vi "UHR-Fleezers Control (host) -VD3_charlie.vi"(0 "Tab Control":T5(tab)) -> ()   [LabVIEW 2012]
uses:
  <vilib>/Utility/miscctls.llb/LVPoint32TypeDef.ctl
  <vilib>/Utility/miscctls.llb/LVMinMaxIncTypeDef.ctl
  <vilib>/userdefined/High Color/nirio_resource_hc.ctl
  <vilib>/Platform/TimedLoop/XDataNode/timing_clust.ctl
  <vilib>/Platform/TimedLoop/XDataNode/nitl_modes.ctl
  <vilib>/Platform/TimedLoop/XDataNode/wakeup.ctl
  <vilib>/FPGAPlugInAG/PCIe-7852R/niLvFpga_Open_PCIe-7852R.vi
  <vilib>/FPGAPlugInAG/PCIe-7852R/niLvFpga_Reset_PCIe-7852R.vi
  <vilib>/Utility/error.llb/Error Cluster From Error Code.vi
  <vilib>/rvi/errors/niLvFpgaAdjustHostInterfaceError.vi
  <vilib>/FPGAPlugInAG/PCIe-7852R/niLvFpga_Run_PCIe-7852R.vi
  <vilib>/Analysis/baseanly.llb/Mean (DBL).vi
  <vilib>/express/express analysis/Spectral/Block/exnSpectralBlock spectral measurements PSD poly.vi
  <vilib>/express/express analysis/Spectral/Block/exnSpectralBlock spectral measurements PSD WFM.vi
  <vilib>/Waveform/WDTOps.llb/WDT Append Waveforms DBL.vi
  <vilib>/FPGAPlugInAG/PCIe-7852R/niLvFpga_Abort_PCIe-7852R.vi
  <vilib>/FPGAPlugInAG/PCIe-7852R/niLvFpga_Close_PCIe-7852R.vi
  openfpgaref.8.6.ctl
  <vilib>/Platform/TimedLoop/XDataNode/XDataNode.xnode
  <vilib>/rvi/interface/nirviOpenFPGA/nirviOpenFPGA.xnode
  FPGA Bitfiles/UHR-FleezersInst_FPGATarget_UHR-FleezersCont_0F5B06C4.lvbitx
  UHR-Fleezers Control (fpga) - 10.3.vi
  <vilib>/rvi/interface/nirviMethod/nirviMethod.xnode
  <vilib>/rvi/interface/nirviReadWriteControl/nirviReadWriteControl.xnode
  <vilib>/express/express analysis/Spectral/XNode/ExpressSpectralMeasurementsBlockNode.xnode
  <vilib>/rvi/interface/nirviCloseFPGA/nirviCloseFPGA.xnode
  <vilib>/Analysis/NI_AALBase.lvlib
  <vilib>/Platform/TimedLoop/XDataNode/XDNodeRunTimeDep.lvlib
  <vilib>/vision/NI_Vision_Development_Module.lvlib
  NiFpgaLv.dll
  <vilib>/FPGAPlugInAG/PCIe-7852R/niLvFpga_ConfigureFifo_PCIe-7852R.vi
  <vilib>/rvi/errors/niLvFpgaMergeErrorWithErrorCode.vi
  <vilib>/FPGAPlugInAG/PCIe-7852R/niLvFpga_ReadFifo_PCIe-7852R.vi
panel:
  in  "Set SP to Reading":bool
  out "Trap X (AI1)":T1={"Trap 1"=-1.0, "Trap 2"=0.899993896484375}
  in  "Trap Pos FB SP":fxp<+/-,16,1>=-0.092803955078125 caption="Setpoint"
  in  "Trap Pos. FB ON":bool
  out "Trap Positions":waveform(dbl)[](graph)=[{"t0"=timestamp(12.90000000000001 s since 1904-01-01), "dt"=0.15, "Y"=[-1.7479351299698465e-12, -1.7479351299698465e-12], "attributes"=variant("NI_ChannelName"=variant(string "Trap 1 Pos."))}, {"t0"=timestamp(12.90000000000001 s since 1904-01-01), "dt"=0.15, "Y"=[6.991740519879386e-12, 6.991740519879386e-12], "attributes"=variant("NI_ChannelName"=variant(string "Trap 2 Pos."))}]
  out "Action (%)":dbl(knob) scale=-100.0..100.0
  in  "Trap Pos. FB Out Scale 2^n":u8=23 caption="Action Scale"
  in  "ESP Port 8":refnum<visa-resource-name>="COM22"
  in  "ESP Port 7":refnum<visa-resource-name>="COM22"
  in  "ESP Port 6":refnum<visa-resource-name>="COM22"
  in  "ESP Port 5":refnum<visa-resource-name>="COM22"
  in  "ESP Port 4":refnum<visa-resource-name>="COM22"
  in  "ESP Port 3":refnum<visa-resource-name>="COM22"
  in  "ESP Port 2":refnum<visa-resource-name>="COM22"
  out "Location path":path=path "D:/UnifiedHighRes_VIs/Locations.txt"
  out "Location Matrix":string[][](array[string])=[["N.D.\r\n", "N.D.\r\n", "N.D.\r\n"], ["0.19233\r\n", "0.00156\r\n", "0.20615\r\n"], ["N.D.\r\n", "N.D.\r\n", "N.D.\r\n"], ["N.D.\r\n", "N.D.\r\n", "N.D.\r\n"]]
  in  "radius":i32=10 min=1 max=20
  in  "clear markers":bool
  in  "trap\nmarkers?":bool
  in  "Pump 3 contents":string="Bottom: ADig beads" caption="contents"
  in  "Pump 1 contents":string="Top: DNA beads" caption="contents"
  in  "Scripts":T2(tab)
  in  "Take Stepping Data":bool
  in  "Got DNA bead":bool
  in  "Got ADig bead":bool
  in  "Cap 1 Flow ON":bool=TRUE
  in  "Move Cap. 1 (DNA Top)":bool
  in  "Dump Beads":bool
  in  "Cap 1 T ON":bool=TRUE
  in  "Cap 1 Samp Flow ON":bool=TRUE
  in  "Offset 2 Set":dbl=2.0
  in  "Offset 1 Set":dbl=1.0
  in  "Cal @ (MHz)":dbl=20.0
  in  "W/ Offset 1":bool=TRUE
  in  "Offset 1 Start (MHz)":dbl=13.0
  in  "W/ Offset 2":bool
  in  "Offset 2 Start (MHz)":dbl=16.0
  in  "Pause at Closest Delta (s)":dbl
  in  "Move to Delta 2 (MHz)":dbl=41.0
  in  "Attempt Limit":dbl=30.0 caption="Limit"
  out "Attempts":dbl=1.0
  in  "Wait Before Save (s)":u32=1
  in  "Fish for Tether":bool
  in  "Closest Delta (MHz)":dbl=13.0 step=0.25
  in  "Stop F (pN)":dbl=10.0
  in  "Then...":string(combo)="2"
  in  "Move to Delta 1 (MHz)":dbl=15.0
  in  "Tether Alarm?":bool=TRUE
  out "Tether":bool
  in  "TA Cancel Save?":bool=TRUE
  in  "TA Green Off?":bool=TRUE
  in  "Raster Set Upon Tether":u32=1
  in  "Save at end (5, 6)":bool
  in  "N Steps":dbl=20.0
  in  "Step Size (nm)":dbl=0.34
  in  "Save ave factor":dbl=1.0
  in  "Dip Trap Delta 1 (MHz)":dbl=15.0
  in  "Move Trap Before?":bool
  in  "Save Data After?":bool
  in  "Green ON After?":bool
  in  "Dip Trap Delta 2 (MHz)":dbl=15.0
  in  "Move Trap After?":bool
  in  "Duration (s)":dbl=1.0
  in  "Dip for Protein":bool
  in  "APD to Watch":bool
  out "Duration (s)":dbl
  in  "Action":string(combo)="Yank"
  in  "Fl. Triggered...":bool
  in  "Fl. Delta Thresh. (kHz)":dbl=0.6
  out "Waiting":bool
  out "Fl. High":bool
  in  "N pts to average":u16=6
  in  "Yank Delay (s)":dbl=3.5
  in  "Yank to Delta Array (MHz)":dbl[](array[numeric])=[16.3, 15.85, 14.85]
  in  "N Array El":u8=3 min=1 step=1
  in  "Random Choice":bool=TRUE
  in  "Force Yank":bool
  in  "Force Reset":bool
  in  "Y change (mm)":dbl
  in  "Profile":bool
  out "Sigma/Mean 2":dbl=nan caption="Sigma/Mean" format="%#_2g"
  out "Rate sigma (Hz) 2":dbl caption="Sigma (Hz)" format="%0.2f"
  out "APD 2 Rate (Hz)":dbl format="%#_3p"
  out "Primary Video Display":T3(plugin-control)
  out "Waveform Graph":dbl[](graph) caption="APD Line Scan"
  out "Messages":string="7:59 AM\tUHR-Fleezers ready.\r"
  in  "APD Ave N":dbl=10.0
  out "Int. Time (s)":dbl=3.0
  in  "Stop All":bool=TRUE
  out "Sigma/Mean":dbl=nan format="%#_2g"
  out "Rate sigma (Hz)":dbl caption="Sigma (Hz)" format="%0.2f"
  in  "Tab Control 6":T4(tab)=enum."Imaging"
  in  "APD 2 Offset":dbl
  in  "APD 1 Offset":dbl
  out "RMS (Ang)":dbl=nan format="%_2g"
  in  "Bead Sep. Int. Time (s)":dbl=5.0 caption="Int. Time (s)"
  in  "Below (kHz)":dbl=0.5
  in  "Above (kHz)":dbl=2.0
  in  "Adjust Scale\nto Mean":bool
  in  "Rescale on Mean":bool
  in  "Offset (nm)":dbl
  out "Mean":dbl=nan caption="Mean (pN)" format="%#_3g"
  out "Force":waveform(dbl)[](graph)=[{"t0"=timestamp(12.90000000000001 s since 1904-01-01), "dt"=0.15, "Y"=[nan, nan], "attributes"=variant("NI_ChannelName"=variant(string "T1 X"))}, {"t0"=timestamp(12.90000000000001 s since 1904-01-01), "dt"=0.15, "Y"=[nan, nan], "attributes"=variant("NI_ChannelName"=variant(string "T2 X"))}]
  out "APD Chart":waveform(dbl)[](graph)=[{"t0"=timestamp(12.90000000000001 s since 1904-01-01), "dt"=0.02, "Y"=[0.0, 0.0, 0.0, 0.0, 0.0, 0.0, 0.0, 0.0, 0.0, 0.0, 0.0, 0.0, 0.0, 0.0, 0.0], "attributes"=variant("NI_ChannelName"=variant(string "APD 1"))}, {"t0"=timestamp(12.90000000000001 s since 1904-01-01), "dt"=0.02, "Y"=[0.0, 0.0, 0.0, 0.0, 0.0, 0.0, 0.0, 0.0, 0.0, 0.0, 0.0, 0.0, 0.0, 0.0, 0.0], "attributes"=variant("NI_ChannelName"=variant(string "APD 2"))}]
  in  "Calibration":u16(ring) items=["None", "Position", "Force"]
  out "T1 X":dbl=nan caption="T1 X (pN)" format="%0.2f"
  out "T2 X":dbl=nan caption="T2 X (pN)" format="%0.2f"
  out "Bead Separation":waveform(dbl)(graph)={"t0"=timestamp(12.90000000000001 s since 1904-01-01), "dt"=0.15, "Y"=[nan, nan], "attributes"=variant("NI_ChannelName"=variant(string "T1 X"))}
  in  "Amplitude (nm)":dbl=3.0
  out "Bead Mean (nm)":dbl=nan caption="Mean (nm)" format="%0.2f"
  out "Difference":dbl=nan caption="Difference (pN)" format="%.2g"
  in  "Take Detection Laser\nImage":bool
  out "APD 2":T3(plugin-control) caption="APD 2 (Cy5)"
  in  "Flip Green Filter":bool
  in  "Set X Only":bool
  in  "Set Y Only":bool
  out "APD 1":T3(plugin-control) caption="APD 1 (Cy3)"
  out "Detection Laser Y":T3(plugin-control)
  out "Pointer Y (V)":dbl format="%_3g"
  out "Pointer X (V)":dbl format="%_3g"
  in  "Set Confocal Spot (X-Y)":bool
  out "Detection Laser X":T3(plugin-control)
  out "Saved APD":dbl[][](graph) caption="Most Recent Time Trace"
  out "Trap Delta Graph":dbl[](graph) caption="Most Recent Time Trace"
  out "Save APD Deriv":dbl[][](graph) caption="Most Recent Time Trace"
  out "Delta Fl. 1":dbl
  out "Delta Fl. 2":dbl
  out "All Signals":waveform(dbl)[](graph)=[{"t0"=timestamp(12.90000000000001 s since 1904-01-01), "dt"=0.02, "Y"=[0.0, 0.0, 0.0, 0.0, 0.0, 0.0, 0.0, 0.0, 0.0, 0.0, 0.0, 0.0, 0.0, 0.0, 0.0], "attributes"=variant("NI_ChannelName"=variant(string "APD 1"))}, {"t0"=timestamp(12.90000000000001 s since 1904-01-01), "dt"=0.02, "Y"=[0.0, 0.0, 0.0, 0.0, 0.0, 0.0, 0.0, 0.0, 0.0, 0.0, 0.0, 0.0, 0.0, 0.0, 0.0], "attributes"=variant("NI_ChannelName"=variant(string "APD 2"))}, {"t0"=timestamp(12.90000000000001 s since 1904-01-01), "dt"=0.15, "Y"=[nan, nan], "attributes"=variant("NI_ChannelName"=variant(string "T1 Y"))}, {"t0"=timestamp(12.90000000000001 s since 1904-01-01), "dt"=0.15, "Y"=[nan, nan], "attributes"=variant("NI_ChannelName"=variant(string "T1 X"))}, {"t0"=timestamp(12.90000000000001 s since 1904-01-01), "dt"=0.15, "Y"=[-0.0004235663930173644, -0.0004722739341410556], "attributes"=variant("NI_ChannelName"=variant(string "T1 Sum"))}, {"t0"=timestamp(12.90000000000001 s since 1904-01-01), "dt"=0.15, "Y"=[nan, nan], "attributes"=variant("NI_ChannelName"=variant(string "T2 Y"))}, {"t0"=timestamp(12.90000000000001 s since 1904-01-01), "dt"=0.15, "Y"=[nan, nan], "attributes"=variant("NI_ChannelName"=variant(string "T2 X"))}, {"t0"=timestamp(12.90000000000001 s since 1904-01-01), "dt"=0.15, "Y"=[-0.0005883053071687949, -0.0006281319620349712], "attributes"=variant("NI_ChannelName"=variant(string "T2 Sum"))}, {"t0"=timestamp(12.90000000000001 s since 1904-01-01), "dt"=0.15, "Y"=[nan, nan], "attributes"=variant("NI_ChannelName"=variant(string "T1 FB X"))}, {"t0"=timestamp(12.90000000000001 s since 1904-01-01), "dt"=0.15, "Y"=[-0.0004680013428144157, -0.0005167699209570592], "attributes"=variant("NI_ChannelName"=variant(string "T2 FB Sum"))}, {"t0"=timestamp(12.90000000000001 s since 1904-01-01), "dt"=0.15, "Y"=[nan, nan], "attributes"=variant("NI_ChannelName"=variant(string "T2 FB X"))}, {"t0"=timestamp(12.90000000000001 s since 1904-01-01), "dt"=0.15, "Y"=[-0.0006226691488387671, -0.0006504715109714008], "attributes"=variant("NI_ChannelName"=variant(string "T2 FB Sum"))}, {"t0"=timestamp(12.90000000000001 s since 1904-01-01), "dt"=0.15, "Y"=[-0.0007901852473525123, -0.0008601641895809732], "attributes"=variant("NI_ChannelName"=variant(string "PSD Y"))}, {"t0"=timestamp(12.90000000000001 s since 1904-01-01), "dt"=0.15, "Y"=[0.00031556138798181086, 0.0002525101474044007], "attributes"=variant("NI_ChannelName"=variant(string "PSD X"))}, {"t0"=timestamp(12.90000000000001 s since 1904-01-01), "dt"=0.15, "Y"=[-0.00019678334910122974, -0.0002453993346964931], "attributes"=variant("NI_ChannelName"=variant(string "PSD Sum"))}]
  in  "Signals to Plot":i32(listbox)
  out "Trap Disp. Freq. (Hz)":dbl=6.666666666666667 caption="Freq. (Hz)" format="%#_6p"
  out "Display Period (s)":dbl=0.15 caption="Period (s)" format="%#_6p"
  in  "Trap Disp. Downsample":dbl=10000.0 caption="Downsample" max=20000.0
  in  "APD Disp. Scale":dbl=0.1 caption="Scale (Divide,\nfor above plot only)"
  in  "APD Disp. Downsample":dbl=2.0 caption="Integrate" min=1.0 max=30.0 step=1.0
  out "APD Display Freq. (Hz)":dbl=50.0 caption="Freq. (Hz)"
  out "APD Display Period (s)":dbl=0.02 caption="Period (s)"
  out "FFT 1":cluster{"f0":dbl, "df":dbl, "magnitude":dbl[]}[](graph)=[{"f0"=0.0, "df"=16.666666666666668, "magnitude"=[-331.1367572010275, -79.05506245821404, -86.61411242440559, -88.4728176091699, -90.3181253945935, -94.12566333707997, -92.52740723119955, -94.92192587982518, -99.60936585245742, -96.87568627870715, -94.02570383337763, -83.8058550151726, -97.57441397235512, -101.59968530846606, -101.523049255742, -103.35038532190343, -101.58594091014982, -102.96098031851216, -91.39759462745924, -103.75019963279499, -104.45030075054324, -103.04245334279298, -104.0720279134107, -106.06482372394834, -103.69131867828104, -104.40395035115309, -105.96420043276396, -107.6735556337804, -106.673030006608, -107.34889066208132, -108.05626565233933, -106.25659018850432, -105.29934513380842, -105.43096056709592, -108.3728498841465, -106.0555440144992, -105.78001282181421, -107.48741857324953, -108.67624970548897, -105.39976667156175, -105.91413119232612, -109.4222808198164, -107.0898971593174, -107.91164191890915, -108.26032038855709, -107.58332347164534, -108.23559688234297, -108.01271040303237, -107.66511723652701, -106.51901583170391, -109.27249501469946, -108.55647681594805, -107.93499259231463, -107.05068166453935, -109.13641475410455, -109.29679733781423, -108.19360835527803, -109.57747591546632, -109.58364591011674, -110.47061433372711, -109.8144340420426, -108.79067462293897, -107.54887553357234, -107.99559866705923, -108.85023923652685, -109.68733225238618, -108.51101278437793, -108.51620475114115, -108.22212402200637, -104.63726950302143, -110.2989919678048, -107.61796444414897, -108.68882962798736, -104.79193983043893, -103.59504263746938, -93.64633660288543, -101.9191640501395, -105.73717393151816, -108.92572458793902, -107.43962662800902, -107.79595323081325, -107.0923101993207, -108.17603277205289, -107.87074270713183, -109.20899066381877, -108.61832060412445, -109.10072003106593, -105.76480632823524, -108.60877649218978, -109.67541158970121, -110.2286232768028, -109.84952155309578, -109.33772024076384, -109.95251642394683, -110.14777282585466, -109.13825677905699, -110.05989365698167, -109.39359990189426, -110.56255614635295, -109.66477183197163, -108.9397158528824, -110.26529907650465, -109.20049464984628, -108.20183857013548, -109.09752250184418, -108.00440442238454, -108.35465963524055, -111.16774134451799, -110.34812550238405, -108.94506763426756, -108.72845542102493, -109.41512344014713, -112.44661664432377, -110.35437330889101, -111.32939440655925, -109.42989530434981, -110.98084669076195, -111.92160561143541, -108.57755551751093, -111.40042616180912, -110.15284955891853, -112.21455132279115, -111.40787773511747, -108.82949641635288, -110.13442122547907, -111.42229298204664, -112.06314940885191, -110.6015308813694, -109.51144097251623, -111.15989713761475, -110.25535755335385, -109.65868178057926, -110.51649885452997, -109.77194745285269, -108.4234206864394, -109.50892632093968, -109.46471287444389, -107.92241289271415, -109.72283805386196, -108.63426821579918, -110.37316681536255, -111.09713996884652, -110.32903619589223, -105.32012665515045, -107.36858557554393, -108.00382215905725, -110.06430686942338, -108.81666625979916, -110.01277074453823, -110.94194741225512, -109.65934609082873, -107.80979136006962, -112.81333866824724, -111.61474300955487, -109.83998277184975, -109.45953946904639, -109.79640584952526, -108.19172301667324, -109.28894656674316, -107.61471301278785, -108.83814006090513, -109.08866847726084, -108.20250571862371, -107.96222236861584, -107.03811197900873, -108.93533000393974, -107.74482548035408, -110.79811544577694, -111.1387476496877, -107.42970105883512, -109.18442281176472, -108.73546184641192, -108.71800246690864, -108.51945944378063, -108.06825856571285, -107.27210712368412, -108.12304695877637, -107.84933283677306, -109.73682373154998, -109.32284761503395, -109.31328817453769, -106.68762108642842, -109.79203616876461, -109.9020278896408, -110.27080024357275, -108.54152101558762, -111.00464391726017, -112.42244020766577, -110.82707315747889, -111.00344011890857, -109.90461839395674, -109.42877207451863, -109.73549298167016, -111.67494793393293, -108.85799077901427, -108.5348443278263, -109.803781083881, -108.30644755543659, -108.5079527456017, -111.2055351312823, -108.53089994340155, -108.01739789012176, -108.70360662855235, -107.95873456794631, -109.58297170693093, -108.9372401694271, -110.15921663527153, -109.22399119911955, -110.89883651739237, -108.92840112258382, -110.0545300523626, -109.05961065387005, -109.45831398589371, -108.61239387653227, -110.13001256174265, -108.80060224137931, -109.46327400696283, -108.0177965824709, -109.29727944627197, -110.3237255895986, -109.03258262543821, -110.97880178489321, -109.70034895077919, -111.16405638194153, -109.17324451464711, -109.65698250854277, -108.96750235822178, -112.00534231585624, -108.69274607723942, -108.98110446396657, -108.40723795464795, -111.44459094807324, -111.74799245277113, -111.1601960491512, -108.92048232753773, -110.30506377784799, -111.33145973979093, -110.91850998672503, -110.33684985776448, -108.90206518366908, -109.28458878227542, -108.98773986023751, -110.85813863075646, -109.00041591105906, -110.84543686681204, -109.84382395806176, -109.69722434763266, -108.50915601095721, -107.80829925826895, -110.59736107582401, -109.75377770317087, -109.3992084496136, -110.51151565846742, -112.49753959826434, -109.7299632589479, -109.54070743868353, -109.90314341132164, -111.05974202976806, -109.03766862152392, -109.46667095459878, -109.52800799036197, -111.3163121356807, -110.07817134522178, -108.69251657453547, -109.40472158898045, -109.71400709815576, -110.60534468715097, -109.46937396724682, -107.70342491418788, -109.86331122597839, -108.64971387994616, -110.90117371097081, -108.34928840565928, -110.04172889660904, -111.52979926554961, -110.34759300823305, -109.62712781837159, -109.24131154553284, -110.23196152450447, -108.68509612326807, -108.0246905483419, -106.61876139289784, -101.5519630114271, -80.57695480953835, -102.03744443354402, -107.1449217193017, -110.0695213407169, -106.61597783999268, -110.79221011808191, -109.58974545931426, -109.1149802216988, -109.20993813088597, -109.63768480465863, -110.10428394219181, -109.08445084271477, -108.83472375362581, -109.69508502050168, -108.05588796178941, -110.62586360101581, -109.95315261676905, -107.52208264977473, -108.80708007514875, -110.43484881098874, -110.45942171588936, -107.83804717866751, -109.98973910294193, -109.3496496054193, -108.425252911127, -110.94579264380809, -108.54181722177951, -108.67696070083541, -108.4150202151644, -109.24973583101504, -112.0454922608961, -111.29046597340738, -110.75018248960077, -109.38326363603683, -109.2033340336957, -109.45076170874889, -109.52878049853727, -109.32340869724774, -110.98123395128233, -110.75736340635505, -109.7218385823809, -107.97422606064993, -109.77313701758703, -110.95948744392717, -110.08996774172691, -108.51011830110778, -109.78063140243836, -110.65996628628228, -109.83684298615616, -110.33329049188029, -110.13755118968292, -110.3717925645783, -108.55302219178951, -106.86811628734195, -108.6302156589162, -108.75341391045045, -108.32589578384841, -108.70061474734084, -112.30742263527534, -109.16842570592085, -109.29767035534508, -108.87829025017463, -108.2255616391397, -108.4316108616088, -108.82995906929271, -110.40135575415563, -109.51623498946435, -109.79409808792403, -107.03832759632121, -108.36534528684132, -109.72010868372905, -107.90933028179892, -106.95643597294047, -111.29929166165778, -110.23001135794706, -108.98838015381585, -109.79115357104436, -108.18627479511115, -108.14988122174307, -109.12074063466532, -109.41904850488358, -111.40409873721113, -108.83156790193294, -108.77032248953847, -108.88363158686694, -108.47515048290681, -105.94172147874599, -109.38146940214403, -109.21277078848794, -108.11309390545507, -110.70840012427504, -109.5504457849329, -109.52330684534209, -110.06776026911132, -108.21949434182314, -111.21266686269992, -108.78581501170974, -108.43115799297222, -109.63260325780062, -109.84070220619535, -109.72041980780126, -110.29615941882527, -110.60316734262464, -108.79165446414692, -110.95840439895592, -109.64926233107009, -109.16526769544322, -108.65292362430982, -109.56113898129935, -109.85693046339026, -108.92316027325207, -109.79492493553914, -109.38157962945887, -110.24545136266825, -109.30031463492487, -109.0795429936869, -111.4091719525013, -108.63499083917162, -108.43863465339358, -109.23207864880891, -111.21947487191643, -109.24525201480154, -109.56842406077318, -109.46711940800672, -111.91389548262572, -108.15655736690546, -108.71882059966947, -111.26328503478568, -110.95027143873176, -108.4853106242357, -110.36902802777546, -109.9314203579182, -108.77686164101732, -108.71871020068312, -111.04829661168574, -109.95072655339462, -109.88221342875462, -109.53241732756136, -108.2625005404823, -108.00677030040697, -110.19659317581693, -108.93858924796267, -109.46817875483995, -110.78063992017232, -111.11066570318451, -110.78774336696706, -109.19199744617812, -108.54914256407436, -109.28414960420909, -110.64143585101183, -110.5855350821307, -109.47578632252726, -108.89705360836223, -109.89214013612292, -107.93271261027171, -109.32631601340563, -108.60274611341092, -109.40110159872573, -110.889237682208, -110.01391165813328, -109.99747108785071, -108.65542819213674, -110.37211847668736, -110.44656500845738, -110.8128133834973, -108.8909299260433, -110.19551227077532, -111.37647266643523, -110.83802189730321, -109.98519377913681, -110.52378970770522, -108.16970420057817, -110.70974729773344, -110.76836765494402, -110.26884275594577, -109.22041044268806, -109.87809744746195, -107.76823252107832, -109.12119474042969, -110.28066108731146, -108.55000033509207, -110.18152097767907, -110.73030521152278, -111.49470908029893, -110.2320929919509, -110.03370979233021, -109.79181668155233, -108.6673501209991, -109.86695766650877, -107.88926518046961, -110.95525003776572, -109.18130359755742, -110.42618009658618, -107.90341931158893, -111.44736855661769, -110.72634267386593, -109.29945988519303, -107.67889101961411, -108.81148059987765, -109.13375212757057, -109.8122873383549, -109.80176697684155, -109.96342275204768, -109.90406635707086, -108.75674342748256, -110.12362902701081, -109.82151095527837, -108.62543344241836, -110.09171852771195, -110.21434637862887, -109.97254504855631, -109.27043209093468, -111.35149588204125, -110.12399876776051, -111.65983675538546, -109.28788875768564, -110.86554069990251, -111.26990906470603, -108.60956517491746, -111.49613890850938, -111.79685722966795, -109.26269485364045, -110.38555615546439, -109.40641023162068, -110.966136593156, -108.78892524584494, -110.29340727375603, -111.44032043281035, -109.95212021173755, -109.79233511584334, -112.41184021118175, -109.73687851881148, -108.65493879781806, -110.76132988919045, -108.43230346094671, -110.32968175895853, -110.29890782023821, -108.77609076424456, -110.3298662333555, -109.47734504217333, -108.2677295732245, -109.21234363352882, -107.83278941978479, -108.85136784424789, -108.43241251530755, -109.76609391460555, -108.53204373005357, -110.9660641972934, -110.3152512161094, -110.72570499399905, -109.23877906286317, -111.72407743101837, -109.20311421918561, -108.06021800233717, -109.29288625761943, -108.78395253409145, -111.85250172876302, -108.78827588901797, -109.79775055719482, -109.12089297455859, -109.49896359356035, -110.34432647103819, -107.94700097960238, -109.30489238477631, -108.89170290869342, -108.82574563272509, -110.11024077194833, -107.37946433552314, -109.60167933458756, -107.80625057819019, -110.11489057210264, -107.35436859378505, -105.69819484613895, -109.11280625683739, -109.27770293057978, -107.7053735252589, -109.75022444894368, -109.3310543596577, -107.87683693707739, -108.19931495338068, -109.26462246191564, -106.71885779297867, -100.00018022217961, -92.54434511397295, -107.20472143807373, -107.39203415155283, -110.04461177268398, -108.48860496315312, -109.0057168110333, -108.37627790492552, -108.4108380728248, -109.65509454313073, -109.64243000632982, -97.04219069306761, -109.0928856629964, -107.9760697315632, -107.52611064047497, -108.87702814778996, -109.08437599027614, -110.70097118837974, -109.00969860961283, -110.38275386163214, -110.0699155421545, -106.91498895181175, -106.22178738309017, -109.36827866896039, -107.59953130968307, -109.19516217272808, -108.31502495393616, -109.384158926223, -107.11670654202719, -108.09436312738853, -110.14559230873704, -109.84997663447679, -107.83465335309926, -108.60947100624459, -108.9932479423645, -109.17174810371898, -108.79457339828916, -109.40909327982367, -109.6328723628302, -109.51081854476179, -107.63054408568418, -109.63728404010122, -108.51163794839918, -107.55002282725216, -108.97796212764939, -107.24648164623483, -112.21470452291085, -108.74294024554423, -109.62070777514892, -108.05768666239368, -109.8224946685739, -109.34575507446003, -108.53536952609525, -109.60789300457671, -107.56681538208278, -109.22777325016398, -108.79047910308894, -110.10332477250668, -108.00206387955672, -108.45604004720035, -109.00645795765472, -109.81039564269616, -108.92785144634745, -108.3978471520567, -107.94411095685999, -110.53486519304262, -108.8773780319227, -109.03345093296107, -107.30746693745031, -108.54277704832029, -108.77629108166091, -108.91111762599647, -107.74965195880401, -109.97375370738439, -109.76326492689246, -107.91717581777407, -109.0730556927617, -107.66804873204664, -110.40438871064791, -108.05794247751498, -108.80206615156494, -107.51329354700796, -108.83687012994949, -107.57713176895379, -107.94774159581414, -109.41894615439651, -107.10869425078764, -110.51480854078629, -108.92221367099775, -109.91358786461535, -110.1744263092835, -109.30795472883494, -107.91359710691006, -109.77888185049835, -109.52060975706438, -108.66686651982212, -108.71041801553639, -110.13619546359467, -108.87957097273856, -109.72150387215271, -109.00776068810654, -109.70251113927438, -110.75769213896399, -108.53234896741436, -109.69439526582246, -110.15412541604617, -108.25183374628219, -107.97402569656481, -110.34920156998648, -108.45106995186384, -108.82031145748209, -111.38690005057539, -107.01968459818563, -110.3044500039584, -110.8755481852125, -111.08915057663255, -107.94824988655199, -110.21669144934839, -109.90539774633154, -109.58985438756767, -110.12258796623348, -109.41689951612143, -109.31128210476795, -109.00258476567323, -109.11093063041056, -108.83347064311234, -108.32685287566952, -109.44770946560935, -108.40145063144861, -109.68448193892085, -108.76525439243828, -107.62837139034596, -107.39300298848994, -109.36993934990318, -109.2465218489418, -106.66307369796812, -110.15891092764934, -109.57151745419041, -108.92425698310808, -109.8036704717834, -108.79751146756549, -109.25926431818017, -108.46260574057584, -109.1967554647261, -110.63319560262356, -109.02343067385144, -111.22073171487528, -109.4731095097105, -109.69335000085164, -109.48782989577005, -107.95204227683271, -108.19468255763758, -111.36195112053247, -109.55696116543685, -110.3130767640534, -108.9621824253354, -109.99735074896789, -109.20198058456344, -108.12100614259485, -111.27227490807289, -110.09248554008288, -109.14395535060149, -110.80882692379708, -109.22632926901655, -108.64497210802793, -111.00030482190711, -111.1317849358033, -107.43140429257826, -107.9783302193555, -109.2639893652291, -108.97008485446163, -108.66556668859064, -108.12995785876932, -109.73001061107855, -108.09691302413727, -110.68391499215569, -112.78583642012705, -108.7093037763389, -110.67868795924797, -109.0190959349128, -108.36247198231372, -109.82829353258869, -108.24916379311045, -109.84154533905823, -108.55470160833775, -109.75438989348815, -108.82865632118325, -107.63622268162582, -111.00943492886312, -110.81824358463759, -109.46028423652966, -107.52479398900992, -108.99087806823736, -109.94494831750349, -110.26788355564504, -109.8954055022304, -106.9478122391182, -108.91705388158901, -107.76095584490312, -109.28456723055147, -109.7982307261767, -108.98552661346622, -109.98937979783426, -110.57907422426224, -108.68113463944836, -108.06257240208589, -110.0707224529617, -109.19515280354733, -109.35868842818849, -110.37311467065695, -109.0404734478992, -108.16686395270187, -108.61859220485148, -109.19986437876149, -108.19707189725302, -110.06564239663074, -108.87850403465154, -110.63824157544798, -107.36918104067212, -108.7008736325543, -110.9359398265406, -111.08529123080929, -108.44209934821818, -109.79529621208783, -108.38917887958179, -108.169117639508, -109.24332926356216, -110.50584058811704, -109.63592524002665, -109.32261039377495, -109.16720880524552, -109.3084314664462, -109.5812223978583, -107.70213196487856, -108.0557884982431, -110.67058020007828, -111.68459781023608, -109.66270627185824, -110.52536245663693, -109.70208409132103, -108.78645420809342, -109.23122088059863, -109.24601474121832, -111.25604763816514, -109.50225851581177, -107.32434217163818, -109.28548556764925, -107.59972621660836, -110.46928774723048, -109.25950101547609, -110.32016453935465, -107.78482761561703, -107.89462895091089, -107.51366154391481, -108.08036891159172, -109.53371809947035, -101.2452927166745, -109.32763325689056, -107.52166868423687, -109.89648659445174, -109.11350200980485, -109.81336712738089, -110.02799517445062, -108.02767143538516, -107.97850220501483, -109.50772934896838, -109.31069875721964, -108.49991657749598, -105.60880911233095, -109.79128597340213, -106.91084537903113, -107.84880087118997, -109.63628170511824, -109.03203967193224, -110.64186113413658, -110.98027990365594, -112.33841002907062, -111.01793075565425, -108.58025797022215, -110.4259296883756, -110.38643255981424, -108.93051671115133, -110.97544177116494, -108.63883100482677, -108.37581711765226, -108.90240163126536, -107.94688047875466, -109.9482937437732, -110.09097112364414, -110.09805032265376, -111.44307114024532, -109.15483789122554, -110.9713708217832, -107.8548737634672, -111.41418477109195, -109.45699779859628, -97.03595099331734, -109.16746744169623, -109.66209204485918, -112.57048704774604, -109.73989735035725, -108.16252575067017, -110.7546980664636, -108.91536673403449, -109.20509151422344, -111.0260632167785, -109.62924582406518, -110.45466277291722, -110.2973970018937, -109.67550222925419, -108.84481022020094, -107.23686414357573, -111.79004633370906, -109.85453094194085, -109.45617270081004, -110.73920606732504, -108.90879956851099, -109.67774425528265, -109.4745715721361, -110.18080454693559, -109.26079184315502, -109.41692499885505, -109.02240975088358, -107.80833423058168, -109.32657361431549, -107.87138278655101, -110.910364670719, -109.70067156846706, -108.55301754282077, -109.4243252157005, -109.77567725161107, -107.83737232063925, -110.36509412773016, -109.6371048811367, -109.49430894422814, -108.55509251499753, -108.03996302911446, -110.4385715838736, -110.08864436068788, -109.48922484379962, -109.90865554258562, -109.7491963238264, -110.04796094537969, -107.413043439116, -108.54229076126079, -108.2522516728666, -109.75464941327974, -110.26795832300996, -109.28073673851144, -108.62990200974927, -109.89408067552287, -109.09160284731726, -109.90740624925795, -109.92534708896517, -109.79578862362752, -109.97278346890566, -107.80679350393824, -112.81728446281548, -108.09689504419987, -109.89549991422173, -108.43930976031248, -109.95153099843282, -108.18277483720716, -111.89607792605433, -109.52567003805, -109.17125106979698, -109.64300739407085, -108.21045178846524, -109.64036472149706, -109.02324448538845, -109.039163008889, -110.41006510134076, -109.50289952116489, -110.4732620447796, -110.08777181504614, -110.15589511434341, -109.55705089158471, -109.2547682932589, -110.86823885471617, -109.96330502176939, -109.85995369810554, -110.63211290903473, -112.08007783432191, -110.24725218052279, -107.62861148917592, -110.08691795849435, -108.89793794632287, -111.07702220466341, -109.46946126482341, -109.19747345337464, -110.70018609416007, -109.66366205691908, -110.78032312133551, -108.05724200456513, -108.195661625627, -110.90724508408255, -110.08307674771669, -110.76863516643007, -110.46620425061583, -109.16986788877276, -109.61921294239114, -108.51159432329543, -109.96308336765689, -107.38178944242856, -111.95930944846394, -109.3329826827624, -109.59119636368249, -108.83148571828912, -110.46194288788257, -105.87694286145472, -107.985886302892, -109.2975019660806, -111.05138725716857, -109.60005889204612, -110.92871351729086, -110.73480546964537, -108.41587420326718, -109.84275465824477, -108.8249071047676, -107.65358887817105, -108.3254150042995, -111.47362100321767, -112.7287536850025, -108.8217125660507, -109.50232320231771, -110.29587061625348, -109.30644535112089, -107.69178032077258, -110.84522325672016, -109.3735891463141, -109.12506388923123, -109.65582307934665, -111.11427272192576, -112.19827973435466, -109.11306367925813, -108.19203577968261, -107.89831568266465, -108.85805249169313, -109.51100049661844, -111.71546684086955, -109.53880495724334, -107.07739286222231, -110.66836728754211, -111.5415170557177, -110.16051267940297, -110.6107546662698, -111.36389129556191, -107.77888179117923, -110.34160392509817, -109.61287125994414, -110.23791773883013, -111.00669159903549, -110.97165069538953, -109.43965413392434, -110.6813161690388, -110.31441293654314, -111.96129906273796, -108.15998218707462, -110.08095912053633, -109.41084567452768, -109.28774416263552, -110.80159950384204, -110.41956747809755, -108.85005186267244, -107.9069227847757, -108.84249369063123, -109.92569208845894, -109.34109797584448, -109.41334788055491, -108.76462023086997, -108.22069272136177, -107.0786679601274, -108.30206755098202, -108.57613406368954, -110.83330887636482, -111.93966942736989, -109.76373713473264, -108.25782074884941, -108.16490627215555, -109.93351470267982, -110.75525684428368, -108.22814762283093, -109.73442331991602, -107.53145627482685, -108.27195221226805, -110.33032779278457, -109.48951857415828, -108.12599093700939, -107.97627415508097, -108.81426859968796, -111.21764717894752, -109.80856212352333, -110.92658779118501, -109.71551885834796, -110.38682741010847, -108.87671328341361, -109.68368600774755, -108.35359806351899, -111.7519400010676, -109.89407081573103, -108.24301180922755, -110.00646944788126, -108.6685299083706, -107.52856885980722, -111.7622363038509, -111.0025144494897, -108.64719599357296, -110.62968467177518, -108.821509935539, -107.94915453463719, -111.53070432277694, -109.87282048586256, -110.71167589371663, -109.79225006081626, -109.96203471712074, -110.29921092232489, -110.10644439440416, -111.28815007382043, -111.19165661703703, -108.46024117100558, -110.22528296512183, -110.32184972386672, -110.05120383416072, -109.78792549362107, -109.00355659956696, -108.85989369286315, -113.00899556732638, -110.91756826567867, -111.25016866167897, -111.84225040552181, -110.54451635944174, -110.72722829912917, -109.60759702177283, -110.49362602516815, -108.74419542915284, -110.3379671069179, -109.66259088220754, -110.45956400953156, -109.13956157147233, -109.27130155486806, -110.83015602667983, -109.17970724944131, -109.09662765889193, -108.0447366108107, -108.9536269357457, -110.35663108940085, -108.73418835472056, -113.42965806805827, -111.81270536656905, -110.06155590173537, -108.76582224646269, -106.7488061675813, -108.5700320158723, -111.11038264410035, -110.41435767488723, -109.12763443489911, -109.30517580756394, -111.61251165371237, -109.8116632664339, -109.36845864976851, -109.00390009629231, -110.54359197165573, -109.52629258465976, -110.75932197632896, -109.50903215359567, -107.42652056246085, -107.81146496533543, -103.22224383145215, -108.53803076819163, -109.78623360072066, -109.66306634612869, -110.80245829141279, -111.87835085452016, -102.27372781471168, -111.27763038431458, -108.45838423437681, -108.79077917058028, -109.31951755762685, -110.05415097017186, -109.5535934823387, -111.62732254641111, -110.73478247119641, -109.9468722686683, -110.39698367573979, -109.30612942398305, -109.7578384694043, -109.34817295524313, -105.56944757301993, -110.1940418750125, -109.27076023513962, -111.03491935225027, -112.2980497521063, -110.65725497955563, -109.0567530102422, -110.31700596563523, -109.64508026365678, -109.6190471404421, -110.52566833759428, -109.68595899227789, -109.7431160985074, -110.4798230300751, -109.45506977604765, -110.69504157940786, -110.63067849573177, -108.06456949500138, -107.99354148885966, -108.11349194720599, -109.15944121207349, -110.61766925164031, -110.14145801314527, -110.67420842201165, -111.91532881806512, -112.15901550030345, -109.94774413630104, -109.2819568305201, -110.94623189179737, -110.17685430287735, -110.39082916961016, -109.53953238698966, -110.76940623620611, -109.89327922318515, -109.10275695043765, -110.21445972656734, -110.58968777252528, -110.57016757660259, -109.59208496373341, -109.07946946465374, -109.10762003745964, -110.36892993974607, -109.81864495218393, -112.12972189864566, -109.26185849434863, -111.56305819991357, -111.36019621828058, -110.3397604159226, -109.58675612753163, -110.58041217474447, -106.34739062044932, -108.6722699609389, -110.03906060709869, -109.16794717548382, -109.65012481802809, -109.35377624077988, -110.51889143862303, -110.03397458059777, -110.7981307056636, -110.56653507062292, -107.61367005067231, -109.99279736988825, -111.79875182878175, -108.60382315996031, -109.71381533228038, -108.60388131505613, -107.0933685540362, -107.86037690830757, -108.40980028847238, -108.83869602763895, -110.76921375395764, -109.96766364716046, -110.8256171465781, -110.13805084291067, -108.5349140035878, -110.57158437465219, -110.8920694413417, -108.71646695477324, -108.33274238445665, -108.96152108305608, -111.03750932994224, -109.48915027983756, -110.29725207211165, -110.79527247268442, -109.47969936716117, -109.79306701834035, -110.16840035577498, -110.29840230783668, -109.15306387075587, -110.72651274964761, -109.08881658764956, -110.8349724030761, -110.64653625576447, -111.40392562616867, -109.94581588927414, -108.85136340231294, -109.77228546607624, -111.48297395390018, -109.7334001251941, -109.30537415590783, -109.63937411233408, -109.69785848648013, -109.3523781030017, -112.04667421182404, -111.56311816195343, -108.18548447362308, -110.63388993686104, -111.39768634137992, -109.87157345395542, -108.6734208287271, -109.46213300216168, -111.75774769437145, -110.10245994173216, -109.52385139033495, -110.96513097775451, -111.8709319163154, -111.54948269614047, -110.29760900080463, -108.52168175904663, -111.09033925738258, -111.14752744054172, -108.83074523709202, -109.05704141259113, -111.74377805749482, -109.57200906899736, -108.84121318623825, -110.86657990204343, -109.54363603755047, -110.89448416316372, -109.58965570570145, -110.21012263847972, -110.4063470702923, -109.5021950342969, -110.33648801598177, -110.90551031296536, -109.69205870504638, -109.8648503154861, -110.28183391384131, -109.65970942950766, -108.43615680946908, -111.11790511866548, -110.89043476451553, -113.64898442872548, -113.08004494963895, -110.81525412051718, -113.91009875719509, -110.95802128672312, -110.40944585634135, -110.33464695414992, -109.98984645778987, -110.18795067005652, -110.62364351231234, -110.44029833291248, -109.01598585569788, -110.95430216511514, -109.77987141110621, -108.54452361812068, -111.41780266439777, -110.47172771858405, -109.06084635984516, -109.30794593246578, -108.8764083815745, -108.18222749506985, -110.31330487887435, -109.04176821738014, -108.8558386035048, -109.47888284507395, -110.01459604573937, -110.48596659065309, -112.6781342298378, -109.85522803775775, -109.0569534499285, -109.08991286548698, -110.89485727880403, -109.18715778948663, -111.50381433568144, -111.3545424730884, -110.07710926239977, -111.99977850157067, -109.47444853853723, -109.81605328527645, -110.74995213151195, -112.56834665925544, -108.52052472391404, -110.89121213995557, -112.02004142355113, -108.66413739656008, -111.10053848695652, -110.41241079991636, -111.80152991764473, -110.21746151515111, -110.63265128607344, -109.483042128511, -112.78639954059729, -109.47114195846122, -109.23309637902875, -108.97133643967169, -110.08909147812822, -111.01105271457081, -111.18602432128249, -110.04633990216801, -109.53453538673071, -108.81939452082017, -111.13486114285661, -111.65877073200598, -111.63763706753498, -112.14107810664572, -113.6231865196724, -109.31743865878806, -109.18551713085722, -108.74951309653638, -109.28206426212142, -112.36687029711229, -110.10933061193728, -111.29501093502684, -108.19021080564794, -109.34497312126749, -110.37228033937312, -108.63277512903049, -110.61033993911002, -111.2975761598062, -111.49780004751436, -109.91019436685814, -109.32789992989028, -111.4482538110117, -110.1538439123475, -110.66347034043578, -110.05055133068794, -108.53002033538341, -111.7522199783972, -113.49108651193104, -108.03793940563418, -110.07108694011555, -110.83958739865201, -109.62805629409038, -112.69637731014087, -109.57996950503268, -110.104850643722, -108.83376203949506, -108.69400304840181, -110.59434352922563, -110.69121011800921, -110.18694553784364, -111.90598571547098, -110.30230802494223, -109.66810649416752, -112.6017099000434, -111.00296745333219, -110.64462650261785, -111.4775358707403, -111.98753241268494, -112.26574909791167, -112.04796822399412, -110.65853064447325, -109.6623218025264, -109.40559579075378, -110.42174451813142, -109.18991987957241, -111.02050178263048, -112.77950487440032, -110.42443751566815, -111.35440372400903, -108.5263524245987, -105.07498063939795, -107.15444425741984, -110.4508720018025, -110.25163264819463, -111.1383261104107, -109.91171620173931, -110.52200560606038, -110.5299174299573, -109.34628087255733, -110.26101817411786, -109.65071853372183, -109.66953335961068, -110.83590602054682, -110.980546313788, -109.4110066989163, -111.47223607390256, -110.00281523859483, -109.4088722967626, -109.00401922839337, -109.59655302543185, -109.7359970854586, -111.46016206343049, -110.23478747568004, -109.29441275295858, -109.82941912510167, -110.43088525283673, -108.21649744751299, -108.70220592702613, -105.2334473604296, -110.60620657984927, -107.97533820921146, -110.7664079806058, -110.56406610911355, -111.76465470250328, -108.84172809688911, -111.03661078143631, -109.85351980370237, -110.70091167176791, -109.52380717508088, -108.4356492672842, -112.25498760397127, -110.69648730540193, -110.36748838594507, -109.99090797924349, -111.2678642544111, -110.42541694325627, -111.4575545259775, -109.3211175669008, -112.7465573314208, -109.56208667784249, -111.59733497772172, -109.42295730962105, -108.55804089331346, -108.71397903286748, -110.09188290952392, -108.90810063278326, -110.31333217069538, -109.69794714542728, -109.06210020835357, -112.42465112160288, -111.74630553904855, -109.99304310093493, -108.93867687355595, -113.1669287525049, -109.09193568851137, -109.27500368450697, -108.99643325722404, -110.53962759110647, -111.2052088429852, -110.05855563908841, -110.30763723153481, -110.03411001268613, -109.6161415052669, -110.6304714466923, -110.17116005754627, -109.0753171640551, -110.92564270851628, -109.60831770517053, -110.25913363817017, -107.76644895378317, -109.2619309023068, -107.64198246311884, -107.37056168314048, -107.31978563121643, -107.68171928702894, -104.57515288104209, -104.75187637758803, -105.27246893266054, -106.96524396060869, -105.93920355631757, -103.66449995825586, -104.08476660009461, -104.53081578265315, -103.0148493379086, -106.74751670818362, -104.92309629919443, -103.98320340724693, -104.81633219413234, -105.77996356028235, -107.12559309216644, -107.28196039053535, -108.84583578337953, -109.4494696919565, -109.15525441177898, -109.7634811359225, -110.79433338587495, -108.44440079452527, -108.79597700117748, -109.98590735173822, -110.72144284267539, -109.30550753718086, -109.70072152916897, -109.65801130162137, -109.65949265997646, -109.82238573025273, -110.30669821947491, -109.83394128869384, -108.90433312205332, -110.664046708231, -110.39926453734134, -110.37725911098757, -112.12508639032839, -110.26795666332589, -108.98741993218054, -107.76168841100478, -109.82334992872889, -110.83516363498563, -112.60649745671253, -111.1960726449926, -111.03919163866381, -112.05129034965563, -108.83187987662883, -109.57240688505179, -109.32857861150738, -109.54934849013647, -108.29359879300195, -111.5179112931669, -109.52702486426027, -109.95429980789645, -110.7011078611564, -109.43204524997455, -105.56031249677113, -107.70609254346495, -108.78303653454363, -108.11457060956113, -110.44215460317537, -110.78267897406572, -110.33119812901934, -109.34449539666907, -108.82636558484161, -107.1834151347969, -108.83808254322192, -108.2542825327446, -108.80298057862501, -107.59922121598055, -108.9131916496929, -109.51519107961856, -107.7704986323755, -108.79678029009878, -111.13791068210752, -110.402746275919, -111.31702623823912, -108.49812727557243, -110.63723264798182, -109.32890666586829, -110.29721723278237, -111.66560929315017, -111.04227698307153, -111.36927505376269, -112.5203298417673, -109.93967930487354, -110.14533835678606, -110.3868348991775, -110.85413569165249, -108.44519725537315, -107.93391978795047, -109.82778679299085, -109.79311153223738, -109.25261055399044, -111.47738679135526, -111.11775495397512, -108.65898844492045, -110.26505495390529, -111.02017977446526, -110.34817965403467, -107.55161094495372, -110.21667403085983, -112.43970497917284, -110.70535338255132, -110.79438078890512, -109.81809822502822, -108.99167960596515, -106.5556893069368, -97.51736665041192, -105.29926513345109, -108.72453297392224, -108.23203912463346, -109.50324111400698, -110.9939986929772, -108.05367524487318, -108.37339392211176, -109.8553291283933, -110.46179639493138, -112.48795697163695, -111.88145079973545, -110.8678969738583, -110.62677605624849, -111.83824818603244, -109.76798658735359, -109.6654742351465, -112.58543522753767, -110.3406716250781, -109.55013159400883, -108.00481229232405, -109.90793236599207, -111.28597960985334, -110.54144527494444, -110.14704702870655, -111.2652554338908, -110.97520848958668, -108.63647576273343, -110.52472680617548, -113.16137826273847, -109.62457037485827, -109.53869420402964, -110.71399284283449, -108.55435337782664, -108.09492728294455, -112.2373886856363, -110.3693019226993, -111.65116752865308, -111.3223986412311, -109.67734725401074, -111.36420709226297, -109.14293108556625, -110.5982939020188, -110.29596476096043, -112.69847120697035, -108.39052787054206, -109.06205229490357, -110.00045399262885, -110.71775009467346, -110.69530760167493, -112.54144940754935, -109.55755373438097, -107.88943697845929, -109.98578587243783, -110.14202980613851, -110.80051915904802, -109.11327182471621, -109.50637030500913, -109.77023677605327, -109.98552825925917, -110.40235854896, -109.37603004890141, -111.36989177909379, -110.8399811877331, -109.30394670937987, -112.2769814990538, -109.10893172594731, -109.17733972841754, -108.35968166480572, -112.64492569586005, -110.13779257328873, -110.64439690778532, -108.45446935516622, -108.97325006911116, -110.54637968933774, -110.66412364132371, -111.38627695224784, -109.8942998516069, -110.36392017322382, -109.92355133054227, -109.61886697310419, -109.71969465343778, -109.85627196259388, -112.1407808286419, -111.1013489416651, -110.70428953307596, -109.3454280179969, -110.22984684615578, -109.53826801613613, -107.83673208330934, -108.72742563398342, -109.5745872123195, -108.83031823548816, -110.89059911076627, -109.87842545384129, -109.21980161063786, -109.07140273870678, -109.04628915564135, -108.79255665097845, -105.20875397856382, -110.0838008881032, -109.68293832806683, -111.24644641302518, -110.01257579497496, -110.99281477454484, -108.99296184719546, -110.96495665514604, -110.70404386182749, -108.25078498739035, -100.77667501455139, -107.61479263900088, -110.06600976399395, -110.02035637581871, -111.45524052052504, -109.975541184397, -111.07333860975358, -108.4808974233161, -109.59513524582242, -110.74711589861774, -109.50005300854993, -105.23071652566294, -111.81094849223531, -109.0168079712372, -111.89029991620679, -109.90672274216391, -109.30959446424889, -108.23718655264584, -110.10868108588909, -109.21139771899594, -110.33333323577992, -110.25792318324204, -110.67825932924109, -112.33148517950511, -108.9724848367048, -110.78371843797613, -111.40913868573313, -110.2930522718577, -111.9538408094371, -108.63639312641844, -112.4462941079034, -110.40266356498321, -108.66617580940074, -109.44306834729083, -111.08962916641603, -110.52132608161017, -110.53757698855654, -111.5587344449704, -109.77722315102946, -110.40060629757771, -109.45395807961631, -108.77558572395142, -109.0151938598724, -109.80739619986889, -108.9332873172888, -112.49933978358132, -111.28667321897437, -110.40629082858706, -109.9829216820938, -108.85102919990373, -110.84179127037925, -110.27309817549309, -109.88857884367955, -112.24517967927224, -110.23377125710859, -111.26951227953063, -110.09782138347559, -109.77508406986834, -110.55359722398646, -110.09534729906368, -109.96333904888587, -110.29372855476366, -111.36651812163072, -109.97141184588116, -110.16701683369045, -112.8562627359291, -110.66651146857079, -108.78873821095968, -108.59208174618087, -110.31784275318834, -109.43177042415276, -112.80272887161644, -111.79874205007107, -111.08216899537892, -110.73699224045636, -111.04738767291953, -110.43395896705012, -111.62106163510778, -111.32599933330843, -110.29360981749807, -109.66562228449096, -109.21316193790335, -110.06363162177448, -110.54480468587292, -109.31791670875509, -112.65386492377107, -109.91857609999171, -110.57233605624137, -110.7597333064856, -111.49767138733276, -109.36548654843229, -112.34145274183716, -110.52831153822652, -111.55802243871352, -111.81399803046556, -110.17680125962372, -111.23811621944807, -110.48042049674514, -112.43786993562033, -109.56507357271987, -110.67030752598993, -110.86377249100713, -109.06001892813467, -111.37023727930494, -109.52881096984436, -112.95107295160436, -110.49467818026214, -109.29804210589607, -109.89270706931751, -109.46354468058833, -112.10350702955014, -111.06083529077077, -110.49996587015904, -111.1617248913634, -108.84725633199014, -111.42852695852422, -110.01433866707184, -109.11616968390972, -110.76961079765468, -111.80403513904453, -109.84442686379181, -109.65447921666167, -111.3378640555306, -110.8882647652338, -112.58014202075226, -109.67128881545659, -111.73429980763389, -110.82258070774773, -110.71895931098041, -112.5117489008152, -109.16182299471309, -109.71651258790612, -109.7770618808562, -111.94294809571427, -111.1629115541574, -109.57489224865171, -109.8402445779754, -111.17931450307283, -110.09045865447595, -109.23658206733491, -112.54929616847242, -110.5150381158864, -111.32296447909377, -111.64472156295191, -111.65832771066007, -111.03359562742956, -110.85303206770837, -110.80655337650862, -109.3712696310075, -110.57313454785879, -111.18525355670417, -111.67423695430561, -112.00829831274282, -111.08915434609605, -110.3298290221436, -108.68552957386795, -112.11377370993225, -110.80288297661977, -110.33640536217185, -109.5907971201988, -107.9195263775506, -108.50223113159429, -111.91191347156142, -110.29585599512956, -109.50902788911351, -110.76819145749467, -108.86899533416589, -112.09963049260891, -110.13374376572433, -110.15881393584463, -110.87392107947531, -109.18658540731009, -109.72734703956934, -110.18732487568724, -108.76554115185057, -109.94122289815374, -110.39583285609643, -111.09540935727229, -110.6618176357367, -111.6281345666718, -109.69686483639367, -110.31633402076315, -110.61246951748903, -111.73300235294965, -111.34221378834899, -109.46708370903485, -110.70412671997354, -110.7007891485379, -110.31685483435038, -111.03016917417074, -110.94517365625376, -109.46580797053619, -111.20935248224806, -109.20661126636224, -109.50147037097533, -110.14241781654353, -109.8510950344643, -111.3794198224028, -111.28966889207122, -110.43347441663424, -109.86759980279523, -111.92101892013198, -109.31594011390644, -112.92253433794441, -110.74000829597605, -110.3690783911604, -111.9386136764295, -111.04196305034188, -110.41800427558245, -110.94287511448232, -111.66035388807579, -107.53723747644062, -110.68014818358719, -111.86628806511304, -110.12097497430523, -109.69880468221378, -111.4312783987915, -109.18240866486639, -111.45649839248873, -110.1242345454651, -113.75911576151633, -112.71747598882953, -110.9614554157337, -110.92294419716129, -110.87229098694876, -111.09943759113875, -109.48107247947176, -108.62783006742795, -110.8108025857779, -111.63342408317932, -112.0221522906341, -109.96411229549527, -111.29821085030613, -110.04566676239914, -108.41674583097112, -107.50256474992416, -108.68086611003493, -110.3738906060137, -108.86763212826641, -109.81681043446049, -111.04539822346567, -111.73290882980949, -109.75238769150758, -110.55268275367449, -110.48423701377924, -112.1116140908134, -109.53952175199518, -108.538611608547, -111.3788321484912, -110.36378736224961, -110.37712171023523, -109.82150687920334, -109.17046632238393, -105.1169578108227, -110.84067642540583, -112.91626789016587, -111.32030958133453, -108.93375913686056, -112.44450956563915, -111.1596840012794, -110.17380444915341, -109.634859036508, -110.68819277718731, -110.0648098825346, -108.87385575091399, -111.99676414571755, -111.32585405719519, -110.59892045991457, -110.32589048340424, -111.1172696292077, -109.79946399891651, -110.10030723919304, -110.71841081343656, -112.23013150012054, -108.94400401141407, -109.71044551701596, -111.77560214164039, -109.68779520039777, -110.96119601299907, -113.66477058855787, -110.17794649102234, -110.30159876509862, -110.11953836266514]}, ...(2 in all)]
  out "FFT 2":cluster{"f0":dbl, "df":dbl, "magnitude":dbl[]}[](graph)=[{"f0"=0.0, "df"=16.666666666666668, "magnitude"=[-324.19011195451765, -78.1272953812706, -85.85545438627958, -89.30587144190069, -92.90590394398903, -93.63083388385274, -91.8644929119412, -95.26924857401164, -97.0710469181336, -98.01148078956652, -99.33043660296804, -95.58776817681839, -99.9570097527269, -101.45494093095093, -101.51838334751548, -101.00386616525799, -103.01963069818913, -103.20223925731209, -103.53783076500916, -103.48065647812659, -103.97797518531912, -104.58942778240602, -104.46991277190502, -104.59813972158683, -104.56685024229951, -104.69893799348945, -105.05669000016238, -106.17061117835001, -106.43303821862656, -107.39468286383597, -106.2899368267905, -105.7863846168199, -105.17170638885071, -104.53818172761852, -106.70340956723133, -106.55444321137247, -106.67654843051936, -107.79888413750199, -107.86424326005849, -106.09722609215336, -107.71648639013972, -107.79500725395155, -106.17330953637067, -105.43663624517525, -108.04970689199158, -109.92106271611999, -106.2505251183406, -110.60221373795562, -107.11377887451098, -108.4126937286195, -108.37794745021417, -113.22457316369011, -106.38281814065472, -107.55385617652075, -108.93026538982782, -106.19334142366085, -108.90462602264525, -107.63084712174981, -109.12192537022624, -107.90627042480016, -109.44472079190832, -108.91731458372392, -105.74102972706788, -105.74407510394178, -107.5989477192235, -106.2838630137392, -107.46190542725505, -107.38881299750702, -109.08024783239452, -104.97871836903269, -106.65424712290651, -107.04966019632134, -106.16202578092883, -102.98374199247179, -99.1568704142098, -87.07383781389657, -96.41471411313154, -102.65176579899618, -107.65674867775193, -102.85397890306213, -107.58658613411464, -104.79044898833125, -106.65282019869865, -108.65027966345534, -109.46169054950127, -108.69969979291741, -110.4048706652988, -108.81020193837274, -109.42808902484134, -108.85398463561398, -108.3849716744813, -109.1844457168716, -109.32787859535676, -111.01992124870878, -106.64843449415699, -108.9926343573667, -111.59837822080355, -110.57121677672183, -111.17280164669164, -110.68901970586144, -111.69013245592781, -109.90200577018311, -109.3554172126163, -110.7515368822992, -109.2863324212524, -109.66209701262974, -108.50795548698007, -110.58126481096504, -112.36093896766921, -109.78612141282203, -108.85120530917233, -109.91424431080952, -109.84698632196245, -110.93960894966105, -109.77214706089354, -110.30762971422381, -108.77791302937449, -110.79522659679036, -108.47242514643455, -111.20629758187835, -109.05996769621125, -111.13574821570619, -107.79388178889101, -111.5768481279296, -110.52058839597171, -111.58729762739313, -108.99000864386126, -111.6585121505227, -110.50715371958135, -108.87151956974363, -110.30486244367107, -108.32392040018144, -108.1769507919999, -110.43198471512189, -109.81454097966842, -110.26717009815644, -110.82924135076777, -110.34103661156989, -110.0692667126265, -109.34555682020833, -109.1694484721415, -109.9940980324044, -110.81940616215803, -108.21162003366862, -107.97087538330561, -107.55312461506225, -110.60339321606872, -110.09004629292225, -109.05860430198882, -113.1412749514818, -109.81628200948371, -108.62343219429849, -109.48172424209761, -110.85978755785311, -109.47778611557064, -108.81728552967951, -107.47864241666747, -107.61735128422292, -109.62511618983821, -110.32417726356636, -108.24287897478176, -108.60460879530194, -110.2181558494026, -107.95550802888957, -110.80234484950323, -111.09955733353904, -109.43923052503506, -108.98949130235951, -110.05778199870154, -110.36224432927585, -108.13523430027999, -110.681114579241, -110.49106131529867, -108.73493328004297, -110.07663907252234, -109.9968931372618, -112.10715231091008, -108.80994125105168, -111.63774865669372, -111.54355694032755, -111.64024217585788, -109.34986300492378, -108.88053713185408, -111.14370830146245, -111.17327416167232, -110.36311492990576, -109.99414559884396, -112.96912007380595, -111.43191437097785, -111.71327312809349, -108.77202323682606, -110.25970374932486, -112.59574277180732, -109.77247894866957, -110.09219852365874, -111.7197662726775, -109.85454092697009, -110.06789440397942, -110.38055758638309, -111.04251386932805, -111.54279434240568, -109.74385329575985, -110.98924544863415, -111.17898077762852, -110.98364252730245, -110.75024385843372, -109.24766708578407, -109.67753987004863, -110.6537235844391, -111.84436313010086, -109.12654337292446, -109.65519521121124, -111.1845162935778, -110.5009101465602, -110.22980642268818, -110.88540043278346, -110.29249073109453, -108.80459864528464, -107.49372141121728, -108.50353962704821, -110.00730069533373, -112.012876492648, -109.01283702976382, -109.07442203290057, -108.2961442983685, -111.60962842680907, -108.84312815413224, -108.6276642979969, -108.75132871638827, -109.30004903844721, -107.20359872252604, -109.12175943862074, -110.43914247337625, -109.55954680842791, -110.37116786618797, -108.55907813251434, -110.19249995041955, -106.95269845697632, -111.07027929458712, -110.1073996792702, -110.61729280468039, -109.6419175310234, -109.47995019876329, -109.66602827275211, -110.01953864498805, -108.45989120418268, -109.79778555296474, -109.94663827736616, -109.52410616839379, -110.58014441463794, -110.09182359045897, -111.0487262011397, -110.49609187214915, -110.6114701312941, -111.17752423063314, -109.74965389041003, -108.58973724447526, -108.84292130035902, -108.90689510645983, -110.69840140049361, -111.30494362640982, -111.00224390075273, -110.50848328538423, -111.59232911931113, -109.30826761863756, -108.44510893127558, -109.63744704504391, -108.95037574307332, -111.36486409910674, -112.74508631930381, -111.03952454593811, -110.57133212903979, -110.59969855145111, -108.25570461975128, -110.44617635200193, -110.32190307214704, -110.95204704643322, -112.0595421753479, -110.45342552693265, -112.50183987758867, -110.08217804938009, -108.90353583389084, -107.02032313792242, -88.3334978919524, -107.92027625495886, -109.83148570028482, -110.30427997450572, -110.92855407802753, -109.67404674397338, -111.03606345823586, -110.58277018943096, -109.77692362669393, -109.39170901729935, -110.20711662408928, -109.41601946806779, -110.34213214925832, -111.2283900972803, -111.51682597931386, -110.47069117801351, -110.93808974285523, -111.11277478000933, -112.50698886748012, -112.12918507523611, -110.46316790252011, -109.9387334819968, -109.78723249688426, -107.13037722044297, -108.16132376075751, -109.07255491017162, -108.85068428558272, -110.28038153100799, -107.77611023481016, -110.69754506886444, -110.09495581837979, -109.21214884561816, -112.62718526248648, -109.22048725312992, -109.17793923163308, -110.87372121410577, -109.71902632604333, -112.61041177225496, -109.6374750969677, -110.74738952366951, -108.93404661877067, -109.84938675700889, -112.25316361679832, -110.30788094875312, -109.26929069321925, -111.20853536783942, -110.05212566057608, -111.72448131932816, -111.55474439772887, -111.81988954424324, -108.44452452934028, -109.21897824914645, -109.55634869894358, -111.36318572800242, -110.05777399011298, -109.64458567712875, -108.73315084760529, -108.93332091319675, -108.4816455312154, -108.80120578498936, -108.1804470361839, -109.7177707524778, -109.31977709844544, -109.33603116022124, -111.46120546572519, -111.7480378245176, -109.17907150677627, -110.47970652472505, -109.73718750984082, -109.7935026884937, -110.40458408612054, -110.91781389491092, -108.39352075861481, -108.27512197925346, -109.59155075404814, -110.40183121737397, -109.25423373270381, -108.37769008625712, -107.91335995938509, -109.5576520703013, -107.27392145737491, -110.98592762117059, -108.41809950647861, -111.48163889400448, -109.70961684769624, -109.22952568656495, -109.76504719131209, -108.86928627177666, -107.97855299877004, -109.8412204399902, -109.6690048999326, -112.28329030175193, -111.54977099314607, -109.55689540119126, -107.93716711232997, -109.84247640855929, -111.5098351445789, -109.14317615215809, -110.28319116384824, -110.57901069942578, -107.2890252845352, -109.66754569546274, -110.15708115946433, -108.83782190109405, -111.60783857760667, -111.46884385151185, -109.21985333366634, -109.63605494317056, -110.87999187262697, -112.26992029775087, -111.05491095860552, -109.22795442529183, -108.99135781712076, -110.46475190704264, -109.35746113713218, -109.29125989270668, -107.40922407684049, -109.24391685563656, -110.41554602144217, -110.68952735085914, -110.62457364102458, -110.39856310555466, -108.84256124354566, -110.01614601335088, -109.8071306678428, -110.2804500736802, -108.76205061238203, -110.3962440297242, -108.98253716257014, -109.32990745926702, -111.17276766165281, -110.41113652364085, -110.36616199963426, -112.09767002991742, -108.43599666470733, -110.91876588140981, -109.05329272502944, -107.07198690769708, -108.72934463903034, -108.6666471996132, -108.97529973794413, -109.68895260146817, -109.2658844652487, -109.75690097249196, -109.38585024123027, -110.17593039468063, -107.87223111061134, -108.15261097418302, -110.09277437980633, -110.8665497655964, -108.43061614348413, -110.3052458526819, -109.22446919161898, -110.51909692711594, -110.06620699121913, -109.53439413051383, -110.31952463872884, -111.4732125902982, -110.41443606663168, -109.9579358088152, -109.930778061577, -108.5473214465574, -109.34719220288939, -109.16964653934396, -110.04824158176345, -109.42616539603762, -108.3556027482992, -110.62331917617789, -111.3652147859356, -110.12362012120938, -110.13175448595814, -111.20110099151856, -111.50643914621541, -108.11659117128028, -111.06037600347967, -109.03822892917451, -108.25678204604324, -110.82608024151122, -109.15887945314851, -109.88255674562845, -111.18322672526185, -110.95836040044516, -107.91535345885436, -110.66285812468733, -109.61906549925033, -109.58059721670746, -109.65198009505977, -109.65950565672951, -108.95264505276342, -109.23343669003113, -110.74308548011575, -106.39170014998685, -109.61471203101753, -108.24258770956924, -109.84609566640096, -107.83834185503922, -108.93052854090027, -107.55568820082641, -109.758551082242, -110.65892780872205, -111.99907420485852, -110.71043004141137, -110.62257237494617, -109.15610413532767, -106.87403836327807, -108.19175324576331, -110.27819583792918, -110.23918003777561, -108.29703377268754, -110.07182881114713, -109.60256111108491, -111.00394752430006, -110.30750337485472, -108.78309624082331, -109.24103013025798, -108.76979253891403, -109.91618737478264, -108.83915940855513, -110.92536150834754, -109.72250903746432, -108.96533939688658, -111.08949280651164, -109.20335070860871, -109.37826578362439, -109.77953166722301, -110.1867310744785, -110.07114559821346, -110.7003631567182, -107.86455899696074, -108.94113264174617, -109.35999427135138, -109.33627364788704, -108.96588828808375, -109.08716536982254, -108.73575375369026, -109.47770132070654, -109.83726171472907, -110.73516506891792, -110.56827134787686, -107.65667508354096, -109.30200115708924, -109.28406803847896, -110.55374624323233, -111.2017766725333, -108.50851279608973, -109.79494403619485, -109.08320018013063, -110.21850624918747, -108.4652936555984, -108.74837610538873, -108.81326140648238, -108.83830180036702, -108.785270477003, -110.01845876259073, -108.76030368637825, -108.57879884880157, -110.6610608456059, -108.74669367794318, -111.55956030460833, -110.22906685783455, -110.48411613865359, -109.48060880085136, -112.77556331479562, -108.2676071206087, -108.8571136162698, -108.56944905160177, -109.16406757131058, -111.42259299295839, -108.25216316582294, -110.48487127684025, -109.69532331373831, -108.13992755196784, -109.2987762526628, -109.82536192480795, -111.28650061088359, -109.12820736404241, -109.37960655471406, -108.96014976926716, -107.97535047619023, -112.31953123574708, -109.06198330523004, -107.52722515967098, -107.31555373665437, -99.89671790804692, -107.44442600896275, -110.6549218761941, -108.02265794322076, -109.63582761762919, -110.00574746987859, -109.51565124961209, -109.3550083591902, -110.4541529175301, -107.85799722437162, -105.1197113090786, -110.25038075579738, -110.39710812865657, -109.3618876098789, -107.6131301952152, -109.21529527621463, -108.7995754403799, -108.48347353145697, -106.45678488065816, -109.60427918561142, -110.81194387812535, -109.52215044127382, -109.88751598659705, -109.30205143590227, -110.74984456751768, -109.03952092986351, -110.69170786328897, -110.39236248162467, -108.65456161733339, -107.60439764386904, -109.97367926606955, -110.2754359970249, -108.81546418006434, -106.99691398176165, -108.42047325825182, -107.24499915944605, -109.28116135603187, -108.70650358781573, -108.05516916105047, -107.20893100196241, -112.07029265690055, -109.38099990478445, -111.53461820465232, -108.11312509555277, -108.76714028655223, -109.89565008459624, -107.71879172001115, -108.08434857420214, -108.79142773619792, -107.25153085963885, -110.05595039449301, -109.31604222314259, -109.94405791565286, -109.04715370361387, -108.89278831045846, -108.84682466376424, -110.0067927716526, -107.63768959294084, -108.98109382020348, -111.4720219575084, -110.76023788797733, -108.78599647633777, -106.59726674064618, -108.66715709719243, -107.99134359630926, -110.11396713841884, -107.21091759882775, -108.08576824949941, -108.80217666857972, -111.72949572713338, -107.33126296136014, -107.33731660097102, -108.04470462977443, -109.42963925921418, -111.03517778720736, -109.55293581015796, -107.99948151285162, -106.59480934999681, -107.63777243313498, -108.96490626068824, -108.8948210299064, -108.30870516747477, -109.13612869658097, -109.59971429402015, -110.2571461001396, -108.7655464686992, -109.81144209568883, -109.80796806645141, -109.20948481699544, -108.68653880881129, -109.26329796696166, -109.22428132233863, -110.12571678351438, -109.14615461144786, -107.08261621308327, -109.11338327144382, -107.75421565039201, -107.45291780756361, -109.00477000647248, -107.41031480478154, -109.98948062864928, -107.45953654921264, -106.37522884807879, -107.7786128523167, -108.03610987358499, -108.05926797128022, -108.59400205554164, -109.89620453365603, -109.03811240487515, -109.96909236705363, -109.28212981785472, -109.6772152101994, -108.26493868190678, -110.55558039199732, -106.6252818398841, -110.19075011176416, -109.56520012524705, -109.8023423576176, -111.2697570480663, -108.26752571816566, -112.00337375484828, -109.85709226796116, -109.36922081321148, -108.8424844298318, -111.2512302139209, -110.61775974680471, -110.22501328999012, -107.76874906708105, -110.71023653476604, -109.4025656165291, -107.66667684986125, -107.59759854092948, -107.94763263251238, -107.3888591871119, -108.62692803125044, -109.18012867988286, -107.78662871481455, -108.5072814073944, -109.50348958982907, -109.95177634938378, -107.78756251182895, -108.03865042797304, -110.1814993556385, -109.34937567548833, -109.52162025123161, -109.50819015441117, -108.20953105254624, -110.52154040214435, -109.3324404469266, -109.2696617050831, -109.54675609195674, -108.5940367000989, -109.40184828664549, -108.2518305610941, -108.55972691669434, -109.03647225394408, -108.48166656251695, -107.42023429066523, -109.42453054302521, -110.09532345960083, -108.78315822119662, -109.97508586102265, -108.22687406536997, -109.17110028890058, -110.15390449992647, -107.88577458651508, -108.28851074361447, -108.52030295163331, -110.03496861709483, -109.40014319167584, -107.73048113044877, -108.17571683963915, -110.34839852994926, -108.55894048192191, -108.74107339998285, -111.17734138993401, -110.22946440841412, -109.45511941802884, -108.0657300641843, -109.33797363184166, -106.95974095511333, -107.93068343723691, -109.78867669512647, -107.2087297624043, -109.542665021243, -110.05035859052961, -110.30235238883523, -109.20586170783808, -109.2796396673401, -109.14260673746566, -108.22019460542734, -109.99011886871159, -109.89103038547285, -110.36964772493243, -108.62340319923602, -109.06779821699769, -109.21830861066148, -107.7402395759509, -107.7178850938205, -113.45665085929117, -109.24039191621704, -109.30387033426037, -107.61849760982835, -109.41430582703529, -109.11482836392241, -111.89328423764577, -111.84653367963301, -109.00674896486915, -109.84488648739638, -109.41914760797953, -108.53442910169935, -109.66883322968232, -107.68762956301386, -109.82583101109167, -107.83405397804887, -108.78052031141966, -107.37842078941692, -105.40843158543845, -108.81430898189338, -109.57374640194516, -109.41111270322058, -108.82621700188898, -110.2552502368822, -110.23903890097205, -110.52171662278697, -108.21249857906324, -109.97268479379733, -108.20088823960992, -108.85682002802234, -110.11642849164285, -109.94087886999255, -111.63180946270296, -108.20899499456195, -106.73341567332112, -109.90003508676807, -110.14688274481229, -109.62259307329889, -107.57811196819495, -106.88584597822792, -109.16132624528932, -109.78677836397806, -108.59319344451784, -108.55877448618652, -109.46883711353044, -108.47309455543844, -108.09487065732198, -109.82219079158135, -109.63780237877428, -109.28348848877269, -107.62893405379826, -109.46986737961593, -108.03089712610223, -110.3931917410696, -106.06970126043262, -109.41866550703786, -105.31710372440419, -109.20218082282653, -108.28467118008108, -108.80026326744611, -107.40729224715713, -111.07322915141532, -107.1057186510818, -107.98286374205958, -108.51298722989311, -108.69632670891366, -107.96509231988331, -108.15882223414738, -106.85862416470376, -109.70705792539056, -108.64519930633055, -106.78708421443504, -109.43552377900174, -109.4474526498122, -109.10135248755788, -111.43316642580763, -109.33457343739448, -110.23547887071898, -108.95690647379442, -109.21159903769149, -108.12969562680841, -110.82751409340537, -108.55724349027832, -109.8796329603075, -108.50369978374582, -107.43145467247209, -108.60003323209516, -108.77155705999647, -109.33806063660796, -108.37500858898439, -109.65641721611547, -109.81905873737344, -108.03483220769625, -110.48028107566635, -108.60527372219985, -109.28768201151478, -99.8804125587218, -108.8913334544964, -108.23534920737794, -111.07646463287153, -108.59029790589766, -110.3405916586831, -107.66387718565608, -108.73793152614131, -110.61440166477816, -108.76211382544581, -110.23236978486065, -109.10669297094852, -109.15247609779597, -109.00539004923506, -110.14424353412238, -110.55445060661157, -109.48721312920799, -108.17040942305823, -108.77592227268228, -108.77130256578067, -107.82494496098512, -109.57266989523707, -108.75767497229612, -108.13688624150026, -107.8280716764963, -105.676279602552, -107.6370316684844, -109.73508547021689, -109.25365178573009, -108.86767843317584, -109.70969944273735, -108.91917504090888, -109.97734866522867, -112.17308993943783, -110.28356299479682, -110.7927103729386, -110.30837645846702, -107.56364161860179, -109.50188349731121, -109.36065627483853, -109.75389877587511, -109.81713476007774, -108.14524057525358, -109.43832376796216, -110.89342891210596, -108.15657882822792, -106.84106061627887, -107.83091759905821, -108.61794662682962, -109.57142366843581, -109.85402645528154, -110.12877022469837, -109.19414429724044, -110.56168468006764, -108.74720588273881, -107.90448559921305, -108.54421401507743, -105.06700039841249, -109.17937358052484, -108.94317576365822, -107.79410219455083, -109.24955437598658, -108.23334395173994, -108.98759227946937, -107.05986359444529, -107.20956512998849, -109.00295831471958, -109.43119556916457, -108.93348410522628, -108.99932477701081, -106.6448790859128, -109.06877251308666, -107.67053918439544, -109.15052780608639, -110.16878033319385, -106.55101141640301, -108.02811045752685, -111.52173447126572, -110.16854119242062, -110.93164036911654, -111.25979320890855, -108.82629030379024, -108.52004501839738, -107.09697056562636, -108.94233383169858, -107.37962568194772, -109.1239201710643, -108.93949898577122, -110.62573772949195, -110.09592372075662, -107.56136391005947, -110.45600430869621, -108.79481000016084, -109.41462449554598, -109.30248158488335, -108.70735295493108, -109.9174743694956, -109.94232543385962, -110.71725446170196, -110.0346196158573, -110.34814317845934, -110.6651078322521, -107.55409880424479, -108.71734776861287, -109.50902203986271, -110.40207542979611, -108.7847687630861, -111.10599488129682, -109.30824728923263, -108.20134064331717, -110.55959112431609, -107.77099734327174, -110.23862843385446, -108.48520797666865, -108.54205896654946, -107.79288769037599, -109.84022250170581, -108.02758364115576, -109.35132492327935, -108.87009749667932, -109.86905123364855, -109.19826752168308, -106.835240323691, -109.37910022114056, -110.80633973102931, -109.12703823829597, -111.07432699570984, -111.8064506085314, -110.09349947650527, -108.66467295777367, -108.75119108236053, -112.63983351316729, -110.90940743670113, -110.27973159222081, -109.57141664526549, -108.61645363771719, -109.31742355616147, -109.5839599160637, -110.01188998365383, -110.01923429741011, -108.94779759137936, -108.26169431000017, -109.24553201026085, -109.95709526422822, -110.68677343596859, -108.7678734483002, -110.47090469179284, -110.31604700116512, -110.10256600741997, -109.76634647265719, -110.8830805828562, -109.94609564072982, -109.20662382740542, -108.12492970530919, -110.5274435478767, -108.02351960398035, -110.6264936805739, -107.14559226383577, -109.13821777857531, -111.05324489472586, -110.15190797512811, -107.96366234783144, -110.03950681967147, -109.17476300510336, -110.41251816187909, -111.39219865477246, -111.32530426869943, -109.97369363558423, -108.98666403063845, -109.62049358645565, -109.58130494498671, -111.72738873188874, -110.39825891106616, -108.57430325757545, -111.28625510212446, -108.77421250595326, -109.75025415031793, -109.51948456745635, -108.82129398637998, -109.81362137198361, -107.86292494316123, -107.49318292857053, -109.66948564589373, -109.54288390056654, -107.99912445612077, -110.3497559614379, -108.00549349666127, -110.01361420523357, -108.4977916421456, -109.67078387286976, -109.85678367732866, -112.01237658746248, -108.4855625950998, -110.84880875737286, -110.9178674382154, -110.44187536727453, -108.75076921971127, -110.04946286646651, -109.99780941000827, -110.14242932305507, -109.56343773672316, -109.6278993388131, -108.77419573790174, -109.10543670530926, -109.7801848627463, -110.30733124104881, -113.13440550301436, -109.32709134514755, -109.74136656933283, -110.01525283266193, -109.43924662938396, -110.25325289253, -107.75460576671303, -110.60057027395933, -110.71458404922404, -110.15788509050662, -110.69167485018224, -110.96006652476157, -111.01156633983031, -111.6058448010008, -109.51364005052672, -109.76058205940885, -108.43421621088261, -109.47973949170208, -109.25533250208288, -109.47422603921065, -111.36411644613841, -107.27566171102698, -110.45098686173688, -109.93589296291184, -109.03803734663714, -110.53118128434016, -110.2408872254969, -110.0532234862915, -109.94185495614619, -110.2662004220774, -109.51094016962288, -108.5210104215432, -108.13691752270934, -110.18460088390265, -108.32609309150783, -109.89652230508281, -109.80923900768477, -109.01917388968883, -110.01248300968739, -109.43415605440147, -108.09823485138017, -107.40637725320931, -109.40632232658412, -111.97981999127656, -111.16609811629485, -111.64500793960192, -110.99793748693381, -109.55531276386903, -110.2535662621666, -108.17429802469516, -109.09425673355422, -110.23187110421917, -110.55358397926925, -109.93461124753053, -109.55604345832225, -109.44569510408274, -109.72185151080762, -109.52963702944834, -109.2303630328152, -109.74819502244243, -109.3932530349457, -109.17096788339686, -110.46153727064616, -113.1073731246639, -109.43753070459397, -108.13332547768168, -109.42294574929969, -108.45798401969856, -110.29453435046327, -112.66249403705643, -108.78314667434937, -105.9634478773668, -109.14327524669528, -108.50645190860273, -100.81571594994128, -104.4482859840643, -110.68926237051092, -109.12362553230196, -109.45234390564677, -107.91461416156068, -110.67788819353727, -110.05744935668449, -111.78333392154664, -106.83628914455993, -110.11115457346548, -109.13434608275826, -110.80006861194663, -110.35323502651462, -112.29149906501372, -109.01656376530778, -109.30871662948859, -109.79736315392456, -109.17848983603582, -108.09752397056482, -111.6039030763455, -109.27008844877828, -110.84475733314184, -109.72393917557073, -111.31060762894991, -110.78858793807466, -107.12841545099752, -109.54510865218204, -105.2805426080281, -106.28514149354733, -109.50656759582803, -110.14700878401054, -110.49737016725709, -109.19811547071924, -109.92527399676051, -110.7961615015146, -109.7447227818197, -109.49432012009893, -108.714081576733, -110.09766801550917, -109.08448507943001, -110.36154838733857, -109.86328656267403, -109.21144237434696, -112.4145136888034, -108.57567151011159, -109.66748589540896, -109.72985837578446, -109.29989238126763, -109.85868902806475, -111.01778182304162, -111.23625326328558, -110.01270868104203, -109.27067928081415, -109.71171312410247, -109.28697459293629, -110.67868067201007, -110.91353786857455, -111.21479955051575, -109.11315965407708, -109.40418681804496, -107.80511819596003, -107.37201025889816, -111.81969609169838, -109.89875624306032, -110.29328043898657, -109.74853280072202, -111.39527865400605, -109.47746221101964, -111.75141177452517, -109.31325306583483, -109.30117448911659, -109.3997781364162, -109.45356931295724, -109.60585285774386, -111.33951689512735, -107.74187210470228, -109.62706021606415, -108.72139655505221, -109.79552836110567, -110.64354037499807, -110.96138240913136, -110.02215059889615, -110.92978442698893, -110.0620778287114, -110.85019647293322, -111.77397403227091, -109.81257196800128, -109.15643451383403, -110.72777566469594, -108.7463769025616, -109.80959395914073, -111.24500986151126, -110.48863498350322, -110.30863780110901, -109.79331354195703, -110.34087081762074, -109.45183222569266, -109.6440990067103, -111.15034876658994, -112.14912485578341, -111.8886180186196, -110.57054820211916, -111.07556239924551, -110.5872832735073, -110.28912501038172, -108.91501133754849, -111.44575118962761, -109.90799859177967, -109.74421995550023, -108.70941446115883, -110.28822893097275, -109.70039554000401, -110.33701797570251, -110.79445894683306, -109.57694314608153, -108.816904416038, -109.66517126767175, -109.39501469321644, -110.85775022889956, -109.3689402795614, -112.09107318723095, -110.67985626248422, -110.32971146814747, -112.08166943494875, -109.93955548712543, -109.31722953035252, -110.2062913031861, -108.22565380081006, -110.680898028151, -111.95386604441454, -110.83354130587097, -108.5873626748948, -111.97536144124408, -109.23944159551515, -111.57859477689586, -110.80135186615524, -110.4800953731021, -110.14040729648133, -109.25873050390551, -108.87000960474569, -110.97091597211167, -110.15787270199012, -111.62434537618091, -108.5421625277294, -110.42258666403919, -110.96896115868603, -108.98253068925274, -109.54245055160168, -110.28051096122468, -109.48060498658319, -109.77618362117276, -111.64513838754992, -111.13945484239875, -110.18094280356001, -110.43757222770748, -110.81588360154201, -110.11656805555333, -108.47936291282355, -109.16476249859961, -109.3549985917136, -110.77753190334253, -111.46065694661178, -110.40387985996301, -109.95673803226478, -111.58660981285446, -108.59894875229345, -109.37333363882607, -110.26849699991793, -109.30500469266264, -109.23789020998296, -110.82000706486865, -109.25927538839868, -111.03285659417519, -111.08899832832414, -110.69361682858042, -109.45187168573815, -109.9614018482838, -109.70209527974106, -112.11903952100165, -109.59713611623246, -110.70292028698111, -110.12743849746808, -110.63315585514292, -108.60450276298175, -109.32832664986026, -109.99753023477764, -109.46644696130294, -109.1781290160558, -111.58830180575129, -111.67229040267557, -111.3750024136205, -108.33616679452298, -109.99797067800029, -110.50892429124391, -108.66074740829372, -111.17094662568759, -109.87538933985836, -109.152526628291, -110.44623159817101, -110.21603106403009, -110.64376935639365, -109.36897426842583, -108.67303022227141, -109.89327693080823, -111.50442955563923, -111.37532237834381, -109.38132821290205, -109.73509680539144, -110.53918379735906, -111.22869870340647, -109.39977573957616, -110.3674665334106, -110.5366125953241, -109.99025356764304, -109.97300035646616, -109.87631077033762, -109.64608829594286, -113.02486102973394, -108.26250283140733, -109.62234918138763, -111.18766216512655, -110.33666026406992, -110.5808115327039, -108.2971671321189, -110.10964334161903, -110.61254021379767, -109.89852549557533, -110.16562049054073, -109.41433790018287, -111.2453823439446, -110.45554802599901, -113.11454453784393, -110.7333866145056, -110.00858191882439, -108.54745315874294, -110.08430415376903, -111.9006972727596, -110.3031506154679, -110.26331790366497, -109.36797925566673, -109.04860552478912, -111.83514212681175, -111.38960737633833, -109.01429665187288, -110.96404839103826, -108.95488871107163, -109.09652004914592, -111.884304581971, -110.57566691021339, -111.95113404442795, -110.13677174050159, -108.10078686353354, -107.69442565416006, -112.42676605669463, -109.12681161784135, -109.23120766087519, -110.57649395555585, -110.22143082743162, -108.40065951773644, -109.46923168308618, -111.39095086729745, -110.46375658526013, -111.45145283328486, -112.22610823637353, -110.61090190564383, -112.22250292674809, -111.7379343196361, -110.18530386733481, -108.93867365671692, -111.89304844956082, -109.06146134986984, -110.98405731832798, -109.76366821333497, -108.08326795663608, -109.95041147835065, -112.94140614324155, -111.79814935135965, -108.07337559063119, -109.13733403265212, -111.74906646037496, -111.12228668433455, -110.02899450462209, -110.22237716929811, -109.0224776891049, -110.18135850497721, -113.32516073881047, -111.3576490243877, -110.60510094465171, -109.6935518470342, -110.36313473154901, -111.95933240129618, -109.49625308071019, -109.18827910216122, -110.54311407822692, -108.4811035913567, -112.81280225723607, -108.86530665787413, -110.85796435061886, -110.40059714639627, -108.19250716343407, -108.96956521802292, -108.61281798886506, -109.78061525370413, -111.58885511891798, -109.06279169160345, -111.43043988466789, -111.63169336321079, -109.54702536206447, -109.62860636296405, -109.47865811135546, -108.02265793654806, -109.97461304995515, -110.72549884050886, -111.57309413919933, -110.03317891949746, -110.39570411598524, -110.27606115470397, -110.63294457306095, -110.71821689302902, -110.38076268941819, -111.51223508887897, -110.40703572670697, -112.24933273737743, -109.74954300082398, -108.46020292937696, -111.05315219575881, -110.38635148390118, -109.58268303790976, -112.34211536832117, -108.45894118755307, -108.96463982695337, -110.56040438523046, -110.67803313671729, -111.07349872375121, -110.42184162876096, -111.82081126435692, -108.85923651136297, -112.57723799596502, -113.65690874668172, -112.62314325834605, -110.70357529341362, -110.959925221544, -111.26336183001875, -108.1350700630152, -107.94545932312926, -111.17610778209841, -110.20386728310686, -108.55646511121591, -109.8400922569145, -111.73466587035968, -110.47272877573613, -108.33011124048193, -107.93042857580332, -108.60928277989103, -109.25240966798974, -108.96403833602028, -106.94222615757475, -109.37086694261907, -106.72743097285155, -109.03160193412796, -107.3549903889451, -106.8543848510082, -107.83503929060929, -106.30745467433752, -108.36915807168845, -107.13065938379303, -107.84769200880969, -106.08004345082777, -108.15244601930225, -108.37254117816573, -106.57863034819223, -108.1283698227614, -108.19776505569902, -107.58283412238643, -108.17365133196301, -108.6794309781181, -107.91552140588759, -111.60122989270022, -107.04360635941174, -111.55535949001795, -109.39870426166594, -109.55937904851662, -111.81389508925734, -109.88957041098786, -110.84764586896561, -110.59130246272693, -111.15944135223884, -110.19496154041607, -111.51861903129362, -110.74798816525838, -111.37312965175558, -110.10842817220238, -110.73198099204856, -111.36708667993291, -110.30840247819665, -110.11744489669044, -110.55237850846444, -108.2073528237766, -112.70750856801911, -110.99917956040802, -109.84949484779976, -111.3403161887679, -110.08924435263565, -110.17749213365616, -112.10849123224503, -110.94270741299202, -109.29350963424746, -110.33477486966507, -112.19620157705627, -111.45484078395934, -111.86858843505124, -110.22491147345858, -108.96177661263177, -108.67862820579893, -107.55155410582937, -108.27984439169573, -108.72682528077233, -110.64231212183269, -109.32873093119183, -112.98564364754564, -110.78933114228725, -108.50921025910479, -107.91087245586935, -112.57350030929283, -111.75871577457525, -108.42095298945462, -112.31266064114303, -110.1295657579673, -109.67444664474456, -110.33749884929306, -109.16098218724147, -109.63554874360221, -109.15892392675141, -111.90580809179818, -108.81196712336858, -111.42223552606656, -109.90571484965518, -109.99739812086352, -111.64103850263211, -111.31463957090885, -110.61247447444549, -110.20960333715526, -110.1707327818923, -109.70412636554525, -110.97278093107532, -110.24386747740314, -109.81378546061525, -110.83784085086458, -109.77357954318757, -111.22663832948885, -111.14563050139252, -110.87152231402447, -110.34246044319893, -109.97174570657546, -110.23599592972218, -111.08206161770731, -110.0073315341242, -111.11748366902188, -112.04005964728601, -109.81290191679287, -109.68543639040858, -112.01143296194752, -110.13641850530031, -108.19348942447623, -109.7534468948808, -109.36697824644176, -97.56454580435337, -104.97829040517887, -108.1539132982256, -110.048991273122, -107.46172505860011, -110.49269280640675, -109.94209901400029, -109.38576869679022, -111.43699124347364, -110.89973083498887, -111.2994445418276, -109.25144782032437, -113.25676258473536, -110.82078737428088, -109.97779571182073, -113.36294799183014, -111.38584551238931, -112.17267897274873, -108.56430946159155, -112.06841286528645, -110.36822473102735, -109.54758527532016, -110.48190506674653, -110.03535695860182, -109.3951469796576, -112.41910682256774, -111.38124138857238, -109.37850389100952, -111.65544568836181, -111.55876881606889, -109.3029209617236, -109.20030046194076, -108.82610577621037, -110.53329453526098, -109.96090595542142, -109.67834229432077, -110.62303603007352, -109.8388817181171, -109.22430039793213, -108.92749786663613, -110.05794249283548, -109.58534943218437, -110.50493887507297, -109.96373022997366, -111.0645036323456, -111.28501675364454, -109.77386932343008, -108.8952247140968, -110.09242801628717, -112.90943444063141, -110.72299296247249, -109.39094335967056, -110.95165384057718, -109.59809519359453, -110.4978602309597, -109.67109981692639, -111.2489619905986, -110.0937750887109, -109.76771021128954, -108.32976315018955, -111.3058145792439, -111.09464974601362, -110.99797900696136, -109.174315000222, -109.630351559617, -110.26289147175856, -110.22688407202517, -109.96748050100612, -112.13247633583758, -110.59994952890855, -110.93023020153811, -109.22457750926695, -110.26162558926984, -110.09713110375579, -111.73858994918328, -109.78183160058515, -109.7603471824367, -110.96016892586911, -111.23309626937036, -109.83093663960678, -114.05354944347246, -111.58202863059464, -110.42281828744524, -110.9521484732059, -112.5120328206343, -111.614891937737, -109.84428787405484, -111.61119567831453, -110.43095563229411, -111.71833448430398, -110.01132196809407, -109.37558169247951, -109.14091380022785, -110.42663661754088, -110.3598013572826, -109.78207135281417, -109.94058843992468, -109.88210328447205, -108.6217811850147, -107.17834387173707, -110.6447226986756, -111.10704778101115, -111.24396771977769, -110.47849395539598, -110.75150631628034, -109.67662689396347, -109.23145032835053, -108.83780193265358, -109.43468321661163, -102.22521103859944, -106.90009867479111, -108.91580608784525, -109.58671397003187, -110.56692028436989, -108.75103142680105, -111.00795573084157, -110.75039085328763, -109.48222099288613, -111.8621134816908, -110.26507966786443, -108.885924716389, -109.30841399453053, -112.3188631425597, -111.05677697153163, -108.8268571902449, -109.63028152237679, -114.82339015806369, -107.03435216376964, -111.34847692589166, -109.61354114874855, -112.32687758049907, -109.59816404231358, -111.64248480241805, -111.84075757907273, -110.44017657636552, -110.15181635726277, -111.93813663582833, -109.11826378836209, -109.99779889778326, -109.927119030584, -109.4389650887841, -111.52448814187727, -111.38736268499642, -110.51920914917922, -108.64230614681055, -108.90307263595304, -110.57246891832371, -109.65575340646116, -109.80359672370373, -108.83368585528197, -111.09385004343437, -108.83430005497769, -112.37784208819113, -109.50005381621696, -109.67421750136593, -111.39664088797532, -109.70867599669316, -109.52498993629875, -111.12341349673187, -110.0484037026941, -109.55138667646308, -111.06614422098669, -109.4785941493091, -110.25724082617013, -110.93950616855716, -110.53487953881397, -111.45722057988401, -110.32393446412904, -110.34361936710438, -108.6610336097813, -109.53631603696368, -108.06930707969195, -107.68056561368934, -108.73860971027449, -108.87111384617579, -108.40433837098611, -110.55999576884835, -106.83832061167207, -108.28786975902513, -109.18482905697472, -107.81071696594883, -107.91047268802457, -108.79613111673706, -111.05361322310213, -109.97897453479862, -109.12920563729425, -111.20538391490288, -109.26286135293664, -111.31400407177502, -109.92167984752287, -110.70854322826071, -108.59406515713611, -109.69371333227458, -109.36664873267313, -110.35521729513704, -110.40667924006368, -112.0181844636846, -111.01529188207431, -110.59246505728431, -109.95068312717868, -110.75807466894047, -109.58596443762707, -111.12127793384956, -109.59041634463125, -111.56255571372793, -110.43405578864342, -108.39660324329928, -111.1420710307505, -113.64788483868595, -111.67645688353934, -111.36878760365944, -109.68523694561108, -110.11608766310304, -109.25670490330123, -110.73546181099229, -111.77855039399805, -107.9662794718261, -109.67483334602832, -109.891258579519, -110.24757768183042, -109.50202895993814, -110.07763831916637, -109.96891925839451, -110.97268925927641, -109.31698133827767, -112.27933593506792, -110.36206721075725, -109.47379463718867, -110.27836850941338, -110.63738280998388, -111.3611682777485, -110.72689155959884, -111.55480904927032, -111.16689658479412, -110.35555645743601, -111.56609319131051, -110.88279459952174, -114.73607246523177, -109.95813757295693, -107.64639932425493, -111.26486783320321, -112.03946356928121, -111.8915972448334, -110.35245920812773, -110.83155104803564, -110.67437747473863, -110.9959682920065, -110.7815352345103, -111.13722283763049, -112.54797265493127, -110.06894780898469, -111.65186554925783, -111.83545188116254, -110.65894756123697, -108.48458025065264, -112.43760714427981, -114.1368408201927, -110.40065777895025, -110.1066998945526, -108.60654239598591, -110.5716060205154, -110.74257357180736, -111.1136089342442, -111.53539811075092, -113.2559601458872, -109.2003227548348, -110.42285840441025, -111.4086884998834, -111.61503050693868, -110.8194303494779, -108.9701587059964, -112.58521089509063, -110.10873915265242, -112.43440038319561, -110.03468788439882, -111.57896603236308, -110.21939233582523, -109.03614470500777, -110.11738923539659, -109.55359574898291, -110.416473622654, -109.4626868574157, -111.17164025076731, -110.3579689035081, -109.04338716157822, -112.36157114517567, -109.32125615922843, -112.71105693789394, -110.11019129547768, -108.96439402555632, -111.107663418839, -111.48306369859839, -110.9317530461794, -107.98628540532181, -111.1636972328743, -110.47837837583148, -109.04649309175733, -110.27110334963734, -111.35803630614352, -110.77259078859605, -111.46352820533895, -111.16789261049541, -109.2376344776325, -111.6795794983659, -111.74292205167644, -109.40835022991612, -111.02163652600731, -108.79482078001607, -110.6718658416566, -111.08747067599332, -112.15383726791498, -109.47049126158717, -109.061574046483, -111.23993049318979, -111.02521156588335, -109.46012868444186, -110.13918914826291, -112.08180381836377, -110.61929875223015, -111.4424805369965, -111.43420275069585, -109.71347556238717, -110.24726273025648, -109.7860268673935, -109.94126895018422, -111.41948668868926, -108.90555991781676, -110.81242861886172, -109.65007052722677, -112.12672329335953, -110.01123170946096, -111.13980448279096, -113.92013682657084, -108.6000853867411, -110.66793592761913, -110.61237681642844, -110.00839105230496, -109.38083187034974, -109.46119372195675, -110.3708067287448, -108.55518656223285, -113.33935987443276, -111.92184778392033, -111.80820718236087, -107.36852757311246, -109.51077803361602, -110.066791721019, -108.756710558672, -107.91391289865918, -110.72851430959301, -111.39074956442978, -112.928843679455, -109.87348280521556, -112.21371750380071, -110.82495902297394, -109.94006136010094, -110.58757785050143, -110.2790091349881, -111.43884888223081, -108.09540986530712, -109.63783244641691, -110.19577975613292, -110.01690033746098, -112.75938920157155, -109.27158857362184, -111.19519821680541, -110.14381902425255, -110.45955291199236, -111.55660330002316, -110.75604254261134, -111.02122553784838, -111.6490091060193, -110.93362819419399, -110.49033159684308, -110.70789549836027, -110.41991882034145, -110.0264093421208, -109.18432746063652, -110.15292268755287, -112.40733942236504, -111.32869665965416, -110.95418667871114, -111.14291568823575, -111.75555369152653, -112.98146297069803, -109.73870744292117, -111.33806139459435, -110.18838799491355, -112.60408243005732, -110.26112648646833, -110.58257045107274, -109.75155437454112]}, ...(2 in all)]
  in  "FFT 1 Choice 1":u16(ring) items=["T1 Y", "T1 X", "T1 Sum", "T2 Y", "T2 X", "T2 Sum", "T1 FB X", "T1 FB Sum", "T2 FB X", "T2 FB Sum", "PSD Y", "PSD X", "PSD Y Sum", "none"]
  in  "FFT 2 Choice 1":u16(ring)=3 items=["T1 Y", "T1 X", "T1 Sum", "T2 Y", "T2 X", "T2 Sum", "T1 FB X", "T1 FB Sum", "T2 FB X", "T2 FB Sum", "PSD Y", "PSD X", "PSD Y Sum", "none"]
  in  "FFT 1 Choice 2":u16(ring)=1 items=["T1 Y", "T1 X", "T1 Sum", "T2 Y", "T2 X", "T2 Sum", "T1 FB X", "T1 FB Sum", "T2 FB X", "T2 FB Sum", "PSD Y", "PSD X", "PSD Y Sum", "none"]
  in  "FFT 2 Choice 2":u16(ring)=4 items=["T1 Y", "T1 X", "T1 Sum", "T2 Y", "T2 X", "T2 Sum", "T1 FB X", "T1 FB Sum", "T2 FB X", "T2 FB Sum", "PSD Y", "PSD X", "PSD Y Sum", "none"]
  in  "Compute FFT":bool
  in  "Reset FFT":bool
  in  "# Spectra to Ave.":dbl=25.0
  out "Ave. Time (s)":dbl=1.5
  out "1 Channel":waveform(dbl)(graph)={"t0"=timestamp(0 s since 1904-01-01), "dt"=1.4999999999999999e-05, "Y"=array[20000 elements], "attributes"=variant("NI_ChannelName"=variant(string "T1 Y"))}
  out "Slow mean":dbl=nan format="%0.2f"
  in  "Slow mean N ave.":dbl=1.0 min=1.0 step=1.0
  out "Mean Intensity":dbl=nan
  out "Sigma":dbl=nan
  out "Sigma/Mean":dbl=nan
  in  "Subtract mean":bool
  in  "High Res. Display":u16(ring) items=["T1 Y", "T1 X", "T1 Sum", "T2 Y", "T2 X", "T2 Sum", "T1 FB X", "T1 FB Sum", "T2 FB X", "T2 FB Sum", "PSD Y", "PSD X", "PSD Y Sum"]
  out "APD 1 Rate (Hz)":dbl format="%#_3p"
  out "Stage Moving":bool
  in  "Read Cal":bool
  in  "Confocal Linescan":bool
  in  "Speed (nm/s)":dbl=100.0
  in  "Furthest Withdraw (MHz)":dbl=15.0
  in  "Confocal Image":bool
  in  "Round T1 X":bool caption="Round"
  in  "T1 offset_x (mV)":dbl=nan format="%#_2g"
  in  "T1 kappa_x (pN/nm)":dbl=nan min=0.0 step=0.001 format="%#_2g"
  out "Time (s)":dbl=6.12
  out "Total Time (s)":dbl=60.0
  in  "Start Saving":bool
  in  "Cal sets to save":u32=50 min=1 step=1
  in  "Comment (data description)":string="testing confocal setup"
  out "Calibrating Trap...":bool
  in  "Trap 2 (ON/OFF)":bool=TRUE
  in  "Trap 1 (ON/OFF)":bool=TRUE
  in  "Save Calibration":bool
  in  "N sets to save":u32=200 caption="N Sets"
  in  "Save N Sets":bool
  out "Save file name":path=path "C:/Data/110526/110526_022.dat"
  in  "Save ave N":dbl=500.0 caption="Averaging Factor"
  out "Saving...":bool
  in  "Stop Saving":bool
  out "Progress":u16(slide) scale=0.0..100.0
  out "Manipulating Trap":bool
  out "Buffer Status":dbl(slide) scale=0.0..1.0
  out "Overflow (data lost)":bool
  in  "Reset":bool
  out "Data Rate (Hz)":dbl=66666.66666666667 caption="Trap Data Rate (Hz)" format="%#_3p"
  out "Data Period (s)":dbl=1.4999999999999999e-05 caption="Trap Data Period (s)" format="%#_6p"
  out "Save Data Rate (Hz)":dbl=133.33333333333334 caption="Rate (Hz)" format="%#_6p"
  out "Save Data Period (s)":dbl=0.0075 caption="Period (s)" format="%#_6p"
  in  "T1 alpha_x (nm/V)":dbl=nan step=10.0 format="%#_3g"
  in  "T2 alpha_x (nm/V)":dbl=nan step=10.0 format="%#_3g"
  in  "T2 kappa_x (pN/nm)":dbl=nan min=0.0 step=0.001 format="%#_2g"
  in  "T2 offset_x (mV)":dbl=nan format="%#_2g"
  in  "BD 1 Frequency 2 (MHz)":dbl=80.0 caption="T2 X (MHz)" min=50.0 max=100.0 step=1.0 format="%#_6p"
  in  "Green Laser ON/Interlacing":bool=TRUE
  in  "Round T2 X":bool caption="Round"
  in  "AO1":dbl(slide) caption="Confocal Y (V)" min=0.0 max=10.0 step=0.01 scale=0.0..10.0 scale format="%_1f"
  in  "AO2":dbl(slide) caption="Confocal X (V)" min=0.0 max=10.0 step=0.01 scale=0.0..10.0 scale format="%_1f"
  in  "Trap Raster Scan":bool
  out "Raster Scanning...":bool
  in  "Trap Delta (MHz)":dbl(slide)=20.0 step=0.1 scale=6.0..15.0
  in  "Trap Intensity\nSetpoints (V)":cluster{"Set 1":dbl, "Set 2":dbl}={"Set 1"=5.2, "Set 2"=6.6}
  in  "Index":dbl=1.0 caption="Save File Index" min=1.0 step=1.0
  in  "BD 1 Frequency 1 (MHz)":dbl=65.0 caption="T1 X (MHz)" min=50.0 max=100.0 step=1.0 format="%#_6p"
  in  "Goto Top (F6)":bool
  in  "Save":bool
  in  "Capture":bool
  out "?":cluster{"x":string, "y":string, "z":string}={"x"="0.19233\r\n", "y"="0.00156\r\n", "z"="0.20615\r\n"}
  in  "Capture Locations":i32(listbox)=1
  out "X Pos":string="0.20503\r\n"
  out "Y Pos":string="0.00713\r\n"
  out "Z Pos Pos":string="0.21899\r\n"
  out "X Motion":string
  out "Y Motion":string
  out "Z motion":string
  in  "Goto Bottom (F7)":bool
  in  "Goto Exp (F8)":bool
  in  "Inject Top:":bool caption="Inject Pump 3"
  in  "Inject Bottom:":bool caption="Inject Pump 1"
  in  "Inject Shunt:":bool
  in  "Inject Main:":bool
  in  "Cal/Data Acq. Spot":bool
  out "Current Position":dbl[](array[numeric])=[4.2944, 4.91027471, 2.9278058] format="%7_7g"
  in  "Position Label 5":string="upper flow spot" caption="5"
  in  "Position 1 Label":string="Top capillary (SA beads)" caption="1"
  in  "Position 2 Label":string="Bottom capillary (AD) beads)" caption="2"
  in  "Position 3 Label":string="lower flow spot (ATP)" caption="3"
  in  "Position 4 Label":string="Dump beads" caption="4"
  out "Pump 3 cont disp":string="Left: ADig beads"
  out "Pump 1 cont disp":string="Right: DNA beads "
  in  "Ch 1 Inject Rate (ul/h)":dbl=50.0
  in  "Pump write delay (ms)":dbl=300.0
  in  "All Pump Parameters":T6={"Pump 1"={"Diameter (mm)"=4.61, "Units"=4.0, "Volume"=100.0, "Rate"=50.0}, "Pump 2"={"Diameter (mm)"=4.61, "Units"=3.0, "Volume"=0.0, "Rate"=0.0}, "Pump 3"={"Diameter (mm)"=4.61, "Units"=4.0, "Volume"=100.0, "Rate"=250.0}}
  in  "Ch 2 Inject Volume (uL)":dbl=100.0
  in  "Pump pause delay (ms)":u32
  in  "Ch 3 Inject Volume (uL)":dbl=100.0
  in  "Ch 3 Inject Rate (ul/h)":dbl=250.0
  in  "Flush Center Ch Volume (uL)":dbl=15.0
  in  "Flush Center Ch Rate (ul/m)":dbl=100.0
  in  "Inject Valve B":bool caption="Inject Pump 2\n(Flush Center)"
  in  "Total Volume\nFlushed (uL)":dbl
  in  "Tab Control 2":T7(tab)=enum."Feedback on Trap Intensity"
  in  "Restart RF":bool
  out "Total Counts (ticks)":u32=600
  in  "Trap ON/OFF X or Y Amp?":bool=TRUE
  in  "Oscillate Set 2":bool
  in  "Trap 1 ON":bool=TRUE
  in  "Number Interlace Sets":u8=3 min=1 max=3
  in  "DIO count 3 (ticks)":u32=200
  in  "DIO count 2 (ticks)":u32=200
  in  "DIO count 1 (ticks)":u32=200
  in  "BD 2 Amplitude 3 (%)":dbl min=0.0 max=75.0 step=1.0
  in  "BD 2 Amplitude 2 (%)":dbl min=0.0 max=75.0 step=1.0
  in  "BD 2 Amplitude 1 (%)":dbl min=0.0 max=75.0 step=1.0
  in  "BD 1 Amplitude 3 (%)":dbl min=0.0 max=75.0 step=1.0
  in  "BD 1 Amplitude 2 (%)":dbl=30.0 min=0.0 max=75.0 step=1.0
  in  "BD 1 Amplitude 1 (%)":dbl=30.0 min=0.0 max=75.0 step=1.0
  in  "BD 2 Frequency 3 (MHz)":dbl=26.0 min=50.0 max=100.0 step=1.0 format="%#_6p"
  in  "BD 1 Frequency 3 (MHz)":dbl=70.0 min=50.0 max=100.0 step=1.0 format="%#_6p"
  in  "BD 2 Frequency 2 (MHz)":dbl=26.0 min=50.0 max=100.0 step=1.0 format="%#_6p"
  in  "BD 2 Frequency 1 (MHz)":dbl=26.0 min=50.0 max=100.0 step=1.0 format="%#_6p"
  in  "Not-Interlacing Set":enum32{"Set 1", "Set 2", "Set 3"}(radio)
  in  "Interlace":bool=TRUE
  in  "Trap 2 ON":bool=TRUE
  in  "Trap 3 ON":bool
  in  "Scan axis 2":bool=TRUE
  in  "Osc. freq. (Hz)":dbl=0.25
  in  "Osc. amp. (MHz)":dbl=2.0 format="%1_3g"
  out "Coords":T8
  in  "Manipulation Scaling":cluster{"Horizontal":dbl, "Vertical":dbl}={"Horizontal"=0.075, "Vertical"=0.01}
  in  "Freq or Amp switch first":bool=TRUE
  in  "Swap F1 and F2":bool
  in  "Freq switch delay":u16
  in  "Amp switch delay":u16=5
  in  "Period":i64=2
  in  "MCL Step Increment (V_int)":dbl=3.0
  out "Time to Finish All (min)":dbl=0.122877 format="%#_2p"
  in  "Scan Speed (nm/s)":dbl=100.0
  in  "Scan Range (nm)":dbl=369.00000000000034
  in  "Step Size (nm)":dbl=1.0
  in  "MCL/AOM Scale Tweak":dbl=1.0
  in  "MCL Step Position Ratio":dbl=0.5
  in  "Move MCL Also?":bool=TRUE
  out "Final sep (nm)":dbl=4587.0
  out "Initial sep (nm)":dbl=4218.0
  out "Save index":dbl=22.0
  out "Final delta (MHz)":dbl=44.0
  out "Initial delta (MHz)":dbl=41.0
  out "Final freq. (MHz)":dbl=50.0
  out "Initial freq. (MHz)":dbl=53.0
  in  "Saved AOD Raster Scan Parameter Sets":T9(array[cluster])=[{"Scan Range AOD (nm) 2"=500.0, "Step Size AOD (nm) 2"=1.0, "Scan Speed AOD (nm/s) 2"=100.0, "Number of scans (AOD) 2"=1, "Label"="offset curve"}, {"Scan Range AOD (nm) 2"=420.0, "Step Size AOD (nm) 2"=1.0, "Scan Speed AOD (nm/s) 2"=100.0, "Number of scans (AOD) 2"=1, "Label"="hp raster check"}, {"Scan Range AOD (nm) 2"=6.8, "Step Size AOD (nm) 2"=0.34, "Scan Speed AOD (nm/s) 2"=0.34, "Number of scans (AOD) 2"=1, "Label"="3.4 kbp - 1 bp steps"}]
  in  "Load parameters":bool
  out "Scan Range (MHz)":dbl=-3.0000000000000027
  in  "Restart DMA? (AOD)":bool=TRUE caption="Restart DMA?"
  out "Incr. int (AOD)":i64=-7759651845
  out "Time/Scan (s) (AOD)":dbl=3.68631 format="%#_2p"
  out "Data points/scans":dbl=491508.0
  out "Data points/scan (f/b)":dbl=491508.0
  in  "Save scans":bool=TRUE
  out "AOD Scan I":u64 caption="Scan I"
  in  "Continuous AOD Scanning":bool caption="Continuous Scanning"
  in  "Abort AOD Scan":bool caption="Abort Scan"
  in  "Scan BD":bool=TRUE
  out "Cycles/step (AOD)":u64=666 format="%.3p"
  in  "Number of F/B Scans (AOD)":u16=1 min=1
  out "Scan steps (AOD)":u64=369
  out "Scan Increment (MHz)":dbl=-0.008152173913043485
  out "AOD Scanning":bool caption="Scanning"
  in  "Start AOD Scan":bool caption="Start Scan"
  out "N sets should be saved":dbl=24.5754
  out "Progress 2":u16(slide) caption="Progress" scale=0.0..100.0
  in  "Abort save 2":bool caption="Abort save"
  in  "Trap 1 Bead Size (nm)":dbl=2100.0
  in  "Trap 2 Bead Size (nm)":dbl=2100.0
  out "MCL Count":dbl=230502201.82069838
  in  "All FB On/Off":bool
  in  "AI2 to Setpoint":cluster{"Set 1":bool, "Set 2":bool}
  out "AI2 (V)":cluster{"Set 1":dbl, "Set 2":dbl}={"Set 1"=-0.0012207403790398877, "Set 2"=0.004577776421399579}
  in  "Reset Feedback":cluster{"Set 1":bool, "Set 2":bool}
  in  "PID Gains":T10={"Set 1"={"proportional gain (Kc)"=0, "integral gain (Kc*Ts/Ti)"=5, "derivative gain (Kc*Td/Ts)"=0}, "Set 2"={"proportional gain (Kc)"=0, "integral gain (Kc*Ts/Ti)"=5, "derivative gain (Kc*Td/Ts)"=0}}
  in  "Feedback On/Off":cluster{"Set 1":bool, "Set 2":bool}={"Set 1"=TRUE, "Set 2"=TRUE}
  in  "Reset Trap Pos. FB":bool
  in  "Tab Control 8":enum32{"Main Setting", "Details"}(tab)
  in  "Trap Pos FB Int Count":u16=100
  in  "Trap Pos. FB Gains":T11={"proportional gain (Kc)"=10.0, "integral gain (Kc*Ts/Ti)"=10.0, "derivative gain (Kc*Td/Ts)"=0.0} {"proportional gain (Kc)" format="%.11g"; "integral gain (Kc*Ts/Ti)" format="%.11g"; "derivative gain (Kc*Td/Ts)" format="%.11g"}
  in  "Trap Pos. FB Offset Factor":i64
  in  "Trap Pos FB Negate Action":bool
  in  "Trap Pos. FB Mult Factor":i64=33554432
  in  "Trap Pos. AI1 X Pre-scale":u16
  in  "Trap Pos. FB Range":T12={"output high"=0.999969482421875, "output low"=-1.0}
  out "Trap Pos FB Int Signal":fxp<+/-,24,9> format="%.18g"
  out "Trap Pos FB Int-Norm Signal":fxp<+/-,16,1> format="%.16g"
  in  "Set SP Using...":bool
  in  "Trap Pos FB Monitor\nT1 or T2":bool
  out "Trap X AI1 (DMA)":T13={"Set 1"=0.999969482421875, "Set 2"=0.999969482421875}
  in  "N El. to Ave.":dbl=10000.0
  out "Trap Pos FB Action":i64
  out "Mean T1 Position (nm)":dbl=-1.7479351299698465e-12 caption="Mean T1 (nm)" format="%0.2f"
  out "Trap 1 Position RMS (A)":dbl caption="RMS (Ang)"
  in  "Tab Control 3":enum32{"Timing", "MCL Scan", "Analog Out"}(tab)
  out "APD 2 Gate Late Counter":u32
  out "APD 2 Gate Relative Phase":i16
  in  "Phase Adj. (APD 2 Gate)":i16=20
  in  "Initial Phase Adjustment (APD 2 Gate)":i16=55
  out "APD 1 Gate Late Counter":u32
  in  "- phase (APD 1 Gate)":bool
  in  "+ phase (APD 1 Gate)":bool
  out "APD 1 Gate Relative Phase":i16
  in  "Phase Adj. (APD 1 Gate)":i16=20
  in  "Initial Phase Adjustment (APD 1 Gate)":i16=60
  in  "Save APD Data\nwith Trap Data":bool=TRUE
  out "APD FIFO Elements Remaining":u32
  in  "- phase (APD Acq)":bool
  in  "+ phase (APD Acq)":bool
  out "APD Acq Late Counter":u32
  out "APD Acq Relative Phase":i16
  in  "Phase Adj. (APD Acq)":i16=20
  in  "Initial Phase Adjustment (APD Acq)":i16
  in  "Invert APD Gate":bool caption="Invert Gate"
  in  "APD Gate OFF Count":u32=450 caption="Gate OFF Count"
  in  "APD Gate ON Count":u32=150 caption="Gate ON Count"
  in  "APD Gate":enum32{"ON", "OFF", "Interlace"}(radio)=enum."Interlace"
  in  "APD Integration Time (s)":dbl=0.01 caption="Integration Time (s)"
  out "APD Acq Rate (Hz)":dbl=100.0 caption="Rate (Hz)"
  out "APD Samples/FIFO Acq.":dbl=30.0
  out "APD Elements/DMA read":u32=60
  out "APD Int. Count":u32=400000 format="%.0p"
  in  "+ phase (APD 2 Gate)":bool
  in  "- phase (APD 2 Gate)":bool
  in  "Tab Control 5":enum32{"PSD X", "PSD Y", "Other Data Channel"}(tab)
  out "Data map":dbl[][](graph)
  in  "Channel":i32=4
  in  "Abort MCL Scan":bool
  out "MCL Scan I":u64
  out "MCL Scanning":bool
  in  "Start MCL Scan":bool
  out "wait to reset values":bool
  in  "Tab Control 4":enum32{"Scan Settings", "MCL FPGA Loop Timing"}(tab)
  out "Total Time (s)":dbl=48.0
  in  "Scan lines (y)":u64=20
  in  "Fast Scan Dir":bool=TRUE
  in  "2D or 1D Scan":bool=TRUE
  out "Initial X":dbl
  out "Initial Y":dbl
  out "Time/f+b scan (s) (MCL)":dbl=2.4 caption="Time/scan (s)"
  in  "Number of scans (MCL)":u64=1 caption="Scans"
  in  "Scan steps (MCL)":u64=40 caption="Scan steps (x)"
  in  "N APD Samp/step":dbl=3.0
  in  "Scan Range (V)\n(of steps)":dbl=3.5
  in  "Restart DMA? (MCL)":bool=TRUE caption="Restart DMA?"
  in  "Continuous MCL Scanning":bool caption="Cont. Scanning"
  in  "Center Scan":bool=TRUE
  in  "Save Data (MCL)":bool=TRUE caption="Save Data"
  out "Actual Incr. int (MCL)":i16=294 caption="Incr. int"
  out "Desired incr (int)":dbl=294.0628205128205
  out "Desired Scan Incr (V)":dbl=0.08974358974358974
  out "N sets should be saved (MCL)":dbl=160.0 caption="N sets should be saved"
  out "Data points/scans (MCL)":dbl=4800.0 caption="Data points/scans"
  out "Data points/scan (f+b)":dbl=240.0 caption="points/scan (f+b)"
  out "Cycles/step (MCL)":u64=2000 caption="Cycles/step" format="%.0p"
  out "Actual MCL Inc (V)":dbl=0.08972441785943175
  in  "Phase adjust (MCL)":i16 caption="Phase adjust"
  out "Relative Phase (MCL)":i16 caption="Relative Phase"
  in  "Initial Phase Adj. (MCL)":i16 caption="Initial Phase Adj."
  in  "Update Count (MCL)":u32=600
  in  "+ phase (MCL)":bool
  in  "- phase (MCL)":bool
  out "MCL Late Counter":u32
  in  "APD 1 AO Mult.":i16=1 min=1
  in  "APD 2 AO Mult.":i16=1 min=1
  in  "Tab Control 7":enum32{"Green FB Signals", "Slow MCL Scan"}(tab)
  out "Green FB Plot":dbl(graph)=10.0
  out "MCL Scan 2":cluster{"Begin (V)":dbl, dbl, dbl[]}(graph)
  out "MCL Scan":cluster{"Begin (V)":dbl, dbl, dbl[]}(graph)
  in  "Green laser mode":enum32{"Laser ON", "Laser OFF", "Interlace"}(radio)
  in  "GI Frequency, ON count":u32=150 min=1 step=1
  in  "Invert GI":bool
  out "GI Late Counter":u32
  in  "Phase adj. (GI)":i16=5
  out "GI relative phase":i16
  in  "+ phase (GI)":bool
  in  "Initial Phase Adjustment (GI)":i16=19
  in  "GI Frequency, OFF count":u32=450 min=1 step=1
  in  "- phase (GI)":bool
  out "Green FB Signals (V)":cluster{"Y":dbl, "X":dbl, "Sum":dbl}={"Y"=1.0, "X"=1.0, "Sum"=10.0}
  out "Relative phase (Green FB)":i16
  in  "+ phase (Green FB)":bool
  in  "- phase (Green FB)":bool
  in  "Green FB Count":u32=600
  in  "Phase adj. (Green FB)":i16=10
  in  "Initial Phase Adjustment (Green FB)":i16=50
  in  "Green FB On/Off":bool
  in  "Current When FB OFF (%)":dbl=10.0 min=0.0 max=100.0 step=1.0
  in  "Green int current ON count adj":u32=150
  in  "Green FB Gains":T14={"proportional gain (Kc)"=10, "integral gain (Kc*Ts/Ti)"=5, "derivative gain (Kc*Td/Ts)"=0}
  in  "Green FB Setpoint (mV)":dbl=100.0
  in  "- phase (GI) 2":bool
  in  "Initial Phase Adjustment (GI) 2":i16=-100
  in  "+ phase (GI) 2":bool
  out "GI relative phase 2":i16
  in  "Phase adj. (GI) 2":i16=20
  out "GI Late Counter 2":u32
  in  "Trap Position FIFO Depth":u32=300000 format="%.0p"
  in  "# Samples/trap":u32=20000 format="%.0p"
  out "Trap AI Elements/DMA read":u32=320000 format="%.0p"
  out "Ave. Rate (Hz)":dbl=200000.0 format="%#_6p"
  out "Trap AI FIFO El. Rem.":u32 format="%.0p"
  in  "Phase adj. (AI1)":i16
  out "Relative phase (AI1)":i16
  in  "+ phase (AI1)":bool
  in  "- phase (AI1)":bool
  out "Late Counter (AI1)":u32
  in  "Initial Phase Adjustment (AI1)":i16=180
  out "AI rate (Hz)":dbl=200000.0 format="%#_6p"
  in  "AI Count (ticks)":u32=200
  out "# Samples/channel":u32=40000 format="%.0p"
  in  "Trap AI FIFO Depth":u32=340000 format="%.0p"
  in  "Detector Type":string(combo)="UCB Fleezers 052511"
  in  "N Acq Sets (Traps + Fl.)":i16=3
  in  "Sets to FIFO (Traps)":T15={"Set 1"=TRUE, "Set 2"=TRUE, "Set 3"=FALSE}
  in  "FPGA Ave.":dbl=1.0 min=1.0 step=1.0
  out "Ave. Period (s)":dbl=5e-06 format="%#_6p"
  out "DMA Update Period (s)":dbl=0.3
  out "FPGA Averaging":bool
  out "Trap Sets":u32=2
  out "Counts/DMA":dbl=12000000.0 format="%#_6p"
  out "Trap Pos FIFO El Remaining":u32=141
  out "Trap Pos Elements/DMA read":u32=120000 format="%.0p"
  out "Trap AI FIFO Timeout":u16
  out "Trap Pos FIFO Timeout":u16
  out "Waveform Chart":i32(graph)=320000
  out "error out 2":errorcluster
  in  "Lost Tether Alarm Threshold (pN)":dbl=0.5
  in  "AOM X Cal (nm/MHz)":dbl=168.33
  in  "MCL X Cal (nm/V)":dbl=1070.0
  out "X RF Amplitude Limits (%)":T16={"Minimum"=0.0, "Maximum"=50.0, "Increment"=1.0}
  out "X RF Frequency Limits (MHz)":T16={"Minimum"=50.0, "Maximum"=100.0, "Increment"=1.0}
  out "Y RF Frequency Limits (MHz)":T16={"Minimum"=50.0, "Maximum"=100.0, "Increment"=1.0}
  out "Y RF Amplitude Limits (%)":T16={"Minimum"=0.0, "Maximum"=50.0, "Increment"=1.0}
  in  "Manip. X?":bool=TRUE
  in  "Manip. Y?":bool
  in  "Force Manip Abort":bool
  out "Read cal error":errorcluster
  in  "DAQ Delay (ms)":u32=1000
  in  "Start Scan":bool
  in  "Scan axis":bool
  in  "Osc. amp. (V)":dbl=5.0
  in  "Osc. center (V)":dbl=5.0
  in  "Osc. freq. (Hz) 2":dbl=1.0
  in  "MCL Mode":u16(ring) items=["Manual Positioning", "Sinusoidal Wave", "Linear Scan"]
  in  "Begin (V)":dbl
  in  "End (V)":dbl=10.0
  in  "N Points":dbl=20.0
  in  "Delay to Interlace (s)":dbl
  in  "Delayed Interlace Start":bool
  in  "Read Lateness and Rel Phase":bool
  out "Vec Mean of T1 T2":dbl[](array[numeric])=[nan, nan]
  in  "Cal read wait (s)":u32=5
  out "Time tether formed":timestamp=timestamp(3371146929.513132 s since 1904-01-01)
  in  "Chemyx Syringe Pump Serial Port":refnum<visa-resource-name>="ASRL3::INSTR"
  in  "Limit Min (MHz)":dbl=10.0 caption="Min (MHz)"
  in  "Limit Max (MHz)":dbl=16.0 caption="Max (MHz)"
  in  "Limits Enable":bool=TRUE caption="Enable"
  out "AI labels":string[](array[string])=["T1 Y", "T1 X", "T1 Sum", "T2 Y", "T2 X", "T2 Sum", "T1 FB X", "T2 FB Sum", "T2 FB X", "T2 FB Sum", "PSD Y", "PSD X", "PSD Sum"]
  in  "Save Trap Pos. Data":bool=TRUE
  in  "ESP Port":refnum<visa-resource-name>="COM22"
  in  "Axis 3":string="0.00500\r\n"
  in  "Axis 2":string="0.00500\r\n"
  in  "Axis 1":string="0.00500\r\n"
  in  "Axis 3":string="0.20000\r\n"
  in  "Axis 2":string="0.20000\r\n"
  in  "Axis 1":string="0.20000\r\n"
  in  "Activate Joystick":bool
  in  "ESP ZL-Limit":string="-0.09900"
  in  "ESP ZR-Limit":string="0.09900"
  in  "error in":errorcluster
  out "error out":errorcluster
  # "Save Positions of Cambers"
  # "After"
  # "During"
  # "Trap On?"
  # "BD Flow ON?"
  # "Samp Flow ON?"
  # "1"
  # "2"
  # "Trap Display:"
  # "APD Display:"
  # "originally 10k"
  # "Data Saving"
  # "Trap Manipulation"
  # "DAQ"
  # "Central frequency 80 MHz"
  # "F9"
  # "F10"
  # "Bead Calibration"
  # "Current Location"
  # "Select the position to go to"
  # "F4"
  # "Press F12 to move stage\nwith the mouse. F12 to cancel."
  # "F5"
  # "F6"
  # "F7"
  # "F8"
  # "Harvard Pump\n(sample channel for flow exp)"
  # "Chemyx Pump 2"
  # "Units: \n1 = ml/m\n2 = ml/h\n3 = ul/m\n4 = ul/h"
  # "Rate param is ul/h\nVolume param is ul"
  # "X"
  # "Y"
  # "Oscillate Set 2 freq. (debugging)"
  # "BD 1"
  # "BD 2"
  # "AOD Raster Scan"
  # "Approx. trap separations"
  # "X"
  # "Y"
  # "DON'T TURN ON\nUNTIL YOU CLOSE\nTHE LOOP"
  # "FPGA\nreading"
  # "DMA\ntransfer"
  # "APD Gates"
  # "APD 2"
  # "APD 1"
  # "X"
  # "2D"
  # "Y"
  # "1D"
  # "Green FB Measurement"
  # "Green Laser Interlacing"
  # "Digital Gate"
  # "Current Analog Control"
  # "was 87"
  # "originally 600k"
  # "Total AI Rates (NOT rates/trap)"
  # "originally 20k"
  # "(Samples/trap x Trap Sets)"
  # "(Samples/channel x\n8 if averaging (8 channels)\n4 if no averaging)"
  # "Trap 1"
  # "Trap 2"
  # "Flour./Trap 3"
  # "External Video Window"
  # "MCL Position Debugging"
  # "Temporary Control Storage\n(these used to be somewhere else, still want to keep them)"
  # "Y"
  # "X"
  # "Trap Position Difference Limits"
  # "Joystick Control"
  # "Setting Limit for the z-axis"
  # "High Jog Velocity"
  # "Low Jog Velocity"
  # "Errors detected in determing Current Location"
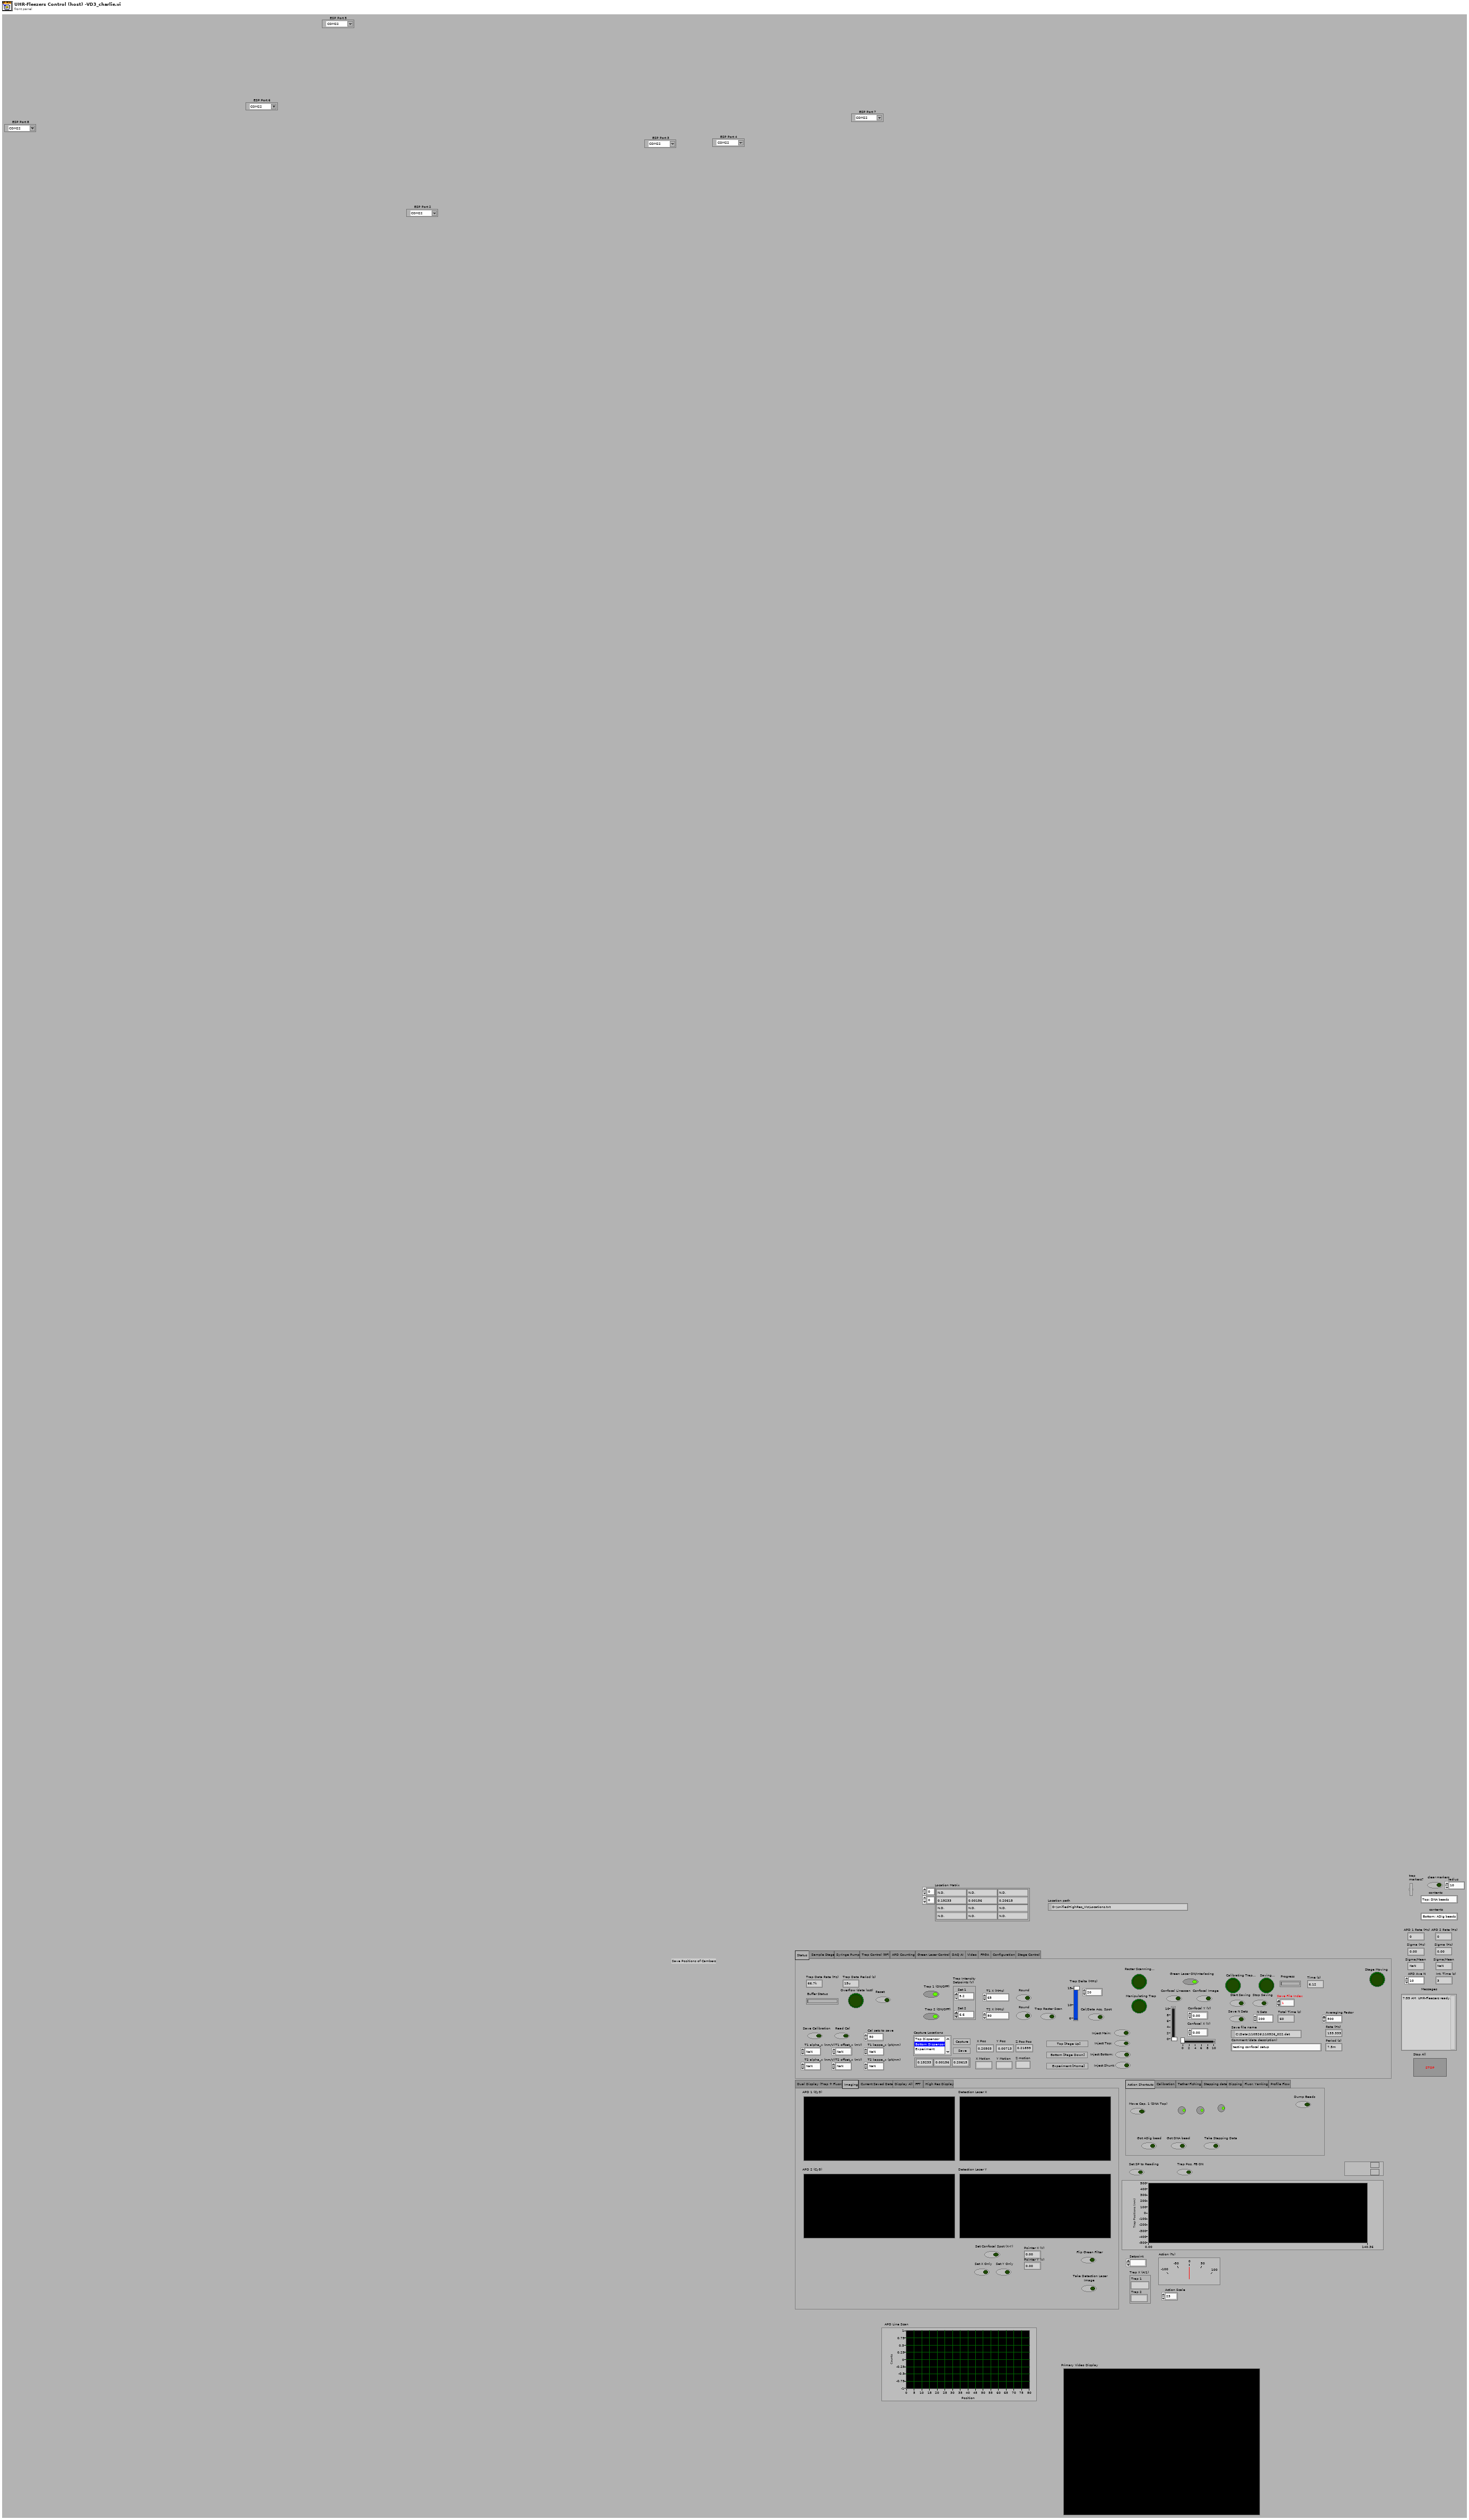
[diagram p1: front panel]
types:
  T1 = cluster{"Trap 1":fxp<+/-,16,1>, "Trap 2":fxp<+/-,16,1>}
  T2 = enum32{"Action Shortcuts", "Calibration", "Tether Fishing", "Stepping data", "Dipping", "Fluor. Yanking", "Profile Flow"}
  T3 = typedef "IMAQ Image.ctl" = refnum<image>
  T4 = enum32{"Dual Display (Trap + Fluor.)", "Imaging", "Current Saved Data", "Display All", "FFT", "High Res Display"}
  T5 = enum32{"Status", "Sample Stage", "Syringe Pump", "Trap Control (RF)", "APD Counting", "Green Laser Control", "DAQ AI", "Video", "FPGA", "Configuration", "Stage Control"}
  T6 = cluster{"Pump 1":cluster{"Diameter (mm)":dbl, "Units":dbl, "Volume":dbl, "Rate":dbl}, "Pump 2":cluster{"Diameter (mm)":dbl, "Units":dbl, "Volume":dbl, "Rate":dbl}, "Pump 3":cluster{"Diameter (mm)":dbl, "Units":dbl, "Volume":dbl, "Rate":dbl}}
  T7 = enum32{"IR Laser Interlacing (Direct RF Board Control Method)", "AOD Raster Scan", "Feedback on Trap Intensity", "Feedback on Trap Position"}
  T8 = typedef "LVPoint32TypeDef.ctl" = cluster{"Horizontal":i32, "Vertical":i32}
  T9 = cluster{"Scan Range AOD (nm) 2":dbl, "Step Size AOD (nm) 2":dbl, "Scan Speed AOD (nm/s) 2":dbl, "Number of scans (AOD) 2":u16, "Label":string}[]
  T10 = cluster{"Set 1":cluster{"proportional gain (Kc)":i16, "integral gain (Kc*Ts/Ti)":i16, "derivative gain (Kc*Td/Ts)":i16}, "Set 2":cluster{"proportional gain (Kc)":i16, "integral gain (Kc*Ts/Ti)":i16, "derivative gain (Kc*Td/Ts)":i16}}
  T11 = cluster{"proportional gain (Kc)":fxp<+/-,16,8>, "integral gain (Kc*Ts/Ti)":fxp<+/-,16,8>, "derivative gain (Kc*Td/Ts)":fxp<+/-,16,8>}
  T12 = cluster{"output high":fxp<+/-,16,1>, "output low":fxp<+/-,16,1>}
  T13 = cluster{"Set 1":fxp<+/-,16,1>, "Set 2":fxp<+/-,16,1>}
  T14 = cluster{"proportional gain (Kc)":i16, "integral gain (Kc*Ts/Ti)":i16, "derivative gain (Kc*Td/Ts)":i16}
  T15 = cluster{"Set 1":bool, "Set 2":bool, "Set 3":bool}
  T16 = typedef "LVMinMaxIncTypeDef.ctl" = cluster{"Minimum":dbl, "Maximum":dbl, "Increment":dbl}
  T17 = typedef "Image Type" = u32
  T18 = typedef "nirio_resource_hc.ctl" = tag
  T19 = typedef "openfpgaref.8.6.ctl" = refnum<k20>
  T20 = enum16{"CONNECT", "INITIALIZE VALVES", "DISCONNECT", "MOVE VALVE"}
  T21 = cluster{"New Image":T3, "New Image":T3, "New Image":T3, "New Image":T3}
  T22 = cluster{"Location Matrix[0]":string, "Location Matrix[1]":string, "Location Matrix[2]":string}
  T23 = enum16{"open", "replace", "create", "open or create", "replace or create", "replace or create with confirmation"}
  T24 = typedef "XDNodeRunTimeDep.lvlib/timing_clust.ctl" = cluster{"Expected End [f-1]":u64, "Actual End [f-1]":u64, "Finished Late? [f-1]":bool, "Expected End [i-1]":u64, "Actual End [i-1]":u64, "Finished Late? [i-1]":bool, "Expected Start [i]":u64, "Actual Start [i]":u64, "Expected Start [f]":u64, "Actual Start [f]":u64, "Source Name":string, "Structure Name":string, "Period":i64, "Deadline":i64, "Offset":i64, "Start":i64, "Priority":i32, "Timeout":i32, "Mode":T25, "Wakeup Reason":T26, "Error":errorcluster, "Source Type":string, "Secondary Source Type":string, "Global End Time":u64, "Global Start Time":u64, "Frame Duration":u64, "Iteration Duration":u64, "Assigned CPU":i32, "I/O Scan Engine Mode":u32}
  T25 = typedef "XDNodeRunTimeDep.lvlib/nitl_modes.ctl" = enum32{"No Change", "Process missed periods, maintain original phase", "Discard missed periods, maintain original phase", "Process missed periods, ignore original phase", "Discard missed periods, ignore original phase"}
  T26 = typedef "XDNodeRunTimeDep.lvlib/wakeup.ctl" = enum32{"Normal", "Aborted", "Asynchronous wakeup", "Timing source error", "Timed loop error", "Timeout"}
  T27 = cluster{"[0]":i32, "[1]":i32, "[2]":i32, "[3]":i32}
  T28 = cluster{"[0]":i32, "[1]":i32, "[2]":i32, "[3]":i32}[]
  T29 = enum16{"big-endian, network order", "native, host order", "little-endian"}
  T30 = cluster{"Scan Range AOD (nm) 2":dbl, "Step Size AOD (nm) 2":dbl, "Scan Speed AOD (nm/s) 2":dbl, "Number of scans (AOD) 2":u16, "Label":string}
  T31 = cluster{"[0]":dbl, "[1]":dbl, "[2]":dbl, "[3]":dbl, "[4]":dbl, "[5]":dbl}
  T32 = cluster{"Diameter (mm)":dbl, "Units":dbl, "Volume":dbl, "Rate":dbl}
  T33 = cluster{"Left":i32, "Top":i32, "Width":u32, "Height":u32}
  T34 = cluster{cluster{"Left":i32, "Top":i32, "Width":u32, "Height":u32}}[]
  T35 = enum32{"Normal Display", "Dual Display (APD)", "FFT", "High Res Display"}
  T36 = cluster{"Origin Pixel":cluster{"X":sgl, "Y":sgl}, "Angle Relative to Horizontal (deg)":sgl, "Axis Reference":u32}
  T37 = typedef "Simple Grid Descriptor" = cluster{"X Step":sgl, "Y Step":sgl, "Unit":T38}
  T38 = typedef "Image Unit" = enum32{"Undefined", "Angström", "Micrometer", "Millimeter", "Centimeter", "Meter", "Kilometer", "Microinch", "Inch", "Feet", "Nautical miles", "Standard miles", "Steps"}
  T39 = cluster{"averaging mode":u16, "weighting mode":u16, "number of averages":u32}
  T40 = cluster{"dB On (F)":bool, "unwrap phase (F)":bool, "convert to degree (F)":bool}
  T41 = cluster{string, string, string, string, string, string, string, string}
  T42 = cluster{string, string, string, string, string, string, string, string, string, string, string, string}
  T43 = cluster{string, string, string, string, string, string, string, string, string, string, string, string, string}
  T44 = cluster{string, string, string, string, string, string, string, string, string, string, string, string, string, string}
  T45 = cluster{"BD 1 Frequency 1 (MHz)":dbl, "BD 1 Frequency 2 (MHz)":dbl}
  T46 = cluster{"f0":dbl, "df":dbl, "magnitude":dbl[]}[][]
  T47 = cluster{"Green FB Ch 0":i16, "Green FB Ch 1":i16, "Green FB Ch 2":i16}
  T48 = cluster{"Green FB Ch 0":dbl, "Green FB Ch 1":dbl, "Green FB Ch 2":dbl}
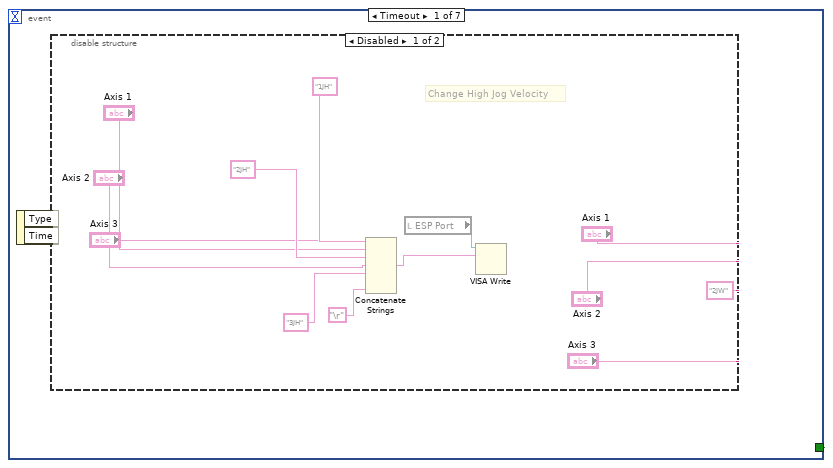
[diagram p2: hidden frame]
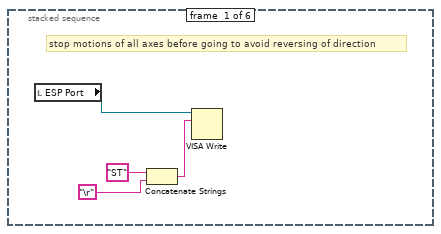
[diagram p5: hidden frame]
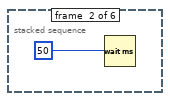
[diagram p6: hidden frame]
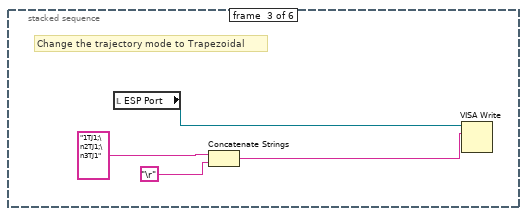
[diagram p7: hidden frame]
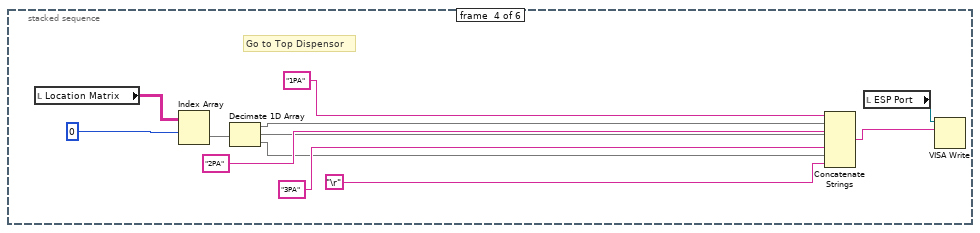
[diagram p8: hidden frame]
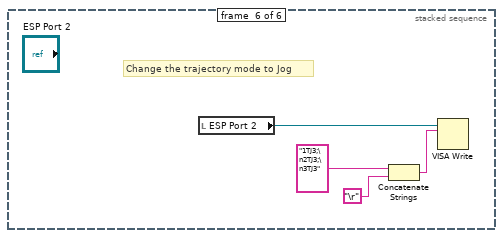
[diagram p9: hidden frame]
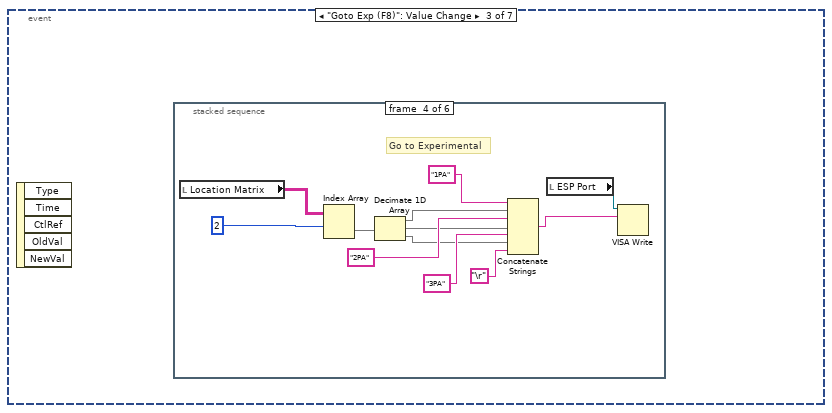
[diagram p10: hidden frame]
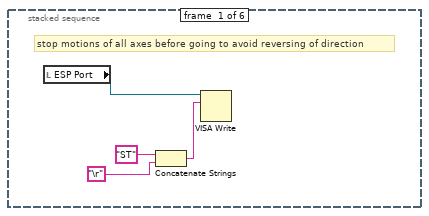
[diagram p11: hidden frame]
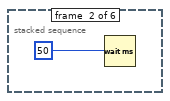
[diagram p12: hidden frame]
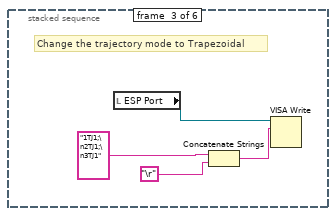
[diagram p13: hidden frame]
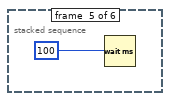
[diagram p14: hidden frame]
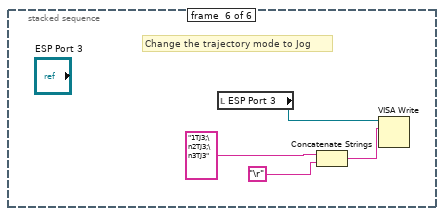
[diagram p15: hidden frame]
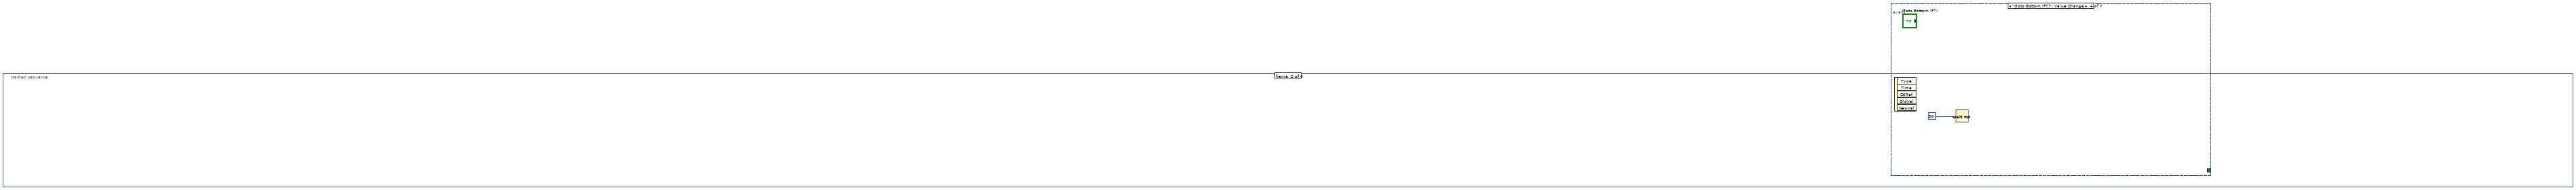
[diagram p16: hidden frame]
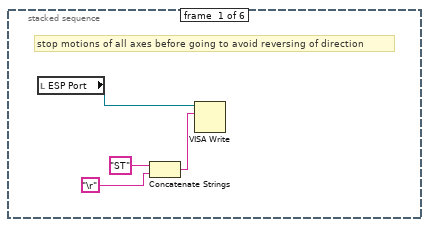
[diagram p17: hidden frame]
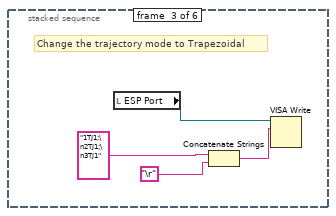
[diagram p18: hidden frame]
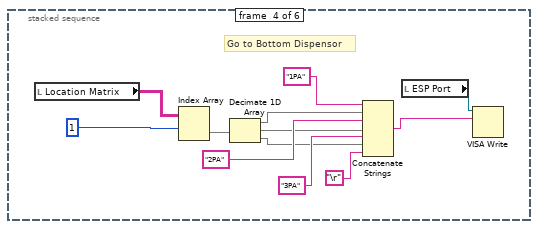
[diagram p19: hidden frame]
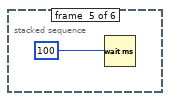
[diagram p20: hidden frame]
diagram:
  w64 = T17 2 items=["Grayscale (U8)", "Grayscale (I16)", "Grayscale (SGL)", "Complex (CSG)", "RGB (U32)", "HSL (U32)", "RGB (U64)", "Grayscale (U16)"] ("Image Type")
  w121 = cluster{"output high":i16, "output low":i16} {"output high"=3000, "output low"=0} ("FB output range 1")
  w196 = 10.0 ("y")
  w195 = 32767.0 ("y")
  w211 = 6.0  # clock mult.
  w212 = 49152000.0  # TCXO frequ.
  # "Initialize location matrix"
  n1 = Build Array("DIO count 1 (ticks)", "DIO count 2 (ticks)", "DIO count 3 (ticks)") -> (w110:u32[])
  n2 = Multiply(x="APD Integration Time (s)", y=40000000.0) -> (x*y=w128:dbl)
  n3 = Reciprocal(x="APD Integration Time (s)") -> (1/x=w125:dbl)
  n4 = local write "APD Acq Rate (Hz)"(w125) -> ()
  n5 = local read "AO1"() -> (w190:dbl)
  n6 = local read "AO2"() -> (w189:dbl)
  n7 = To Unsigned Long Integer(number=w128) -> (unsigned 32bit integer=w127:u32)
  "APD Int. Count" <- w127
  n8 = local read "Scan Increment (MHz)"() -> (w207:dbl)
  n9 = local read "Continuous MCL Scanning"() -> (w177:bool)
  n10 = local read "Fast Scan Dir"() -> (w176:bool)
  n11 = local read "Trap Intensity\nSetpoints (V)"() -> (w226:cluster{"Set 1":dbl, "Set 2":dbl})
  n12 = local read "Number of scans (MCL)"() -> (w178:u64)
  n13 = Multiply(x=w190, y=w195) -> (x*y=w192:dbl)
  n14 = Multiply(x=w189, y=w195) -> (x*y=w194:dbl)
  n15 = Divide(x=w192, y=w196) -> (x/y=w191:dbl)
  n16 = Divide(x=w194, y=w196) -> (x/y=w193:dbl)
  n17 = To Word Integer(number=w191) -> (16bit integer=w188:i16)
  n18 = To Word Integer(number=w193) -> (16bit integer=w187:i16)
  n19 = Not(x=w176) -> (.not. x?=w171:bool)
  n20 = local read "Cycles/step (MCL)"() -> (w179:u64)
  n21 = Multiply(x=w207, y=1000.0) -> (x*y=w214:dbl)
  n22 = local read "Scan steps (MCL)"() -> (w180:u64)
  n23 = local write "Trap Pos FIFO Timeout"(u16 0 ("Trap Pos FIFO Timeout")) -> ()
  n24 = local read "Desired Scan Incr (V)"() -> (w182:dbl)
  n25 = Scale By Power Of 2(n=48, x=w214) -> (x*2^n=w215:dbl)
  n26 = Multiply(x=w212, y=w211) -> (x*y=w210:dbl)
  n27 = Divide(x=w215, y=w210) -> (x/y=w209:dbl)
  n28 = local read "Number Interlace Sets"() -> (w103:u8)
  n29 = Split 1D Array(array=w110, index=w103) -> (first subarray=w112:u32[])  [unwired: 1 out]
  n30 = Add Array Elements(numeric array=w112) -> (sum=w111:u32)
  n31 = property on="AI Count (ticks)" class="DigNum (strict)"("Val(Sgnl)"="AI Count (ticks)") -> ()  [unwired: 2 in, 2 out]
  n32 = local read "# Samples/channel"() -> (w199:u32)
  n33 = local read "Number of F/B Scans (AOD)"() -> (w200:u16)
  n34 = To Quad Integer(1:w209) -> (0:w206:i64)
  n35 = local read "Not-Interlacing Set"() -> (w102:enum32{"Set 1", "Set 2", "Set 3"})
  n36 = To Unsigned Byte Integer(number=w102) -> (unsigned 8bit integer=w108:u8)
  n37 = Index Array(array=w110, index=w108) -> (element=w109:u32)
  n38 = local read "Feedback On/Off"() -> (w229:cluster{"Set 1":bool, "Set 2":bool})
  n39 = local read "PID Gains"() -> (w221:T10)
  n40 = Divide(x=40000000.0, y="AI Count (ticks)") -> (x/y=w168:dbl)
  n41 = Multiply(x=w182, y=32767.0) -> (x*y=w184:dbl)
  n42 = local read "Scan steps (AOD)"() -> (w205:u64)
  n43 = local read "All FB On/Off"() -> (w230:bool)
  n44 = local read "Cycles/step (AOD)"() -> (w204:u64)
  n45 = local write "AI rate (Hz)"(w168) -> ()
  n46 = Divide(x=w184, y=10.0) -> (x/y=w183:dbl)
  n47 = Multiply(x=w205, y=w204) -> (x*y=w203:u64)
  n48 = Multiply(x=3276.7, y=w226) -> (x*y=w225:cluster{"Set 1":dbl, "Set 2":dbl})
  n49 = To Word Integer(number=w183) -> (16bit integer=w181:i16)
  n50 = Multiply(x=w203, y=u64 2) -> (x*y=w201:u64)
  n51 = local read "Sets to FIFO (Traps)"() -> (w233:T15)
  n52 = Divide(x=w168, y="FPGA Ave.") -> (x/y=w169:dbl)
  n53 = To Word Integer(number=w225) -> (16bit integer=w224:cluster{"Set 1":i16, "Set 2":i16})
  n54 = xnode "Open FPGA VI Reference"("resource name"=T18 "750kHzDAQ") -> ("FPGA VI Reference Out"=w218:T19)  [unwired: 1 in, 1 out]
  n55 = Unbundle By Name(w221) -> ("Set 1"=w220:T14, "Set 2"=w219:T14)
  n56 = Multiply(x=w201, y=w200) -> (x*y=w198:u64)
  n57 = local write "Ave. Rate (Hz)"(w169) -> ()
  n58 = Divide(x=w198, y=w199) -> (x/y=w197:dbl)
  n59 = Unbundle By Name(w224) -> ("Set 1"=w223:i16, "Set 2"=w222:i16)
  n60 = local read "2D or 1D Scan"() -> (w122:bool)
  n61 = local write "Data points/scans"(w198) -> ()
  n62 = local read "Scan BD"() -> (w216:bool)
  n63 = And(x=w229, y=w230) -> (x .and. y?=w228:cluster{"Set 1":bool, "Set 2":bool})
  n64 = local write "Data points/scan (f/b)"(w201) -> ()
  n65 = Reciprocal(x=w169) -> (1/x=w170:dbl)
  n66 = local read "N Acq Sets (Traps + Fl.)"() -> (w161:i16)
  n67 = local write "N sets should be saved"(w197) -> ()
  n68 = Unbundle By Name(w228) -> ("Set 1"=w232:bool, "Set 2"=w231:bool)
  n69 = local read "Interlace"() -> (w104:bool)
  n70 = Select(t=w111, s=w104, f=w109) -> (s? t:f=w101:u32)
  n71 = local write "Update Count (MCL)"(w101) -> ()
  n72 = local write "Total Counts (ticks)"(w101) -> ()
  n73 = xnode "Invoke Method"("FPGA VI Reference In"=w218) -> ("FPGA VI Reference Out"=w120:T19, "error out"=w139:errorcluster)  [unwired: 1 in]
  n74 = local write "Ave. Period (s)"(w170) -> ()
  n75 = property on="2D or 1D Scan" class="Bool (strict)"("Val(Sgnl)"=w122) -> ()  [unwired: 2 in, 2 out]
  n76 = xnode "Read/Write Control"("FPGA VI Reference In"=w119, "error in"=w139, "ai count"="AI Count (ticks)", "Interlace ON/OFF"=w104, "Number Interlace Cycles"=w103, "AI1 Sets to FIFO"=w233, "FB On/Off Set 1"=w232, "FB On/Off Set 2"=w231, "Interlace Off Parameters"=w102, "FB Setpoint Set 1"=w223, "FB Setpoint Set 2"=w222, "FB Gains Set 1"=w220, "FB Gains Set 2"=w219, "FB output range 1"=w121, "FB output range 2"=w121, "Cycles per step"=w204, "Scan BD"=w216, "Number of scans"=w200, "Scan steps"=w205, "Scan freq.  increment"=w206, "AO1"=w188, "AO2"=w187, "Scan freq.  increment (MCL)"=w181, "Scan steps (MCL)"=w180, "Cycles per step (MCL)"=w179, "Number of scans (MCL)"=w178, "MCL count"=w101, "Cont. Scan (MCL)"=w177, "MCL Scan Axis"=w171, "1D or 2D Scan?"=w122, "N of AI1 Int Acq Sets"=w161, "Freq or Amp switch first"="Freq or Amp switch first", "Freq switch delay"="Freq switch delay", "Amp switch delay"="Amp switch delay", "Swap F1 and F2"="Swap F1 and F2", "APD Acq Rate Count"=w127, "APD to FIFO"=FALSE, "APD Gate Operating Mode"="APD Gate", "APD Gate ON Count"="APD Gate ON Count", "APD Gate OFF Count"="APD Gate OFF Count", "Invert APD Gate"="Invert APD Gate", "DIO count 1 (ticks)"="DIO count 1 (ticks)", "DIO count 2 (ticks)"="DIO count 2 (ticks)", "DIO count 3 (ticks)"="DIO count 3 (ticks)", "APD 1 AO scale factor"="APD 1 AO Mult.", "APD 2 AO scale factor"="APD 2 AO Mult.") -> ("FPGA VI Reference Out"=w96:T19, "error out"=w98:errorcluster)  [unwired: 1 in]
  n77 = local read "Green Laser ON/Interlacing"() -> (w99:bool)
  n78 = local read "Green laser mode"() -> (w100:enum32{"Laser ON", "Laser OFF", "Interlace"})
  n79 = local read "GI Frequency, OFF count"() -> (w92:u32)
  n80 = local read "GI Frequency, ON count"() -> (w91:u32)
  n81 = Multiply(x="Current When FB OFF (%)", y=655.35) -> (x*y=w82:dbl)
  n82 = local read "Green FB Count"() -> (w90:u32)
  n83 = Multiply(x="Green FB Setpoint (mV)", y=3.2767) -> (x*y=w79:dbl)
  n84 = To Unsigned Word Integer(number=w82) -> (unsigned 16bit integer=w80:u16)
  n85 = local read "Invert GI"() -> (w94:bool)
  n86 = To Word Integer(number=w79) -> (16bit integer=w77:i16)
  n87 = case shown="True" w99 {
    tunnel: w100 -> [_ w253]
    tunnel: [enum32{"Laser ON", "Laser OFF", "Interlace"}."Laser OFF" ("Green laser mode") w253] -> w93
    frame False {
    }
    frame True {
    }
  }
  n88 = local read "Trap Pos. AI1 X Pre-scale"() -> (w48:u16)
  n89 = local read "Trap Pos FB Monitor\nT1 or T2"() -> (w55:bool)
  n90 = local read "Trap Pos FB Int Count"() -> (w43:u16)
  n91 = local read "Trap Pos FB Negate Action"() -> (w54:bool)
  n92 = local read "Trap Pos. FB Offset Factor"() -> (w53:i64)
  n93 = local read "Trap Pos. FB Mult Factor"() -> (w52:i64)
  n94 = local read "Trap Pos. FB Gains"() -> (w50:T11)
  n95 = local read "Trap Pos. FB Range"() -> (w51:T12)
  n96 = xnode "Read/Write Control"("FPGA VI Reference In"=w96, "error in"=w98, "Green interlace ON count 2"=w91, "Green interlace OFF count 2"=w92, "Invert GI 2"=w94, "Operating Mode 2"=w93, "Green FB Gains"="Green FB Gains", "Green FB Setpoint"=w77, "Green FB On/Off"="Green FB On/Off", "Current Out"=w80, "Green int current ON count adj"="Green int current ON count adj", "Green FB Count"=w90, "Operating Mode"=w93, "Green interlace OFF count"=w92, "Green interlace ON count"=w91, "Invert GI"=w94, "Trap Pos FB Monitor T1 or T2"=w55, "Trap Pos FB Negate Action"=w54, "Trap Pos. FB Offset Factor"=w53, "Trap Pos. FB Mult Factor"=w52, "Trap Pos. FB Range"=w51, "Trap Pos. FB Gains"=w50, "Force feedback"=FALSE, "AI1 X Scale"=w48, "Trap Pos to FIFO"=TRUE, "Trap Pos FB Int Count"=w43) -> ("FPGA VI Reference Out"=w95:T19, "error out"=w97:errorcluster)
  n97 = xnode "Invoke Method"("FPGA VI Reference In"=w95, "error in"=w97, "Requested Depth"="Trap AI FIFO Depth") -> ("FPGA VI Reference Out"=w58:T19, "error out"=w57:errorcluster)  [unwired: 1 out]
  n98 = xnode "Invoke Method"("FPGA VI Reference In"=w58, "error in"=w57, "Requested Depth"="Trap Position FIFO Depth") -> ("FPGA VI Reference Out"=w45:T19, "error out"=w44:errorcluster)  [unwired: 1 out]
  n99 = flat-sequence {
    tunnel: w120 -> [w258]
    tunnel: [w258] -> w119
    tunnel: [w257] -> w118
    tunnel: [w256] -> w117
    tunnel: [w254] -> w115
    tunnel: [w255] -> w116
    frame #0 {
      w255 = T16 {"Minimum"=50.0, "Maximum"=100.0, "Increment"=1.0} ("Min Max Inc")
      w254 = T16 {"Minimum"=0.0, "Maximum"=75.0, "Increment"=1.0} ("Data Entry Limits")
      w257 = T16 {"Minimum"=50.0, "Maximum"=100.0, "Increment"=1.0} ("Min Max Inc")
      w256 = T16 {"Minimum"=0.0, "Maximum"=75.0, "Increment"=1.0} ("Data Entry Limits")
      n100 = property on="BD 2 Frequency 1 (MHz)" class="DigNum (strict)"("Data Range"=w255) -> ()  [unwired: 2 in, 2 out]
      n101 = property on="BD 2 Frequency 3 (MHz)" class="DigNum (strict)"("Data Range"=w255) -> ()  [unwired: 2 in, 2 out]
      n102 = property on="BD 2 Frequency 2 (MHz)" class="DigNum (strict)"("Data Range"=w255) -> ()  [unwired: 2 in, 2 out]
      n103 = property on="BD 1 Frequency 1 (MHz)" class="DigNum (strict)"("Data Range"=w257) -> ()  [unwired: 2 in, 2 out]
      n104 = property on="BD 1 Frequency 2 (MHz)" class="DigNum (strict)"("Data Range"=w257) -> ()  [unwired: 2 in, 2 out]
      n105 = property on="BD 1 Frequency 3 (MHz)" class="DigNum (strict)"("Data Range"=w257) -> ()  [unwired: 2 in, 2 out]
      n106 = property on="BD 2 Amplitude 1 (%)" class="DigNum (strict)"("Data Range"=w254) -> ()  [unwired: 2 in, 2 out]
      n107 = property on="BD 2 Amplitude 2 (%)" class="DigNum (strict)"("Data Range"=w254) -> ()  [unwired: 2 in, 2 out]
      n108 = property on="BD 2 Amplitude 3 (%)" class="DigNum (strict)"("Data Range"=w254) -> ()  [unwired: 2 in, 2 out]
      n109 = property on="BD 1 Amplitude 3 (%)" class="DigNum (strict)"("Data Range"=w256) -> ()  [unwired: 2 in, 2 out]
      n110 = property on="BD 1 Amplitude 2 (%)" class="DigNum (strict)"("Data Range"=w256) -> ()  [unwired: 2 in, 2 out]
      n111 = property on="BD 1 Amplitude 1 (%)" class="DigNum (strict)"("Data Range"=w256) -> ()  [unwired: 2 in, 2 out]
      "X RF Frequency Limits (MHz)" <- w257
      "X RF Amplitude Limits (%)" <- w256
      "Y RF Amplitude Limits (%)" <- w254
      "Y RF Frequency Limits (MHz)" <- w255
    }
  }
  n112 = xnode "Invoke Method"("FPGA VI Reference In"=w45, "error in"=w44) -> ("FPGA VI Reference Out"=w22:T19, "error out"=w21:errorcluster)  [unwired: 1 in]
  n113 = flat-sequence "Initial FPGA Loop Relative Phase Adjustment" {
    tunnel: "Initial Phase Adjustment (APD 2 Gate)" -> [w260]
    tunnel: "Initial Phase Adjustment (GI) 2" -> [w261]
    tunnel: "Initial Phase Adj. (MCL)" -> [w262]
    tunnel: w21 -> [w263]
    tunnel: w22 -> [w264]
    tunnel: "Initial Phase Adjustment (GI)" -> [w265]
    tunnel: "Initial Phase Adjustment (AI1)" -> [w266]
    tunnel: [w266] -> w31
    tunnel: [w265] -> w30
    tunnel: [w264] -> w29
    tunnel: [w263] -> w28
    tunnel: [w262] -> w27
    tunnel: [w261] -> w26
    tunnel: [w260] -> w25
    tunnel: [w278] -> w145
    tunnel: [w272] -> w143
    tunnel: "Initial Phase Adjustment (APD Acq)" -> [w271]
    tunnel: "Initial Phase Adjustment (APD 1 Gate)" -> [w270]
    tunnel: "Initial Phase Adjustment (Green FB)" -> [w269]
    tunnel: w31 -> [w277]
    tunnel: w30 -> [w276]
    tunnel: w29 -> [w275]
    tunnel: w28 -> [w274]
    tunnel: w27 -> [w273]
    tunnel: w26 -> [w268]
    tunnel: w25 -> [w267]
    tunnel: w145 -> [w280]
    tunnel: [w281] -> w144
    tunnel: w143 -> [w281]
    tunnel: [w280] -> w142
    tunnel: w144 -> [w284]
    tunnel: w142 -> [w283]
    tunnel: [w286] -> w141
    tunnel: [w285] -> w140
    tunnel: [w288] -> w20
    tunnel: [w289] -> w23
    tunnel: w141 -> [w289]
    tunnel: w140 -> [w288]
    frame #0 {
      n114 = Wait (ms)(milliseconds to wait=u32 1000) -> ()  [unwired: 1 out]
    }
    frame #1 {
      n115 = xnode "Read/Write Control"("FPGA VI Reference In"=w275, "error in"=w274, "Phase count adjustment"=w277, "Phase count adjustment (GI)"=w276, "Phase count adjustment (MCL)"=w273, "Phase Count Adjustment (APD Acq)"=w271, "Phase count adjustment (APD 1 Gate)"=w270, "Phase count adjustment (APD 2 Gate)"=w267, "Phase count adjustment (Green FB)"=w269, "Phase count adjustment (GI) 2"=w268) -> ("FPGA VI Reference Out"=w272:T19, "error out"=w278:errorcluster)
    }
    frame #2 {
      n116 = Wait (ms)(milliseconds to wait=u32 1000) -> ()  [unwired: 1 out]
    }
    frame #3 {
      w282 = TRUE
      n117 = xnode "Read/Write Control"("FPGA VI Reference In"=w284, "error in"=w283, "+ phase"=w282, "+ phase (GI)"=w282, "+ phase (MCL)"=w282, "+ phase (APD Acq)"=w282, "+ phase (APD 1 Gate)"=w282, "+ phase (APD 2 Gate)"=w282, "+ phase (Green FB)"=w282, "+ phase (GI) 2"=w282) -> ("FPGA VI Reference Out"=w285:T19, "error out"=w286:errorcluster)
    }
    frame #4 {
      n118 = Wait (ms)(milliseconds to wait=u32 1000) -> ()  [unwired: 1 out]
    }
  }
  n119 = local read "Phase adj. (Green FB)"() -> (w113:i16)
  n120 = local read "Phase adj. (GI) 2"() -> (w83:i16)
  n121 = local read "Phase adjust (MCL)"() -> (w172:i16)
  n122 = local read "Phase adj. (AI1)"() -> (w174:i16)
  n123 = local read "Phase adj. (GI)"() -> (w173:i16)
  n124 = xnode "Read/Write Control"("FPGA VI Reference In"=w20, "error in"=w23, "Phase count adjustment"=w174, "Phase count adjustment (GI)"=w173, "Phase count adjustment (MCL)"=w172, "Phase Count Adjustment (APD Acq)"="Phase Adj. (APD Acq)", "Phase count adjustment (APD 1 Gate)"="Phase Adj. (APD 1 Gate)", "Phase count adjustment (APD 2 Gate)"="Phase Adj. (APD 2 Gate)", "Phase count adjustment (Green FB)"=w113, "Phase count adjustment (GI) 2"=w83) -> ("FPGA VI Reference Out"=w19:T19, "error out"=w18:errorcluster)
  n125 = call "Initialize RF boards - interlace 3.vi"("error in"=w18, "FPGA VI Reference In"=w19) -> ("FPGA VI Reference Out"=w150:T19)  [unwired: 1 out]
  n126 = call "set RF board frequency - interlace.vi"("Board 2 Frequency Limits"=w116, "Board 1 Frequency Limits"=w118, "FPGA VI Reference In"=w150, "Board 2 Frequency 3 (MHz)"="BD 2 Frequency 3 (MHz)", "Board 1 Frequency 3 (MHz)"="BD 1 Frequency 3 (MHz)", "Board 2 Frequency 2 (MHz)"="BD 2 Frequency 2 (MHz)", "Board 2 Frequency 1 (MHz)"="BD 2 Frequency 1 (MHz)", "Board 1 Frequency 2 (MHz)"="BD 1 Frequency 2 (MHz)", "Board 1 Frequency 1  (MHz)"="BD 1 Frequency 1 (MHz)") -> ("error out"=w244:errorcluster, "FPGA VI Reference Out"=w245:T19)  [unwired: 1 in]
  n127 = call "set RF board amplitude - interlace.vi"("Board 2 Amplitude Limits"=w115, "Board 1 Amplitude Limits"=w117, "error in"=w244, "FPGA VI Reference In"=w245, "Board 2 Amplitude 3 (%)"="BD 2 Amplitude 3 (%)", "Board 1 Amplitude 3 (%)"="BD 1 Amplitude 3 (%)", "Board 2 Amplitude 2 (%)"="BD 2 Amplitude 2 (%)", "Board 2 Amplitude 1 (%)"="BD 2 Amplitude 1 (%)", "Board 1 Amplitude 2 (%)"="BD 1 Amplitude 2 (%)", "Board 1 Amplitude 1 (%)"="BD 1 Amplitude 1 (%)") -> ("error out"=w16:errorcluster, "FPGA VI Reference Out"=w17:T19)
  n128 = flat-sequence {
    tunnel: w17 -> [w298]
    tunnel: w16 -> [w297]
    tunnel: [w296] -> w237
    tunnel: [w295] -> w236
    tunnel: [w302] -> w235
    tunnel: w237 -> [w302]
    tunnel: [w301] -> w234
    tunnel: w236 -> [w301]
    tunnel: w235 -> [w311]
    tunnel: w234 -> [w310]
    tunnel: [w309] -> w12
    tunnel: [w304] -> w11
    tunnel: [w314] -> w40
    tunnel: [w318] -> w24
    tunnel: w12 -> [w318]
    tunnel: w11 -> [w313]
    frame #0 {
      n129 = local read "Trap 1 (ON/OFF)"() -> (w290:bool)
      n130 = xnode "Read/Write Control"("FPGA VI Reference In"=w298, "error in"=w297, "Direct RF Box  Communication"=FALSE) -> ("FPGA VI Reference Out"=w296:T19, "error out"=w295:errorcluster)
      n131 = local write "Saving..."(FALSE ("Saving Data")) -> ()
      n132 = local write "Stop All"(FALSE ("Stop All")) -> ()
      n133 = local write "Index"(1.0 ("Index")) -> ()
      n134 = property on="Trap 1 ON" class="Bool (strict)"("Value"=w290) -> ()  [unwired: 2 in, 2 out]
      "Manipulating Trap" <- FALSE ("Manipulating Trap")
    }
    frame #1 {
      n135 = local read "Trap 2 (ON/OFF)"() -> (w300:bool)
      n136 = Wait (ms)(milliseconds to wait=u32 50) -> ()  [unwired: 1 out]
      n137 = property on="Trap 2 ON" class="Bool (strict)"("Val(Sgnl)"=w300) -> ()  [unwired: 2 in, 2 out]
    }
    frame #2 {
      n138 = local read "Scan Range (nm)"() -> (w305:dbl)
      n139 = xnode "Read/Write Control"("FPGA VI Reference In"=w311, "error in"=w310, "FPGA Controls  RF Box"=TRUE ("Direct RF Box  Communication")) -> ("FPGA VI Reference Out"=w309:T19, "error out"=w304:errorcluster)
      n140 = call "Update messages.vi"("Message to add"="UHR-Fleezers ready.", "Old message string"="") -> ("New message string"=w308:string)
      n141 = local write "Messages"(w308) -> ()
      n142 = property on="Scan Range (nm)" class="DigNum (strict)"("Val(Sgnl)"=w305) -> ()  [unwired: 2 in, 2 out]
    }
    frame #3 {
      n143 = call "hamilton_controller.vi"("error in"=w313, "action"=T20."CONNECT") -> ("error out"=w315:errorcluster)  [unwired: 9 in]
      n144 = call "hamilton_controller.vi"("error in"=w315, "action"=T20."INITIALIZE VALVES") -> ("error out"=w314:errorcluster)  [unwired: 9 in]
    }
  }
  n145 = Subtract(x="BD 1 Frequency 1 (MHz)", y="BD 1 Frequency 2 (MHz)") -> (x-y=w160:dbl)
  n146 = Subtract(x="BD 2 Frequency 1 (MHz)", y="BD 2 Frequency 2 (MHz)") -> (x-y=w159:dbl)
  n147 = Square(x=w159) -> (x^2=w157:dbl)
  n148 = Square(x=w160) -> (x^2=w158:dbl)
  n149 = Add(x=w158, y=w157) -> (x+y=w156:dbl)
  n150 = Square Root(x=w156) -> (sqrt(x)=w155:dbl)
  n151 = local write "Trap Delta (MHz)"(w155) -> ()
  n152 = call "IMAQ Create"("Image Name"="APD 1 Image", "Image Type"=w64) -> ("New Image"=w63:T3)  [unwired: 3 in, 1 out]
  n153 = call "IMAQ Create"("Image Name"="APD 2 Image", "Image Type"=w64) -> ("New Image"=w62:T3)  [unwired: 3 in, 1 out]
  n154 = call "IMAQ Create"("Image Name"="Det. X Image", "Image Type"=w64) -> ("New Image"=w61:T3)  [unwired: 3 in, 1 out]
  n155 = call "IMAQ Create"("Image Name"="Det. Y Image", "Image Type"=w64) -> ("New Image"=w60:T3)  [unwired: 3 in, 1 out]
  n156 = Bundle("New Image"=w63, "New Image"=w62, "New Image"=w61, "New Image"=w60) -> (w59:T21)  [unwired: 1 in]
  n157 = Current VI's Path() -> (path=w1:path)
  n158 = Strip Path(path=w1) -> (stripped path=w2:path)  [unwired: 1 out]
  n159 = Build Path(base path=w2, name or relative path="Locations.txt") -> (appended path=→"Location path":path)
  n160 = Concatenate Strings("N.D.", "\r\n") -> (w5:string)
  n161 = Initialize Array(w5, 4, 3) -> (w8:string[][])
  n162 = local write "Location Matrix"(w8) -> ()
  n163 = while {
    stop <- w319 stop-if-true
    n164 = event shown="[1] \"Goto Top (F6)\": Value Change" {
      selector: _ -> [_ _ _ _ _ _ _]
      dyn-events: _ -> [_ _ _ _ _ _ _]
      timeout: 10 -> [_ _ _ _ _ _ _]
      tunnel: [FALSE _ _ _ _ _ _] -> w319
      event Timeout {
        # "Change the trajectory mode to Jog"
        # "Query and display stage positions"
        # "Setting ESP300 left and right limits for Z-axis, input in mm"
        # "Display Selected Location"
        n165 = local read "ESP Port"() -> (w340:refnum<visa-resource-name>)
        n166 = Concatenate Strings("3SL" ("Substring"), "ESP ZL-Limit", ";3SR", "ESP ZR-Limit", "\r") -> (w339:string)
        n167 = VISA Write(VISA resource name=w340, write buffer=w339) -> ()  [unwired: 1 in, 3 out]
        n168 = local read "Capture Locations"() -> (w344:i32)
        n169 = local read "Location Matrix"() -> (w345:string[][])
        n170 = Index Array(array=w345, index (row)=w344) -> (element=w343:string[])  [unwired: 1 in]
        n171 = Array To Cluster(array=w343) -> (cluster=w342:T22)
        n172 = local write item#485(w342) -> ()
        n173 = event-data() -> ()  [unwired: 1 in, 2 out]
        n174 = disable-structure shown="Disabled" {
          frame Disabled {
            # "Change Low Jog Velocity"
            # "Change High Jog Velocity"
            n175 = Concatenate Strings("1JH" ("Substring"), "Axis 1", "2JH" ("Substring"), "Axis 2", "3JH" ("Substring"), "Axis 3", "\r") -> (w363:string)
            n176 = local read "ESP Port"() -> (w362:refnum<visa-resource-name>)
            n177 = VISA Write(VISA resource name=w362, write buffer=w363) -> ()  [unwired: 1 in, 3 out]
            n178 = Concatenate Strings("1JW" ("Substring"), "Axis 1", "2JW" ("Substring"), "Axis 2", "3JW" ("Substring"), "Axis 3", "\r") -> (w354:string)
            n179 = local read "ESP Port"() -> (w353:refnum<visa-resource-name>)
            n180 = VISA Write(VISA resource name=w353, write buffer=w354) -> ()  [unwired: 1 in, 3 out]
          }
          frame Enabled {
          }
        }
        n181 = local read "ESP Port 8"() -> (w321:refnum<visa-resource-name>)
        n182 = Concatenate Strings("1TJ3;\n2TJ3;\n3TJ3" ("Substring"), "\r") -> (w324:string)
        n183 = VISA Write(VISA resource name=w321, write buffer=w324) -> ()  [unwired: 1 in, 3 out]
        n184 = Concatenate Strings("1TP;\n2TP;\n3TP;\n1MD?;\n2MD?;\n3MD?" ("Substring"), "\r") -> (w328:string)
        n185 = local read "ESP Port"() -> (w331:refnum<visa-resource-name>)
        n186 = VISA Write(VISA resource name=w331, write buffer=w328, error in (no error)="error in") -> (VISA resource name out=w329:refnum<visa-resource-name>, error out=w327:errorcluster)  [unwired: 1 out]
        n187 = case shown="True" TRUE ("Case Constant\n(See Context Help)") {
          tunnel: w329 -> [_ w383]
          tunnel: w327 -> [w364 w382]
          tunnel: [w364 w366] -> w333
          frame False {
          }
          frame True {
            w376 = u16 10 items=["1.0"=10, "1.5"=15, "2.0"=20] ("Serial Settings:Stop Bits")
            w377 = u16 0 items=["None", "Odd", "Even", "Mark", "Space"] ("Serial Settings:Parity")
            n188 = property class="Instr"(reference=w383, error in=w382, "Baud"=u32 921600 ("Serial Settings:Baud Rate"), "Data Bits"=u16 8 ("Serial Settings:Data Bits"), "Parity"=w377, "Stop Bits"=w376) -> (reference out=w381:refnum<visa-resource-name>, error out=w380:errorcluster, "Bytes at Port"=w365:u32)
            n189 = Wait (ms)(milliseconds to wait=u32 10) -> ()  [unwired: 1 out]
            n190 = VISA Read(VISA resource name=w381, byte count=w365, error in (no error)=w380) -> (VISA resource name out=w389:refnum<visa-resource-name>, read buffer=→"X Pos":string, error out=w390:errorcluster)  [unwired: 1 out]
            n191 = VISA Read(VISA resource name=w389, byte count=w365, error in (no error)=w390) -> (VISA resource name out=w387:refnum<visa-resource-name>, read buffer=→"Y Pos":string, error out=w388:errorcluster)  [unwired: 1 out]
            n192 = VISA Read(VISA resource name=w387, byte count=w365, error in (no error)=w388) -> (VISA resource name out=w375:refnum<visa-resource-name>, read buffer=→"Z Pos Pos":string, error out=w374:errorcluster)  [unwired: 1 out]
            n193 = VISA Read(VISA resource name=w375, byte count=w365, error in (no error)=w374) -> (VISA resource name out=w371:refnum<visa-resource-name>, read buffer=→"X Motion":string, error out=w372:errorcluster)  [unwired: 1 out]
            n194 = VISA Read(VISA resource name=w371, byte count=w365, error in (no error)=w372) -> (VISA resource name out=w370:refnum<visa-resource-name>, read buffer=→"Y Motion":string, error out=w368:errorcluster)  [unwired: 1 out]
            n195 = VISA Read(VISA resource name=w370, byte count=w365, error in (no error)=w368) -> (read buffer=→"Z motion":string, error out=w366:errorcluster)  [unwired: 2 out]
          }
        }
        "error out" <- w333
      }
      event "Goto Top (F6)": Value Change {
        n196 = stacked-sequence {
          frame #0 {
            # "stop motions of all axes before going to avoid reversing of direction"
            n197 = local read "ESP Port"() -> (w395:refnum<visa-resource-name>)
            n198 = Concatenate Strings("ST" ("Substring"), "\r") -> (w392:string)
            n199 = VISA Write(VISA resource name=w395, write buffer=w392) -> ()  [unwired: 1 in, 3 out]
          }
          frame #1 {
            n200 = Wait (ms)(milliseconds to wait=u32 50) -> ()  [unwired: 1 out]
          }
          frame #2 {
            # "Change the trajectory mode to Trapezoidal"
            n201 = local read "ESP Port"() -> (w400:refnum<visa-resource-name>)
            n202 = Concatenate Strings("1TJ1;\n2TJ1;\n3TJ1" ("Substring"), "\r") -> (w397:string)
            n203 = VISA Write(VISA resource name=w400, write buffer=w397) -> ()  [unwired: 1 in, 3 out]
          }
          frame #3 {
            # "Go to Top Dispensor"
            n204 = local read "Location Matrix"() -> (w412:string[][])
            n205 = Index Array(array=w412, index (row)=0) -> (element=w408:string[])  [unwired: 1 in]
            n206 = Decimate 1D Array(w408) -> (w406:string[], w404:string[], w402:string[])
            n207 = Concatenate Strings("1PA" ("Substring"), w406, "2PA" ("Substring"), w404, "3PA" ("Substring"), w402, "\r") -> (w410:string)
            n208 = local read "ESP Port"() -> (w409:refnum<visa-resource-name>)
            n209 = VISA Write(VISA resource name=w409, write buffer=w410) -> ()  [unwired: 1 in, 3 out]
          }
          frame #4 {
            n210 = Wait (ms)(milliseconds to wait=u32 100) -> ()  [unwired: 1 out]
          }
          frame #5 {
            # "Change the trajectory mode to Jog"
            n211 = local read "ESP Port 2"() -> (w417:refnum<visa-resource-name>)
            n212 = Concatenate Strings("1TJ3;\n2TJ3;\n3TJ3" ("Substring"), "\r") -> (w414:string)
            n213 = VISA Write(VISA resource name=w417, write buffer=w414) -> ()  [unwired: 1 in, 3 out]
          }
        }
        n214 = event-data() -> ()  [unwired: 1 in, 5 out]
      }
      event "Goto Exp (F8)": Value Change {
        n215 = event-data() -> ()  [unwired: 1 in, 5 out]
        n216 = stacked-sequence {
          frame #0 {
            # "stop motions of all axes before going to avoid reversing of direction"
            n217 = local read "ESP Port"() -> (w421:refnum<visa-resource-name>)
            n218 = Concatenate Strings("ST" ("Substring"), "\r") -> (w418:string)
            n219 = VISA Write(VISA resource name=w421, write buffer=w418) -> ()  [unwired: 1 in, 3 out]
          }
          frame #1 {
            n220 = Wait (ms)(milliseconds to wait=u32 50) -> ()  [unwired: 1 out]
          }
          frame #2 {
            # "Change the trajectory mode to Trapezoidal"
            n221 = local read "ESP Port"() -> (w426:refnum<visa-resource-name>)
            n222 = Concatenate Strings("1TJ1;\n2TJ1;\n3TJ1" ("Substring"), "\r") -> (w423:string)
            n223 = VISA Write(VISA resource name=w426, write buffer=w423) -> ()  [unwired: 1 in, 3 out]
          }
          frame #3 {
            # "Go to Experimental"
            n224 = local read "Location Matrix"() -> (w438:string[][])
            n225 = Index Array(array=w438, index (row)=2) -> (element=w434:string[])  [unwired: 1 in]
            n226 = Decimate 1D Array(w434) -> (w432:string[], w430:string[], w428:string[])
            n227 = Concatenate Strings("1PA" ("Substring"), w432, "2PA" ("Substring"), w430, "3PA" ("Substring"), w428, "\r") -> (w436:string)
            n228 = local read "ESP Port"() -> (w435:refnum<visa-resource-name>)
            n229 = VISA Write(VISA resource name=w435, write buffer=w436) -> ()  [unwired: 1 in, 3 out]
          }
          frame #4 {
            n230 = Wait (ms)(milliseconds to wait=u32 100) -> ()  [unwired: 1 out]
          }
          frame #5 {
            # "Change the trajectory mode to Jog"
            n231 = local read "ESP Port 3"() -> (w440:refnum<visa-resource-name>)
            n232 = Concatenate Strings("1TJ3;\n2TJ3;\n3TJ3" ("Substring"), "\r") -> (w443:string)
            n233 = VISA Write(VISA resource name=w440, write buffer=w443) -> ()  [unwired: 1 in, 3 out]
          }
        }
      }
      event "Goto Bottom (F7)": Value Change {
        n234 = stacked-sequence {
          frame #0 {
            # "stop motions of all axes before going to avoid reversing of direction"
            n235 = local read "ESP Port"() -> (w447:refnum<visa-resource-name>)
            n236 = Concatenate Strings("ST" ("Substring"), "\r") -> (w444:string)
            n237 = VISA Write(VISA resource name=w447, write buffer=w444) -> ()  [unwired: 1 in, 3 out]
          }
          frame #1 {
            n238 = Wait (ms)(milliseconds to wait=u32 50) -> ()  [unwired: 1 out]
          }
          frame #2 {
            # "Change the trajectory mode to Trapezoidal"
            n239 = local read "ESP Port"() -> (w452:refnum<visa-resource-name>)
            n240 = Concatenate Strings("1TJ1;\n2TJ1;\n3TJ1" ("Substring"), "\r") -> (w449:string)
            n241 = VISA Write(VISA resource name=w452, write buffer=w449) -> ()  [unwired: 1 in, 3 out]
          }
          frame #3 {
            # "Go to Bottom Dispensor"
            n242 = local read "Location Matrix"() -> (w464:string[][])
            n243 = Index Array(array=w464, index (row)=1) -> (element=w460:string[])  [unwired: 1 in]
            n244 = Decimate 1D Array(w460) -> (w458:string[], w456:string[], w454:string[])
            n245 = Concatenate Strings("1PA" ("Substring"), w458, "2PA" ("Substring"), w456, "3PA" ("Substring"), w454, "\r") -> (w462:string)
            n246 = local read "ESP Port"() -> (w461:refnum<visa-resource-name>)
            n247 = VISA Write(VISA resource name=w461, write buffer=w462) -> ()  [unwired: 1 in, 3 out]
          }
          frame #4 {
            n248 = Wait (ms)(milliseconds to wait=u32 100) -> ()  [unwired: 1 out]
          }
          frame #5 {
            # "Change the trajectory mode to Jog"
            n249 = local read "ESP Port 4"() -> (w466:refnum<visa-resource-name>)
            n250 = Concatenate Strings("1TJ3;\n2TJ3;\n3TJ3" ("Substring"), "\r") -> (w469:string)
            n251 = VISA Write(VISA resource name=w466, write buffer=w469) -> ()  [unwired: 1 in, 3 out]
          }
        }
        n252 = event-data() -> ()  [unwired: 1 in, 5 out]
      }
      event "Capture": Value Change {
        n253 = event-data() -> ()  [unwired: 1 in, 5 out]
        n254 = local read "Capture Locations"() -> (w470:i32)
        n255 = local read "Z Pos Pos"() -> (w471:string)
        n256 = local read "X Pos"() -> (w473:string)
        n257 = local read "Y Pos"() -> (w472:string)
        n258 = case shown="1" w470 {
          selector: w470 -> [w477 w484 w491 w498]
          tunnel: w473 -> [w480 w487 w494 w501]
          tunnel: w472 -> [w479 w486 w493 w500]
          tunnel: w471 -> [w478 w485 w492 w499]
          frame 0, Default {
            # "Capture Top Dispensor Location"
            n259 = local read "Location Matrix"() -> (w476:string[][])
            n260 = Build Array(w480, w479, w478) -> (w475:string[])
            n261 = Replace Array Subset(array=w476, new element=w475, index (row)=w477) -> (w474:string[][])  [unwired: 1 in]
            n262 = local write "Location Matrix"(w474) -> ()
          }
          frame 1 {
            # "Capture Bottom Dispensor Location"
            n263 = local read "Location Matrix"() -> (w483:string[][])
            n264 = Build Array(w487, w486, w485) -> (w482:string[])
            n265 = Replace Array Subset(array=w483, new element=w482, index (row)=w484) -> (w481:string[][])  [unwired: 1 in]
            n266 = local write "Location Matrix"(w481) -> ()
          }
          frame 2 {
            # "Capture Experimental Region Location"
            n267 = local read "Location Matrix"() -> (w490:string[][])
            n268 = Build Array(w494, w493, w492) -> (w489:string[])
            n269 = Replace Array Subset(array=w490, new element=w489, index (row)=w491) -> (w488:string[][])  [unwired: 1 in]
            n270 = local write "Location Matrix"(w488) -> ()
          }
          frame 3 {
            # "Capture Other Location"
            n271 = local read "Location Matrix"() -> (w497:string[][])
            n272 = Build Array(w501, w500, w499) -> (w496:string[])
            n273 = Replace Array Subset(array=w497, new element=w496, index (row)=w498) -> (w495:string[][])  [unwired: 1 in]
            n274 = local write "Location Matrix"(w495) -> ()
          }
        }
      }
      event "Save": Value Change {
        # "reshape Location Matrix to 1-D array to write"
        n275 = event-data() -> ()  [unwired: 1 in, 5 out]
        n276 = local read "Location Matrix"() -> (w505:string[][])
        n277 = local read "Location path"() -> (w502:path)
        n278 = Reshape Array(w505, 12) -> (w503:string[])
        n279 = Write to Text File(file (use dialog)=w502, text=w503) -> ()  [unwired: 2 in, 3 out]
      }
      event "Activate Joystick": Value Change {
        # "Change the trajectory mode to Jog"
        n280 = disable-structure shown="Disabled" {
          frame Disabled {
            n281 = case shown="True" "Activate Joystick" {
              frame False {
              }
              frame True {
                # "Change the trajectory mode to Jog"
                n282 = local read "ESP Port"() -> (w514:refnum<visa-resource-name>)
                n283 = Concatenate Strings("1TJ3;\n2TJ3;\n3TJ3" ("Substring"), "\r") -> (w511:string)
                n284 = VISA Write(VISA resource name=w514, write buffer=w511) -> ()  [unwired: 1 in, 3 out]
              }
            }
          }
          frame Enabled {
          }
        }
        n285 = local read "ESP Port 5"() -> (w509:refnum<visa-resource-name>)
        n286 = event-data() -> ()  [unwired: 1 in, 5 out]
        n287 = Concatenate Strings("1TJ3;\n2TJ3;\n3TJ3" ("Substring"), "\r") -> (w506:string)
        n288 = VISA Write(VISA resource name=w509, write buffer=w506) -> ()  [unwired: 1 in, 3 out]
      }
    }
  }
  n289 = disable-structure shown="Disabled" {
    disable-tunnel: w24 -> [w543 _]
    frame Disabled {
      w538 = T17 0 items=["Grayscale (U8)", "Grayscale (I16)", "Grayscale (SGL)", "Complex (CSG)", "RGB (U32)", "HSL (U32)", "RGB (U64)", "Grayscale (U16)"] ("Image Type")
      n290 = call <vilib>:"IMAQ Init.vi"("Interface Name"="img0") -> ("error out"=w540:errorcluster, "IMAQ Session Out"=w542:refnum<k11>)  [unwired: 9 in]
      n291 = call <vilib>:"IMAQ Grab Setup.vi"("error in (no error)"=w540, "IMAQ Session In"=w542) -> ("error out"=w536:errorcluster, "IMAQ Session Out"=w537:refnum<k11>)  [unwired: 8 in]
      n292 = call "IMAQ Create"("Image Name"="untitled", "Image Type"=w538) -> ("New Image"=w535:T3)  [unwired: 3 in, 1 out]
      n293 = call <vilib>:"Application Directory.vi"() -> ("Application Directory"=w522:path)
      n294 = Build Path(base path=w522, name or relative path="_trap_screen_positions") -> (appended path=w530:path)
      n295 = Open/Create/Replace File(file path (use dialog)=w530, operation (0:open)=T23."open or create", access (0:read/write)=enum16{"read/write", "read-only", "write-only"}."read/write") -> (refnum out=w532:refnum<file>)  [unwired: 3 in, 2 out]
      n296 = local read "Trap Sets"() -> (w524:u32)
      n297 = for "Load trap positions on video screen from file." {
        N: w524 -> [_]
        tunnel: [w550] -> w525
        tunnel: w532 -> [w549]
        tunnel: [w546] -> w521 mode=indexing
        w548 = 4
        n298 = for {
          N: w548 -> [_]
          tunnel: [w554] -> w550
          tunnel: w549 -> [w553]
          tunnel: w548 -> [w552]
          tunnel: [w551] -> w547 mode=indexing
          n299 = Read from Binary File(5:w552, 11:w553) -> (2:w551:i32, 3:w554:refnum<file>)  [unwired: 4 in, 2 out]
        }
        n300 = Array To Cluster(array=w547) -> (cluster=w546:T27)
      }
      n301 = node-c288() -> (w545:T24)  [unwired: 4 in]
      n302 = timed-loop "acquire video and stage position" {
        timing: w545 -> [_]
        timing-out: [_] -> w544
        tunnel: w537 -> [w573]
        tunnel: w536 -> [w572]
        tunnel: w535 -> [w571]
        tunnel: [w570] -> w517
        tunnel: [w567] -> w518
        tunnel: [w568] -> w516
        tunnel: w543 -> [_]
        shift-right: [w564] -> w534
        shift-left: w521 -> [w565]
        tunnel: w524 -> [w562]
        stop <- w569 stop-if-true
        n303 = node-c288() -> ()  [unwired: 1 in, 1 out]
        n304 = event shown="[0] Timeout" {
          selector: _ -> [_ _ _ _]
          dyn-events: _ -> [_ _ _ _]
          timeout: 10 -> [_ _ _ _]
          tunnel: w573 -> [w584 w599 w608 w627]
          tunnel: w572 -> [w583 w601 w606 w629]
          tunnel: w571 -> [w582 w600 w607 w628]
          tunnel: [w581 w599 w608 w627] -> w570
          tunnel: [w574 w603 FALSE FALSE] -> w569
          tunnel: [w578 w601 w606 w629] -> w568
          tunnel: [w577 w600 w607 w628] -> w567
          tunnel: "radius" -> [_ _ w613 _]
          tunnel: w565 -> [w575 w602 w611 _]
          tunnel: [w575 w602 w612 cluster{i32, i32, i32, i32}[] []] -> w564
          tunnel: w562 -> [_ _ w604 _]
          event Timeout {
            n305 = event-data() -> ()  [unwired: 1 in, 2 out]
            n306 = call <vilib>:"IMAQ Grab Acquire.vi"("error in (no error)"=w583, "Image In"=w582, "IMAQ Session In"=w584) -> ("error out"=w579:errorcluster, "Image Out"=w580:T3, "IMAQ Session Out"=w581:refnum<k11>)  [unwired: 5 in, 1 out]
            n307 = case shown="True" "trap\nmarkers?" {
              tunnel: w575 -> [_ w592]
              tunnel: w580 -> [w586 w591]
              tunnel: w579 -> [w585 w590]
              tunnel: [w585 w589] -> w578
              tunnel: [w586 w587] -> w577
              frame False {
              }
              frame True {
                n308 = for {
                  tunnel: w592 -> [w598] mode=indexing
                  shift-right: [w596] -> w587
                  shift-left: w591 -> [w597]
                  tunnel: w590 -> [w595]
                  tunnel: [w594] -> w589
                  tunnel: u32 16711680 ("Color") -> [w593]
                  n309 = call "IMAQ Overlay Oval"("Color"=w593, "error in (no error)"=w595, "Bounding Rectangle"=w598, "Image"=w597) -> ("error out"=w594:errorcluster, "Image Out"=w596:T3)  [unwired: 6 in]
                }
              }
            }
            "Primary Video Display" <- w577
            n310 = Unbundle By Name(w579) -> ("status"=w574:bool)
          }
          event "Stop All": Value Change {
            n311 = event-data() -> ()  [unwired: 1 in, 5 out]
            n312 = local read "Stop All"() -> (w603:bool)
          }
          event "Primary Video Display": Mouse Down {
            n313 = event-data() -> ()  [unwired: 1 in, 7 out]
            n314 = Array Size(array=w611) -> (size(s)=w610:i32)
            n315 = Less?(x=w610, y=w604) -> (x < y?=w609:bool)
            n316 = case shown="True" w609 {
              tunnel: w613 -> [_ w623]
              tunnel: w611 -> [w614 w617]
              tunnel: [w614 w616] -> w612
              frame False {
              }
              frame True {
                n317 = property on="Primary Video Display" class="ImageControl"() -> ("Last Mouse Position"=w615:cluster{"X":i32, "Y":i32})  [unwired: 2 in, 2 out]
                n318 = Unbundle By Name(w615) -> ("X"=w625:i32, "Y"=w624:i32)
                n319 = Add(x=w624, y=w623) -> (x+y=w621:i32)
                n320 = Subtract(x=w624, y=w623) -> (x-y=w619:i32)
                n321 = Add(x=w625, y=w623) -> (x+y=w620:i32)
                n322 = Subtract(x=w625, y=w623) -> (x-y=w622:i32)
                n323 = Bundle(w622, w621, w620, w619) -> (w618:cluster{i32, i32, i32, i32})  [unwired: 1 in]
                n324 = Build Array (concatenate)(w617, w618) -> (w616:T28)
              }
            }
          }
          event "clear markers": Value Change {
            n325 = event-data() -> ()  [unwired: 1 in, 5 out]
          }
        }
        n326 = node-c288() -> ()  [unwired: 1 in, 1 out]
      }
      n327 = node-c288(w544) -> ()  [unwired: 1 out]
      n328 = Set File Position(offset (in bytes) (0)=i64 0, refnum=w525, from (0:start)=enum16{"start", "end", "current"}."start") -> (refnum out=w526:refnum<file>)  [unwired: 1 in, 1 out]
      n329 = for "Write trap positions to file so they can be remembered\nwhen program is removed from memory" {
        tunnel: w534 -> [w558] mode=indexing
        tunnel: [w556] -> w533
        tunnel: w526 -> [w555]
        n330 = Cluster To Array(cluster=w558) -> (array=w557:i32[])
        n331 = for {
          tunnel: w557 -> [w561] mode=indexing
          tunnel: [w560] -> w556
          tunnel: w555 -> [w559]
          n332 = Write to Binary File(file (use dialog)=w559, data=w561) -> (refnum out=w560:refnum<file>)  [unwired: 4 in, 2 out]
        }
      }
      n333 = Close File(refnum=w533) -> ()  [unwired: 1 in, 2 out]
      n334 = call "IMAQ Dispose"("Image"=w518, "error in (no error)"=w516) -> ("error out"=w515:errorcluster)  [unwired: 4 in]
      n335 = call <vilib>:"IMAQ Stop.vi"("error in (no error)"=w515, "IMAQ Session In"=w517) -> ("error out"=w519:errorcluster, "IMAQ Session Out"=w520:refnum<k11>)  [unwired: 8 in]
      n336 = call <vilib>:"IMAQ Close.vi"("error in (no error)"=w519, "IMAQ Session In"=w520) -> ()  [unwired: 9 in, 1 out]
    }
    frame Enabled {
    }
  }
  n337 = disable-structure shown="Enabled" {
    disable-tunnel: [w636 _] -> w35
    disable-tunnel: w24 -> [w635 _]
    frame Enabled {
      n338 = node-c288() -> (w638:T24)  [unwired: 4 out]
      n339 = timed-loop "Rough control of MCL mirror stage (debugging)" {
        tunnel: w635 -> [w641]
        tunnel: [w640] -> w636
        timing: w638 -> [_]
        timing-out: [_] -> w637
        stop <- w640 stop-if-true
        n340 = node-c288() -> ()  [unwired: 2 out]
        n341 = case shown="1" "MCL Mode" {
          tunnel: w641 -> [_ w644 w691]
          frame 0, Default {
            # "manual positioning"
          }
          frame 1 {
            # "sinusoidal wave"
            n342 = node-c288() -> (w646:T24)  [unwired: 4 out]
            n343 = timed-loop "Oscillate MCL mirror" {
              timing: w646 -> [_]
              timing-out: [_] -> w645
              tunnel: w644 -> [w685]
              i -> [w684]
              stop <- w647 stop-if-true
              n344 = node-c288() -> (w683:i64)  [unwired: 1 out]
              n345 = Multiply(x="AO1", y=32767.0) -> (x*y=w679:dbl)
              n346 = Multiply(x="AO2", y=32767.0) -> (x*y=w674:dbl)
              n347 = Divide(x=w679, y=10.0) -> (x/y=w680:dbl)
              n348 = Divide(x=w674, y=10.0) -> (x/y=w675:dbl)
              n349 = To Word Integer(number=w680) -> (16bit integer=w672:i16)
              n350 = To Word Integer(number=w675) -> (16bit integer=w671:i16)
              n351 = Divide(x=w683, y=i64 1000) -> (x/y=w654:dbl)
              n352 = Multiply(x=w654, y=w684) -> (x*y=w665:dbl)
              n353 = Multiply(x="Osc. freq. (Hz) 2", y=6.283185307179586) -> (x*y=w666:dbl)
              n354 = Multiply(x=w666, y=w665) -> (x*y=w664:dbl)
              n355 = Sine(x=w664) -> (sin(x)=w663:dbl)
              n356 = Multiply(x=w663, y="Osc. amp. (V)") -> (x*y=w661:dbl)
              n357 = Add(x=w661, y="Osc. center (V)") -> (x+y=w659:dbl)
              n358 = Divide(x=w659, y=10.0) -> (x/y=w657:dbl)
              n359 = Multiply(x=w657, y=32767.0) -> (x*y=w652:dbl)
              n360 = Select(t=w652, s="Scan axis", f=w672) -> (s? t:f=w670:dbl)
              n361 = Select(t=w671, s="Scan axis", f=w652) -> (s? t:f=w669:dbl)
              n362 = local read "MCL Mode"() -> (w651:u16)
              n363 = Not Equal?(x=w651, y=u16 1) -> (x != y?=w648:bool)
              n364 = local read "Stop All"() -> (w649:bool)
              n365 = xnode "Read/Write Control"("FPGA VI Reference In"=w685, "AO1"=w670, "AO2"=w669) -> ()  [unwired: 1 in, 2 out]
              n366 = Compound Arithmetic op=OR(w649, w648) -> (w647:bool)
              n367 = node-c288() -> ()  [unwired: 2 out]
            }
            n368 = node-c288(w645) -> ()  [unwired: 1 out]
          }
          frame 2 {
            # "linear scan"
            n369 = case shown="True" "Start Scan" {
              tunnel: w691 -> [_ w703]
              frame False {
              }
              frame True {
                n370 = Subtract(x="End (V)", y="Begin (V)") -> (x-y=w699:dbl)
                n371 = Decrement(x="N Points") -> (x-1=w698:dbl)
                n372 = Divide(x=w699, y=w698) -> (x/y=w696:dbl)
                n373 = for {
                  N: "N Points" -> [_]
                  tunnel: "Begin (V)" -> [w716]
                  tunnel: w703 -> [w708]
                  tunnel: [w707] -> w702 mode=indexing
                  tunnel: w696 -> [w706]
                  tunnel: [w704] -> w695 mode=indexing
                  i -> [w715]
                  n374 = Multiply(x=w706, y=w715) -> (x*y=w714:dbl)
                  n375 = Add(x=w716, y=w714) -> (x+y=w711:dbl)
                  n376 = local read "Scan axis"() -> (w705:bool)
                  n377 = local read "AO1"() -> (w713:dbl)
                  n378 = local read "AO2"() -> (w712:dbl)
                  n379 = Select(t=w711, s=w705, f=w713) -> (s? t:f=w710:dbl)
                  n380 = Select(t=w712, s=w705, f=w711) -> (s? t:f=w709:dbl)
                  n381 = flat-sequence {
                    tunnel: w710 -> [w720]
                    tunnel: w709 -> [w719]
                    tunnel: w708 -> [w717]
                    tunnel: [w730] -> w707
                    tunnel: [w729] -> w704
                    frame #0 {
                      w723 = 10.0 ("y")
                      w718 = 32767.0 ("y")
                      n382 = Multiply(x=w720, y=w718) -> (x*y=w726:dbl)
                      n383 = Multiply(x=w719, y=w718) -> (x*y=w724:dbl)
                      n384 = Divide(x=w726, y=w723) -> (x/y=w727:dbl)
                      n385 = Divide(x=w724, y=w723) -> (x/y=w725:dbl)
                      n386 = To Word Integer(number=w727) -> (16bit integer=w721:i16)
                      n387 = To Word Integer(number=w725) -> (16bit integer=w722:i16)
                      n388 = xnode "Read/Write Control"("FPGA VI Reference In"=w717, "AO1"=w721, "AO2"=w722) -> ()  [unwired: 1 in, 2 out]
                    }
                    frame #1 {
                      n389 = Wait (ms)(milliseconds to wait="DAQ Delay (ms)") -> ()  [unwired: 1 out]
                    }
                    frame #2 {
                      n390 = local read "Slow mean"() -> (w730:dbl)
                      n391 = local read "Sigma"() -> (w729:dbl)
                    }
                  }
                }
                n392 = Bundle("Begin (V)"="Begin (V)", w696, w702) -> (→"MCL Scan":cluster{"Begin (V)":dbl, dbl, dbl[]})  [unwired: 1 out]
                n393 = Bundle("Begin (V)"="Begin (V)", w696, w695) -> (→"MCL Scan 2":cluster{"Begin (V)":dbl, dbl, dbl[]})  [unwired: 1 out]
              }
            }
          }
        }
        n394 = local read "Stop All"() -> (w640:bool)
        n395 = node-c288() -> ()  [unwired: 2 out]
      }
      n396 = node-c288(w637) -> ()  [unwired: 1 out]
    }
    frame Disabled {
    }
  }
  n397 = node-c288(2 ("Processor")) -> (w15:T24)  [unwired: 3 in]
  n398 = node-c288() -> (w69:T24)  [unwired: 4 in]
  n399 = timed-loop "Control parameters (event loop)" {
    tunnel: w24 -> [w736]
    shift-right: [w735] -> _
    shift-left: errorcluster {"status"=FALSE, "code"=0, "source"=""} ("error out") -> [w734]
    tunnel: [w733] -> w37
    timing: w15 -> [_]
    timing-out: [_] -> w14
    stop <- w733 stop-if-true
    n400 = node-c288() -> ()  [unwired: 1 in, 1 out]
    n401 = event shown="[6] \"BD 1 Frequency 1 (MHz)\", \"BD 1 Frequency 2 (MHz)\", \"BD 1 Frequency 3 (MHz)\", \"BD 2 Frequency 1 (MHz)\", \"BD 2 Frequency 2 (MHz)\", \"BD 2 Frequency 3 (MHz)\", \"Trap Delta (MHz)\": Value Change" {
      selector: _ -> [_ _ _ _ _ _ _ _ _ _ _ _ _ _ _ _ _ _ _ _ _ _ _ _ _ _ _ _ _ _ _ _ _ _ _ _ _ _ _ _ _ _ _ _ _ _ _ _ _ _ _ _ _ _ _ _]
      dyn-events: _ -> [_ _ _ _ _ _ _ _ _ _ _ _ _ _ _ _ _ _ _ _ _ _ _ _ _ _ _ _ _ _ _ _ _ _ _ _ _ _ _ _ _ _ _ _ _ _ _ _ _ _ _ _ _ _ _ _]
      timeout: _ -> [_ _ _ _ _ _ _ _ _ _ _ _ _ _ _ _ _ _ _ _ _ _ _ _ _ _ _ _ _ _ _ _ _ _ _ _ _ _ _ _ _ _ _ _ _ _ _ _ _ _ _ _ _ _ _ _]
      tunnel: w736 -> [w774 _ _ _ w811 _ w833 _ w900 _ _ _ w943 _ _ w986 w992 w997 w1003 w1039 w1057 w1064 w1082 w1093 w1104 w1115 w1126 w1137 w1155 w1161 w1255 _ w1264 w1302 _ w1337 w1341 w1352 w1356 w1360 _ w1368 _ _ _ _ _ w1504 _ w1521 w1524 w1533 w1536 w1540 _ w1557]
      tunnel: [w773 _ _ _ w801 _ w832 _ w863 _ w908 _ w922 _ _ w985 w988 w994 w1000 w1038 w1055 w1063 w1076 w1087 w1098 w1109 w1120 w1131 w1153 w1160 w1253 _ w1262 w1300 _ w1335 w1339 w1342 w1354 w1358 _ w1366 _ _ _ _ _ w1502 _ _ _ _ _ _ _ _] -> w735
      tunnel: w734 -> [w772 _ _ _ w810 _ w831 _ w895 _ w908 _ w942 _ _ w984 w987 w993 w999 w1037 w1056 w1062 w1081 w1092 w1103 w1114 w1125 w1136 w1154 w1159 w1254 _ w1263 w1301 _ w1336 w1340 w1351 w1355 w1359 _ w1367 _ _ _ _ _ w1503 _ w1520 w1523 w1532 w1535 w1539 _ w1556]
      tunnel: [_ _ _ _ _ _ _ _ _ _ w907 _ _ _ _ _ _ _ _ _ _ _ _ _ _ _ _ _ _ _ _ _ _ _ _ _ _ _ _ _ _ _ _ _ _ _ _ _ _ _ _ _ _ _ _ _] -> w733
      tunnel: [_ _ _ _ _ _ _ "Round T1 X" _ _ _ _ _ _ _ _ _ _ _ _ _ _ _ _ _ _ _ _ _ _ _ _ _ _ _ _ _ _ _ _ _ _ _ _ _ _ _ _ _ _ _ _ _ _ _ _] -> _
      tunnel: [_ _ _ "Adjust Scale\nto Mean" _ _ _ _ _ _ _ _ _ _ _ _ _ _ _ _ _ _ _ _ _ _ _ _ _ _ _ _ _ _ _ _ _ _ _ _ _ _ _ _ _ _ _ _ _ _ _ _ _ "Set SP to Reading" _ _] -> _
      tunnel: [_ _ _ _ _ _ _ _ _ "Round T2 X" _ "Delayed Interlace Start" _ _ _ _ _ _ _ _ _ _ _ _ _ _ _ _ _ _ _ _ _ _ _ _ _ _ _ _ _ _ _ _ _ _ _ _ _ _ _ _ _ _ _ _] -> _
      event "AI Count (ticks)", "Sets to FIFO (Traps)", "Save ave N", "FPGA Ave.", "# Samples/channel", "N sets to save": Value Change {
        # "So that if 'Save ave N' is updated, the AOD scanning code updates too."
        n402 = event-data() -> ()  [unwired: 6 out]
        n403 = local read "AI Count (ticks)"() -> (w754:u32)
        n404 = Boolean To (0,1)(Boolean="Sets to FIFO (Traps)") -> (0, 1=w764:cluster{"Set 1":i16, "Set 2":i16, "Set 3":i16})
        n405 = xnode "Read/Write Control"("FPGA VI Reference In"=w774, "error in"=w772, "ai count"=w754, "AI1 Sets to FIFO"="Sets to FIFO (Traps)", "N of AI1 Int Acq Sets"="N Acq Sets (Traps + Fl.)") -> ("error out"=w773:errorcluster)  [unwired: 1 out]
        n406 = Cluster To Array(cluster=w764) -> (array=w763:i16[])
        n407 = To Unsigned Long Integer(number=w763) -> (unsigned 32bit integer=w743:u32[])
        n408 = local read "Scan steps (AOD)"() -> (w765:u64)
        n409 = Multiply(x=w754, y="N Acq Sets (Traps + Fl.)") -> (x*y=w752:u32)
        n410 = Divide(x=40000000.0, y=w754) -> (x/y=w746:dbl)
        "AI rate (Hz)" <- w746
        "Ave. Rate (Hz)" <- w746
        n411 = Add Array Elements(numeric array=w743) -> (sum=w755:u32)
        "Trap Sets" <- w755
        n412 = Reciprocal(x=w746) -> (1/x=→"Ave. Period (s)":dbl)
        n413 = property on="Scan steps (AOD)" class="DigNum (strict)"("Val(Sgnl)"=w765) -> ()  [unwired: 2 in, 2 out]
        n414 = Divide(x=w746, y="N Acq Sets (Traps + Fl.)") -> (x/y=w769:dbl)
        "Data Rate (Hz)" <- w769
        n415 = Reciprocal(x=w769) -> (1/x=→"Data Period (s)":dbl)
        n416 = local read "Save ave N"() -> (w768:dbl)
        n417 = Divide(x=w769, y=w768) -> (x/y=w767:dbl)
        "Save Data Rate (Hz)" <- w767
        n418 = Reciprocal(x=w767) -> (1/x=→"Save Data Period (s)":dbl)
        n419 = Multiply(x=w752, y="# Samples/trap") -> (x*y=w750:u32)
        "Counts/DMA" <- w750
        n420 = property on="Trap Disp. Downsample" class="DigNum (strict)"("Maximum"="# Samples/trap") -> ()  [unwired: 2 in, 2 out]
        n421 = Multiply(x=w755, y="# Samples/trap") -> (x*y=w744:u32)
        "# Samples/channel" <- w744
        n422 = Multiply(x=w744, y=u32 8) -> (x*y=→"Trap AI Elements/DMA read":u32)
        n423 = local read "APD Int. Count"() -> (w751:u32)
        n424 = Multiply(x=w744, y=u32 3) -> (x*y=→"Trap Pos Elements/DMA read":u32)
        n425 = Divide(x=w750, y=w751) -> (x/y=w741:dbl)
        "APD Samples/FIFO Acq." <- w741
        n426 = Divide(x=w750, y=40000000.0) -> (x/y=w748:dbl)
        "DMA Update Period (s)" <- w748
        n427 = Multiply(x=2.0, y=w741) -> (x*y=→"APD Elements/DMA read":dbl)
        n428 = property on="APD Disp. Downsample" class="DigNum (strict)"("Maximum"=w741) -> ()  [unwired: 2 in, 2 out]
        n429 = local read "N sets to save"() -> (w761:u32)
        n430 = Multiply(x=w748, y=w761) -> (x*y=→"Total Time (s)":dbl)
        "FPGA Averaging" <- FALSE ("FPGA Averaging")
      }
      event "Rescale on Mean": Value Change {
        n431 = event-data() -> ()  [unwired: 7 out]
        n432 = And(x=FALSE, y="Rescale on Mean") -> (x .and. y?=w776:bool)
        n433 = local write "Rescale on Mean"(w776) -> ()
        n434 = local read "Bead Mean (nm)"() -> (w781:dbl)
        n435 = Add(x="Amplitude (nm)", y=w781) -> (x+y=w779:dbl)
        n436 = Subtract(x=w781, y="Amplitude (nm)") -> (x-y=w778:dbl)
        n437 = property on="Bead Separation" class="WFChart (strict)"("YScale.Minimum"=w778) -> ()  [unwired: 2 in, 2 out]
        n438 = property on="Bead Separation" class="WFChart (strict)"("YScale.Maximum"=w779) -> ()  [unwired: 2 in, 2 out]
      }
      event "Detector Type": Value Change {
        n439 = event-data() -> ()  [unwired: 7 out]
        n440 = local read "AI labels"() -> (w782:string[])
        n441 = property on="High Res. Display" class="Ring (strict)"("Strings []"=w782) -> ()  [unwired: 2 in, 2 out]
        n442 = Build Array (concatenate)(w782, "none") -> (w783:string[])
        n443 = property on="FFT 1 Choice 1" class="Ring (strict)"("Strings []"=w783) -> ()  [unwired: 2 in, 2 out]
        n444 = property on="FFT 1 Choice 2" class="Ring (strict)"("Strings []"=w783) -> ()  [unwired: 2 in, 2 out]
        n445 = property on="FFT 2 Choice 1" class="Ring (strict)"("Strings []"=w783) -> ()  [unwired: 2 in, 2 out]
        n446 = property on="FFT 2 Choice 2" class="Ring (strict)"("Strings []"=w783) -> ()  [unwired: 2 in, 2 out]
        n447 = Bundle("APD 1", "APD 2") -> (w786:cluster{string, string})  [unwired: 1 out]
        n448 = Cluster To Array(cluster=w786) -> (array=w784:string[])
        n449 = Build Array (concatenate)(w784, w783) -> (w788:string[])
        n450 = Array Size(array=w788) -> (size(s)=w789:i32)
        n451 = property on="Signals to Plot" class="LstBox (strict)"("Item Names"=w788) -> ()  [unwired: 2 in, 2 out]
        n452 = property on="Signals to Plot" class="LstBox (strict)"("Number of Rows"=w789) -> ()  [unwired: 2 in, 2 out]
        n453 = property on="All Signals" class="WFChart (strict)"("LegNumRows"=w789) -> ()  [unwired: 2 in, 2 out]
      }
      event "Adjust Scale\nto Mean": Value Change {
        n454 = event-data() -> ()  [unwired: 7 out]
        n455 = local read "APD 1 Rate (Hz)"() -> (w798:dbl)
        n456 = Multiply(x=1000.0, y="Above (kHz)") -> (x*y=w796:dbl)
        n457 = Multiply(x=1000.0, y="Below (kHz)") -> (x*y=w794:dbl)
        n458 = Add(x=w796, y=w798) -> (x+y=w791:dbl)
        n459 = Subtract(x=w798, y=w794) -> (x-y=w792:dbl)
        n460 = property on="APD Chart" class="WFChart (strict)"("YScale.Minimum"=w792) -> ()  [unwired: 2 in, 2 out]
        n461 = property on="APD Chart" class="WFChart (strict)"("YScale.Maximum"=w791) -> ()  [unwired: 2 in, 2 out]
      }
      event "Phase adj. (AI1)", "+ phase (AI1)", "- phase (AI1)": Value Change {
        n462 = event-data() -> ()  [unwired: 7 out]
        n463 = Negate(x="Phase adj. (AI1)") -> (-x=w808:i16)
        n464 = Select(t=w808, s="- phase (AI1)", f="Phase adj. (AI1)") -> (s? t:f=w807:i16)
        n465 = xnode "Read/Write Control"("FPGA VI Reference In"=w811, "error in"=w810, "Phase count adjustment"=w807) -> ("FPGA VI Reference Out"=w806:T19, "error out"=w805:errorcluster)
        n466 = Or(x="- phase (AI1)", y="+ phase (AI1)") -> (x .or. y?=w802:bool)
        n467 = xnode "Read/Write Control"("FPGA VI Reference In"=w806, "error in"=w805, "+ phase"=w802) -> ("error out"=w801:errorcluster)  [unwired: 1 out]
      }
      event "Signals to Plot": Double Click {
        w814 = u32 9868950 ("Color Box")
        n468 = event-data() -> ("Row"=w816:i32)  [unwired: 9 out]
        n469 = property on="All Signals" class="WFChart (strict)"("Active Plot"=w816) -> (error out=w827:errorcluster)  [unwired: 2 in, 1 out]
        n470 = property on="All Signals" class="WFChart (strict)" props=["Plot", "Visible?", "Plot", "Plot Color"](error in=w827) -> (error out=w826:errorcluster, "Plot.Visible?"=w825:bool)  [unwired: 1 in, 2 out]
        n471 = Select(t=FALSE ("Plot.Visible"), s=w825, f=TRUE ("Plot.Visible")) -> (s? t:f=w820:bool)
        n472 = property on="All Signals" class="WFChart (strict)"(error in=w826, "Plot.Visible?"=w820) -> (error out=w822:errorcluster)  [unwired: 1 in, 1 out]
        n473 = property on="All Signals" class="WFChart (strict)"(error in=w822) -> (error out=w817:errorcluster, "Plot.Plot Color"=w821:u32)  [unwired: 1 in, 1 out]
        n474 = property on="Signals to Plot" class="LstBox (strict)"(error in=w817, "Active Row"=w816) -> (error out=w815:errorcluster)  [unwired: 1 in, 1 out]
        n475 = Select(t=w821, s=w820, f=u32 0) -> (s? t:f=w818:u32)
        n476 = property on="Signals to Plot" class="LstBox (strict)"(error in=w815, "CellFontColor"=w818, "SelColor"=w814, "CellBG"=w814, "CellFontSize"=u32 20 ("Active Row:Cell Font:Size"), "CellFontBold"=TRUE ("Active Row:Cell Font:Bold")) -> ()  [unwired: 1 in, 2 out]
      }
      event "BD 1 Frequency 1 (MHz)", "BD 1 Frequency 2 (MHz)", "BD 1 Frequency 3 (MHz)", "BD 2 Frequency 1 (MHz)", "BD 2 Frequency 2 (MHz)", "BD 2 Frequency 3 (MHz)", "Trap Delta (MHz)": Value Change {
        # "anytime one of the frequencies is changed, write it to the RF board UNLESS Set 2 is being oscillated. The oscillation\nscript writes the frequencies to the RF board."
        n477 = event-data() -> ("CtlRef"=w830:refnum<vi>)  [unwired: 6 out]
        n478 = control-ref of="Trap Delta (MHz)"() -> (w829:refnum<vi>)
        n479 = Equal?(x=w829, y=w830) -> (x = y?=w828:bool)
        n480 = case shown="False" "Oscillate Set 2" {
          tunnel: w833 -> [w856 _]
          tunnel: [w855 w859] -> w832
          tunnel: w831 -> [w854 w859]
          tunnel: w828 -> [w841 _]
          frame False {
            w835 = 80
            n481 = local read "BD 1 Frequency 2 (MHz)"() -> (w843:dbl)
            n482 = Divide(x="Trap Delta (MHz)", y=2) -> (x/y=w837:dbl)
            n483 = Subtract(x=w835, y=w837) -> (x-y=w836:dbl)
            n484 = local write "BD 1 Frequency 1 (MHz)"(w836) -> ()
            n485 = Add(x=w835, y=w837) -> (x+y=w842:dbl)
            n486 = Select(t=w842, s=w841, f=w843) -> (s? t:f=w840:dbl)
            n487 = local read "Y RF Frequency Limits (MHz)"() -> (w844:T16)
            n488 = local read "X RF Frequency Limits (MHz)"() -> (w845:T16)
            n489 = local read "BD 1 Frequency 3 (MHz)"() -> (w857:dbl)
            n490 = local write "BD 1 Frequency 2 (MHz)"(w840) -> ()
            n491 = local read "BD 2 Frequency 1 (MHz)"() -> (w848:dbl)
            n492 = local read "BD 2 Frequency 2 (MHz)"() -> (w847:dbl)
            n493 = local read "BD 2 Frequency 3 (MHz)"() -> (w858:dbl)
            n494 = call "set RF board frequency - interlace.vi"("Board 2 Frequency Limits"=w844, "Board 1 Frequency Limits"=w845, "error in"=w854, "FPGA VI Reference In"=w856, "Board 2 Frequency 3 (MHz)"=w858, "Board 1 Frequency 3 (MHz)"=w857, "Board 2 Frequency 2 (MHz)"=w847, "Board 2 Frequency 1 (MHz)"=w848, "Board 1 Frequency 2 (MHz)"=w840, "Board 1 Frequency 1  (MHz)"=w836) -> ("error out"=w855:errorcluster)  [unwired: 1 out]
            n495 = Subtract(x=w848, y=w847) -> (x-y=w852:dbl)
            n496 = Subtract(x=w840, y=w836) -> (x-y=w853:dbl)
            n497 = Square(x=w852) -> (x^2=w850:dbl)
            n498 = Square(x=w853) -> (x^2=w851:dbl)
            n499 = Add(x=w851, y=w850) -> (x+y=w849:dbl)
            n500 = Square Root(x=w849) -> (sqrt(x)=w846:dbl)
            n501 = local write "Trap Delta (MHz)"(w846) -> ()
            n502 = property on="Initial delta (MHz)" class="DigNum (strict)"("Val(Sgnl)"=w846) -> ()  [unwired: 2 in, 2 out]
          }
          frame True {
          }
        }
      }
      event "Round T1 X": Value Change {
        n503 = event-data() -> ()  [unwired: 7 out]
        n504 = local read "BD 1 Frequency 1 (MHz)"() -> (w862:dbl)
        n505 = Round To Nearest(number=w862) -> (nearest integer value=w861:dbl)
        n506 = property on="BD 1 Frequency 1 (MHz)" class="DigNum (strict)"("Val(Sgnl)"=w861) -> ()  [unwired: 2 in, 2 out]
      }
      event "Restart RF": Value Change {
        n507 = event-data() -> ()  [unwired: 7 out]
        n508 = xnode "Read/Write Control"("FPGA VI Reference In"=w900, "error in"=w895, "FPGA Controls  RF Box"=FALSE) -> ("FPGA VI Reference Out"=w899:T19, "error out"=w894:errorcluster)
        n509 = local read "Y RF Amplitude Limits (%)"() -> (w875:T16)
        n510 = local read "X RF Amplitude Limits (%)"() -> (w876:T16)
        n511 = local read "X RF Frequency Limits (MHz)"() -> (w878:T16)
        n512 = local read "Y RF Frequency Limits (MHz)"() -> (w877:T16)
        n513 = xnode "Read/Write Control"("FPGA VI Reference In"=w899, "error in"=w894, "Direct RF Box  Communication"=TRUE) -> ("FPGA VI Reference Out"=w898:T19, "error out"=w893:errorcluster)
        n514 = local read "BD 2 Frequency 3 (MHz)"() -> (w885:dbl)
        n515 = local read "BD 2 Frequency 2 (MHz)"() -> (w886:dbl)
        n516 = local read "BD 1 Frequency 3 (MHz)"() -> (w889:dbl)
        n517 = local read "BD 1 Frequency 1 (MHz)"() -> (w890:dbl)
        n518 = local read "BD 2 Frequency 1 (MHz)"() -> (w887:dbl)
        n519 = local read "BD 1 Frequency 2 (MHz)"() -> (w888:dbl)
        n520 = call "Initialize RF boards - interlace 3.vi"("error in"=w893, "FPGA VI Reference In"=w898) -> ("error out"=w892:errorcluster, "FPGA VI Reference Out"=w897:T19)
        n521 = local read "BD 2 Amplitude 2 (%)"() -> (w880:dbl)
        n522 = local read "BD 2 Amplitude 1 (%)"() -> (w881:dbl)
        n523 = local read "BD 2 Amplitude 3 (%)"() -> (w879:dbl)
        n524 = local read "BD 1 Amplitude 3 (%)"() -> (w884:dbl)
        n525 = local read "BD 1 Amplitude 1 (%)"() -> (w883:dbl)
        n526 = local read "BD 1 Amplitude 2 (%)"() -> (w882:dbl)
        n527 = call "set RF board frequency - interlace.vi"("Board 2 Frequency Limits"=w877, "Board 1 Frequency Limits"=w878, "error in"=w892, "FPGA VI Reference In"=w897, "Board 2 Frequency 3 (MHz)"=w885, "Board 1 Frequency 3 (MHz)"=w889, "Board 2 Frequency 2 (MHz)"=w886, "Board 2 Frequency 1 (MHz)"=w887, "Board 1 Frequency 2 (MHz)"=w888, "Board 1 Frequency 1  (MHz)"=w890) -> ("error out"=w891:errorcluster, "FPGA VI Reference Out"=w896:T19)
        n528 = call "set RF board amplitude - interlace.vi"("Board 2 Amplitude Limits"=w875, "Board 1 Amplitude Limits"=w876, "error in"=w891, "FPGA VI Reference In"=w896, "Board 2 Amplitude 3 (%)"=w879, "Board 1 Amplitude 3 (%)"=w884, "Board 2 Amplitude 2 (%)"=w880, "Board 2 Amplitude 1 (%)"=w881, "Board 1 Amplitude 2 (%)"=w882, "Board 1 Amplitude 1 (%)"=w883) -> ("error out"=w868:errorcluster, "FPGA VI Reference Out"=w872:T19)
        n529 = xnode "Read/Write Control"("FPGA VI Reference In"=w872, "error in"=w868, "Direct RF Box  Communication"=FALSE) -> ("FPGA VI Reference Out"=w871:T19, "error out"=w870:errorcluster)
        n530 = flat-sequence {
          tunnel: w870 -> [w901]
          tunnel: [w901] -> w869
          frame #0 {
            n531 = Wait (ms)(milliseconds to wait=u32 50) -> ()  [unwired: 1 out]
          }
        }
        n532 = xnode "Read/Write Control"("FPGA VI Reference In"=w871, "error in"=w869, "FPGA Controls  RF Box"=TRUE) -> ("error out"=w864:errorcluster)  [unwired: 1 out]
        n533 = property on="Restart RF" class="Bool (strict)"(error in=w864, "Value"=FALSE ("Restart RF")) -> (error out=w863:errorcluster)  [unwired: 1 in, 1 out]
      }
      event "Round T2 X": Value Change {
        n534 = event-data() -> ()  [unwired: 7 out]
        n535 = local read "BD 1 Frequency 2 (MHz)"() -> (w904:dbl)
        n536 = Round To Nearest(number=w904) -> (nearest integer value=w903:dbl)
        n537 = property on="BD 1 Frequency 2 (MHz)" class="DigNum (strict)"("Val(Sgnl)"=w903) -> ()  [unwired: 2 in, 2 out]
      }
      event "Stop All": Value Change {
        n538 = event-data() -> ()  [unwired: 7 out]
        n539 = call "hamilton_controller.vi"("action"=T20."DISCONNECT") -> ()  [unwired: 10 in, 1 out]
        n540 = local read "Stop All"() -> (w907:bool)
      }
      event "Delayed Interlace Start": Value Change {
        n541 = event-data() -> ()  [unwired: 7 out]
        n542 = flat-sequence {
          frame #0 {
            n543 = Multiply(x="Delay to Interlace (s)", y=1000.0) -> (x*y=w910:dbl)
            n544 = Wait (ms)(milliseconds to wait=w910) -> ()  [unwired: 1 out]
          }
          frame #1 {
            n545 = property on="Green laser mode" class="RadioBtnsControl (strict)"("Val(Sgnl)"=enum32{"Laser ON", "Laser OFF", "Interlace"}."Interlace" ("Value (Signaling)")) -> ()  [unwired: 2 in, 2 out]
          }
        }
      }
      event "BD 1 Amplitude 1 (%)", "BD 1 Amplitude 2 (%)", "BD 1 Amplitude 3 (%)", "BD 2 Amplitude 1 (%)", "BD 2 Amplitude 2 (%)", "BD 2 Amplitude 3 (%)", "Trap 1 ON", "Trap 2 ON", "Trap 3 ON", "Feedback On/Off", "All FB On/Off": Value Change {
        w934 = i16 1 ("f")
        n546 = event-data() -> ()  [unwired: 7 out]
        n547 = local write "Trap 1 (ON/OFF)"("Trap 1 ON") -> ()
        n548 = local write "Trap 2 (ON/OFF)"("Trap 2 ON") -> ()
        n549 = Boolean To (0,1)(Boolean="Trap 3 ON") -> (0, 1=w935:i16)
        n550 = Boolean To (0,1)(Boolean="Trap 1 ON") -> (0, 1=w936:i16)
        n551 = Boolean To (0,1)(Boolean="Trap 2 ON") -> (0, 1=w937:i16)
        n552 = Select(t=w937, s="Trap ON/OFF X or Y Amp?", f=w934) -> (s? t:f=w932:i16)
        n553 = Select(t=w936, s="Trap ON/OFF X or Y Amp?", f=w934) -> (s? t:f=w933:i16)
        n554 = Select(t=w935, s="Trap ON/OFF X or Y Amp?", f=w934) -> (s? t:f=w931:i16)
        n555 = Select(t=w934, s="Trap ON/OFF X or Y Amp?", f=w937) -> (s? t:f=w929:i16)
        n556 = Select(t=w934, s="Trap ON/OFF X or Y Amp?", f=w936) -> (s? t:f=w930:i16)
        n557 = Select(t=w934, s="Trap ON/OFF X or Y Amp?", f=w935) -> (s? t:f=w928:i16)
        n558 = And(x="All FB On/Off", y="Feedback On/Off") -> (x .and. y?=w926:cluster{"Set 1":bool, "Set 2":bool})
        n559 = local read "BD 1 Amplitude 1 (%)"() -> (w946:dbl)
        n560 = local read "BD 1 Amplitude 2 (%)"() -> (w945:dbl)
        n561 = local read "BD 1 Amplitude 3 (%)"() -> (w944:dbl)
        n562 = Unbundle By Name(w926) -> ("Set 1"=w921:bool, "Set 2"=w918:bool)
        n563 = local read "Y RF Amplitude Limits (%)"() -> (w914:T16)
        n564 = local read "X RF Amplitude Limits (%)"() -> (w915:T16)
        n565 = local read "BD 2 Amplitude 1 (%)"() -> (w947:dbl)
        n566 = local read "BD 2 Amplitude 2 (%)"() -> (w948:dbl)
        n567 = local read "BD 2 Amplitude 3 (%)"() -> (w949:dbl)
        n568 = And(x="Trap 2 ON", y=w918) -> (x .and. y?=w916:bool)
        n569 = And(x="Trap 1 ON", y=w921) -> (x .and. y?=w919:bool)
        n570 = Multiply(x=w933, y=w946) -> (x*y=w941:dbl)
        n571 = Multiply(x=w945, y=w932) -> (x*y=w939:dbl)
        n572 = Multiply(x=w944, y=w931) -> (x*y=w940:dbl)
        n573 = Multiply(x=w947, y=w930) -> (x*y=w950:dbl)
        n574 = Multiply(x=w948, y=w929) -> (x*y=w951:dbl)
        n575 = Multiply(x=w949, y=w928) -> (x*y=w952:dbl)
        n576 = call "set RF board amplitude - interlace.vi"("Board 2 Amplitude Limits"=w914, "Board 1 Amplitude Limits"=w915, "error in"=w942, "FPGA VI Reference In"=w943, "Board 2 Amplitude 3 (%)"=w952, "Board 1 Amplitude 3 (%)"=w940, "Board 2 Amplitude 2 (%)"=w951, "Board 2 Amplitude 1 (%)"=w950, "Board 1 Amplitude 2 (%)"=w939, "Board 1 Amplitude 1 (%)"=w941) -> ("error out"=w923:errorcluster, "FPGA VI Reference Out"=w924:T19)
        n577 = xnode "Read/Write Control"("FPGA VI Reference In"=w924, "error in"=w923, "FB On/Off Set 1"=w919, "FB On/Off Set 2"=w916) -> ("error out"=w922:errorcluster)  [unwired: 1 out]
      }
      event "Load parameters": Value Change {
        n578 = event-data() -> ()  [unwired: 7 out]
        n579 = property on="Saved AOD Raster Scan Parameter Sets" class="Arr (strict)"() -> ("Index Values"=w963:u32[])  [unwired: 2 in, 2 out]
        n580 = Index Array(array=w963, index=0) -> (element=w960:u32)
        n581 = local write "Load parameters"(FALSE ("Load parameters")) -> ()
        n582 = Index Array(array="Saved AOD Raster Scan Parameter Sets", index=w960) -> (element=w959:T30)
        n583 = Unbundle By Name(w959) -> ("Scan Range AOD (nm) 2"=w958:dbl, "Step Size AOD (nm) 2"=w957:dbl, "Scan Speed AOD (nm/s) 2"=w956:dbl, "Number of scans (AOD) 2"=w955:u16)
        n584 = flat-sequence {
          tunnel: w958 -> [w966]
          tunnel: w957 -> [w965]
          tunnel: w956 -> [w964]
          tunnel: w955 -> [w967]
          frame #0 {
            n585 = local write "Scan Speed (nm/s)"(w964) -> ()
            n586 = local write "Scan Range (nm)"(w966) -> ()
            n587 = local write "Step Size (nm)"(w965) -> ()
          }
          frame #1 {
            n588 = property on="Number of F/B Scans (AOD)" class="DigNum (strict)"("Val(Sgnl)"=w967) -> ()  [unwired: 2 in, 2 out]
          }
        }
      }
      event "Trap 1 (ON/OFF)", "Trap 2 (ON/OFF)": Value Change {
        n589 = event-data() -> ()  [unwired: 7 out]
        n590 = property on="Trap 2 ON" class="Bool (strict)"("Val(Sgnl)"="Trap 2 (ON/OFF)") -> ()  [unwired: 2 in, 2 out]
        n591 = property on="Trap 1 ON" class="Bool (strict)"("Val(Sgnl)"="Trap 1 (ON/OFF)") -> ()  [unwired: 2 in, 2 out]
      }
      event "DIO count 1 (ticks)", "DIO count 2 (ticks)", "DIO count 3 (ticks)", "Interlace", "Number Interlace Sets", "Not-Interlacing Set": Value Change {
        n592 = event-data() -> ()  [unwired: 7 out]
        n593 = local read "DIO count 3 (ticks)"() -> (w980:u32)
        n594 = local read "DIO count 1 (ticks)"() -> (w982:u32)
        n595 = local read "DIO count 2 (ticks)"() -> (w981:u32)
        n596 = To Unsigned Byte Integer(number="Not-Interlacing Set") -> (unsigned 8bit integer=w971:u8)
        n597 = Add(x=w971, y=u8 1) -> (x+y=w975:u8)
        n598 = xnode "Read/Write Control"("FPGA VI Reference In"=w986, "error in"=w984, "DIO count 1 (ticks)"=w982, "DIO count 2 (ticks)"=w981, "DIO count 3 (ticks)"=w980, "Interlace ON/OFF"="Interlace", "Number Interlace Cycles"="Number Interlace Sets", "Interlace Off Parameters"=w975) -> ("error out"=w985:errorcluster)  [unwired: 1 out]
        n599 = Build Array(w982, w981, w980) -> (w973:u32[])
        n600 = Split 1D Array(array=w973, index="Number Interlace Sets") -> (first subarray=w983:u32[])  [unwired: 1 out]
        n601 = Index Array(array=w973, index=w971) -> (element=w972:u32)
        n602 = Add Array Elements(numeric array=w983) -> (sum=w977:u32)
        n603 = Select(t=w977, s="Interlace", f=w972) -> (s? t:f=→"Total Counts (ticks)":u32)
      }
      event "Reset Feedback": Value Change {
        n604 = event-data() -> ()  [unwired: 7 out]
        n605 = Unbundle By Name("Reset Feedback") -> ("Set 1"=w990:bool, "Set 2"=w989:bool)
        n606 = xnode "Read/Write Control"("FPGA VI Reference In"=w992, "error in"=w987, "FB Reset Set 1"=w990, "FB Reset Set 2"=w989) -> ("error out"=w988:errorcluster)  [unwired: 1 out]
      }
      event "PID Gains": Value Change {
        n607 = event-data() -> ()  [unwired: 7 out]
        n608 = Unbundle By Name("PID Gains") -> ("Set 1"=w996:T14, "Set 2"=w995:T14)
        n609 = xnode "Read/Write Control"("FPGA VI Reference In"=w997, "error in"=w993, "FB Gains Set 1"=w996, "FB Gains Set 2"=w995) -> ("error out"=w994:errorcluster)  [unwired: 1 out]
      }
      event "AI2 to Setpoint", "Trap Intensity\nSetpoints (V)": Value Change {
        n610 = event-data() -> ()  [unwired: 7 out]
        n611 = xnode "Read/Write Control"("FPGA VI Reference In"=w1003, "error in"=w999) -> ("FPGA VI Reference Out"=w1002:T19, "error out"=w1001:errorcluster, "AI2 Y Sum Set 1"=w1010:i16, "AI2 Y Sum Set 2"=w1009:i16)
        n612 = Cluster To Array(cluster="AI2 to Setpoint") -> (array=w1013:bool[])
        n613 = local read "AI2 (V)"() -> (w1011:cluster{"Set 1":dbl, "Set 2":dbl})
        n614 = Or Array Elements(Boolean array=w1013) -> (logical OR=w1014:bool)
        n615 = Bundle By Name(cluster=w1011, "Set 1"=w1010, "Set 2"=w1009) -> (w1008:cluster{"Set 1":dbl, "Set 2":dbl})
        n616 = Divide(x=w1008, y=3276.7) -> (x/y=w1007:cluster{"Set 1":dbl, "Set 2":dbl})
        "AI2 (V)" <- w1007
        n617 = case shown="True" w1014 {
          tunnel: [w1017 w1034] -> w1006
          tunnel: "AI2 to Setpoint" -> [_ w1030]
          tunnel: "Trap Intensity\nSetpoints (V)" -> [w1018 w1033]
          tunnel: w1007 -> [_ w1027]
          frame False {
            n618 = Multiply(x=3276.7, y=w1018) -> (x*y=w1019:cluster{"Set 1":dbl, "Set 2":dbl})
            n619 = To Word Integer(number=w1019) -> (16bit integer=w1017:cluster{"Set 1":i16, "Set 2":i16})
          }
          frame True {
            n620 = Unbundle By Name(w1027) -> ("Set 1"=w1026:dbl, "Set 2"=w1025:dbl)
            n621 = Unbundle By Name(w1033) -> ("Set 1"=w1032:dbl, "Set 2"=w1031:dbl)
            n622 = Unbundle By Name(w1030) -> ("Set 1"=w1029:bool, "Set 2"=w1028:bool)
            n623 = Select(t=w1026, s=w1029, f=w1032) -> (s? t:f=w1024:dbl)
            n624 = Select(t=w1025, s=w1028, f=w1031) -> (s? t:f=w1023:dbl)
            n625 = Bundle By Name(cluster=w1033, "Set 1"=w1024, "Set 2"=w1023) -> (w1021:cluster{"Set 1":dbl, "Set 2":dbl})
            n626 = local write "Trap Intensity\nSetpoints (V)"(w1021) -> ()
            n627 = Multiply(x=3276.7, y=w1021) -> (x*y=w1022:cluster{"Set 1":dbl, "Set 2":dbl})
            n628 = To Word Integer(number=w1022) -> (16bit integer=w1034:cluster{"Set 1":i16, "Set 2":i16})
          }
        }
        n629 = Unbundle By Name(w1006) -> ("Set 1"=w1005:i16, "Set 2"=w1004:i16)
        n630 = xnode "Read/Write Control"("FPGA VI Reference In"=w1002, "error in"=w1001, "FB Setpoint Set 1"=w1005, "FB Setpoint Set 2"=w1004) -> ("error out"=w1000:errorcluster)  [unwired: 1 out]
      }
      event "Invert GI": Value Change {
        n631 = event-data() -> ()  [unwired: 7 out]
        n632 = xnode "Read/Write Control"("FPGA VI Reference In"=w1039, "error in"=w1037, "Invert GI"="Invert GI", "Invert GI 2"="Invert GI") -> ("error out"=w1038:errorcluster)  [unwired: 1 out]
      }
      event "Green FB Setpoint (mV)", "Green FB Gains", "Green FB On/Off", "Current When FB OFF (%)", "Green int current ON count adj": Value Change {
        n633 = event-data() -> ()  [unwired: 7 out]
        n634 = local read "Green FB Setpoint (mV)"() -> (w1046:dbl)
        n635 = local read "Current When FB OFF (%)"() -> (w1049:dbl)
        n636 = Multiply(x=w1046, y=3.2767) -> (x*y=w1045:dbl)
        n637 = Multiply(x=w1049, y=655.35) -> (x*y=w1050:dbl)
        n638 = To Unsigned Word Integer(number=w1050) -> (unsigned 16bit integer=w1048:u16)
        n639 = local read "Green int current ON count adj"() -> (w1053:u32)
        n640 = local read "Green FB Gains"() -> (w1052:T14)
        n641 = local read "Green Laser ON/Interlacing"() -> (w1043:bool)
        n642 = local read "Green laser mode"() -> (w1042:enum32{"Laser ON", "Laser OFF", "Interlace"})
        n643 = local read "Green FB On/Off"() -> (w1054:bool)
        n644 = Equal?(x=w1042, y=enum32{"Laser ON", "Laser OFF", "Interlace"}."Interlace") -> (x = y?=w1040:bool)
        n645 = Compound Arithmetic op=AND(w1040, w1054, w1043) -> (w1044:bool)
        n646 = xnode "Read/Write Control"("FPGA VI Reference In"=w1057, "error in"=w1056, "Green FB Setpoint"=w1045, "Green FB On/Off"=w1044, "Current Out"=w1048, "Green int current ON count adj"=w1053, "Green FB Gains"=w1052) -> ("error out"=w1055:errorcluster)  [unwired: 1 out]
      }
      event "Green laser mode", "Green Laser ON/Interlacing": Value Change {
        n647 = event-data() -> ()  [unwired: 7 out]
        n648 = case shown="True" "Green Laser ON/Interlacing" {
          tunnel: "Green laser mode" -> [_ w1071]
          tunnel: [enum32{"Laser ON", "Laser OFF", "Interlace"}."Laser OFF" ("Green laser mode") w1071] -> w1059
          tunnel: [FALSE w1067] -> w1058
          frame False {
          }
          frame True {
            n649 = local read "Green FB On/Off"() -> (w1068:bool)
            n650 = Equal?(x=w1071, y=enum32{"Laser ON", "Laser OFF", "Interlace"}."Interlace") -> (x = y?=w1069:bool)
            n651 = And(x=w1069, y=w1068) -> (x .and. y?=w1067:bool)
          }
        }
        n652 = xnode "Read/Write Control"("FPGA VI Reference In"=w1064, "error in"=w1062, "Operating Mode"=w1059, "Operating Mode 2"=w1059, "Green FB On/Off"=w1058) -> ("error out"=w1063:errorcluster)  [unwired: 1 out]
      }
      event "- phase (APD 1 Gate)", "+ phase (APD 1 Gate)": Value Change {
        n653 = event-data() -> ()  [unwired: 7 out]
        n654 = local read "Phase Adj. (APD 1 Gate)"() -> (w1072:i16)
        n655 = Negate(x=w1072) -> (-x=w1080:i16)
        n656 = Select(t=w1080, s="- phase (APD 1 Gate)", f=w1072) -> (s? t:f=w1079:i16)
        n657 = Or(x="- phase (APD 1 Gate)", y="+ phase (APD 1 Gate)") -> (x .or. y?=w1075:bool)
        n658 = xnode "Read/Write Control"("FPGA VI Reference In"=w1082, "error in"=w1081, "Phase count adjustment (APD 1 Gate)"=w1079) -> ("FPGA VI Reference Out"=w1077:T19, "error out"=w1078:errorcluster)
        n659 = xnode "Read/Write Control"("FPGA VI Reference In"=w1077, "error in"=w1078, "+ phase (APD 1 Gate)"=w1075) -> ("error out"=w1076:errorcluster)  [unwired: 1 out]
      }
      event "+ phase (APD 2 Gate)", "- phase (APD 2 Gate)": Value Change {
        n660 = event-data() -> ()  [unwired: 7 out]
        n661 = local read "Phase Adj. (APD 2 Gate)"() -> (w1083:i16)
        n662 = Negate(x=w1083) -> (-x=w1091:i16)
        n663 = Select(t=w1091, s="- phase (APD 2 Gate)", f=w1083) -> (s? t:f=w1090:i16)
        n664 = Or(x="- phase (APD 2 Gate)", y="+ phase (APD 2 Gate)") -> (x .or. y?=w1086:bool)
        n665 = xnode "Read/Write Control"("FPGA VI Reference In"=w1093, "error in"=w1092, "Phase count adjustment (APD 2 Gate)"=w1090) -> ("FPGA VI Reference Out"=w1088:T19, "error out"=w1089:errorcluster)
        n666 = xnode "Read/Write Control"("FPGA VI Reference In"=w1088, "error in"=w1089, "+ phase (APD 2 Gate)"=w1086) -> ("error out"=w1087:errorcluster)  [unwired: 1 out]
      }
      event "Phase Adj. (APD Acq)", "+ phase (APD Acq)", "- phase (APD Acq)": Value Change {
        n667 = event-data() -> ()  [unwired: 7 out]
        n668 = local read "Phase Adj. (APD Acq)"() -> (w1096:i16)
        n669 = Negate(x=w1096) -> (-x=w1102:i16)
        n670 = Select(t=w1102, s="+ phase (APD Acq)", f=w1096) -> (s? t:f=w1101:i16)
        n671 = Or(x="+ phase (APD Acq)", y="- phase (APD Acq)") -> (x .or. y?=w1097:bool)
        n672 = xnode "Read/Write Control"("FPGA VI Reference In"=w1104, "error in"=w1103, "Phase Count Adjustment (APD Acq)"=w1101) -> ("FPGA VI Reference Out"=w1099:T19, "error out"=w1100:errorcluster)
        n673 = xnode "Read/Write Control"("FPGA VI Reference In"=w1099, "error in"=w1100, "+ phase (APD Acq)"=w1097) -> ("error out"=w1098:errorcluster)  [unwired: 1 out]
      }
      event "Phase adj. (GI)", "+ phase (GI)", "- phase (GI)": Value Change {
        n674 = event-data() -> ()  [unwired: 7 out]
        n675 = Negate(x="Phase adj. (GI)") -> (-x=w1113:i16)
        n676 = Select(t=w1113, s="+ phase (GI)", f="Phase adj. (GI)") -> (s? t:f=w1112:i16)
        n677 = Or(x="+ phase (GI)", y="- phase (GI)") -> (x .or. y?=w1108:bool)
        n678 = xnode "Read/Write Control"("FPGA VI Reference In"=w1115, "error in"=w1114, "Phase count adjustment (GI)"=w1112) -> ("FPGA VI Reference Out"=w1110:T19, "error out"=w1111:errorcluster)
        n679 = xnode "Read/Write Control"("FPGA VI Reference In"=w1110, "error in"=w1111, "+ phase (GI)"=w1108) -> ("error out"=w1109:errorcluster)  [unwired: 1 out]
      }
      event "Phase adj. (GI) 2", "+ phase (GI) 2", "- phase (GI) 2": Value Change {
        n680 = event-data() -> ()  [unwired: 7 out]
        n681 = Negate(x="Phase adj. (GI) 2") -> (-x=w1124:i16)
        n682 = Select(t=w1124, s="+ phase (GI) 2", f="Phase adj. (GI) 2") -> (s? t:f=w1123:i16)
        n683 = Or(x="+ phase (GI) 2", y="- phase (GI) 2") -> (x .or. y?=w1119:bool)
        n684 = xnode "Read/Write Control"("FPGA VI Reference In"=w1126, "error in"=w1125, "Phase count adjustment (GI) 2"=w1123) -> ("FPGA VI Reference Out"=w1121:T19, "error out"=w1122:errorcluster)
        n685 = xnode "Read/Write Control"("FPGA VI Reference In"=w1121, "error in"=w1122, "+ phase (GI) 2"=w1119) -> ("error out"=w1120:errorcluster)  [unwired: 1 out]
      }
      event "Phase adj. (Green FB)", "- phase (Green FB)", "+ phase (Green FB)": Value Change {
        n686 = event-data() -> ()  [unwired: 7 out]
        n687 = Negate(x="Phase adj. (Green FB)") -> (-x=w1135:i16)
        n688 = Select(t=w1135, s="+ phase (Green FB)", f="Phase adj. (Green FB)") -> (s? t:f=w1134:i16)
        n689 = Or(x="+ phase (Green FB)", y="- phase (Green FB)") -> (x .or. y?=w1130:bool)
        n690 = xnode "Read/Write Control"("FPGA VI Reference In"=w1137, "error in"=w1136, "Phase count adjustment (Green FB)"=w1134) -> ("FPGA VI Reference Out"=w1132:T19, "error out"=w1133:errorcluster)
        n691 = xnode "Read/Write Control"("FPGA VI Reference In"=w1132, "error in"=w1133, "+ phase (Green FB)"=w1130) -> ("error out"=w1131:errorcluster)  [unwired: 1 out]
      }
      event "Invert APD Gate", "APD Gate ON Count", "APD Gate OFF Count", "APD Gate", "APD Integration Time (s)", "APD 1 AO Mult.", "APD 2 AO Mult.": Value Change {
        n692 = event-data() -> ()  [unwired: 7 out]
        n693 = local read "APD Integration Time (s)"() -> (w1138:dbl)
        n694 = local read "APD Gate ON Count"() -> (w1151:u32)
        n695 = local read "APD Gate OFF Count"() -> (w1150:u32)
        n696 = local read "Invert APD Gate"() -> (w1152:bool)
        n697 = local read "APD Gate"() -> (w1149:enum32{"ON", "OFF", "Interlace"})
        n698 = Multiply(x=w1138, y=40000000.0) -> (x*y=w1147:dbl)
        n699 = Reciprocal(x=w1138) -> (1/x=→"APD Acq Rate (Hz)":dbl)
        n700 = To Unsigned Long Integer(number=w1147) -> (unsigned 32bit integer=w1146:u32)
        n701 = local read "DMA Update Period (s)"() -> (w1139:dbl)
        n702 = Divide(x=w1139, y=w1138) -> (x/y=w1142:dbl)
        n703 = local read "APD 1 AO Mult."() -> (w1144:i16)
        n704 = local read "APD 2 AO Mult."() -> (w1143:i16)
        n705 = Multiply(x=2.0, y=w1142) -> (x*y=w1141:dbl)
        n706 = local write "APD Samples/FIFO Acq."(w1142) -> ()
        n707 = local write "APD Elements/DMA read"(w1141) -> ()
        n708 = xnode "Read/Write Control"("FPGA VI Reference In"=w1155, "error in"=w1154, "Invert APD Gate"=w1152, "APD Gate ON Count"=w1151, "APD Gate OFF Count"=w1150, "APD Acq Rate Count"=w1146, "APD Gate Operating Mode"=w1149, "APD 1 AO scale factor"=w1144, "APD 2 AO scale factor"=w1143) -> ("error out"=w1153:errorcluster)  [unwired: 1 out]
      }
      event "GI Frequency, ON count", "Green FB Count", "GI Frequency, OFF count": Value Change {
        n709 = event-data() -> ()  [unwired: 7 out]
        n710 = xnode "Read/Write Control"("FPGA VI Reference In"=w1161, "error in"=w1159, "Green interlace ON count"="GI Frequency, ON count", "Green interlace OFF count"="GI Frequency, OFF count", "Green interlace ON count 2"="GI Frequency, ON count", "Green interlace OFF count 2"="GI Frequency, OFF count", "Green FB Count"="Green FB Count") -> ("error out"=w1160:errorcluster)  [unwired: 1 out]
      }
      event "Number of F/B Scans (AOD)", "Scan Speed (nm/s)", "Scan BD", "Initial delta (MHz)", "Step Size (nm)", "Scan Range (nm)": Value Change {
        w1223 = 123.0  # AOM cal (nm/MHz)
        n711 = event-data() -> ()  [unwired: 7 out]
        n712 = local read "BD 1 Frequency 1 (MHz)"() -> (w1206:dbl)
        n713 = local read "AOM X Cal (nm/MHz)"() -> (w1198:dbl)
        n714 = local read "X RF Frequency Limits (MHz)"() -> (w1210:T16)
        n715 = local read "Y RF Frequency Limits (MHz)"() -> (w1207:T16)
        n716 = local read "BD 2 Frequency 1 (MHz)"() -> (w1212:dbl)
        n717 = Negate(x="Scan Range (nm)") -> (-x=w1176:dbl)
        n718 = Divide(x=w1176, y=w1198) -> (x/y=w1180:dbl)
        n719 = Select(t=w1210, s="Scan BD", f=w1207) -> (s? t:f=w1209:T16)
        n720 = Select(t=w1206, s="Scan BD", f=w1212) -> (s? t:f=w1211:dbl)
        n721 = Unbundle By Name(w1209) -> ("Maximum"=w1218:dbl, "Minimum"=w1217:dbl)
        n722 = Add(x=w1180, y=w1211) -> (x+y=w1215:dbl)
        n723 = Divide(x=w1176, y="Step Size (nm)") -> (x/y=w1195:dbl)
        n724 = Divide(x="Step Size (nm)", y=w1198) -> (x/y=w1204:dbl)
        n725 = Absolute Value(x=w1195) -> (abs(x)=w1179:dbl)
        n726 = Sign(1:w1176) -> (0:w1177:dbl)
        n727 = In Range and Coerce(upper limit=w1218, x=w1215, lower limit=w1217) -> (coerced(x)=w1214:dbl, In Range?=w1216:bool)
        n728 = To Unsigned Quad Integer(1:w1179) -> (0:w1194:u64)
        "Scan steps (AOD)" <- w1194
        n729 = call "IR AOM freq to word.vi"("Frequency In (MHz)"=w1204) -> ("Frequency Word Out (double)"=w1201:dbl)
        n730 = Multiply(x=w1177, y=w1201) -> (x*y=w1178:dbl)
        n731 = Subtract(x=w1215, y=w1214) -> (x-y=w1213:dbl)
        n732 = To Quad Integer(1:w1178) -> (0:w1200:i64)
        "Incr. int (AOD)" <- w1200
        n733 = Subtract(x=w1180, y=w1213) -> (x-y=w1199:dbl)
        "Scan Range (MHz)" <- w1199
        n734 = Select(t=w1180, s=w1216, f=w1199) -> (s? t:f=w1219:dbl)
        n735 = Multiply(x=w1199, y=w1198) -> (x*y=w1197:dbl)
        n736 = Decrement(x=w1194) -> (x-1=w1247:u64)
        n737 = Negate(x=w1197) -> (-x=w1193:dbl)
        n738 = local write "Scan Range (nm)"(w1193) -> ()
        n739 = Divide(x=w1219, y=w1247) -> (x/y=w1203:dbl)
        "Scan Increment (MHz)" <- w1203
        n740 = call "IR AOM freq to word.vi"("Frequency In (MHz)"=w1203) -> ("Frequency Word Out (double)"=w1202:dbl)
        n741 = Divide(x="Step Size (nm)", y="Scan Speed (nm/s)") -> (x/y=w1190:dbl)
        n742 = To Quad Integer(1:w1202) -> ()  [unwired: 1 out]
        n743 = local read "Number Interlace Sets"() -> (w1174:u8)
        n744 = local read "AI Count (ticks)"() -> (w1175:u32)
        n745 = local read "Total Counts (ticks)"() -> (w1173:u32)
        n746 = local read "# Samples/trap"() -> (w1205:u32)
        n747 = Multiply(x=w1175, y=w1174) -> (x*y=w1172:u32)
        n748 = Divide(x=w1173, y=w1172) -> (x/y=w1171:dbl)
        n749 = Select(t=w1206, s="Scan BD", f=w1212) -> (s? t:f=w1244:dbl)
        "Initial freq. (MHz)" <- w1244
        n750 = Add(x=w1219, y=w1244) -> (x+y=→"Final freq. (MHz)":dbl)
        n751 = Divide(x=w1173, y=40000000.0) -> (x/y=w1189:dbl)
        n752 = Divide(x=w1190, y=w1189) -> (x/y=w1188:dbl)
        n753 = To Unsigned Quad Integer(1:w1188) -> (0:w1163:u64)
        n754 = Quotient & Remainder(x=w1163, y=u64 2) -> (x-y*floor(x/y)=w1167:u64)  [unwired: 1 out]
        n755 = Equal?(x=w1167, y=u64 0) -> (x = y?=w1165:bool)
        n756 = Decrement(x=w1163) -> (x-1=w1164:u64)
        n757 = Select(t=w1163, s=w1165, f=w1164) -> (s? t:f=w1162:u64)
        "Cycles/step (AOD)" <- w1162
        n758 = xnode "Read/Write Control"("FPGA VI Reference In"=w1255, "error in"=w1254, "Scan steps"=w1194, "Number of scans"="Number of F/B Scans (AOD)", "Cycles per step"=w1162, "Scan freq.  increment"=w1200, "Scan BD"="Scan BD") -> ("error out"=w1253:errorcluster)  [unwired: 1 out]
        n759 = Multiply(x=w1194, y=w1162) -> (x*y=w1248:u64)
        n760 = Multiply(x=w1248, y=u64 2) -> (x*y=w1170:u64)
        n761 = Multiply(x=w1171, y=w1170) -> (x*y=w1169:dbl)
        "Data points/scan (f/b)" <- w1169
        n762 = Multiply(x=w1169, y="Number of F/B Scans (AOD)") -> (x*y=w1251:dbl)
        "Data points/scans" <- w1251
        n763 = Divide(x=w1251, y=w1205) -> (x/y=→"N sets should be saved":dbl)
        n764 = Multiply(x=w1248, y=w1189) -> (x*y=w1187:dbl)
        "Time/Scan (s) (AOD)" <- w1187
        n765 = Select(t=w1219, s="Scan BD", f=0.0) -> (s? t:f=w1245:dbl)
        n766 = Select(t=0.0, s="Scan BD", f=w1219) -> (s? t:f=w1241:dbl)
        n767 = local read "BD 2 Frequency 2 (MHz)"() -> (w1237:dbl)
        n768 = local read "BD 1 Frequency 2 (MHz)"() -> (w1240:dbl)
        n769 = Add(x=w1241, y=w1212) -> (x+y=w1238:dbl)
        n770 = Add(x=w1206, y=w1245) -> (x+y=w1239:dbl)
        n771 = Multiply(x=w1187, y=2.0) -> (x*y=w1186:dbl)
        n772 = Multiply(x=w1186, y="Number of F/B Scans (AOD)") -> (x*y=w1183:dbl)
        n773 = Divide(x=w1183, y=60.0) -> (x/y=→"Time to Finish All (min)":dbl)
        n774 = Add(x="Trap 2 Bead Size (nm)", y="Trap 1 Bead Size (nm)") -> (x+y=w1227:dbl)
        n775 = local read "Initial delta (MHz)"() -> (w1224:dbl)
        n776 = Divide(x=w1227, y=2.0) -> (x/y=w1221:dbl)
        n777 = Subtract(x=w1238, y=w1237) -> (x-y=w1235:dbl)
        n778 = Subtract(x=w1239, y=w1240) -> (x-y=w1236:dbl)
        n779 = Square(x=w1235) -> (x^2=w1234:dbl)
        n780 = Square(x=w1236) -> (x^2=w1233:dbl)
        n781 = Add(x=w1233, y=w1234) -> (x+y=w1232:dbl)
        n782 = Square Root(x=w1232) -> (sqrt(x)=w1231:dbl)
        "Final delta (MHz)" <- w1231
        n783 = Multiply(x=w1223, y=w1231) -> (x*y=w1230:dbl)
        n784 = Multiply(x=w1224, y=w1223) -> (x*y=w1222:dbl)
        n785 = Subtract(x=w1222, y=w1221) -> (x-y=→"Initial sep (nm)":dbl)
        n786 = Subtract(x=w1230, y=w1221) -> (x-y=→"Final sep (nm)":dbl)
      }
      event "Raster Scanning...": Value Change {
        n787 = event-data() -> ("NewVal"=w1256:bool)  [unwired: 6 out]
        n788 = case shown="True" w1256 {
          frame False {
          }
          frame True {
            n789 = property on="BD 1 Frequency 1 (MHz)" class="DigNum (strict)"("Val(Sgnl)"=65.0 ("Value (Signaling)")) -> ()  [unwired: 2 in, 2 out]
          }
        }
      }
      event "Freq or Amp switch first", "Swap F1 and F2", "Freq switch delay", "Amp switch delay": Value Change {
        n790 = event-data() -> ()  [unwired: 7 out]
        n791 = local read "Freq or Amp switch first"() -> (w1258:bool)
        n792 = local read "Amp switch delay"() -> (w1259:u16)
        n793 = local read "Freq switch delay"() -> (w1261:u16)
        n794 = local read "Swap F1 and F2"() -> (w1260:bool)
        n795 = xnode "Read/Write Control"("FPGA VI Reference In"=w1264, "error in"=w1263, "Freq switch delay"=w1261, "Swap F1 and F2"=w1260, "Amp switch delay"=w1259, "Freq or Amp switch first"=w1258) -> ("error out"=w1262:errorcluster)  [unwired: 1 out]
      }
      event "Scan steps (MCL)", "Number of scans (MCL)", "Scan Range (V)\n(of steps)", "2D or 1D Scan", "N APD Samp/step", "Fast Scan Dir", "Continuous MCL Scanning", "Scan lines (y)": Value Change {
        w1266 = 32767.0 ("y")
        n796 = event-data() -> ()  [unwired: 7 out]
        n797 = Select(t="Scan lines (y)", s="2D or 1D Scan", f="Number of scans (MCL)") -> (s? t:f=w1271:u64)
        n798 = Decrement(x="Scan steps (MCL)") -> (x-1=w1287:u64)
        n799 = Divide(x="Scan Range (V)\n(of steps)", y=w1287) -> (x/y=w1286:dbl)
        "Desired Scan Incr (V)" <- w1286
        n800 = local read "APD Integration Time (s)"() -> (w1279:dbl)
        n801 = Multiply(x=w1286, y=w1266) -> (x*y=w1295:dbl)
        n802 = Divide(x=w1295, y=10.0) -> (x/y=w1285:dbl)
        "Desired incr (int)" <- w1285
        n803 = local read "Update Count (MCL)"() -> (w1291:u32)
        n804 = Round Toward -Infinity(1:w1285) -> (0:w1294:dbl)
        n805 = To Word Integer(number=w1294) -> (16bit integer=w1269:i16)
        "Actual Incr. int (MCL)" <- w1269
        n806 = Multiply(x=w1279, y=40000000.0) -> (x*y=w1292:dbl)
        n807 = Divide(x=w1292, y=w1291) -> (x/y=w1290:dbl)
        n808 = Multiply(x=i16 10, y=w1269) -> (x*y=w1267:i16)
        n809 = Multiply(x="N APD Samp/step", y=w1290) -> (x*y=w1289:dbl)
        "Cycles/step (MCL)" <- w1289
        n810 = Divide(x=w1267, y=w1266) -> (x/y=→"Actual MCL Inc (V)":dbl)
        n811 = Multiply(x="N APD Samp/step", y="Scan steps (MCL)") -> (x*y=w1281:dbl)
        n812 = local read "APD Samples/FIFO Acq."() -> (w1278:dbl)
        n813 = Multiply(x=w1281, y=u64 2) -> (x*y=w1280:dbl)
        "Data points/scan (f+b)" <- w1280
        n814 = Multiply(x=w1280, y=w1271) -> (x*y=w1298:dbl)
        "Data points/scans (MCL)" <- w1298
        n815 = Multiply(x=w1279, y=w1280) -> (x*y=w1272:dbl)
        "Time/f+b scan (s) (MCL)" <- w1272
        n816 = Divide(x=w1298, y=w1278) -> (x/y=→"N sets should be saved (MCL)":dbl)
        n817 = Multiply(x=w1272, y=w1271) -> (x*y=→"Total Time (s)":dbl)
        n818 = Not(x="Fast Scan Dir") -> (.not. x?=w1276:bool)
        n819 = xnode "Read/Write Control"("FPGA VI Reference In"=w1302, "error in"=w1301, "Scan steps (MCL)"="Scan steps (MCL)", "Number of scans (MCL)"=w1271, "Cycles per step (MCL)"=w1289, "Scan freq.  increment (MCL)"=w1269, "1D or 2D Scan?"="2D or 1D Scan", "MCL Scan Axis"=w1276, "Cont. Scan (MCL)"="Continuous MCL Scanning") -> ("error out"=w1300:errorcluster)  [unwired: 1 out]
      }
      event "Read Cal": Value Change {
        w1304 = 1000.0 ("y")
        n820 = event-data() -> ()  [unwired: 7 out]
        n821 = local read "Save file name"() -> (w1329:path)
        n822 = local write "Read Cal"(FALSE ("Read Cal")) -> ()
        n823 = Strip Path(path=w1329) -> (stripped path=w1328:path)  [unwired: 1 out]
        n824 = Path To String(path=w1328) -> (string=w1327:string)
        n825 = Concatenate Strings(w1327, "\\current.cal" ("string")) -> (w1325:string)
        n826 = String To Path(string=w1325) -> (path=w1324:path)
        n827 = Open/Create/Replace File(file path (use dialog)=w1324, operation (0:open)=T23."open", access (0:read/write)=enum16{"read/write", "read-only", "write-only"}."read-only") -> (refnum out=w1332:refnum<file>, error out=w1318:errorcluster)  [unwired: 1 in, 3 out]
        n828 = Deny Access(4:w1318, 7:w1332) -> (0:w1317:errorcluster, 3:w1323:refnum<file>)  [unwired: 1 out]
        n829 = Read from Binary File(5:0.0, 8:w1317, 9:T29."big-endian, network order" ("byte order (0:big-endian, network order)"), 10:-1 ("count (1)"), 11:w1323) -> (0:w1316:errorcluster, 2:w1314:dbl[], 3:w1319:refnum<file>)  [unwired: 2 out]
        n830 = Array To Cluster(array=w1314) -> (cluster=w1313:T31)
        n831 = Unbundle(w1313) -> ("[0]"=w1312:dbl, "[1]"=w1311:dbl, "[2]"=w1310:dbl, "[3]"=w1309:dbl, "[4]"=w1308:dbl, "[5]"=w1307:dbl)
        n832 = Close File(refnum=w1319, error in=w1316) -> (error out=→"Read cal error":errorcluster)  [unwired: 1 out]
        n833 = Multiply(x=w1307, y=w1304) -> (x*y=w1305:dbl)
        n834 = local write "T2 kappa_x (pN/nm)"(w1309) -> ()
        n835 = local write "T1 kappa_x (pN/nm)"(w1310) -> ()
        n836 = local write "T1 alpha_x (nm/V)"(w1312) -> ()
        n837 = local write "T2 alpha_x (nm/V)"(w1311) -> ()
        n838 = Multiply(x=w1308, y=w1304) -> (x*y=w1306:dbl)
        n839 = local write "T1 offset_x (mV)"(w1306) -> ()
        n840 = local write "T2 offset_x (mV)"(w1305) -> ()
      }
      event "Abort MCL Scan": Value Change {
        n841 = event-data() -> ()  [unwired: 7 out]
        n842 = local write "MCL Scanning"(FALSE ("MCL Scanning")) -> ()
        n843 = xnode "Read/Write Control"("FPGA VI Reference In"=w1337, "error in"=w1336, "Abort scan (MCL)"="Abort MCL Scan") -> ("error out"=w1335:errorcluster)  [unwired: 1 out]
      }
      event "Update Count (MCL)": Value Change {
        n844 = event-data() -> ()  [unwired: 7 out]
        n845 = xnode "Read/Write Control"("FPGA VI Reference In"=w1341, "error in"=w1340, "MCL count"="Update Count (MCL)") -> ("error out"=w1339:errorcluster)  [unwired: 1 out]
      }
      event "Phase adjust (MCL)", "+ phase (MCL)", "- phase (MCL)": Value Change {
        n846 = event-data() -> ()  [unwired: 7 out]
        n847 = Negate(x="Phase adjust (MCL)") -> (-x=w1350:i16)
        n848 = Select(t=w1350, s="- phase (MCL)", f="Phase adjust (MCL)") -> (s? t:f=w1348:i16)
        n849 = Or(x="- phase (MCL)", y="+ phase (MCL)") -> (x .or. y?=w1343:bool)
        n850 = xnode "Read/Write Control"("FPGA VI Reference In"=w1352, "error in"=w1351, "Phase count adjustment (MCL)"=w1348) -> ("FPGA VI Reference Out"=w1344:T19, "error out"=w1345:errorcluster)
        n851 = xnode "Read/Write Control"("FPGA VI Reference In"=w1344, "error in"=w1345, "+ phase (MCL)"=w1343) -> ("error out"=w1342:errorcluster)  [unwired: 1 out]
      }
      event "Abort AOD Scan": Value Change {
        n852 = event-data() -> ()  [unwired: 7 out]
        n853 = xnode "Read/Write Control"("FPGA VI Reference In"=w1356, "error in"=w1355, "Abort scan"="Abort AOD Scan") -> ("error out"=w1354:errorcluster)  [unwired: 1 out]
      }
      event "Continuous AOD Scanning": Value Change {
        n854 = event-data() -> ()  [unwired: 7 out]
        n855 = xnode "Read/Write Control"("FPGA VI Reference In"=w1360, "error in"=w1359, "Cont. Scan"="Continuous AOD Scanning") -> ("error out"=w1358:errorcluster)  [unwired: 1 out]
      }
      event "Index": Value Change {
        n856 = event-data() -> ()  [unwired: 7 out]
        n857 = call "Create new save file.vi"("Insert"="", "Ext"=".dat" ("string"), "Index In"="Index") -> ("Path Out"=→"Save file name":path, "Index Out"=w1361:dbl)
        "Save index" <- w1361
        n858 = local write "Index"(w1361) -> ()
      }
      event "AO1", "AO2": Value Change {
        w1376 = 10.0 ("y")
        w1375 = 32767.0 ("y")
        n859 = event-data() -> ()  [unwired: 7 out]
        n860 = local read "AO2"() -> (w1374:dbl)
        n861 = local read "AO1"() -> (w1371:dbl)
        n862 = Multiply(x=w1371, y=w1375) -> (x*y=w1370:dbl)
        n863 = Multiply(x=w1374, y=w1375) -> (x*y=w1373:dbl)
        n864 = Divide(x=w1370, y=w1376) -> (x/y=w1369:dbl)
        n865 = Divide(x=w1373, y=w1376) -> (x/y=w1372:dbl)
        n866 = To Word Integer(number=w1369) -> (16bit integer=w1377:i16)
        n867 = To Word Integer(number=w1372) -> (16bit integer=w1378:i16)
        n868 = xnode "Read/Write Control"("FPGA VI Reference In"=w1368, "error in"=w1367, "AO1"=w1377, "AO2"=w1378) -> ("error out"=w1366:errorcluster)  [unwired: 1 out]
      }
      event "Inject Bottom:": Value Change {
        n869 = event-data() -> ()  [unwired: 7 out]
        n870 = disable-structure shown="Enabled" {
          disable-tunnel: "Inject Bottom:" -> [w1380 w1420]
          frame Disabled {
            n871 = local read "Chemyx Syringe Pump Serial Port"() -> (w1381:refnum<visa-resource-name>)
            n872 = local read "Pump write delay (ms)"() -> (w1382:dbl)
            n873 = case shown="True" w1380 {
              tunnel: w1382 -> [w1388 w1402]
              tunnel: w1381 -> [w1385 w1401]
              frame False {
                n874 = flat-sequence {
                  tunnel: w1385 -> [w1389]
                  tunnel: [w1389] -> w1386
                  tunnel: w1388 -> [_]
                  tunnel: [w1392] -> w1387
                  tunnel: w1386 -> [w1392]
                  tunnel: w1387 -> [w1393]
                  tunnel: [w1393] -> w1383
                  tunnel: [w1395] -> w1384
                  tunnel: w1383 -> [w1395]
                  tunnel: w1384 -> [w1397]
                  frame #0 {
                    n875 = call "Write to pump.vi"("string"="enter pump1", "VISA resource name"=w1389) -> ()  [unwired: 1 out]
                  }
                  frame #1 {
                    n876 = Wait (ms)(milliseconds to wait="Pump pause delay (ms)") -> ()  [unwired: 1 out]
                  }
                  frame #2 {
                    n877 = call "Write to pump.vi"("string"="stop", "VISA resource name"=w1393) -> ()  [unwired: 1 out]
                  }
                  frame #3 {
                    n878 = Wait (ms)(milliseconds to wait=u32 500) -> ()  [unwired: 1 out]
                  }
                  frame #4 {
                    n879 = call "Write to pump.vi"("string"="stop", "VISA resource name"=w1397) -> ()  [unwired: 1 out]
                  }
                }
              }
              frame True {
                n880 = flat-sequence {
                  tunnel: w1401 -> [w1411]
                  tunnel: w1402 -> [w1406]
                  tunnel: w1402 -> [w1413]
                  tunnel: w1401 -> [w1414]
                  tunnel: [w1414] -> w1399
                  tunnel: [w1416] -> w1400
                  tunnel: w1399 -> [w1416]
                  tunnel: w1400 -> [w1418]
                  frame #0 {
                    n881 = local read "All Pump Parameters"() -> (w1405:T6)
                    n882 = Unbundle By Name(w1405) -> ("Pump 1"=w1412:T32)
                    n883 = call "Set pump parameters.vi"("Pump write delay (ms)"=w1406, "Volume (uL)"="Ch 2 Inject Volume (uL)", "Rate (uL/h)"="Ch 1 Inject Rate (ul/h)", "Units"=4.0, "Pump #"=1.0, "Pump Parameters In"=w1412, "VISA resource name"=w1411) -> ("Pump Parameters Out"=w1404:T32)  [unwired: 3 in]
                    n884 = Bundle By Name(cluster=w1405, "Pump 1"=w1404) -> (w1403:T6)
                    n885 = local write "All Pump Parameters"(w1403) -> ()
                  }
                  frame #1 {
                    n886 = Wait (ms)(milliseconds to wait=w1413) -> ()  [unwired: 1 out]
                  }
                  frame #2 {
                    n887 = call "Write to pump.vi"("string"="start", "VISA resource name"=w1414) -> ()  [unwired: 1 out]
                  }
                  frame #3 {
                    n888 = Wait (ms)(milliseconds to wait=u32 500) -> ()  [unwired: 1 out]
                  }
                  frame #4 {
                    n889 = call "Write to pump.vi"("string"="start", "VISA resource name"=w1418) -> ()  [unwired: 1 out]
                  }
                }
              }
            }
          }
          frame Enabled {
            n890 = call "hamilton_controller.vi"("Open?"=w1420, "valve"=enum16{"A", "B", "C", "D", "ALL"}."B", "action"=T20."MOVE VALVE") -> ()  [unwired: 8 in, 1 out]
          }
        }
      }
      event "Inject Top:": Value Change {
        n891 = event-data() -> ()  [unwired: 7 out]
        n892 = disable-structure shown="Disabled" {
          disable-tunnel: "Inject Top:" -> [_ w1464]
          frame Disabled {
            n893 = local read "Pump write delay (ms)"() -> (w1425:dbl)
            n894 = case shown="False" w1426 {
              tunnel: w1425 -> [w1432 w1446]
              tunnel: "Chemyx Syringe Pump Serial Port" -> [w1429 w1445]
              frame False {
                n895 = flat-sequence {
                  tunnel: w1429 -> [w1433]
                  tunnel: [w1433] -> w1430
                  tunnel: w1432 -> [_]
                  tunnel: [w1436] -> w1431
                  tunnel: w1430 -> [w1436]
                  tunnel: w1431 -> [w1437]
                  tunnel: [w1437] -> w1427
                  tunnel: [w1439] -> w1428
                  tunnel: w1427 -> [w1439]
                  tunnel: w1428 -> [w1441]
                  frame #0 {
                    n896 = call "Write to pump.vi"("string"="enter pump3", "VISA resource name"=w1433) -> ()  [unwired: 1 out]
                  }
                  frame #1 {
                    n897 = local read "Pump pause delay (ms)"() -> (w1435:u32)
                    n898 = Wait (ms)(milliseconds to wait=w1435) -> ()  [unwired: 1 out]
                  }
                  frame #2 {
                    n899 = call "Write to pump.vi"("string"="stop", "VISA resource name"=w1437) -> ()  [unwired: 1 out]
                  }
                  frame #3 {
                    n900 = Wait (ms)(milliseconds to wait=u32 0) -> ()  [unwired: 1 out]
                  }
                  frame #4 {
                    n901 = call "Write to pump.vi"("string"="stop", "VISA resource name"=w1441) -> ()  [unwired: 1 out]
                  }
                }
              }
              frame True {
                n902 = flat-sequence {
                  tunnel: w1445 -> [w1455]
                  tunnel: w1446 -> [w1450]
                  tunnel: w1446 -> [w1457]
                  tunnel: w1445 -> [w1458]
                  tunnel: [w1458] -> w1443
                  tunnel: [w1461] -> w1444
                  tunnel: w1443 -> [w1461]
                  tunnel: w1444 -> [w1462]
                  frame #0 {
                    n903 = local read "All Pump Parameters"() -> (w1449:T6)
                    n904 = Unbundle By Name(w1449) -> ("Pump 3"=w1456:T32)
                    n905 = call "Set pump parameters.vi"("Pump write delay (ms)"=w1450, "Volume (uL)"="Ch 3 Inject Volume (uL)", "Rate (uL/h)"="Ch 3 Inject Rate (ul/h)", "Units"=4.0, "Pump #"=3.0, "Pump Parameters In"=w1456, "VISA resource name"=w1455) -> ("Pump Parameters Out"=w1448:T32)  [unwired: 3 in]
                    n906 = Bundle By Name(cluster=w1449, "Pump 3"=w1448) -> (w1447:T6)
                    n907 = local write "All Pump Parameters"(w1447) -> ()
                  }
                  frame #1 {
                    n908 = Wait (ms)(milliseconds to wait=w1457) -> ()  [unwired: 1 out]
                  }
                  frame #2 {
                    n909 = call "Write to pump.vi"("string"="start", "VISA resource name"=w1458) -> ()  [unwired: 1 out]
                  }
                  frame #3 {
                    n910 = Wait (ms)(milliseconds to wait=u32 500) -> ()  [unwired: 1 out]
                  }
                  frame #4 {
                    n911 = call "Write to pump.vi"("string"="start", "VISA resource name"=w1462) -> ()  [unwired: 1 out]
                  }
                }
              }
            }
          }
          frame Enabled {
            n912 = call "hamilton_controller.vi"("Open?"=w1464, "valve"=enum16{"A", "B", "C", "D", "ALL"}."A", "action"=T20."MOVE VALVE") -> ()  [unwired: 8 in, 1 out]
          }
        }
      }
      event "Inject Valve B": Value Change {
        n913 = event-data() -> ()  [unwired: 7 out]
        n914 = disable-structure shown="Enabled" {
          disable-tunnel: "Inject Valve B" -> [w1468 w1488]
          frame Disabled {
            n915 = local read "Pump write delay (ms)"() -> (w1470:dbl)
            n916 = flat-sequence {
              tunnel: w1469 -> [w1483]
              tunnel: w1470 -> [w1479]
              tunnel: w1468 -> [_]
              tunnel: w1470 -> [w1485]
              tunnel: w1469 -> [w1486]
              frame #0 {
                n917 = local read "All Pump Parameters"() -> (w1478:T6)
                n918 = Multiply(x=60.0, y="Flush Center Ch Rate (ul/m)") -> (x*y=w1475:dbl)
                n919 = Unbundle By Name(w1478) -> ("Pump 2"=w1484:T32)
                n920 = call "Set pump parameters.vi"("Pump write delay (ms)"=w1479, "Volume (uL)"="Flush Center Ch Volume (uL)", "Rate (uL/h)"=w1475, "Units"=3.0, "Pump #"=2.0, "Pump Parameters In"=w1484, "VISA resource name"=w1483) -> ("Pump Parameters Out"=w1477:T32)  [unwired: 3 in]
                n921 = Bundle By Name(cluster=w1478, "Pump 2"=w1477) -> (w1476:T6)
                n922 = local write "All Pump Parameters"(w1476) -> ()
                n923 = Add(x="Flush Center Ch Volume (uL)", y="Total Volume\nFlushed (uL)") -> (x+y=w1472:dbl)
                n924 = local write "Total Volume\nFlushed (uL)"(w1472) -> ()
              }
              frame #1 {
                n925 = Wait (ms)(milliseconds to wait=w1485) -> ()  [unwired: 1 out]
              }
              frame #2 {
                n926 = call "Write to pump.vi"("string"="start", "VISA resource name"=w1486) -> ()  [unwired: 1 out]
              }
            }
            n927 = local read "Chemyx Syringe Pump Serial Port"() -> (w1469:refnum<visa-resource-name>)
          }
          frame Enabled {
            n928 = call "hamilton_controller.vi"("Open?"=w1488, "valve"=enum16{"A", "B", "C", "D", "ALL"}."B", "action"=T20."MOVE VALVE") -> ()  [unwired: 8 in, 1 out]
          }
        }
      }
      event "Inject Main:": Value Change {
        n929 = event-data() -> ()  [unwired: 7 out]
        n930 = call "hamilton_controller.vi"("Open?"="Inject Main:", "valve"=enum16{"A", "B", "C", "D", "ALL"}."C", "action"=T20."MOVE VALVE") -> ()  [unwired: 8 in, 1 out]
      }
      event "Inject Shunt:": Value Change {
        n931 = event-data() -> ()  [unwired: 7 out]
        n932 = call "hamilton_controller.vi"("Open?"="Inject Shunt:", "valve"=enum16{"A", "B", "C", "D", "ALL"}."D", "action"=T20."MOVE VALVE") -> ()  [unwired: 8 in, 1 out]
      }
      event "Flip Green Filter": Value Change {
        n933 = event-data() -> ()  [unwired: 7 out]
        n934 = local write "Flip Green Filter"("Flip Green Filter") -> ()
        n935 = flat-sequence {
          tunnel: w1504 -> [w1509]
          tunnel: w1503 -> [w1508]
          tunnel: [w1506] -> w1501
          tunnel: [w1505] -> w1500
          tunnel: [w1511] -> w1499
          tunnel: w1501 -> [w1511]
          tunnel: [w1510] -> w1498
          tunnel: w1500 -> [w1510]
          tunnel: w1499 -> [w1515]
          tunnel: w1498 -> [w1514]
          tunnel: [w1513] -> w1502
          frame #0 {
            n936 = xnode "Read/Write Control"("FPGA VI Reference In"=w1509, "error in"=w1508, "Green Filter Flipper"=TRUE) -> ("FPGA VI Reference Out"=w1506:T19, "error out"=w1505:errorcluster)
          }
          frame #1 {
            n937 = Wait (ms)(milliseconds to wait=u32 100) -> ()  [unwired: 1 out]
          }
          frame #2 {
            n938 = xnode "Read/Write Control"("FPGA VI Reference In"=w1515, "error in"=w1514, "Green Filter Flipper"=FALSE) -> ("error out"=w1513:errorcluster)  [unwired: 1 out]
          }
        }
      }
      event "Pump 1 contents", "Pump 3 contents": Value Change {
        n939 = event-data() -> ()  [unwired: 7 out]
        n940 = local read "Pump 1 contents"() -> (→"Pump 1 cont disp":string)
        n941 = local read "Pump 3 contents"() -> (→"Pump 3 cont disp":string)
      }
      event "Reset Trap Pos. FB": Value Change {
        n942 = event-data() -> ()  [unwired: 7 out]
        n943 = xnode "Read/Write Control"("FPGA VI Reference In"=w1521, "error in"=w1520, "Trap Pos. FB Reset"="Reset Trap Pos. FB") -> ()  [unwired: 2 out]
      }
      event "Trap Pos. FB ON": Value Change {
        n944 = event-data() -> ()  [unwired: 7 out]
        n945 = xnode "Read/Write Control"("FPGA VI Reference In"=w1524, "error in"=w1523, "Force feedback"="Trap Pos. FB ON") -> ()  [unwired: 2 out]
      }
      event "Trap Pos. FB Range", "Trap Pos. FB Gains", "Trap Pos. FB Mult Factor", "Trap Pos. FB Offset Factor", "Trap Pos FB Negate Action", "Trap Pos FB Monitor\nT1 or T2": Value Change {
        n946 = event-data() -> ()  [unwired: 7 out]
        n947 = xnode "Read/Write Control"("FPGA VI Reference In"=w1533, "error in"=w1532, "Trap Pos. FB Range"="Trap Pos. FB Range", "Trap Pos. FB Gains"="Trap Pos. FB Gains", "Trap Pos. FB Mult Factor"="Trap Pos. FB Mult Factor", "Trap Pos. FB Offset Factor"="Trap Pos. FB Offset Factor", "Trap Pos FB Negate Action"="Trap Pos FB Negate Action", "Trap Pos FB Monitor T1 or T2"="Trap Pos FB Monitor\nT1 or T2", "AI1 X Scale"="Trap Pos. AI1 X Pre-scale") -> ()  [unwired: 2 out]
      }
      event "Trap Pos FB SP": Value Change {
        n948 = event-data() -> ()  [unwired: 7 out]
        n949 = xnode "Read/Write Control"("FPGA VI Reference In"=w1536, "error in"=w1535, "Trap Pos. FB SP"="Trap Pos FB SP") -> ()  [unwired: 2 out]
      }
      event "Set SP to Reading": Value Change {
        n950 = event-data() -> ()  [unwired: 7 out]
        n951 = local read "Trap Pos FB Monitor\nT1 or T2"() -> (w1544:bool)
        n952 = local read "Trap X AI1 (DMA)"() -> (w1547:T13)
        n953 = local read "Trap X (AI1)"() -> (w1550:T1)
        n954 = Unbundle By Name(w1550) -> ("Trap 1"=w1549:fxp<+/-,16,1>, "Trap 2"=w1548:fxp<+/-,16,1>)
        n955 = Unbundle By Name(w1547) -> ("Set 1"=w1546:fxp<+/-,16,1>, "Set 2"=w1545:fxp<+/-,16,1>)
        n956 = Select(t=w1549, s=w1544, f=w1548) -> (s? t:f=w1543:fxp<+/-,16,1>)
        n957 = Select(t=w1546, s=w1544, f=w1545) -> (s? t:f=w1542:fxp<+/-,16,1>)
        n958 = Not(x="Set SP Using...") -> (.not. x?=w1537:bool)
        n959 = Select(t=w1543, s=w1537, f=w1542) -> (s? t:f=w1538:fxp<+/-,16,1>)
        n960 = xnode "Read/Write Control"("FPGA VI Reference In"=w1540, "error in"=w1539, "Trap Pos. FB SP"=w1538) -> ()  [unwired: 2 out]
        n961 = local write "Trap Pos FB SP"(w1538) -> ()
      }
      event "Trap Pos. FB Out Scale 2^n": Value Change {
        n962 = event-data() -> ()  [unwired: 7 out]
        n963 = Scale By Power Of 2(n="Trap Pos. FB Out Scale 2^n", x=ext 1.0) -> (x*2^n=w1552:ext)
        n964 = property on="Trap Pos. FB Mult Factor" class="DigNum (strict)"("Val(Sgnl)"=w1552) -> ()  [unwired: 2 in, 2 out]
      }
      event "Trap Pos FB Int Count": Value Change {
        n965 = event-data() -> ()  [unwired: 7 out]
        n966 = xnode "Read/Write Control"("FPGA VI Reference In"=w1557, "error in"=w1556, "Trap Pos FB Int Count"="Trap Pos FB Int Count") -> ()  [unwired: 2 out]
      }
    }
    "error out 2" <- w735
    n967 = node-c288() -> ()  [unwired: 1 in, 1 out]
  }
  n968 = timed-loop "Run Scripts, including: stage motion" {
    timing: w69 -> [_]
    timing-out: [_] -> w68
    tunnel: w24 -> [_]
    stop <- w1559 stop-if-true
    n969 = node-c288() -> ()  [unwired: 1 in, 1 out]
    n970 = event shown="[1] Timeout" {
      selector: _ -> [_ _ _ _ _ _ _ _ _ _ _ _]
      dyn-events: _ -> [_ _ _ _ _ _ _ _ _ _ _ _]
      timeout: 50 -> [_ _ _ _ _ _ _ _ _ _ _ _]
      tunnel: ["Move Cap. 1 (DNA Top)" _ "Cal/Data Acq. Spot" "Dump Beads" "Dip for Protein" _ "Got ADig bead" "Got DNA bead" "Take Stepping Data" _ "Take Detection Laser\nImage" _] -> _
      tunnel: [_ _ _ _ _ _ _ _ _ _ _ w1767] -> w1559
      event "Move Cap. 1 (DNA Top)": Value Change {
        n971 = event-data() -> ()  [unwired: 1 in, 5 out]
        n972 = local write "Move Cap. 1 (DNA Top)"(FALSE ("Move Cap. 1 (DNA Right)")) -> ()
        n973 = flat-sequence {
          tunnel: "Cap 1 Samp Flow ON" -> [w1565]
          frame #0 {
            n974 = local write "Stage Moving"(FALSE ("Stage Moving")) -> ()
            n975 = case "stop flow" shown="True" w1565 {
              frame False {
              }
              frame True {
                n976 = call "hamilton_controller.vi"("Open?"=FALSE, "valve"=enum16{"A", "B", "C", "D", "ALL"}."C", "action"=T20."MOVE VALVE") -> ()  [unwired: 8 in, 1 out]
              }
            }
            n977 = case shown="True" TRUE {
              tunnel: "Cap 1 T ON" -> [w1574 w1575]
              frame False {
                n978 = property on="Trap 1 (ON/OFF)" class="Bool (strict)"("Val(Sgnl)"=w1574) -> ()  [unwired: 2 in, 2 out]
              }
              frame True {
                n979 = property on="Trap 2 (ON/OFF)" class="Bool (strict)"("Val(Sgnl)"=w1575) -> ()  [unwired: 2 in, 2 out]
              }
            }
            n980 = call <vilib>:"Beep.vi"() -> ()  [unwired: 3 in, 9 out]
            n981 = case shown="True" "Cap 1 Flow ON" {
              frame False {
              }
              frame True {
                n982 = property on="Inject Top:" class="Bool (strict)"("Val(Sgnl)"=TRUE ("Value (Signaling)")) -> ()  [unwired: 2 in, 2 out]
              }
            }
          }
        }
      }
      event Timeout {
        n983 = event-data() -> ()  [unwired: 1 in, 2 out]
      }
      event "Cal/Data Acq. Spot": Value Change {
        # "wait for calibration file\nto be written"
        # "signal save cal true\nthis tells the data \nacquisition loop to\nstart sending the data\nto a calibration file"
        # "separate traps to\nthe desired trap delta"
        # "move stage to data acquisition spot"
        # "CHANGE FISH FOR TETHER BACK\nTO TRUE VALUE HERE."
        n984 = event-data() -> ()  [unwired: 1 in, 5 out]
        n985 = local write "Cal/Data Acq. Spot"(FALSE ("Cal/Data Acq. Spot")) -> ()
        n986 = flat-sequence {
          tunnel: ["Cal @ (MHz)"] -> w1576
          tunnel: w1576 -> [w1586]
          tunnel: w1576 -> [w1607]
          frame #0 {
            n987 = property on="Trap Delta (MHz)" class="Slide (strict)"("Val(Sgnl)"="Cal @ (MHz)") -> ()  [unwired: 2 in, 2 out]
            n988 = call <vilib>:"Beep.vi"() -> ()  [unwired: 3 in, 9 out]
          }
          frame #1 {
            n989 = Wait (ms)(milliseconds to wait=u32 100) -> ()  [unwired: 1 out]
          }
          frame #2 {
            n990 = property on="Save Calibration" class="Bool (strict)"("Val(Sgnl)"=TRUE ("Value (Signaling)")) -> ()  [unwired: 2 in, 2 out]
          }
          frame #3 {
            n991 = Wait (ms)(milliseconds to wait=u32 4000) -> ()  [unwired: 1 out]
          }
          frame #4 {
            n992 = while {
              stop <- w1583 stop-if-true
              n993 = local read "Saving..."() -> (w1584:bool)
              n994 = Wait (ms)(milliseconds to wait=u32 100) -> ()  [unwired: 1 out]
              n995 = Not(x=w1584) -> (.not. x?=w1583:bool)
            }
          }
          frame #5 {
            n996 = case shown="True" "W/ Offset 1" {
              tunnel: w1586 -> [_ w1588]
              frame False {
              }
              frame True {
                n997 = stacked-sequence {
                  tunnel: w1588 -> [_ _ _ _ _ _ _ w1605]
                  frame #0 {
                    n998 = Replace Array Subset(array=u32[] [0] ("Index Values"), new element="Offset 1 Set", index=0) -> (w1589:u32[])
                    n999 = property on="Saved AOD Raster Scan Parameter Sets" class="Arr (strict)"("Index Values"=w1589) -> ()  [unwired: 2 in, 2 out]
                    n1000 = property on="Trap Delta (MHz)" class="Slide (strict)"("Val(Sgnl)"="Offset 1 Start (MHz)") -> ()  [unwired: 2 in, 2 out]
                  }
                  frame #1 {
                    n1001 = Wait (ms)(milliseconds to wait=u32 200) -> ()  [unwired: 1 out]
                  }
                  frame #2 {
                    n1002 = property on="Load parameters" class="Bool (strict)"("Val(Sgnl)"=TRUE ("Value (Signaling)")) -> ()  [unwired: 2 in, 2 out]
                  }
                  frame #3 {
                    n1003 = Wait (ms)(milliseconds to wait=u32 200) -> ()  [unwired: 1 out]
                  }
                  frame #4 {
                    n1004 = property on="Trap Raster Scan" class="Bool (strict)"("Val(Sgnl)"=TRUE ("Value (Signaling)")) -> ()  [unwired: 2 in, 2 out]
                  }
                  frame #5 {
                    n1005 = Wait (ms)(milliseconds to wait=u32 2000) -> ()  [unwired: 1 out]
                  }
                  frame #6 {
                    n1006 = while {
                      stop <- w1602 stop-if-true
                      n1007 = local read "Raster Scanning..."() -> (w1604:bool)
                      n1008 = local read "Saving..."() -> (w1600:bool)
                      n1009 = Wait (ms)(milliseconds to wait=u32 100) -> ()  [unwired: 1 out]
                      n1010 = Not(x=w1600) -> (.not. x?=w1599:bool)
                      n1011 = Not(x=w1604) -> (.not. x?=w1601:bool)
                      n1012 = And(x=w1601, y=w1599) -> (x .and. y?=w1602:bool)
                    }
                  }
                  frame #7 {
                    n1013 = property on="Trap Delta (MHz)" class="Slide (strict)"("Val(Sgnl)"=w1605) -> ()  [unwired: 2 in, 2 out]
                  }
                }
              }
            }
          }
          frame #6 {
            n1014 = local read "Save ave N"() -> (w1606:dbl)
            n1015 = case shown="True" "W/ Offset 2" {
              tunnel: w1607 -> [_ w1613]
              tunnel: w1606 -> [_ w1612]
              frame False {
                n1016 = Multiply(x="Cal read wait (s)", y=u32 1000 ("milliseconds to wait")) -> (x*y=w1610:u32)
                n1017 = Wait (ms)(milliseconds to wait=w1610) -> ()  [unwired: 1 out]
              }
              frame True {
                n1018 = stacked-sequence {
                  tunnel: w1613 -> [_ _ _ _ _ _ _ _ _ w1634 _ _]
                  tunnel: w1612 -> [_ _ _ _ _ _ _ _ _ w1632 _ _]
                  frame #0 {
                    n1019 = property on="Save ave N" class="DigNum (strict)"("Val(Sgnl)"=1.0 ("Value (Signaling)")) -> ()  [unwired: 2 in, 2 out]
                  }
                  frame #1 {
                    n1020 = Wait (ms)(milliseconds to wait=u32 500) -> ()  [unwired: 1 out]
                  }
                  frame #2 {
                    n1021 = property on="Trap Delta (MHz)" class="Slide (strict)"("Val(Sgnl)"="Offset 2 Start (MHz)") -> ()  [unwired: 2 in, 2 out]
                    n1022 = Replace Array Subset(array=u32[] [0] ("Index Values"), new element="Offset 2 Set", index=0) -> (w1618:u32[])
                    n1023 = property on="Saved AOD Raster Scan Parameter Sets" class="Arr (strict)"("Index Values"=w1618) -> ()  [unwired: 2 in, 2 out]
                  }
                  frame #3 {
                    n1024 = Wait (ms)(milliseconds to wait=u32 500) -> ()  [unwired: 1 out]
                  }
                  frame #4 {
                    n1025 = property on="Load parameters" class="Bool (strict)"("Val(Sgnl)"=TRUE ("Value (Signaling)")) -> ()  [unwired: 2 in, 2 out]
                  }
                  frame #5 {
                    n1026 = Wait (ms)(milliseconds to wait=u32 500) -> ()  [unwired: 1 out]
                  }
                  frame #6 {
                    n1027 = property on="Trap Raster Scan" class="Bool (strict)"("Val(Sgnl)"=TRUE ("Value (Signaling)")) -> ()  [unwired: 2 in, 2 out]
                  }
                  frame #7 {
                    n1028 = Wait (ms)(milliseconds to wait=u32 2000) -> ()  [unwired: 1 out]
                  }
                  frame #8 {
                    n1029 = while {
                      stop <- w1627 stop-if-true
                      n1030 = local read "Raster Scanning..."() -> (w1630:bool)
                      n1031 = local read "Saving..."() -> (w1628:bool)
                      n1032 = Wait (ms)(milliseconds to wait=u32 100) -> ()  [unwired: 1 out]
                      n1033 = Not(x=w1628) -> (.not. x?=w1626:bool)
                      n1034 = Not(x=w1630) -> (.not. x?=w1629:bool)
                      n1035 = And(x=w1629, y=w1626) -> (x .and. y?=w1627:bool)
                    }
                  }
                  frame #9 {
                    n1036 = property on="Trap Delta (MHz)" class="Slide (strict)"("Val(Sgnl)"=w1634) -> ()  [unwired: 2 in, 2 out]
                    n1037 = property on="Saved AOD Raster Scan Parameter Sets" class="Arr (strict)"("Index Values"=u32[] [0]) -> ()  [unwired: 2 in, 2 out]
                    n1038 = property on="Save ave N" class="DigNum (strict)"("Val(Sgnl)"=w1632) -> ()  [unwired: 2 in, 2 out]
                  }
                  frame #10 {
                    n1039 = Wait (ms)(milliseconds to wait=u32 500) -> ()  [unwired: 1 out]
                  }
                  frame #11 {
                    n1040 = property on="Load parameters" class="Bool (strict)"("Val(Sgnl)"=TRUE ("Value (Signaling)")) -> ()  [unwired: 2 in, 2 out]
                  }
                }
              }
            }
          }
          frame #7 {
            n1041 = property on="Read Cal" class="Bool (strict)"("Val(Sgnl)"=TRUE ("Value (Signaling)")) -> ()  [unwired: 2 in, 2 out]
          }
          frame #8 {
            n1042 = Wait (ms)(milliseconds to wait=u32 500) -> ()  [unwired: 1 out]
          }
          frame #9 {
            n1043 = property on="Fish for Tether" class="Bool (strict)"("Val(Sgnl)"=FALSE ("Value (Signaling)")) -> ()  [unwired: 2 in, 2 out]
          }
        }
      }
      event "Dump Beads": Value Change {
        # "SCRIPT TO REMOVE BOTH BEADS FROM THE TRAPS. TURNS ON LIGHT WHICH INDICATES THAT STAGE IS MOVING. THEN STOPS SAVING DATA. \nSETS Sample Channel Flow TO TRUE. STOPS INTERLACING GREEN FLUORESCENCE. TURNS OFF Tether INDICATOR BECAUSE WE ARE THROWING IT\nAWAY. SHUTS OFF TRAP POSITION FEEDBACK."
        n1044 = event-data() -> ()  [unwired: 1 in, 5 out]
        n1045 = flat-sequence {
          frame #0 {
            w1641 = FALSE ("Fl. Triggered...")
            w1642 = TRUE ("Stage Moving")
            n1046 = local read "Saving..."() -> (w1643:bool)
            n1047 = local write "Fl. Triggered..."(w1641) -> ()
            n1048 = local write "Stage Moving"(w1642) -> ()
            n1049 = local write "Tether"(w1641) -> ()
            n1050 = property on="Green Laser ON/Interlacing" class="Bool (strict)"("Val(Sgnl)"=w1641) -> ()  [unwired: 2 in, 2 out]
            n1051 = property on="Trap Pos. FB ON" class="Bool (strict)"("Val(Sgnl)"=w1641) -> ()  [unwired: 2 in, 2 out]
            n1052 = property on="Inject Main:" class="Bool (strict)"("Val(Sgnl)"=w1642) -> ()  [unwired: 2 in, 2 out]
            n1053 = local write "Stop Saving"(w1643) -> ()
          }
          frame #1 {
            w1644 = FALSE ("Value (Signaling)")
            # "TURNS TRAPS OFF SO THAT\nBEADS REMAIN AT DUMP \nBEADS POSITION"
            n1054 = property on="Trap 1 (ON/OFF)" class="Bool (strict)"("Val(Sgnl)"=w1644) -> ()  [unwired: 2 in, 2 out]
            n1055 = property on="Trap 2 (ON/OFF)" class="Bool (strict)"("Val(Sgnl)"=w1644) -> ()  [unwired: 2 in, 2 out]
            n1056 = call <vilib>:"Beep.vi"() -> ()  [unwired: 3 in, 9 out]
          }
          frame #2 {
            n1057 = property on="Goto Bottom (F7)" class="Bool (strict)"("Val(Sgnl)"=TRUE ("Value (Signaling)")) -> ()  [unwired: 2 in, 2 out]
          }
          frame #3 {
            n1058 = Wait (ms)(milliseconds to wait=u32 8000) -> ()  [unwired: 1 out]
          }
          frame #4 {
            n1059 = property on="Trap Delta (MHz)" class="Slide (strict)"("Val(Sgnl)"=20.0 ("Value (Signaling)")) -> ()  [unwired: 2 in, 2 out]
          }
          frame #5 {
            n1060 = property on="Trap 2 (ON/OFF)" class="Bool (strict)"("Val(Sgnl)"=TRUE ("Value (Signaling)")) -> ()  [unwired: 2 in, 2 out]
          }
          frame #6 {
            n1061 = property on="Inject Main:" class="Bool (strict)"("Val(Sgnl)"=FALSE ("Value (Signaling)")) -> ()  [unwired: 2 in, 2 out]
          }
        }
      }
      event "Dip for Protein": Value Change {
        n1062 = event-data() -> ()  [unwired: 1 in, 5 out]
        n1063 = flat-sequence {
          frame #0 {
            n1064 = case shown="True" "Move Trap Before?" {
              frame False {
              }
              frame True {
                n1065 = property on="Trap Delta (MHz)" class="Slide (strict)"("Val(Sgnl)"="Dip Trap Delta 1 (MHz)") -> ()  [unwired: 2 in, 2 out]
              }
            }
          }
          frame #1 {
            n1066 = Multiply(x="Duration (s)", y=1000.0) -> (x*y=w1653:dbl)
            n1067 = Wait (ms)(milliseconds to wait=w1653) -> ()  [unwired: 1 out]
          }
          frame #2 {
            n1068 = case shown="True" "Move Trap After?" {
              frame False {
              }
              frame True {
                n1069 = property on="Trap Delta (MHz)" class="Slide (strict)"("Val(Sgnl)"="Dip Trap Delta 2 (MHz)") -> ()  [unwired: 2 in, 2 out]
              }
            }
          }
          frame #3 {
            n1070 = case shown="True" "Green ON After?" {
              frame False {
              }
              frame True {
                n1071 = property on="Green Laser ON/Interlacing" class="Bool (strict)"("Val(Sgnl)"=TRUE ("Value (Signaling)")) -> ()  [unwired: 2 in, 2 out]
              }
            }
          }
          frame #4 {
            n1072 = Wait (ms)(milliseconds to wait=u32 500) -> ()  [unwired: 1 out]
          }
          frame #5 {
            n1073 = case shown="True" "Save Data After?" {
              frame False {
              }
              frame True {
                n1074 = property on="Start Saving" class="Bool (strict)"("Val(Sgnl)"=TRUE ("Value (Signaling)")) -> ()  [unwired: 2 in, 2 out]
              }
            }
          }
        }
      }
      event "Profile": Value Change {
        n1075 = event-data() -> ()  [unwired: 1 in, 5 out]
        n1076 = flat-sequence {
          frame #0 {
            w1663 = 0.0 ("element")
            n1077 = Build Array(w1663, "Y change (mm)", w1663) -> ()  [unwired: 1 out]
          }
          frame #1 {
            # "stop saving"
            n1078 = local write "Stop Saving"(TRUE ("Stop Saving")) -> ()
            n1079 = local write "Stage Moving"(FALSE ("Stage Moving")) -> ()
          }
        }
      }
      event "Got ADig bead": Value Change {
        n1080 = event-data() -> ()  [unwired: 1 in, 5 out]
        n1081 = property on="Move Cap. 1 (DNA Top)" class="Bool (strict)"("Val(Sgnl)"=TRUE ("Value (Signaling)")) -> ()  [unwired: 2 in, 2 out]
        n1082 = property on="Inject Bottom:" class="Bool (strict)"("Val(Sgnl)"=FALSE ("Value (Signaling)")) -> ()  [unwired: 2 in, 2 out]
      }
      event "Got DNA bead": Value Change {
        n1083 = event-data() -> ()  [unwired: 1 in, 5 out]
        n1084 = property on="Cal/Data Acq. Spot" class="Bool (strict)"("Val(Sgnl)"=TRUE ("Value (Signaling)")) -> ()  [unwired: 2 in, 2 out]
        n1085 = property on="Inject Top:" class="Bool (strict)"("Val(Sgnl)"=FALSE ("Value (Signaling)")) -> ()  [unwired: 2 in, 2 out]
      }
      event "Take Stepping Data": Value Change {
        n1086 = event-data() -> ()  [unwired: 1 in, 5 out]
        n1087 = local read "Save ave N"() -> (w1681:dbl)
        n1088 = flat-sequence {
          tunnel: w1681 -> [w1683]
          tunnel: [w1683] -> w1676
          tunnel: [w1685] -> w1677
          tunnel: w1676 -> [w1685]
          tunnel: [w1687] -> w1678
          tunnel: w1677 -> [w1687]
          tunnel: [w1690] -> w1679
          tunnel: w1678 -> [w1690]
          tunnel: [w1692] -> w1680
          tunnel: w1679 -> [w1692]
          tunnel: [w1694] -> w1674
          tunnel: w1680 -> [w1694]
          tunnel: w1674 -> [w1697]
          tunnel: [w1697] -> w1673
          tunnel: w1673 -> [w1698]
          tunnel: [w1698] -> w1675
          tunnel: w1675 -> [w1704]
          frame #0 {
            n1089 = property on="Save ave N" class="DigNum (strict)"("Val(Sgnl)"="Save ave factor") -> ()  [unwired: 2 in, 2 out]
          }
          frame #1 {
            n1090 = Wait (ms)(milliseconds to wait=u32 100) -> ()  [unwired: 1 out]
          }
          frame #2 {
            n1091 = local read "Offset 2 Start (MHz)"() -> (w1689:dbl)
            n1092 = property on="Saved AOD Raster Scan Parameter Sets" class="Arr (strict)"("Index Values"=u32[] [2]) -> ()  [unwired: 2 in, 2 out]
            n1093 = property on="Trap Delta (MHz)" class="Slide (strict)"("Val(Sgnl)"=w1689) -> ()  [unwired: 2 in, 2 out]
          }
          frame #3 {
            n1094 = property on="Load parameters" class="Bool (strict)"("Val(Sgnl)"=TRUE ("Value (Signaling)")) -> ()  [unwired: 2 in, 2 out]
          }
          frame #4 {
            n1095 = Wait (ms)(milliseconds to wait=u32 100) -> ()  [unwired: 1 out]
          }
          frame #5 {
            n1096 = property on="Trap Raster Scan" class="Bool (strict)"("Val(Sgnl)"=TRUE ("Value (Signaling)")) -> ()  [unwired: 2 in, 2 out]
          }
          frame #6 {
            n1097 = Wait (ms)(milliseconds to wait=u32 1000) -> ()  [unwired: 1 out]
          }
          frame #7 {
            n1098 = while {
              stop <- w1701 stop-if-true
              n1099 = local read "Raster Scanning..."() -> (w1703:bool)
              n1100 = local read "Saving..."() -> (w1702:bool)
              n1101 = Not(x=w1702) -> (.not. x?=w1699:bool)
              n1102 = Not(x=w1703) -> (.not. x?=w1700:bool)
              n1103 = And(x=w1700, y=w1699) -> (x .and. y?=w1701:bool)
            }
          }
          frame #8 {
            n1104 = property on="Save ave N" class="DigNum (strict)"("Val(Sgnl)"=w1704) -> ()  [unwired: 2 in, 2 out]
          }
        }
      }
      event "Step Size (nm)": Value Change {
        n1105 = event-data() -> ()  [unwired: 1 in, 5 out]
        n1106 = flat-sequence {
          frame #0 {
            n1107 = property on="Saved AOD Raster Scan Parameter Sets" class="Arr (strict)"("Index Values"=u32[] [1]) -> ()  [unwired: 2 in, 2 out]
          }
          frame #1 {
            n1108 = Multiply(x="N Steps", y="Step Size (nm)") -> (x*y=w1706:dbl)
            n1109 = property on="Scan Speed AOD (nm/s) 2" class="DigNum (strict)"("Value"="Step Size (nm)") -> ()  [unwired: 2 in, 2 out]
            n1110 = property on="Step Size AOD (nm) 2" class="DigNum (strict)"("Value"="Step Size (nm)") -> ()  [unwired: 2 in, 2 out]
            n1111 = property on="Scan Range AOD (nm) 2" class="DigNum (strict)"("Value"=w1706) -> ()  [unwired: 2 in, 2 out]
          }
        }
      }
      event "Take Detection Laser\nImage": Value Change {
        n1112 = event-data() -> ()  [unwired: 1 in, 5 out]
        n1113 = flat-sequence {
          tunnel: [w1734] -> w1724
          tunnel: [w1733] -> w1717
          tunnel: [w1732] -> w1709
          tunnel: [w1737] -> w1725
          tunnel: w1724 -> [w1737]
          tunnel: [w1736] -> w1718
          tunnel: w1717 -> [w1736]
          tunnel: [w1735] -> w1710
          tunnel: w1709 -> [w1735]
          tunnel: [w1741] -> w1726
          tunnel: w1725 -> [w1741]
          tunnel: [w1740] -> w1719
          tunnel: w1718 -> [w1740]
          tunnel: [w1739] -> w1711
          tunnel: w1710 -> [w1739]
          tunnel: [w1747] -> w1727
          tunnel: w1726 -> [w1747]
          tunnel: [w1746] -> w1720
          tunnel: w1719 -> [w1746]
          tunnel: [w1745] -> w1712
          tunnel: w1711 -> [w1745]
          tunnel: [w1751] -> w1728
          tunnel: w1727 -> [w1751]
          tunnel: [w1750] -> w1721
          tunnel: w1720 -> [w1750]
          tunnel: [w1749] -> w1713
          tunnel: w1712 -> [w1749]
          tunnel: [w1755] -> w1729
          tunnel: w1728 -> [w1755]
          tunnel: [w1754] -> w1722
          tunnel: w1721 -> [w1754]
          tunnel: [w1753] -> w1714
          tunnel: w1713 -> [w1753]
          tunnel: [w1759] -> w1730
          tunnel: w1729 -> [w1759]
          tunnel: [w1758] -> w1723
          tunnel: w1722 -> [w1758]
          tunnel: [w1757] -> w1715
          tunnel: w1714 -> [w1757]
          tunnel: w1730 -> [w1765]
          tunnel: w1723 -> [w1764]
          tunnel: [w1762] -> w1716
          tunnel: w1715 -> [w1762]
          tunnel: w1716 -> [w1766]
          frame #0 {
            n1114 = local read "Green Laser ON/Interlacing"() -> (w1734:bool)
            n1115 = local read "Green laser mode"() -> (w1733:enum32{"Laser ON", "Laser OFF", "Interlace"})
            n1116 = local read "Green FB On/Off"() -> (w1732:bool)
          }
          frame #1 {
            n1117 = property on="Green FB On/Off" class="Bool (strict)"("Val(Sgnl)"=FALSE ("Value (Signaling)")) -> ()  [unwired: 2 in, 2 out]
          }
          frame #2 {
            n1118 = property on="Green Laser ON/Interlacing" class="Bool (strict)"("Val(Sgnl)"=TRUE ("Value (Signaling)")) -> ()  [unwired: 2 in, 2 out]
            n1119 = property on="Flip Green Filter" class="Bool (strict)"("Val(Sgnl)"=TRUE ("Value (Signaling)")) -> ()  [unwired: 2 in, 2 out]
            n1120 = property on="Green laser mode" class="RadioBtnsControl (strict)"("Val(Sgnl)"=enum32{"Laser ON", "Laser OFF", "Interlace"}."Laser ON" ("Value (Signaling)")) -> ()  [unwired: 2 in, 2 out]
          }
          frame #3 {
            n1121 = Wait (ms)(milliseconds to wait=u32 500) -> ()  [unwired: 1 out]
          }
          frame #4 {
            n1122 = property on="Confocal Image" class="Bool (strict)"("Val(Sgnl)"=TRUE ("Value (Signaling)")) -> ()  [unwired: 2 in, 2 out]
          }
          frame #5 {
            n1123 = Wait (ms)(milliseconds to wait=u32 2000) -> ()  [unwired: 1 out]
          }
          frame #6 {
            n1124 = while {
              stop <- w1760 stop-if-true
              n1125 = local read "Saving..."() -> (w1761:bool)
              n1126 = Not(x=w1761) -> (.not. x?=w1760:bool)
            }
          }
          frame #7 {
            n1127 = property on="Flip Green Filter" class="Bool (strict)"("Val(Sgnl)"=TRUE ("Value (Signaling)")) -> ()  [unwired: 2 in, 2 out]
            n1128 = property on="Green Laser ON/Interlacing" class="Bool (strict)"("Val(Sgnl)"=w1765) -> ()  [unwired: 2 in, 2 out]
            n1129 = property on="Green laser mode" class="RadioBtnsControl (strict)"("Val(Sgnl)"=w1764) -> ()  [unwired: 2 in, 2 out]
          }
          frame #8 {
            n1130 = property on="Green FB On/Off" class="Bool (strict)"("Val(Sgnl)"=w1766) -> ()  [unwired: 2 in, 2 out]
          }
        }
      }
      event "Stop All": Value Change {
        n1131 = event-data() -> ()  [unwired: 1 in, 5 out]
        n1132 = local read "Stop All"() -> (w1767:bool)
      }
    }
    n1133 = node-c288() -> ()  [unwired: 1 in, 1 out]
  }
  n1134 = node-c288() -> (w76:T24)  [unwired: 4 out]
  n1135 = timed-loop "Mouse control: trap position (AOM deflection), set confocal spot from image" {
    tunnel: [w1769] -> w34
    tunnel: w24 -> [w1768]
    timing: w76 -> [_]
    timing-out: [_] -> w75
    stop <- w1769 stop-if-true
    n1136 = node-c288() -> ()  [unwired: 2 out]
    n1137 = event shown="[0] \"Pane\": Mouse Down" {
      selector: _ -> [_ _]
      dyn-events: _ -> [_ _]
      timeout: _ -> [_ _]
      tunnel: w1768 -> [w1772 _]
      event Mouse Down {
        n1138 = event-data() -> ("Time"=w1774:u32, "Coords"=w1773:T8, "Button"=w1775:u16)  [unwired: 6 out]
        n1139 = case shown="1" w1775 {
          tunnel: w1774 -> [_ _ w1878]
          tunnel: w1773 -> [_ w1812 w1876]
          tunnel: w1772 -> [_ _ w1874]
          frame 0, Default {
          }
          frame 1 {
            n1140 = property on="APD 2" class="ImageControl"() -> ("Displayed Image Position"=w1782:cluster{"Left":i32, "Top":i32})  [unwired: 2 in, 2 out]
            n1141 = property on="APD 1" class="ImageControl"() -> ("Displayed Image Position"=w1811:cluster{"Left":i32, "Top":i32})  [unwired: 2 in, 2 out]
            n1142 = property on="Detection Laser X" class="ImageControl"() -> ("Displayed Image Position"=w1808:cluster{"Left":i32, "Top":i32})  [unwired: 2 in, 2 out]
            n1143 = property on="Detection Laser Y" class="ImageControl"() -> ("Displayed Image Position"=w1807:cluster{"Left":i32, "Top":i32})  [unwired: 2 in, 2 out]
            n1144 = property on="APD 2" class="ImageControl"() -> ("Displayed Image Size"=w1781:cluster{"Width":u32, "Height":u32})  [unwired: 2 in, 2 out]
            n1145 = property on="APD 1" class="ImageControl"() -> ("Displayed Image Size"=w1809:cluster{"Width":u32, "Height":u32})  [unwired: 2 in, 2 out]
            n1146 = property on="Detection Laser X" class="ImageControl"() -> ("Displayed Image Size"=w1810:cluster{"Width":u32, "Height":u32})  [unwired: 2 in, 2 out]
            n1147 = property on="Detection Laser Y" class="ImageControl"() -> ("Displayed Image Size"=w1806:cluster{"Width":u32, "Height":u32})  [unwired: 2 in, 2 out]
            n1148 = Unbundle By Name(w1781) -> ("Width"=w1778:u32, "Height"=w1777:u32)
            n1149 = Unbundle By Name(w1782) -> ("Left"=w1780:i32, "Top"=w1779:i32)
            n1150 = Unbundle By Name(w1809) -> ("Width"=w1803:u32, "Height"=w1802:u32)
            n1151 = Unbundle By Name(w1810) -> ("Width"=w1799:u32, "Height"=w1798:u32)
            n1152 = Unbundle By Name(w1806) -> ("Width"=w1795:u32, "Height"=w1794:u32)
            n1153 = Unbundle By Name(w1811) -> ("Left"=w1805:i32, "Top"=w1804:i32)
            n1154 = Unbundle By Name(w1808) -> ("Left"=w1801:i32, "Top"=w1800:i32)
            n1155 = Unbundle By Name(w1807) -> ("Left"=w1797:i32, "Top"=w1796:i32)
            n1156 = Bundle("Left"=w1780, "Top"=w1779, "Width"=w1778, "Height"=w1777) -> (w1776:T33)  [unwired: 1 in]
            n1157 = Bundle("Left"=w1805, "Top"=w1804, "Width"=w1803, "Height"=w1802) -> (w1793:T33)  [unwired: 1 in]
            n1158 = Bundle("Left"=w1801, "Top"=w1800, "Width"=w1799, "Height"=w1798) -> (w1792:T33)  [unwired: 1 in]
            n1159 = Bundle("Left"=w1797, "Top"=w1796, "Width"=w1795, "Height"=w1794) -> (w1791:T33)  [unwired: 1 in]
            n1160 = Build Cluster Array(w1776, w1793, w1792, w1791) -> (w1790:T34)
            n1161 = for {
              tunnel: w1812 -> [w1823]
              tunnel: w1790 -> [w1824] mode=indexing
              shift-right: [w1821] -> w1788
              shift-left: TRUE -> [w1822]
              shift-right: [w1820] -> w1786
              shift-left: _ -> [w1816]
              shift-right: [w1819] -> w1785
              shift-left: _ -> [w1815]
              shift-right: [w1818] -> w1784
              shift-left: _ -> [w1814]
              shift-right: [w1817] -> w1783
              shift-left: _ -> [w1813]
              n1162 = case shown="True" w1822 {
                selector: w1822 -> [w1829 _]
                tunnel: w1824 -> [_ w1838]
                tunnel: w1823 -> [_ w1836]
                tunnel: [w1829 w1834] -> w1821
                tunnel: [w1828 w1833] -> w1820
                tunnel: [w1827 w1832] -> w1819
                tunnel: [w1826 w1831] -> w1818
                tunnel: [w1825 w1830] -> w1817
                tunnel: w1816 -> [w1828 _]
                tunnel: w1815 -> [w1827 _]
                tunnel: w1814 -> [w1826 _]
                tunnel: w1813 -> [w1825 _]
                frame False {
                }
                frame True {
                  n1163 = Unbundle(w1838) -> (w1837:T33)
                  n1164 = call "isclickinwindow.vi"("Image Param"=w1837, "Point32"=w1836) -> ("4 Y"=w1830:i32, "3 Height"=w1831:i32, "2 X"=w1832:i32, "1 Width"=w1833:i32, "In image?"=w1835:bool)  [unwired: 1 in]
                  n1165 = Not(x=w1835) -> (.not. x?=w1834:bool)
                }
              }
            }
            n1166 = Not(x=w1788) -> (.not. x?=w1787:bool)
            n1167 = case shown="True" w1787 {
              tunnel: w1785 -> [_ w1851]
              tunnel: w1783 -> [_ w1850]
              tunnel: w1786 -> [_ w1849]
              tunnel: w1784 -> [_ w1848]
              frame False {
              }
              frame True {
                w1844 = FALSE ("Get Point")
                n1168 = local read "Scan lines (y)"() -> (w1853:u64)
                n1169 = local read "Actual MCL Inc (V)"() -> (w1845:dbl)
                n1170 = local read "Scan steps (MCL)"() -> (w1852:u64)
                n1171 = Divide "Y Pix/step"(x=w1848, y=w1853) -> (x/y=w1860:dbl)
                n1172 = Divide "Y V/pix"(x=w1845, y=w1860) -> (x/y=w1859:dbl)
                n1173 = Divide "Y half step offset"(x=w1845, y=2.0) -> (x/y=w1861:dbl)
                n1174 = Divide "X pix/step"(x=w1849, y=w1852) -> (x/y=w1858:dbl)
                n1175 = Negate(x=w1861) -> (-x=w1862:dbl)
                n1176 = local read "Initial Y"() -> (w1868:dbl)
                n1177 = Multiply(x=w1850, y=w1859) -> (x*y=w1869:dbl)
                n1178 = Divide "X half step offset"(x=w1845, y=2.0) -> (x/y=w1855:dbl)
                n1179 = Divide "X V/pix"(x=w1845, y=w1858) -> (x/y=w1857:dbl)
                n1180 = Multiply(x=w1845, y=w1852) -> (x*y=w1864:dbl)
                n1181 = Compound Arithmetic op=ADD(w1862, w1869, w1868) -> (w1846:dbl)
                "Pointer Y (V)" <- w1846
                n1182 = Multiply(x=w1857, y=w1851) -> (x*y=w1866:dbl)
                n1183 = Negate(x=w1855) -> (-x=w1854:dbl)
                n1184 = local read "Initial X"() -> (w1867:dbl)
                n1185 = Negate(x=w1866) -> (-x=w1865:dbl)
                n1186 = Compound Arithmetic op=ADD(w1854, w1864, w1867, w1865) -> (w1847:dbl)
                "Pointer X (V)" <- w1847
                n1187 = Or(x="Set X Only", y="Set Confocal Spot (X-Y)") -> (x .or. y?=w1840:bool)
                n1188 = Or(x="Set Confocal Spot (X-Y)", y="Set Y Only") -> (x .or. y?=w1839:bool)
                n1189 = case shown="True" w1840 {
                  tunnel: w1847 -> [_ w1870]
                  frame False {
                  }
                  frame True {
                    n1190 = property on="AO2" class="Slide (strict)"("Val(Sgnl)"=w1870) -> ()  [unwired: 2 in, 2 out]
                  }
                }
                n1191 = case shown="True" w1839 {
                  tunnel: w1846 -> [_ w1871]
                  frame False {
                  }
                  frame True {
                    n1192 = property on="AO1" class="Slide (strict)"("Val(Sgnl)"=w1871) -> ()  [unwired: 2 in, 2 out]
                  }
                }
                n1193 = local write "Set Confocal Spot (X-Y)"(w1844) -> ()
                n1194 = local write "Set X Only"(w1844) -> ()
                n1195 = local write "Set Y Only"(w1844) -> ()
              }
            }
          }
          frame 3 {
            n1196 = local read "BD 2 Frequency 1 (MHz)"() -> (w1872:dbl)
            n1197 = local read "BD 1 Frequency 1 (MHz)"() -> (w1873:dbl)
            n1198 = local write "Manipulating Trap"(TRUE ("Manipulating Trap")) -> ()
            n1199 = local write "Coords"(T8 {"Horizontal"=0, "Vertical"=0} ("Coords")) -> ()
            n1200 = while {
              tunnel: w1878 -> [w1883]
              tunnel: w1876 -> [w1882]
              tunnel: w1874 -> [w1881]
              tunnel: w1873 -> [w1880]
              tunnel: w1872 -> [w1879]
              stop <- w1884 stop-if-true
              n1201 = event shown="[0] \"Pane\": Mouse Move" {
                selector: _ -> [_ _]
                dyn-events: _ -> [_ _]
                timeout: _ -> [_ _]
                tunnel: ["Force Manip Abort" w1948] -> w1884
                tunnel: w1883 -> [w1891 _]
                tunnel: w1882 -> [w1889 _]
                tunnel: w1881 -> [w1888 _]
                tunnel: w1880 -> [w1887 _]
                tunnel: w1879 -> [w1886 _]
                event Mouse Move {
                  n1202 = event-data() -> ("Time"=w1892:u32, "Coords"=w1893:T8)  [unwired: 3 out]
                  n1203 = Less?(x=w1892, y=w1891) -> (x < y?=w1890:bool)
                  n1204 = case "Makes sure old motion events prior to mouse click aren't used" shown="False" w1890 {
                    tunnel: w1893 -> [w1935 _]
                    tunnel: w1889 -> [w1936 _]
                    tunnel: w1888 -> [w1913 _]
                    tunnel: w1887 -> [w1909 _]
                    tunnel: w1886 -> [w1908 _]
                    frame False {
                      n1205 = Subtract(x=w1935, y=w1936) -> (x-y=w1934:T8)
                      "Coords" <- w1934
                      n1206 = local read "Y RF Frequency Limits (MHz)"() -> (w1894:T16)
                      n1207 = To Double Precision Float(number=w1934) -> (double precision float=w1933:cluster{"Horizontal":dbl, "Vertical":dbl})
                      n1208 = Multiply(x=cluster{"Horizontal":dbl, "Vertical":dbl} {"Horizontal"=-1.0, "Vertical"=1.0}, y="Manipulation Scaling") -> (x*y=w1929:cluster{"Horizontal":dbl, "Vertical":dbl})
                      n1209 = local read "X RF Frequency Limits (MHz)"() -> (w1895:T16)
                      n1210 = Multiply(x=w1933, y=w1929) -> (x*y=w1931:cluster{"Horizontal":dbl, "Vertical":dbl})
                      n1211 = Unbundle By Name(w1931) -> ("Horizontal"=w1926:dbl, "Vertical"=w1930:dbl)
                      n1212 = Unbundle By Name(w1894) -> ("Maximum"=w1897:dbl, "Minimum"=w1896:dbl)
                      n1213 = Boolean To (0,1)(Boolean="Manip. X?") -> (0, 1=w1924:i16)
                      n1214 = Boolean To (0,1)(Boolean="Manip. Y?") -> (0, 1=w1921:i16)
                      n1215 = local read "BD 1 Frequency 2 (MHz)"() -> (w1911:dbl)
                      n1216 = Multiply(x=w1930, y=w1921) -> (x*y=w1923:dbl)
                      n1217 = Multiply(x=w1924, y=w1926) -> (x*y=w1927:dbl)
                      n1218 = local read "BD 2 Frequency 2 (MHz)"() -> (w1910:dbl)
                      n1219 = Unbundle By Name(w1895) -> ("Maximum"=w1899:dbl, "Minimum"=w1898:dbl)
                      n1220 = Add(x=w1908, y=w1923) -> (x+y=w1901:dbl)
                      n1221 = Add(x=w1909, y=w1927) -> (x+y=w1903:dbl)
                      n1222 = In Range and Coerce(upper limit=w1899, x=w1903, lower limit=w1898) -> (coerced(x)=w1902:dbl)  [unwired: 1 out]
                      n1223 = In Range and Coerce(upper limit=w1897, x=w1901, lower limit=w1896) -> (coerced(x)=w1900:dbl)  [unwired: 1 out]
                      n1224 = Subtract(x=w1902, y=w1911) -> (x-y=w1920:dbl)
                      n1225 = Subtract(x=w1900, y=w1910) -> (x-y=w1919:dbl)
                      n1226 = Square(x=w1920) -> (x^2=w1918:dbl)
                      n1227 = Square(x=w1919) -> (x^2=w1917:dbl)
                      n1228 = Add(x=w1918, y=w1917) -> (x+y=w1916:dbl)
                      n1229 = Square Root(x=w1916) -> (sqrt(x)=w1912:dbl)
                      n1230 = In Range and Coerce(upper limit="Limit Max (MHz)", x=w1912, lower limit="Limit Min (MHz)") -> (In Range?=w1905:bool)  [unwired: 1 out]
                      n1231 = Not(x="Limits Enable") -> (.not. x?=w1904:bool)
                      n1232 = Or(x=w1905, y=w1904) -> (x .or. y?=w1906:bool)
                      n1233 = case shown="True" w1906 {
                        tunnel: w1913 -> [_ w1946]
                        tunnel: w1912 -> [_ w1937]
                        tunnel: w1902 -> [_ w1944]
                        tunnel: w1911 -> [_ w1943]
                        tunnel: w1900 -> [_ w1942]
                        tunnel: w1910 -> [_ w1941]
                        tunnel: w1895 -> [_ w1939]
                        tunnel: w1894 -> [_ w1938]
                        frame False {
                        }
                        frame True {
                          n1234 = local read "BD 1 Frequency 3 (MHz)"() -> (w1945:dbl)
                          n1235 = local read "BD 2 Frequency 3 (MHz)"() -> (w1940:dbl)
                          n1236 = local write "Trap Delta (MHz)"(w1937) -> ()
                          n1237 = property on="Initial delta (MHz)" class="DigNum (strict)"("Val(Sgnl)"=w1937) -> ()  [unwired: 2 in, 2 out]
                          n1238 = call "set RF board frequency - interlace.vi"("Board 2 Frequency Limits"=w1938, "Board 1 Frequency Limits"=w1939, "FPGA VI Reference In"=w1946, "Board 2 Frequency 3 (MHz)"=w1940, "Board 1 Frequency 3 (MHz)"=w1945, "Board 2 Frequency 2 (MHz)"=w1941, "Board 2 Frequency 1 (MHz)"=w1942, "Board 1 Frequency 2 (MHz)"=w1943, "Board 1 Frequency 1  (MHz)"=w1944) -> ()  [unwired: 1 in, 2 out]
                          n1239 = local write "BD 2 Frequency 1 (MHz)"(w1942) -> ()
                          n1240 = local write "BD 1 Frequency 1 (MHz)"(w1944) -> ()
                        }
                      }
                    }
                    frame True {
                    }
                  }
                }
                event Mouse Up {
                  n1241 = event-data() -> ("Button"=w1947:u16)  [unwired: 8 out]
                  n1242 = case shown="3" w1947 {
                    tunnel: [FALSE TRUE] -> w1948
                    frame 0, Default {
                    }
                    frame 3 {
                      n1243 = local write "Manipulating Trap"(FALSE ("Manipulating Trap")) -> ()
                    }
                  }
                }
              }
            }
          }
        }
      }
      event Mouse Move {
        n1244 = event-data() -> ()  [unwired: 6 out]
      }
    }
    n1245 = local read "Stop All"() -> (w1769:bool)
    n1246 = node-c288() -> ()  [unwired: 2 out]
  }
  n1247 = node-c288(w14) -> ()  [unwired: 1 out]
  n1248 = node-c288(w68) -> ()  [unwired: 1 out]
  n1249 = node-c288(w75) -> ()  [unwired: 1 out]
  n1250 = node-c288(i64 1 ("Period"), 1 ("Processor")) -> (w164:T24)  [unwired: 2 out]
  n1251 = timed-loop "Acquire Data" {
    tunnel: w24 -> [w2206]
    tunnel: w40 -> [w2205]
    tunnel: [w2236] -> w33
    tunnel: [w2230] -> w32
    timing: w164 -> [_]
    timing-out: [_] -> w163
    tunnel: w59 -> [w2034]
    stop <- "Stop All" stop-if-true
    (unwired) u32 0 ("Number of Elements")
    w2021 = "NI_ChannelName" ("name")
    n1252 = node-c288() -> ()  [unwired: 2 out]
    n1253 = First Call?() -> (First Call?: T/F=w1987:bool)
    n1254 = Or(x="Reset", y=w1987) -> (x .or. y?=w1988:bool)
    n1255 = case "Reset data stream" shown="True" w1988 {
      tunnel: w2206 -> [w2252 w2260]
      tunnel: w2205 -> [w2251 w2259]
      tunnel: [w2252 w2254] -> w2201
      tunnel: [w2251 w2253] -> w2200
      frame False {
      }
      frame True {
        w2257 = TRUE ("AI to FIFO")
        n1256 = local write "Overflow (data lost)"(FALSE ("Overflow (data lost)")) -> ()
        n1257 = call "reset FPGA DMA.vi"("error in"=w2259, "FPGA VI Reference In"=w2260) -> ("error out"=w2255:errorcluster, "FPGA VI Reference Out"=w2256:T19)
        n1258 = xnode "Read/Write Control"("FPGA VI Reference In"=w2256, "error in"=w2255, "AI to FIFO"=w2257, "APD to FIFO"=w2257) -> ("FPGA VI Reference Out"=w2254:T19, "error out"=w2253:errorcluster)
      }
    }
    n1259 = Or(x="Start AOD Scan", y="Trap Raster Scan") -> (x .or. y?=w2151:bool)
    n1260 = case "Start AOM raster scan" shown="True" w2151 {
      tunnel: w2201 -> [w2989 w2999]
      tunnel: w2200 -> [w2988 w2998]
      tunnel: [w2989 w2992] -> w2199
      tunnel: [w2988 w2991] -> w2198
      frame False {
      }
      frame True {
        n1261 = case shown="True" "Restart DMA? (AOD)" {
          tunnel: [w3037 w3039] -> w2993
          tunnel: [w3036 w3038] -> w2994
          tunnel: w2999 -> [w3037 w3041]
          tunnel: w2998 -> [w3036 w3040]
          frame False {
          }
          frame True {
            n1262 = local write "Overflow (data lost)"(FALSE ("Overflow (data lost)")) -> ()
            n1263 = call "reset FPGA DMA.vi"("error in"=w3040, "FPGA VI Reference In"=w3041) -> ("error out"=w3038:errorcluster, "FPGA VI Reference Out"=w3039:T19)
          }
        }
        n1264 = local write "Trap Raster Scan"(FALSE ("Trap Raster Scan")) -> ()
        n1265 = case shown="False" "Move MCL Also?" {
          tunnel: w2994 -> [w3002 w3031]
          tunnel: w2993 -> [w3003 w3032]
          tunnel: [w3001 w3035] -> w2992
          tunnel: [w3000 w3034] -> w2991
          frame False {
            w3004 = TRUE ("AI to FIFO")
            n1266 = xnode "Read/Write Control"("FPGA VI Reference In"=w3003, "error in"=w3002, "AI to FIFO"=w3004, "APD to FIFO"=w3004, "Start scan"=w3004) -> ("FPGA VI Reference Out"=w3001:T19, "error out"=w3000:errorcluster)
          }
          frame True {
            w3028 = FALSE ("1D or 2D Scan?")
            w3033 = TRUE ("AI to FIFO")
            # "Count for MCL loop"
            # "N total cycles"
            # "N steps"
            # "V_int"
            n1267 = local read "Scan Range (nm)"() -> (w3010:dbl)
            n1268 = local read "Number of F/B Scans (AOD)"() -> (w3027:u16)
            n1269 = Sign(1:w3010) -> (0:w3009:dbl)
            n1270 = Compound Arithmetic op=MULTIPLY(w3010, "MCL Step Position Ratio", "MCL/AOM Scale Tweak") -> (w3014:dbl)
            n1271 = Negate(x=w3009) -> (-x=w3006:dbl)
            n1272 = Multiply(x=w3006, y="MCL Step Increment (V_int)") -> (x*y=w3008:dbl)
            n1273 = Divide(x=w3014, y="MCL X Cal (nm/V)") -> (x/y=w3020:dbl)
            n1274 = Multiply(x=32767.0 ("y"), y=w3020) -> (x*y=w3026:dbl)
            n1275 = local read "Total Counts (ticks)"() -> (w3011:u32)
            n1276 = local read "Cycles/step (AOD)"() -> (w3022:u64)
            n1277 = local read "Scan steps (AOD)"() -> (w3023:u64)
            n1278 = Divide(x=w3026, y=10.0) -> (x/y=w3019:dbl)
            n1279 = Divide(x=w3019, y="MCL Step Increment (V_int)") -> (x/y=w3017:dbl)
            n1280 = Absolute Value(x=w3017) -> (abs(x)=w3005:dbl)
            n1281 = Compound Arithmetic op=MULTIPLY(w3023, w3022, w3011) -> (w3018:u64)
            n1282 = local write "wait to reset values"(w3033) -> ()
            n1283 = local write "MCL Scanning"(w3033) -> ()
            n1284 = Divide(x=w3018, y=w3005) -> (x/y=w3015:dbl)
            "MCL Count" <- w3015
            n1285 = xnode "Read/Write Control"("FPGA VI Reference In"=w3032, "error in"=w3031, "Scan steps (MCL)"=w3005, "Number of scans (MCL)"=w3027, "Cycles per step (MCL)"=u64 1, "Scan freq.  increment (MCL)"=w3008, "1D or 2D Scan?"=w3028, "MCL Scan Axis"=w3028, "Cont. Scan (MCL)"=w3028, "MCL count"=w3015) -> ("FPGA VI Reference Out"=w3030:T19, "error out"=w3029:errorcluster)
            n1286 = xnode "Read/Write Control"("FPGA VI Reference In"=w3030, "error in"=w3029, "AI to FIFO"=w3033, "APD to FIFO"=w3033, "Start scan"=w3033, "Start scan (MCL)"=w3033) -> ("FPGA VI Reference Out"=w3035:T19, "error out"=w3034:errorcluster)
          }
        }
        "Raster Scanning..." <- TRUE ("Scanning...")
      }
    }
    n1287 = And(x="Save scans", y=w2151) -> (x .and. y?=w2197:bool)
    n1288 = Compound Arithmetic op=OR("Start MCL Scan", "Confocal Image", "Confocal Linescan") -> (w2149:bool)
    n1289 = And(x="Save Data (MCL)", y=w2149) -> (x .and. y?=w2196:bool)
    n1290 = case "Start MCL raster scan" shown="True" w2149 {
      tunnel: w2199 -> [w2543 w2558]
      tunnel: w2198 -> [w2542 w2557]
      tunnel: [w2543 w2553] -> w1956
      tunnel: [w2542 w2552] -> w1955
      tunnel: [FALSE w2551] -> w2182
      tunnel: "Start MCL Scan" -> [_ w2546]
      tunnel: "Confocal Image" -> [_ w2545]
      tunnel: "Confocal Linescan" -> [_ _]
      frame False {
      }
      frame True {
        w2551 = TRUE
        n1291 = case shown="True" "Restart DMA? (MCL)" {
          tunnel: [w2603 w2605] -> w2556
          tunnel: [w2602 w2604] -> w2555
          tunnel: w2558 -> [w2603 w2608]
          tunnel: w2557 -> [w2602 w2607]
          frame False {
          }
          frame True {
            n1292 = call "reset FPGA DMA.vi"("error in"=w2607, "FPGA VI Reference In"=w2608) -> ("error out"=w2604:errorcluster, "FPGA VI Reference Out"=w2605:T19)
            n1293 = local write "Overflow (data lost)"(FALSE ("Overflow (data lost)")) -> ()
          }
        }
        n1294 = case shown="False" w2546 {
          selector: w2546 -> [_ w2562]
          tunnel: w2545 -> [w2561 _]
          tunnel: [w2561 w2562] -> w2544
          frame False {
            n1295 = property on="2D or 1D Scan" class="Bool (strict)"("Val(Sgnl)"=w2561) -> ()  [unwired: 2 in, 2 out]
            n1296 = property on="Confocal Image" class="Bool (strict)"("Value"=FALSE ("Start Confocal Map")) -> ()  [unwired: 2 in, 2 out]
          }
          frame True {
          }
        }
        n1297 = local write "MCL Scanning"(w2551) -> ()
        n1298 = local read "AO1"() -> (w2548:dbl)
        n1299 = local read "AO2"() -> (w2547:dbl)
        n1300 = case shown="True" "Center Scan" {
          tunnel: w2556 -> [w2569 w2601]
          tunnel: w2555 -> [w2568 w2600]
          tunnel: [w2567 w2599] -> w2553
          tunnel: [w2566 w2598] -> w2552
          tunnel: [w2564 w2585] -> w2550
          tunnel: [w2563 w2584] -> w2549
          tunnel: w2548 -> [w2564 w2590]
          tunnel: w2547 -> [w2563 w2593]
          tunnel: w2544 -> [_ _]
          frame False {
            w2565 = TRUE ("AI to FIFO")
            n1301 = xnode "Read/Write Control"("FPGA VI Reference In"=w2569, "error in"=w2568, "AI to FIFO"=w2565, "APD to FIFO"=w2565, "Start scan (MCL)"=w2565) -> ("FPGA VI Reference Out"=w2567:T19, "error out"=w2566:errorcluster)
          }
          frame True {
            w2597 = TRUE ("AI to FIFO")
            n1302 = local read "Scan steps (MCL)"() -> (w2576:u64)
            n1303 = local read "Scan lines (y)"() -> (w2572:u64)
            n1304 = local read "Fast Scan Dir"() -> (w2583:bool)
            n1305 = local read "Actual MCL Inc (V)"() -> (w2573:dbl)
            n1306 = Decrement(x=w2572) -> (x-1=w2571:u64)
            n1307 = Decrement(x=w2576) -> (x-1=w2575:u64)
            n1308 = Multiply(x=w2573, y=w2571) -> (x*y=w2570:dbl)
            n1309 = Divide(x=w2570, y=2.0) -> (x/y=w2580:dbl)
            n1310 = Multiply(x=w2573, y=w2575) -> (x*y=w2574:dbl)
            n1311 = Divide(x=w2574, y=2.0) -> (x/y=w2579:dbl)
            n1312 = Select(t=w2579, s=w2583, f=w2580) -> (s? t:f=w2578:dbl)
            n1313 = Select(t=w2580, s=w2583, f=w2579) -> (s? t:f=w2582:dbl)
            n1314 = Subtract(x=w2590, y=w2582) -> (x-y=w2581:dbl)
            n1315 = Subtract(x=w2593, y=w2578) -> (x-y=w2577:dbl)
            n1316 = local read "2D or 1D Scan"() -> (w2595:bool)
            n1317 = Not(x=w2583) -> (.not. x?=w2589:bool)
            n1318 = Not(x=w2595) -> (.not. x?=w2591:bool)
            n1319 = And(x=w2583, y=w2591) -> (x .and. y?=w2592:bool)
            n1320 = And(x=w2591, y=w2589) -> (x .and. y?=w2594:bool)
            n1321 = Select(t=w2593, s=w2594, f=w2577) -> (s? t:f=w2584:dbl)
            n1322 = Select(t=w2590, s=w2592, f=w2581) -> (s? t:f=w2585:dbl)
            n1323 = call "Volt to I16.vi"("Voltage In"=w2585) -> ("I16 Voltage Out"=w2588:i16)
            n1324 = call "Volt to I16.vi"("Voltage In"=w2584) -> ("I16 Voltage Out"=w2587:i16)
            n1325 = xnode "Read/Write Control"("FPGA VI Reference In"=w2601, "error in"=w2600, "AI to FIFO"=w2597, "APD to FIFO"=w2597, "Start scan (MCL)"=w2597, "AO1"=w2588, "AO2"=w2587) -> ("FPGA VI Reference Out"=w2599:T19, "error out"=w2598:errorcluster)
          }
        }
        "Initial Y" <- w2550
        "Initial X" <- w2549
        "wait to reset values" <- w2551
      }
    }
    n1326 = local read "Trap Pos Elements/DMA read"() -> (w2030:u32)
    n1327 = local read "Trap AI Elements/DMA read"() -> (w1954:u32)
    n1328 = local read "APD Elements/DMA read"() -> (w2073:u32)
    n1329 = local read "Trap AI FIFO Depth"() -> (w2246:u32)
    n1330 = xnode "Invoke Method"("FPGA VI Reference In"=w1956, "error in"=w1955, "Number of Elements"=w2030, "Timeout (ms)"=-1) -> ("Data"=w1994:u16[], "Elements Remaining"=→"Trap Pos FIFO El Remaining":u32)  [unwired: 2 out]
    n1331 = xnode "Invoke Method"("FPGA VI Reference In"=w1956, "error in"=w1955, "Number of Elements"=w1954, "Timeout (ms)"=-1 ("Timeout")) -> ("FPGA VI Reference Out"=w1958:T19, "error out"=w1957:errorcluster, "Data"=w1953:i16[], "Elements Remaining"=w1959:u32)
    "Trap AI FIFO El. Rem." <- w1959
    n1332 = xnode "Get APD Data"("FPGA VI Reference In"=w1956, "error in"=w1955, "Number of Elements"=w2073, "Timeout (ms)"=-1) -> ("Data"=w2072:u32[], "Elements Remaining"=→"APD FIFO Elements Remaining":u32)  [unwired: 2 out]
    n1333 = Subtract(x=w2246, y=w1954) -> (x-y=w2245:u32)
    n1334 = Decimate 1D Array(w1994) -> (w1991:u16[], w1993:u16[], w1992:u16[])
    n1335 = Divide(x=w1959, y=w2245) -> (x/y=w2244:dbl)
    "Buffer Status" <- w2244
    n1336 = To Unsigned Long Integer(number=w1991) -> (unsigned 32bit integer=w1990:u32[])
    n1337 = Join Numbers(hi=w1993, lo=w1992) -> ((hi.lo)=w1989:u32[])
    n1338 = Equal?(x=w2244, y=1.0) -> (x = y?=w2242:bool)
    n1339 = Join Numbers(hi=w1990, lo=w1989) -> ((hi.lo)=w1983:u64[])
    n1340 = call "IR AOM word to freq - vec.vi"("Frequency Word In (double vec)"=w1983) -> ("Frequency Out"=w2029:dbl[])
    n1341 = case "Alert buffer overflow" shown="False" w2242 {
      frame False {
      }
      frame True {
        n1342 = call <vilib>:"Beep.vi"() -> ()  [unwired: 3 in, 9 out]
        "Overflow (data lost)" <- TRUE ("Overflow (data lost)")
      }
    }
    n1343 = Decimate 1D Array(w2029) -> (w2028:dbl[], w2027:dbl[])
    n1344 = Array Size(array=w1953) -> (size(s)=→"Waveform Chart":i32)
    n1345 = Build Array(w2028, w2027) -> (w2026:dbl[][])
    n1346 = local read "Trap Sets"() -> (w2110:u32)
    n1347 = case "Deinterlace trap data, average down PSD" shown="2" w2110 {
      tunnel: w1953 -> [w2638 w2703]
      tunnel: [w2635 w2700] -> w2103
      tunnel: [w2638 w2702] -> w1986
      tunnel: "Detector Type" -> [w2637 w2698]
      tunnel: [w2636 w2701] -> w2102
      tunnel: [w2634 w2699] -> w2217
      frame 1, Default {
        n1348 = Divide(x=w2638, y=3276.7) -> (x/y=w2639:dbl[])
        n1349 = Decimate 1D Array(w2639) -> (w2648:dbl[], w2647:dbl[], w2646:dbl[], w2645:dbl[], w2644:dbl[], w2643:dbl[], w2642:dbl[], w2641:dbl[])
        n1350 = case shown="\"IR-QPD + PSD + FB-QPD position\"" w2637 {
          tunnel: w2648 -> [w2672 w2697]
          tunnel: w2647 -> [w2671 w2696]
          tunnel: w2646 -> [w2656 w2674]
          tunnel: w2645 -> [w2657 w2684]
          tunnel: w2644 -> [w2670 w2695]
          tunnel: w2643 -> [w2669 w2694]
          tunnel: w2642 -> [w2653 w2675]
          tunnel: w2641 -> [w2652 w2673]
          tunnel: [w2651 w2681] -> w2636
          tunnel: [w2650 w2680] -> w2635
          tunnel: [w2649 w2679] -> w2634
          frame "IR-QPD + PSD + FB-QPD", Default {
            w2649 = 0  # Channel pattern
            n1351 = Divide(x=w2672, y=w2657) -> (x/y=w2659:dbl[])
            n1352 = Divide(x=w2671, y=w2657) -> (x/y=w2658:dbl[])
            n1353 = Divide(x=w2670, y=w2653) -> (x/y=w2655:dbl[])
            n1354 = Divide(x=w2669, y=w2652) -> (x/y=w2654:dbl[])
            n1355 = Build Array(w2659, w2658, w2657, w2656, w2655, w2654, w2653, w2652) -> (w2650:dbl[][])
            n1356 = Bundle("T1 Y", "T1 X", "T1 Sum", "FB Sum", "PSD Y", "PSD X", "PSD Y Sum", "PSD X Sum") -> (w2668:T41)  [unwired: 1 out]
            n1357 = Cluster To Array(cluster=w2668) -> (array=w2651:string[])
          }
          frame "IR-QPD + PSD + FB-QPD position" {
            w2679 = 3  # Channel pattern
            n1358 = Negate(x=w2675) -> (-x=w2676:dbl[])
            n1359 = Divide(x=w2697, y=w2684) -> (x/y=w2686:dbl[])
            n1360 = Divide(x=w2696, y=w2684) -> (x/y=w2685:dbl[])
            n1361 = Divide(x=w2695, y=w2675) -> (x/y=w2683:dbl[])
            n1362 = Divide(x=w2694, y=w2676) -> (x/y=w2682:dbl[])
            n1363 = Build Array(w2686, w2685, w2684, w2673, w2674, w2683, w2682, w2675) -> (w2680:dbl[][])
            n1364 = Bundle("T1 Y", "T1 X", "T1 Sum", "FB X", "FB Sum", "PSD Y", "PSD X", "PSD Y Sum") -> (w2693:T41)  [unwired: 1 out]
            n1365 = Cluster To Array(cluster=w2693) -> (array=w2681:string[])
          }
        }
      }
      frame 2 {
        n1366 = case shown="\"UCB Fleezers 052511\"" w2698 {
          tunnel: w2703 -> [w2765 w2832 w2860 w2967]
          tunnel: [w2704 w2824 w2855 w2898] -> w2702
          tunnel: [w2731 w2815 w2857 w2945] -> w2701
          tunnel: [w2730 w2779 w2834 w2912] -> w2700
          tunnel: [w2724 w2814 w2897 w2943] -> w2699
          frame "IR-QPD + PSD + FB-QPD", Default {
            w2724 = 1  # Channel pattern
            # "time average x2 the 4th signal and the 4 psd signals (detection laser)"
            # "deinterlace 3 signals from qpd"
            n1367 = Decimate 1D Array(w2765) -> (w2764:i16[], w2763:i16[], w2729:i16[], w2762:i16[], w2752:i16[], w2750:i16[], w2749:i16[], w2747:i16[])
            n1368 = call "downsample 1D array - double.vi"("Ave N"=2.0, "Array In"=w2752) -> ("Array Out"=w2751:dbl[])  [unwired: 1 out]
            n1369 = call "downsample 1D array - double.vi"("Ave N"=2.0, "Array In"=w2747) -> ("Array Out"=w2746:dbl[])  [unwired: 1 out]
            n1370 = call "downsample 1D array - double.vi"("Ave N"=2.0, "Array In"=w2749) -> ("Array Out"=w2748:dbl[])  [unwired: 1 out]
            n1371 = call "downsample 1D array - double.vi"("Ave N"=2.0, "Array In"=w2750) -> ("Array Out"=w2732:dbl[])  [unwired: 1 out]
            n1372 = Decimate 1D Array(w2764) -> (w2761:i16[], w2733:i16[])
            n1373 = Decimate 1D Array(w2763) -> (w2760:i16[], w2758:i16[])
            n1374 = Decimate 1D Array(w2762) -> (w2759:i16[], w2757:i16[])
            n1375 = Decimate 1D Array(w2729) -> (w2728:i16[], w2727:i16[])
            n1376 = Interleave 1D Arrays(w2761, w2760, w2759, w2733, w2758, w2757, w2728, w2727, w2751, w2732, w2748, w2746) -> (w2745:dbl[])
            n1377 = To Word Integer(number=w2745) -> (16bit integer=w2704:i16[])
            n1378 = Divide(x=w2745, y=3276.7) -> (x/y=w2744:dbl[])
            n1379 = Decimate 1D Array(w2744) -> (w2743:dbl[], w2742:dbl[], w2741:dbl[], w2740:dbl[], w2739:dbl[], w2738:dbl[], w2726:dbl[], w2725:dbl[], w2737:dbl[], w2736:dbl[], w2735:dbl[], w2734:dbl[])
            n1380 = Divide(x=w2743, y=w2741) -> (x/y=w2711:dbl[])
            n1381 = Divide(x=w2742, y=w2741) -> (x/y=w2710:dbl[])
            n1382 = Divide(x=w2740, y=w2738) -> (x/y=w2709:dbl[])
            n1383 = Divide(x=w2739, y=w2738) -> (x/y=w2708:dbl[])
            n1384 = Divide(x=w2737, y=w2735) -> (x/y=w2707:dbl[])
            n1385 = Divide(x=w2736, y=w2734) -> (x/y=w2706:dbl[])
            n1386 = Bundle("T1 Y", "T1 X", "T1 Sum", "T2 Y", "T2 X", "T2 Sum", "T1 FB Sum", "T2 FB Sum", "PSD Y", "PSD X", "PSD Y Sum", "PSD X Sum") -> (w2712:T42)  [unwired: 1 out]
            n1387 = Build Array(w2711, w2710, w2741, w2709, w2708, w2738, w2726, w2725, w2707, w2706, w2735, w2734) -> (w2730:dbl[][])
            n1388 = Cluster To Array(cluster=w2712) -> (array=w2731:string[])
          }
          frame "IR-QPD + PSD + FB-QPD X position" {
            w2814 = 2  # Channel pattern
            # "convert\nADC numbers\nto volts"
            # "time average x2 the 3 psd signals (detection laser)"
            # "deinterlace 3 signals from qpds"
            n1389 = Decimate 1D Array(w2832) -> (w2831:i16[], w2830:i16[], w2767:i16[], w2768:i16[], w2777:i16[], w2774:i16[], w2771:i16[], w2802:i16[])
            n1390 = Decimate 1D Array(w2831) -> (w2829:i16[], w2816:i16[])
            n1391 = call "downsample 1D array - I16.vi"("Ave N"=2.0, "Array In"=w2777) -> ("Array Out"=w2775:i16[])  [unwired: 1 in]
            n1392 = call "downsample 1D array - I16.vi"("Ave N"=2.0, "Array In"=w2774) -> ("Array Out"=w2772:i16[])  [unwired: 1 in]
            n1393 = Decimate 1D Array(w2830) -> (w2828:i16[], w2826:i16[])
            n1394 = Decimate 1D Array(w2768) -> (w2827:i16[], w2825:i16[])
            n1395 = Decimate 1D Array(w2802) -> (w2801:i16[], w2799:i16[])
            n1396 = Decimate 1D Array(w2767) -> (w2800:i16[], w2798:i16[])
            n1397 = call "downsample 1D array - I16.vi"("Ave N"=2.0, "Array In"=w2771) -> ("Array Out"=w2769:i16[])  [unwired: 1 in]
            n1398 = Interleave 1D Arrays(w2829, w2828, w2827, w2816, w2826, w2825, w2801, w2800, w2799, w2798, w2775, w2772, w2769) -> (w2824:i16[])
            n1399 = Divide(x=w2824, y=3276.7) -> (x/y=w2823:dbl[])
            n1400 = Decimate 1D Array(w2823) -> (w2822:dbl[], w2821:dbl[], w2820:dbl[], w2819:dbl[], w2818:dbl[], w2817:dbl[], w2790:dbl[], w2788:dbl[], w2787:dbl[], w2785:dbl[], w2784:dbl[], w2783:dbl[], w2780:dbl[])
            n1401 = Divide(x=w2822, y=w2820) -> (x/y=w2806:dbl[])
            n1402 = Divide(x=w2821, y=w2820) -> (x/y=w2805:dbl[])
            n1403 = Divide(x=w2819, y=w2817) -> (x/y=w2804:dbl[])
            n1404 = Divide(x=w2818, y=w2817) -> (x/y=w2803:dbl[])
            n1405 = Divide(x=w2790, y=w2788) -> (x/y=w2789:dbl[])
            n1406 = Divide(x=w2787, y=w2785) -> (x/y=w2786:dbl[])
            n1407 = Divide(x=w2784, y=w2780) -> (x/y=w2782:dbl[])
            n1408 = Negate(x=w2780) -> (-x=w2778:dbl[])
            n1409 = Divide(x=w2783, y=w2778) -> (x/y=w2781:dbl[])
            n1410 = Bundle("T1 Y", "T1 X", "T1 Sum", "T2 Y", "T2 X", "T2 Sum", "T1 FB X", "T1 FB Sum", "T2 FB X", "T2 FB Sum", "PSD Y", "PSD X", "PSD Y Sum") -> (w2807:T43)  [unwired: 1 out]
            n1411 = Build Array(w2806, w2805, w2820, w2804, w2803, w2817, w2789, w2788, w2786, w2785, w2782, w2781, w2780) -> (w2779:dbl[][])
            n1412 = Cluster To Array(cluster=w2807) -> (array=w2815:string[])
          }
          frame "UCB Fleezers 052511" {
            w2897 = 2  # Channel pattern
            n1413 = Decimate 1D Array(w2860) -> (w2895:i16[], w2894:i16[], w2859:i16[], w2858:i16[], w2852:i16[], w2849:i16[], w2848:i16[], w2847:i16[])
            n1414 = Decimate 1D Array(w2895) -> (w2893:i16[], w2878:i16[])
            n1415 = Decimate 1D Array(w2894) -> (w2892:i16[], w2890:i16[])
            n1416 = Decimate 1D Array(w2859) -> (w2891:i16[], w2889:i16[])
            n1417 = Decimate 1D Array(w2858) -> (w2854:i16[], w2853:i16[])
            n1418 = Decimate 1D Array(w2852) -> (w2851:i16[], w2850:i16[])
            n1419 = call "downsample 1D array - I16.vi"("Ave N"=2.0, "Array In"=w2849) -> ("Array Out"=w2846:i16[])  [unwired: 1 in]
            n1420 = call "downsample 1D array - I16.vi"("Ave N"=2.0, "Array In"=w2848) -> ("Array Out"=w2845:i16[])  [unwired: 1 in]
            n1421 = call "downsample 1D array - I16.vi"("Ave N"=2.0, "Array In"=w2847) -> ("Array Out"=w2844:i16[])  [unwired: 1 in]
            n1422 = Interleave 1D Arrays(w2893, w2892, w2891, w2878, w2890, w2889, w2854, w2851, w2853, w2850, w2846, w2845, w2844) -> (w2855:i16[])
            n1423 = Divide(x=w2855, y=3276.7) -> (x/y=w2885:dbl[])
            n1424 = Decimate 1D Array(w2885) -> (w2884:dbl[], w2883:dbl[], w2882:dbl[], w2881:dbl[], w2880:dbl[], w2879:dbl[], w2843:dbl[], w2841:dbl[], w2840:dbl[], w2838:dbl[], w2837:dbl[], w2836:dbl[], w2835:dbl[])
            n1425 = Divide(x=w2884, y=w2882) -> (x/y=w2865:dbl[])
            n1426 = Divide(x=w2883, y=w2882) -> (x/y=w2864:dbl[])
            n1427 = Divide(x=w2881, y=w2879) -> (x/y=w2863:dbl[])
            n1428 = Divide(x=w2880, y=w2879) -> (x/y=w2862:dbl[])
            n1429 = Divide(x=w2843, y=w2841) -> (x/y=w2842:dbl[])
            n1430 = Divide(x=w2840, y=w2838) -> (x/y=w2839:dbl[])
            n1431 = Bundle("T1 Y", "T1 X", "T1 Sum", "T2 Y", "T2 X", "T2 Sum", "T1 FB X", "T2 FB Sum", "T2 FB X", "T2 FB Sum", "PSD Y", "PSD X", "PSD Sum") -> (w2866:T43)  [unwired: 1 out]
            n1432 = Build Array(w2865, w2864, w2882, w2863, w2862, w2879, w2842, w2841, w2839, w2838, w2837, w2836, w2835) -> (w2834:dbl[][])
            n1433 = Cluster To Array(cluster=w2866) -> (array=w2857:string[])
          }
          frame "IR-QPD + PSD + FB-QPD XY positions" {
            w2943 = 4  # Channel pattern
            # "time average x2 the 3 psd signals (detection laser)"
            # "deinterlace 3 signals from qpds"
            n1434 = Decimate 1D Array(w2967) -> (w2966:i16[], w2965:i16[], w2944:i16[], w2964:i16[], w2910:i16[], w2956:i16[], w2955:i16[], w2932:i16[])
            n1435 = Decimate 1D Array "QPD Y"(w2966) -> (w2963:i16[], w2946:i16[])
            n1436 = call "downsample 1D array - double.vi"("Ave N"=2.0, "Array In"=w2956) -> ("Array Out"=w2931:dbl[])  [unwired: 1 out]
            n1437 = call "downsample 1D array - double.vi"("Ave N"=2.0, "Array In"=w2955) -> ("Array Out"=w2930:dbl[])  [unwired: 1 out]
            n1438 = Decimate 1D Array "Feedback Sum"(w2944) -> (w2928:i16[], w2926:i16[])
            n1439 = Decimate 1D Array "Feedback Y"(w2910) -> (w2909:i16[], w2908:i16[])
            n1440 = Decimate 1D Array "Feedback X"(w2932) -> (w2929:i16[], w2927:i16[])
            n1441 = Decimate 1D Array "QPD Sum"(w2964) -> (w2961:i16[], w2959:i16[])
            n1442 = Decimate 1D Array "QPD X"(w2965) -> (w2962:i16[], w2960:i16[])
            n1443 = Interleave 1D Arrays(w2963, w2962, w2961, w2946, w2960, w2959, w2909, w2929, w2928, w2908, w2927, w2926, w2931, w2930) -> (w2954:dbl[])
            n1444 = To Word Integer(number=w2954) -> (16bit integer=w2898:i16[])
            n1445 = Divide(x=w2954, y=3276.7) -> (x/y=w2953:dbl[])
            n1446 = Decimate 1D Array(w2953) -> (w2952:dbl[], w2951:dbl[], w2950:dbl[], w2949:dbl[], w2948:dbl[], w2947:dbl[], w2905:dbl[], w2919:dbl[], w2903:dbl[], w2904:dbl[], w2917:dbl[], w2901:dbl[], w2915:dbl[], w2913:dbl[])
            n1447 = Divide(x=w2952, y=w2950) -> (x/y=w2936:dbl[])
            n1448 = Divide(x=w2951, y=w2950) -> (x/y=w2935:dbl[])
            n1449 = Divide(x=w2949, y=w2947) -> (x/y=w2934:dbl[])
            n1450 = Divide(x=w2948, y=w2947) -> (x/y=w2933:dbl[])
            n1451 = Divide(x=w2905, y=w2903) -> (x/y=w2902:dbl[])
            n1452 = Divide(x=w2919, y=w2903) -> (x/y=w2918:dbl[])
            n1453 = Divide(x=w2904, y=w2901) -> (x/y=w2900:dbl[])
            n1454 = Divide(x=w2917, y=w2901) -> (x/y=w2916:dbl[])
            n1455 = Negate(x=w2913) -> (-x=w2911:dbl[])
            n1456 = Divide(x=w2915, y=w2911) -> (x/y=w2914:dbl[])
            n1457 = Bundle("T1 Y", "T1 X", "T1 Sum", "T2 Y", "T2 X", "T2 Sum", "T1 FB Y", "T1 FB X", "T1 FB Sum", "T2 FB Y", "T2 FB X", "T2 FB Sum", "PSD X", "PSD Y Sum") -> (w2899:T44)  [unwired: 1 out]
            n1458 = Build Array(w2936, w2935, w2950, w2934, w2933, w2947, w2902, w2918, w2903, w2900, w2916, w2901, w2914, w2913) -> (w2912:dbl[][])
            n1459 = Cluster To Array(cluster=w2899) -> (array=w2945:string[])
          }
        }
      }
    }
    "AI labels" <- w2102
    n1460 = Decimate 1D Array(w2072) -> (w2100:u32[], w2036:u32[])
    n1461 = local read "DMA Update Period (s)"() -> (w2111:dbl)
    n1462 = local read "BD 1 Frequency 2 (MHz)"() -> (w1978:dbl)
    n1463 = local read "BD 1 Frequency 1 (MHz)"() -> (w1979:dbl)
    n1464 = Build Array(w2100, w2036) -> (w2179:u32[][])
    n1465 = local read "Data Period (s)"() -> (w2085:dbl)
    n1466 = Decimate 1D Array(w1986) -> (w2009:i16[], w2008:i16[], w2006:i16[], w2005:i16[])  [unwired: 9 out]
    n1467 = To Double Precision Float(number=w2179) -> (double precision float=w2180:dbl[][])
    n1468 = local read "APD Integration Time (s)"() -> (w2049:dbl)
    n1469 = Divide(x=w2009, y=w2008) -> (x/y=w2010:dbl[])
    n1470 = Divide(x=w2006, y=w2005) -> (x/y=w2007:dbl[])
    n1471 = feedback #1(0.0) -> (w2023:dbl)
    n1472 = Add(x=w2111, y=w2023) -> (x+y=w2219:dbl)
    n1473 = feedback-in #1(w2219) -> ()
    n1474 = local read "AOM X Cal (nm/MHz)"() -> (w1976:dbl)
    n1475 = To Time Stamp(1:w2023) -> (0:w2022:timestamp)
    n1476 = Split 1D Array(array=w2010, index="N El. to Ave.") -> (second subarray=w2013:dbl[])  [unwired: 1 out]
    n1477 = Split 1D Array(array=w2007, index="N El. to Ave.") -> (second subarray=w2012:dbl[])  [unwired: 1 out]
    n1478 = local read "Trap X AI1 (DMA)"() -> (w2011:T13)
    n1479 = Multiply(x=w2085, y="Trap Disp. Downsample") -> (x*y=w2024:dbl)
    "Display Period (s)" <- w2024
    n1480 = Bundle("BD 1 Frequency 1 (MHz)"=w1979, "BD 1 Frequency 2 (MHz)"=w1978) -> (w1980:T45)  [unwired: 1 out]
    n1481 = for "Trap AI" {
      tunnel: [w2633] -> w2213 mode=indexing
      tunnel: w2022 -> [w2623]
      tunnel: "Trap Disp. Downsample" -> [w2631]
      tunnel: w2103 -> [w2629] mode=indexing
      tunnel: w2085 -> [w2628]
      tunnel: w2102 -> [w2627] mode=indexing
      tunnel: w2021 -> [w2626]
      tunnel: [w2625] -> w2060 mode=indexing
      tunnel: w2024 -> [w2624]
      n1482 = Bundle By Name("Y"=w2629, "dt"=w2628) -> (w2630:waveform(dbl))  [unwired: 1 out]
      n1483 = Set Waveform Attribute(5:w2627, 6:w2626, 7:w2630) -> (3:w2625:waveform(dbl))  [unwired: 1 in, 2 out]
      n1484 = call "downsample 1D array - double.vi"("Ave N"=w2631, "Array In"=w2629) -> ("Array Out"=w2632:dbl[])  [unwired: 1 out]
      n1485 = Bundle By Name(cluster=w2625, "t0"=w2623, "Y"=w2632, "dt"=w2624) -> (w2633:waveform(dbl))
    }
    n1486 = call-poly <vilib>:"Mean.vi"("X"=w2012) -> ("mean"=w2000:dbl)  [unwired: 1 out]
    n1487 = call-poly <vilib>:"Mean.vi"("X"=w2013) -> ("mean"=w2001:dbl)  [unwired: 1 out]
    n1488 = Cluster To Array(cluster=w1980) -> (array=w1977:dbl[])
    n1489 = Reciprocal(x=w2024) -> (1/x=→"Trap Disp. Freq. (Hz)":dbl)
    n1490 = local read "Data points/scans (MCL)"() -> (w2191:dbl)
    n1491 = To Fixed-Point(number=w2000) -> (fixed-point=w1998:fxp<+/-,16,1>)  [unwired: 1 in]
    n1492 = To Fixed-Point(number=w2001) -> (fixed-point=w1999:fxp<+/-,16,1>)  [unwired: 1 in]
    n1493 = Bundle("Trap 1 Pos.", "Trap 2 Pos.") -> (w2020:cluster{string, string})  [unwired: 1 out]
    n1494 = Bundle By Name(cluster=w2011, "Set 1"=w1999, "Set 2"=w1998) -> (→"Trap X AI1 (DMA)":T13)
    n1495 = Cluster To Array(cluster=w2020) -> (array=w2017:string[])
    n1496 = for "Trap Position" {
      tunnel: w2026 -> [w2273] mode=indexing
      tunnel: "Trap Disp. Downsample" -> [w2272]
      tunnel: w2024 -> [w2270]
      tunnel: w2022 -> [w2269]
      tunnel: w2021 -> [w2267]
      tunnel: w2017 -> [w2266] mode=indexing
      tunnel: [w2265] -> w1975 mode=indexing
      tunnel: w1977 -> [w2263] mode=indexing
      tunnel: w1976 -> [w2261]
      n1497 = call "downsample 1D array - double.vi"("Ave N"=w2272, "Array In"=w2273) -> ("Array Out"=w2271:dbl[])  [unwired: 1 out]
      n1498 = Subtract(x=w2271, y=w2263) -> (x-y=w2264:dbl[])
      n1499 = Multiply(x=w2261, y=w2264) -> (x*y=w2262:dbl[])
      n1500 = Bundle By Name("Y"=w2262, "dt"=w2270, "t0"=w2269) -> (w2268:waveform(dbl))  [unwired: 1 out]
      n1501 = Set Waveform Attribute(5:w2266, 6:w2267, 7:w2268) -> (3:w2265:waveform(dbl))  [unwired: 1 in, 2 out]
    }
    "Trap Positions" <- w1975
    n1502 = Bundle("APD 1", "APD 2") -> (w2212:cluster{string, string})  [unwired: 1 out]
    n1503 = Cluster To Array(cluster=w2212) -> (array=w2209:string[])
    n1504 = for "APD" {
      tunnel: w2180 -> [w2612] mode=indexing
      tunnel: w2049 -> [w2620]
      tunnel: [w2616] -> w2056 mode=indexing
      tunnel: "APD Disp. Scale" -> [w2617]
      tunnel: w2021 -> [w2615]
      tunnel: w2209 -> [w2614] mode=indexing
      tunnel: "APD Disp. Downsample" -> [w2610]
      tunnel: [w2613] -> w2208
      tunnel: w2022 -> [w2609]
      n1505 = call "integrate 1D array interval - double.vi"("Ave N"=w2610, "Array In"=w2612) -> ("Array Out"=w2611:dbl[])  [unwired: 1 out]
      n1506 = Multiply(x=w2620, y=w2610) -> (x*y=w2613:dbl)
      n1507 = Divide(x=w2611, y=w2617) -> (x/y=w2618:dbl[])
      n1508 = Bundle By Name("t0"=w2609, "Y"=w2618, "dt"=w2613) -> (w2619:waveform(dbl))  [unwired: 1 out]
      n1509 = Set Waveform Attribute(5:w2614, 6:w2615, 7:w2619) -> (3:w2616:waveform(dbl))  [unwired: 1 in, 2 out]
    }
    "APD Display Period (s)" <- w2208
    n1510 = Reciprocal(x=w2208) -> (1/x=→"APD Display Freq. (Hz)":dbl)
    n1511 = local read "Display Period (s)"() -> (w2084:dbl)
    n1512 = Increment(x=w2191) -> (x+1=w2192:dbl)
    n1513 = Index Array(array=w1975, index=0) -> (element=w1973:waveform(dbl))
    n1514 = To Double Precision Float(number=w2100) -> (double precision float=w2099:dbl[])
    n1515 = feedback #2(w2192) -> (w2195:dbl)
    n1516 = Select(t=0, s=w2182, f=w2195) -> (s? t:f=w2188:dbl)
    n1517 = Array Size(array=w2099) -> (size(s)=w2194:i32)
    n1518 = Add(x=w2194, y=w2188) -> (x+y=w2189:dbl)
    n1519 = Unbundle By Name(w1973) -> ("Y"=w1971:dbl[])
    n1520 = feedback #3(w2100) -> (w2178:u32[])
    n1521 = Build Array (concatenate)(w2178, w2100) -> (w2175:u32[])
    n1522 = feedback #4(w2036) -> (w2055:u32[])
    n1523 = Divide(x="Bead Sep. Int. Time (s)", y=w2084) -> (x/y=w1969:dbl)
    n1524 = Build Array (concatenate)(w2055, w2036) -> (w2054:u32[])
    n1525 = Greater?(x=w2189, y=w2191) -> (0:w2190:bool)
    n1526 = feedback #5(w1971) -> (w1972:dbl[])
    n1527 = Build Array (concatenate)(w1971, w1972) -> (w1970:dbl[])
    n1528 = Select(t=w2188, s=w2190, f=w2189) -> (s? t:f=w2187:dbl)
    n1529 = feedback-in #2(w2187) -> ()
    n1530 = Array Size(array=w2175) -> (size(s)=w2172:i32)
    n1531 = Array Size(array=w2100) -> (size(s)=w2174:i32)
    n1532 = local read "MCL Scanning"() -> (w2185:bool)
    n1533 = local read "APD Integration Time (s)"() -> (w2063:dbl)
    n1534 = Build Array (concatenate)(w2056, w2213) -> (w2058:waveform(dbl)[])
    "All Signals" <- w2058
    n1535 = Split 1D Array(array=w1970, index=w1969) -> (first subarray=w1963:dbl[])  [unwired: 1 out]
    n1536 = feedback-in #5(w1963) -> ()
    n1537 = Multiply(x=w2174, y="APD Ave N") -> (x*y=w2173:dbl)
    n1538 = Greater?(x=w2172, y=w2173) -> (0:w2176:bool)
    n1539 = Not(x=w2190) -> (.not. x?=w2184:bool)
    n1540 = To Double Precision Float(number=w2036) -> (double precision float=w2035:dbl[])
    n1541 = call-poly <vilib>:"Mean.vi"("X"=w1963) -> ("mean"=w1962:dbl)  [unwired: 1 out]
    "Mean T1 Position (nm)" <- w1962
    n1542 = Subtract(x=w1963, y=w1962) -> (x-y=w1968:dbl[])
    n1543 = Square(x=w1968) -> (x^2=w1967:dbl[])
    n1544 = And(x=w2184, y=w2185) -> (x .and. y?=w2186:bool)
    n1545 = call-poly <vilib>:"Mean.vi"("X"=w1967) -> ("mean"=w1966:dbl)  [unwired: 1 out]
    n1546 = case shown="True" w2176 {
      tunnel: w2175 -> [w2393 w2400]
      tunnel: [w2393 w2398] -> w2116
      tunnel: w2173 -> [_ w2395]
      tunnel: w2172 -> [_ w2399]
      tunnel: w2054 -> [w2392 w2397]
      tunnel: [w2392 w2394] -> w2051
      frame False {
      }
      frame True {
        n1547 = Subtract(x=w2399, y=w2395) -> (x-y=w2396:dbl)
        n1548 = Array Subset(array=w2400, index=w2396, length=w2395) -> (w2398:u32[])
        n1549 = Array Subset(array=w2397, index=w2396, length=w2395) -> (w2394:u32[])
      }
    }
    n1550 = feedback-in #3(w2116) -> ()
    n1551 = feedback-in #4(w2051) -> ()
    n1552 = Or(x=w2186, y=w2182) -> (x .or. y?=w2183:bool)
    n1553 = Square Root(x=w1966) -> (sqrt(x)=w1965:dbl)
    n1554 = Equal?(x="Tab Control 6", y=T35."High Res Display") -> (x = y?=w2106:bool)
    n1555 = Multiply(x="APD Disp. Scale", y=w2056) -> (x*y=w2065:waveform(dbl)[])
    n1556 = Multiply(x="APD Disp. Downsample", y=w2063) -> (x*y=w2061:dbl)
    n1557 = Multiply(x=10.0, y=w1965) -> (x*y=→"Trap 1 Position RMS (A)":dbl)
    n1558 = Divide(x=w2065, y=w2061) -> (x/y=w2033:waveform(dbl)[])
    n1559 = Index Array(array=w2033, index=0) -> (element=w2043:waveform(dbl))
    n1560 = case "For computing FFTs for display" shown="True" "Compute FFT" {
      tunnel: w2060 -> [_ w3070]
      frame False {
      }
      frame True {
        n1561 = Build Array("FFT 1 Choice 1", "FFT 1 Choice 2", "FFT 2 Choice 1", "FFT 2 Choice 2") -> (w3063:u16[])
        n1562 = Array Size(array=w3070) -> (size(s)=w3069:i32)
        n1563 = feedback-in #6(w3063) -> ()
        n1564 = feedback #6(u16[] [100, 100, 100, 100]) -> (w3064:u16[])
        n1565 = feedback-in #7("# Spectra to Ave.") -> ()
        n1566 = feedback #7("# Spectra to Ave.") -> (w3061:dbl)
        n1567 = Not Equal?(x="# Spectra to Ave.", y=w3061) -> (x != y?=w3060:bool)
        n1568 = Not Equal?(x=w3063, y=w3064) -> (x != y?=w3062:bool)
        n1569 = feedback #8(1.0) -> (w3047:dbl)
        n1570 = Compound Arithmetic op=OR("Reset FFT", w3062, w3060) -> (w3045:bool)
        n1571 = Select(t=1.0, s=w3045, f=w3047) -> (s? t:f=w3049:dbl)
        n1572 = Greater?(x=w3049, y="# Spectra to Ave.") -> (0:w3068:bool)
        n1573 = Increment(x=w3049) -> (x+1=w3048:dbl)
        n1574 = feedback-in #8(w3048) -> ()
        n1575 = local read "DMA Update Period (s)"() -> (w3043:dbl)
        n1576 = Multiply(x="# Spectra to Ave.", y=w3043) -> (x*y=→"Ave. Time (s)":dbl)
        n1577 = Build Array(cluster{"f0":dbl, "df":dbl, "magnitude":dbl[]} {"f0"=0.0, "df"=0.0, "magnitude"=[]} ("PSD")) -> (w3052:cluster{"f0":dbl, "df":dbl, "magnitude":dbl[]}[])
        n1578 = Build Array(w3052, w3052, w3052, w3052) -> (w3054:T46)
        n1579 = feedback #9(w3054) -> (w3059:T46)
        n1580 = for {
          N: 4 -> [_]
          tunnel: w3063 -> [w3092] mode=indexing
          tunnel: w3070 -> [w3093]
          tunnel: w3069 -> [w3095]
          tunnel: w3045 -> [w3088]
          tunnel: w3068 -> [w3087]
          tunnel: "# Spectra to Ave." -> [w3086]
          tunnel: [w3085] -> w3058 mode=indexing
          tunnel: w3059 -> [w3090] mode=indexing
          tunnel: [w3089] -> w3046 mode=indexing
          tunnel: w3049 -> [w3084]
          n1581 = Less?(x=w3092, y=w3095) -> (x < y?=w3094:bool)
          n1582 = Index Array(array=w3093, index=w3092) -> (element=w3091:waveform(dbl))
          n1583 = case shown="True" w3094 {
            tunnel: w3091 -> [_ w3112]
            tunnel: w3090 -> [w3097 w3110]
            tunnel: [w3097 w3098] -> w3089
            tunnel: w3088 -> [_ w3109]
            tunnel: w3087 -> [_ w3102]
            tunnel: w3086 -> [_ w3101]
            tunnel: [cluster{"f0":dbl, "df":dbl, "magnitude":dbl[]} {"f0"=0.0, "df"=0.0, "magnitude"=[]} ("PSD") w3103] -> w3085
            tunnel: w3084 -> [_ w3100]
            frame False {
            }
            frame True {
              n1584 = call <vilib>:"Std Deviation and Variance.vi"("X"=w3112) -> ("mean"=w3113:dbl)  [unwired: 1 in, 2 out]
              n1585 = Subtract(x=w3112, y=w3113) -> (x-y=w3111:waveform(dbl))
              n1586 = xnode "Spectral Measurements"("Signals"=w3111) -> ("PSD"=w3105:cluster{"f0":dbl, "df":dbl, "magnitude":dbl[]})  [unwired: 1 in, 1 out]
              n1587 = case shown="False" w3109 {
                tunnel: w3110 -> [w3122 _]
                tunnel: [w3118 w3127] -> w3098
                tunnel: w3105 -> [w3121 w3128]
                tunnel: w3102 -> [w3120 _]
                frame False {
                  n1588 = Build Array (concatenate)(w3122, w3121) -> (w3119:cluster{"f0":dbl, "df":dbl, "magnitude":dbl[]}[])
                  n1589 = case shown="True" w3120 {
                    tunnel: w3119 -> [w3123 w3126]
                    tunnel: [w3123 w3124] -> w3118
                    frame False {
                    }
                    frame True {
                      n1590 = Delete From Array(array=w3126, index=0) -> (array with subset deleted=w3124:cluster{"f0":dbl, "df":dbl, "magnitude":dbl[]}[])  [unwired: 1 in, 1 out]
                    }
                  }
                }
                frame True {
                  n1591 = Build Array(w3128) -> (w3127:cluster{"f0":dbl, "df":dbl, "magnitude":dbl[]}[])
                }
              }
              n1592 = for {
                tunnel: w3098 -> [w3117] mode=indexing
                tunnel: [w3116] -> w3108 mode=indexing
                workers-P: _ -> [_]
                n1593 = Unbundle By Name(w3117) -> ("magnitude"=w3116:dbl[])
              }
              n1594 = Transpose 2D Array(2D array=w3108) -> (transposed array=w3107:dbl[][])
              n1595 = for {
                tunnel: w3107 -> [w3115] mode=indexing
                tunnel: [w3114] -> w3106 mode=indexing
                workers-P: _ -> [_]
                n1596 = Add Array Elements(numeric array=w3115) -> (sum=w3114:dbl)
              }
              n1597 = Select(t=w3101, s=w3102, f=w3100) -> (s? t:f=w3099:dbl)
              n1598 = Divide(x=w3106, y=w3099) -> (x/y=w3104:dbl[])
              n1599 = Bundle By Name(cluster=w3105, "magnitude"=w3104) -> (w3103:cluster{"f0":dbl, "df":dbl, "magnitude":dbl[]})
            }
          }
        }
        n1600 = case shown="True" w3045 {
          tunnel: w3046 -> [w3077 w3083]
          tunnel: [w3077 w3078] -> w3044
          frame False {
          }
          frame True {
            n1601 = Array Subset(array=w3083, index (row)=0 ("index"), length (row)=4 ("length"), index (col)=0 ("index"), length (col)=1 ("length")) -> (w3078:T46)
          }
        }
        n1602 = feedback-in #9(w3044) -> ()
        n1603 = Split 1D Array(array=w3058, index=2) -> (first subarray=→"FFT 1":cluster{"f0":dbl, "df":dbl, "magnitude":dbl[]}[], second subarray=→"FFT 2":cluster{"f0":dbl, "df":dbl, "magnitude":dbl[]}[])
      }
    }
    n1604 = Index Array(array=w2033, index=1) -> (element=w2041:waveform(dbl))
    n1605 = case "For displaying the high resolution display (no downsampling)" shown="True" w2106 {
      tunnel: w2060 -> [_ w2293]
      frame False {
      }
      frame True {
        n1606 = Index Array(array=w2293, index="High Res. Display") -> (element=w2294:waveform(dbl))
        n1607 = call <vilib>:"Std Deviation and Variance.vi"("X"=w2294) -> ("mean"=w2301:dbl, "standard deviation"=w2306:dbl)  [unwired: 1 in, 1 out]
        "Mean Intensity" <- w2301
        "Sigma" <- w2306
        n1608 = Subtract(x=w2294, y=w2301) -> (x-y=w2300:waveform(dbl))
        n1609 = Select(t=w2300, s="Subtract mean", f=w2294) -> (s? t:f=→"1 Channel":waveform(dbl))
        n1610 = Divide(x=w2306, y=w2301) -> (x/y=→"Sigma/Mean":dbl)
        n1611 = feedback #10(1) -> (w2295:i32)
        n1612 = Greater Or Equal?(x=w2295, y="Slow mean N ave.") -> (x >= y?=w2308:bool)
        n1613 = Increment(x=w2295) -> (x+1=w2310:i32)
        n1614 = Select(t=1, s=w2308, f=w2310) -> (s? t:f=w2297:i32)
        n1615 = feedback-in #10(w2297) -> ()
        n1616 = feedback #11() -> (w2298:waveform(dbl))  [unwired: 1 out]
        n1617 = case shown="Default" w2295 {
          tunnel: [w2313 w2316] -> w2299
          tunnel: w2298 -> [w2315 _]
          tunnel: w2294 -> [w2314 w2316]
          frame Default {
            n1618 = call-poly <vilib>:"Append Waveforms.vi"("waveform B"=w2314, "waveform A"=w2315) -> ("waveform out"=w2313:waveform(dbl))  [unwired: 1 in, 8 out]
          }
          frame 1 {
          }
        }
        n1619 = feedback-in #11(w2299) -> ()
        n1620 = case shown="True" w2308 {
          tunnel: w2299 -> [_ w2312]
          frame False {
          }
          frame True {
            n1621 = call-poly <vilib>:"Mean.vi"("X"=w2312) -> ("mean"=→"Slow mean":dbl)  [unwired: 1 out]
          }
        }
      }
    }
    n1622 = case "For plotting results of scanning MCL" shown="True" w2183 {
      tunnel: w2182 -> [_ w2433]
      tunnel: w2099 -> [_ w2529]
      tunnel: w2191 -> [_ _]
      tunnel: w2060 -> [_ w2503]
      tunnel: w2035 -> [_ w2434]
      tunnel: w2034 -> [_ w2407]
      frame False {
      }
      frame True {
        w2414 = u32 0 items=["Horizontal", "Vertical", "Central", "1st Diagonal", "2nd Diagonal"] ("Type of Symmetry")
        w2442 = u32 0 items=["Horizontal", "Vertical", "Central", "1st Diagonal", "2nd Diagonal"] ("Type of Symmetry")
        w2445 = u32 0 items=["Horizontal", "Vertical", "Central", "1st Diagonal", "2nd Diagonal"] ("Type of Symmetry")
        w2474 = u32 0 items=["Horizontal", "Vertical", "Central", "1st Diagonal", "2nd Diagonal"] ("Type of Symmetry")
        n1623 = Index Array(array=w2503, index=10) -> (element=w2509:waveform(dbl))
        n1624 = Index Array(array=w2503, index=11) -> (element=w2506:waveform(dbl))
        n1625 = local read "Cycles/step (MCL)"() -> (w2459:u64)
        n1626 = Index Array(array=w2503, index="Channel") -> (element=w2505:waveform(dbl))
        n1627 = Unbundle(w2407) -> ("New Image"=w2406:T3, "New Image"=w2405:T3, "New Image"=w2404:T3, "New Image"=w2403:T3)
        n1628 = Unbundle By Name(w2509) -> ("Y"=w2461:dbl[])
        n1629 = Unbundle By Name(w2506) -> ("Y"=w2463:dbl[])
        n1630 = Unbundle By Name(w2505) -> ("Y"=w2468:dbl[])
        n1631 = call "downsample 1D array - double.vi"("Ave N"=w2459, "Array In"=w2461) -> ("Array Out"=w2460:dbl[])  [unwired: 1 out]
        n1632 = call "downsample 1D array - double.vi"("Ave N"=w2459, "Array In"=w2463) -> ("Array Out"=w2462:dbl[])  [unwired: 1 out]
        n1633 = call "downsample 1D array - double.vi"("Ave N"=w2459, "Array In"=w2468) -> ("Array Out"=w2467:dbl[])  [unwired: 1 out]
        n1634 = feedback #12(w2529) -> (w2530:dbl[])
        n1635 = Build Array (concatenate)(w2530, w2529) -> (w2511:dbl[])
        n1636 = feedback #13(w2434) -> (w2436:dbl[])
        n1637 = Build Array (concatenate)(w2436, w2434) -> (w2435:dbl[])
        n1638 = local read "Scan steps (MCL)"() -> (w2416:u64)
        n1639 = Select(t=w2529, s=w2433, f=w2511) -> (s? t:f=w2515:dbl[])
        n1640 = feedback-in #12(w2515) -> ()
        n1641 = Select(t=w2434, s=w2433, f=w2435) -> (s? t:f=w2417:dbl[])
        n1642 = feedback-in #13(w2417) -> ()
        n1643 = local read "Scan lines (y)"() -> (w2402:u64)
        n1644 = local read "N APD Samp/step"() -> (w2418:dbl)
        n1645 = feedback #14(w2460) -> (w2517:dbl[])
        n1646 = Build Array (concatenate)(w2517, w2460) -> (w2508:dbl[])
        n1647 = feedback #15(w2467) -> (w2527:dbl[])
        n1648 = Build Array (concatenate)(w2527, w2467) -> (w2526:dbl[])
        n1649 = feedback #16(w2462) -> (w2519:dbl[])
        n1650 = Build Array (concatenate)(w2519, w2462) -> (w2520:dbl[])
        n1651 = Select(t=w2460, s=w2433, f=w2508) -> (s? t:f=w2464:dbl[])
        n1652 = feedback-in #14(w2464) -> ()
        n1653 = Select(t=w2467, s=w2433, f=w2526) -> (s? t:f=w2466:dbl[])
        n1654 = feedback-in #15(w2466) -> ()
        n1655 = Select(t=w2462, s=w2433, f=w2520) -> (s? t:f=w2465:dbl[])
        n1656 = feedback-in #16(w2465) -> ()
        n1657 = Multiply(x=w2416, y=u64 2) -> (x*y=w2401:u64)
        n1658 = call "integrate 1D array interval - double.vi"("Ave N"=w2418, "Array In"=w2417) -> ("Array Out"=w2429:dbl[])  [unwired: 1 out]
        n1659 = call "integrate 1D array interval - double.vi"("Ave N"=w2418, "Array In"=w2515) -> ("Array Out"=w2514:dbl[])  [unwired: 1 out]
        n1660 = Array Size(array=w2429) -> (size(s)=w2430:i32)
        n1661 = Array Size(array=w2514) -> (size(s)=w2516:i32)
        n1662 = Multiply(x=w2402, y=w2401) -> (x*y=w2432:u64)
        n1663 = Multiply(x=w2402, y=w2401) -> (x*y=w2524:u64)
        n1664 = call-poly <vilib>:"Mean.vi"("X"=w2464) -> ("mean"=w2448:dbl)  [unwired: 1 out]
        n1665 = Subtract(x=w2432, y=w2430) -> (x-y=w2423:u64)
        n1666 = call-poly <vilib>:"Mean.vi"("X"=w2466) -> ("mean"=w2453:dbl)  [unwired: 1 out]
        n1667 = call-poly <vilib>:"Mean.vi"("X"=w2465) -> ("mean"=w2451:dbl)  [unwired: 1 out]
        n1668 = call-poly <vilib>:"Mean.vi"("X"=w2429) -> ("mean"=w2420:dbl)  [unwired: 1 out]
        n1669 = Subtract(x=w2524, y=w2516) -> (x-y=w2458:u64)
        n1670 = call-poly <vilib>:"Mean.vi"("X"=w2514) -> ("mean"=w2455:dbl)  [unwired: 1 out]
        n1671 = Initialize Array(1.0 ("element"), w2423) -> (w2419:dbl[])
        n1672 = Initialize Array(1.0 ("element"), w2458) -> (w2449:dbl[])
        n1673 = Multiply(x=w2419, y=w2420) -> (x*y=w2421:dbl[])
        n1674 = Multiply(x=w2449, y=w2451) -> (x*y=w2452:dbl[])
        n1675 = Multiply(x=w2449, y=w2453) -> (x*y=w2454:dbl[])
        n1676 = Multiply(x=w2449, y=w2448) -> (x*y=w2450:dbl[])
        n1677 = Multiply(x=w2449, y=w2455) -> (x*y=w2456:dbl[])
        n1678 = Build Array (concatenate)(w2464, w2450) -> (w2518:dbl[])
        n1679 = Build Array (concatenate)(w2466, w2454) -> (w2522:dbl[])
        n1680 = Build Array (concatenate)(w2465, w2452) -> (w2521:dbl[])
        n1681 = Build Array (concatenate)(w2429, w2421) -> (w2431:dbl[])
        n1682 = Build Array (concatenate)(w2514, w2456) -> (w2523:dbl[])
        n1683 = Reshape Array(w2518, w2402, w2401) -> (w2484:dbl[][])
        n1684 = Reshape Array(w2431, w2402, w2401) -> (w2427:dbl[][])
        n1685 = Reshape Array(w2522, w2402, w2401) -> (w2476:dbl[][])
        n1686 = Reshape Array(w2521, w2402, w2401) -> (w2491:dbl[][])
        n1687 = Reshape Array(w2523, w2402, w2401) -> (w2501:dbl[][])
        n1688 = Array Subset(array=w2491, index (col)=0 ("index"), length (col)=w2416) -> (w2496:dbl[][])  [unwired: 2 in]
        n1689 = Array Subset(array=w2491, index (col)=w2416) -> (w2494:dbl[][])  [unwired: 3 in]
        n1690 = Array Subset(array=w2476, index (col)=0 ("index"), length (col)=w2416) -> (w2482:dbl[][])  [unwired: 2 in]
        n1691 = Array Subset(array=w2476, index (col)=w2416) -> (w2480:dbl[][])  [unwired: 3 in]
        n1692 = Array Subset(array=w2427, index (col)=0 ("index"), length (col)=w2416) -> (w2426:dbl[][])  [unwired: 2 in]
        n1693 = Array Subset(array=w2427, index (col)=w2416) -> (w2424:dbl[][])  [unwired: 3 in]
        n1694 = Array Subset(array=w2501, index (col)=0 ("index"), length (col)=w2416) -> (w2500:dbl[][])  [unwired: 2 in]
        n1695 = Array Subset(array=w2501, index (col)=w2416) -> (w2498:dbl[][])  [unwired: 3 in]
        n1696 = Array Subset(array=w2484, index (col)=0 ("index"), length (col)=w2416) -> (w2489:dbl[][])  [unwired: 2 in]
        n1697 = Array Subset(array=w2484, index (col)=w2416) -> (w2487:dbl[][])  [unwired: 3 in]
        n1698 = for {
          tunnel: w2496 -> [w2538] mode=indexing
          tunnel: [w2537] -> w2495 mode=indexing
          workers-P: _ -> [_]
          n1699 = Reverse 1D Array(array=w2538) -> (reversed array=w2537:dbl[])
        }
        n1700 = for {
          tunnel: w2482 -> [w2534] mode=indexing
          tunnel: [w2533] -> w2481 mode=indexing
          workers-P: _ -> [_]
          n1701 = Reverse 1D Array(array=w2534) -> (reversed array=w2533:dbl[])
        }
        n1702 = for {
          tunnel: w2426 -> [w2532] mode=indexing
          tunnel: [w2531] -> w2425 mode=indexing
          workers-P: _ -> [_]
          n1703 = Reverse 1D Array(array=w2532) -> (reversed array=w2531:dbl[])
        }
        n1704 = for {
          tunnel: w2500 -> [w2540] mode=indexing
          tunnel: [w2539] -> w2499 mode=indexing
          workers-P: _ -> [_]
          n1705 = Reverse 1D Array(array=w2540) -> (reversed array=w2539:dbl[])
        }
        n1706 = for {
          tunnel: w2489 -> [w2536] mode=indexing
          tunnel: [w2535] -> w2488 mode=indexing
          workers-P: _ -> [_]
          n1707 = Reverse 1D Array(array=w2536) -> (reversed array=w2535:dbl[])
        }
        n1708 = Index Array(array=w2501, index (row)=0) -> (element=→"Waveform Graph":dbl[])  [unwired: 1 in]
        n1709 = Add(x=w2495, y=w2494) -> (x+y=w2493:dbl[][])
        n1710 = Add(x=w2481, y=w2480) -> (x+y=w2479:dbl[][])
        n1711 = Add(x=w2425, y=w2424) -> (x+y=w2409:dbl[][])
        n1712 = Add(x=w2499, y=w2498) -> (x+y=w2473:dbl[][])
        n1713 = Add(x=w2488, y=w2487) -> (x+y=w2486:dbl[][])
        n1714 = Divide(x=w2479, y=2) -> (x/y=w2477:dbl[][])
        n1715 = Divide(x=w2493, y=2) -> (x/y=w2438:dbl[][])
        n1716 = Divide(x=w2486, y=2) -> (x/y=w2440:dbl[][])
        n1717 = To Single Precision Float(number=w2473) -> (single precision float=w2472:sgl[][])
        n1718 = Transpose 2D Array(2D array=w2477) -> (transposed array=→"Data map":dbl[][])
        n1719 = To Single Precision Float(number=w2409) -> (single precision float=w2413:sgl[][])
        n1720 = To Single Precision Float(number=w2438) -> (single precision float=w2444:sgl[][])
        n1721 = To Single Precision Float(number=w2440) -> (single precision float=w2441:sgl[][])
        n1722 = call "IMAQ ArrayToImage"("Image Pixels (Float)"=w2472, "Image"=w2406) -> ("Image Out"=w2475:T3)  [unwired: 8 in, 1 out]
        n1723 = call "IMAQ ArrayToImage"("Image Pixels (Float)"=w2413, "Image"=w2405) -> ("Image Out"=w2415:T3)  [unwired: 8 in, 1 out]
        n1724 = call "IMAQ ArrayToImage"("Image Pixels (Float)"=w2444, "Image"=w2404) -> ("Image Out"=w2446:T3)  [unwired: 8 in, 1 out]
        n1725 = call "IMAQ ArrayToImage"("Image Pixels (Float)"=w2441, "Image"=w2403) -> ("Image Out"=w2443:T3)  [unwired: 8 in, 1 out]
        n1726 = call "IMAQ Symmetry"("Type of Symmetry"=w2474, "Image Src"=w2475) -> ("Image Dst Out"=w2470:T3)  [unwired: 3 in, 1 out]
        n1727 = call "IMAQ Symmetry"("Type of Symmetry"=w2414, "Image Src"=w2415) -> ("Image Dst Out"=w2411:T3)  [unwired: 3 in, 1 out]
        n1728 = call "IMAQ Symmetry"("Type of Symmetry"=w2445, "Image Src"=w2446) -> ("Image Dst Out"=→"Detection Laser X":T3)  [unwired: 3 in, 1 out]
        n1729 = call "IMAQ Symmetry"("Type of Symmetry"=w2442, "Image Src"=w2443) -> ("Image Dst Out"=→"Detection Laser Y":T3)  [unwired: 3 in, 1 out]
        n1730 = call "IMAQ Set Simple Calibration"("Calibration Axis Info"=T36 {"Origin Pixel"={"X"=0.0, "Y"=0.0}, "Angle Relative to Horizontal (deg)"=0.0, "Axis Reference"=0}, "Grid Descriptor"=T37 {"X Step"=0.3, "Y Step"=0.3, "Unit"=enum."Undefined"}, "Image"=w2470) -> ("Calibrated Image"=→"APD 1":T3)  [unwired: 7 in, 1 out]
        n1731 = call "IMAQ Set Simple Calibration"("Calibration Axis Info"=T36 {"Origin Pixel"={"X"=0.0, "Y"=0.0}, "Angle Relative to Horizontal (deg)"=0.0, "Axis Reference"=0}, "Grid Descriptor"=T37 {"X Step"=0.3, "Y Step"=0.3, "Unit"=enum."Undefined"}, "Image"=w2411) -> ("Calibrated Image"=→"APD 2":T3)  [unwired: 7 in, 1 out]
      }
    }
    n1732 = Subtract(x=w2041, y="APD 2 Offset") -> (x-y=w2038:waveform(dbl))
    n1733 = Subtract(x=w2043, y="APD 1 Offset") -> (x-y=w2039:waveform(dbl))
    n1734 = Index Array(array=w2058, index=3) -> (element=w2127:waveform(dbl))
    n1735 = Index Array(array=w2058, index=6) -> (element=w2124:waveform(dbl))
    n1736 = Build Array(w2039, w2038) -> (→"APD Chart":waveform(dbl)[])
    n1737 = Array Size(array=w2116) -> (size(s)=w2171:i32)
    n1738 = call <vilib>:"Std Deviation and Variance.vi"("X"=w2051) -> ("standard deviation"=w2050:dbl)  [unwired: 1 in, 2 out]
    n1739 = Add Array Elements(numeric array=w2051) -> (sum=w2053:u32)
    n1740 = Add Array Elements(numeric array=w2116) -> (sum=w2181:u32)
    n1741 = call <vilib>:"Std Deviation and Variance.vi"("X"=w2116) -> ("standard deviation"=w2115:dbl)  [unwired: 1 in, 2 out]
    n1742 = Divide(x="T1 offset_x (mV)", y=1000.0) -> (x/y=w2128:dbl)
    n1743 = Divide(x=w2050, y=w2049) -> (x/y=w2046:dbl)
    "Rate sigma (Hz) 2" <- w2046
    n1744 = Multiply(x=w2049, y=w2171) -> (x*y=w2052:dbl)
    "Int. Time (s)" <- w2052
    n1745 = Divide(x=w2053, y=w2052) -> (x/y=w2047:dbl)
    "APD 2 Rate (Hz)" <- w2047
    n1746 = Divide(x=w2181, y=w2052) -> (x/y=w2113:dbl)
    "APD 1 Rate (Hz)" <- w2113
    n1747 = Divide(x=w2115, y=w2049) -> (x/y=w2114:dbl)
    "Rate sigma (Hz)" <- w2114
    n1748 = Divide(x=w2046, y=w2047) -> (x/y=→"Sigma/Mean 2":dbl)
    n1749 = Divide(x=w2114, y=w2113) -> (x/y=→"Sigma/Mean":dbl)
    n1750 = Divide(x="T2 offset_x (mV)", y=1000.0) -> (x/y=w2126:dbl)
    n1751 = case shown="1" "Calibration" {
      tunnel: "T1 alpha_x (nm/V)" -> [_ w2369 w2390]
      tunnel: "T1 kappa_x (pN/nm)" -> [_ _ w2380]
      tunnel: "T2 alpha_x (nm/V)" -> [_ w2368 w2388]
      tunnel: "T2 kappa_x (pN/nm)" -> [_ _ w2381]
      tunnel: w2127 -> [w2351 w2366 w2386]
      tunnel: w2124 -> [w2350 w2364 w2384]
      tunnel: [w2351 w2363 w2383] -> w2157
      tunnel: [w2350 w2362 w2382] -> w2156
      tunnel: ["T1 X (V)" ("Label.Text") "T1 X (nm)" ("Label.Text") "T1 X (pN)" ("Label.Text")] -> w2145
      tunnel: ["T2 X (V)" ("Label.Text") "T2 X (nm)" ("Label.Text") "T2 X (pN)" ("Label.Text")] -> w2144
      tunnel: ["Position (V)" ("Label.Text") "Position (nm)" ("Label.Text") "Force (pN)" ("Label.Text")] -> w2146
      tunnel: w2126 -> [_ w2354 w2373]
      tunnel: w2128 -> [_ w2357 w2375]
      tunnel: ["Mean (V)" ("Label.Text") "Mean (nm)" ("Label.Text") "Mean (pN)" ("Label.Text")] -> w2141
      tunnel: ["Difference (V)" ("Label.Text") "Difference (nm)" ("Label.Text") "Difference (pN)" ("Label.Text")] -> w2066
      frame 0, Default {
      }
      frame 1 {
        # "position"
        n1752 = Unbundle By Name(w2366) -> ("Y"=w2370:dbl[])
        n1753 = Unbundle By Name(w2364) -> ("Y"=w2355:dbl[])
        n1754 = Subtract(x=w2370, y=w2357) -> (x-y=w2358:dbl[])
        n1755 = Subtract(x=w2355, y=w2354) -> (x-y=w2356:dbl[])
        n1756 = Multiply(x=w2356, y=w2368) -> (x*y=w2365:dbl[])
        n1757 = Multiply(x=w2369, y=w2358) -> (x*y=w2367:dbl[])
        n1758 = Bundle By Name(cluster=w2364, "Y"=w2365) -> (w2362:waveform(dbl))
        n1759 = Bundle By Name(cluster=w2366, "Y"=w2367) -> (w2363:waveform(dbl))
      }
      frame 2 {
        # "force"
        n1760 = Unbundle By Name(w2386) -> ("Y"=w2391:dbl[])
        n1761 = Unbundle By Name(w2384) -> ("Y"=w2389:dbl[])
        n1762 = Subtract(x=w2389, y=w2373) -> (x-y=w2374:dbl[])
        n1763 = Subtract(x=w2391, y=w2375) -> (x-y=w2376:dbl[])
        n1764 = Compound Arithmetic op=MULTIPLY(w2374, w2388, w2381) -> (w2385:dbl[])
        n1765 = Compound Arithmetic op=MULTIPLY(w2380, w2390, w2376) -> (w2387:dbl[])
        n1766 = Bundle By Name(cluster=w2384, "Y"=w2385) -> (w2382:waveform(dbl))
        n1767 = Bundle By Name(cluster=w2386, "Y"=w2387) -> (w2383:waveform(dbl))
      }
    }
    n1768 = feedback-in #17("Calibration") -> ()
    n1769 = feedback #17(u16 1 ("Calibration")) -> (w2148:u16)
    n1770 = Not Equal?(x=w2148, y="Calibration") -> (x != y?=w2104:bool)
    n1771 = Unbundle By Name(w2127) -> ("Y"=w2130:dbl[])
    n1772 = Unbundle By Name(w2124) -> ("Y"=w2133:dbl[])
    n1773 = Subtract(x=w2130, y=w2128) -> (x-y=w2131:dbl[])
    n1774 = Subtract(x=w2133, y=w2126) -> (x-y=w2132:dbl[])
    n1775 = disable-structure shown="Enabled" {
      disable-tunnel: [-1.0 ("y") 1.0] -> w2134
      frame Disabled {
      }
      frame Enabled {
      }
    }
    n1776 = Multiply(x=w2132, y="T2 alpha_x (nm/V)") -> (x*y=w2123:dbl[])
    n1777 = Multiply(x="T1 alpha_x (nm/V)", y=w2131) -> (x*y=w2122:dbl[])
    n1778 = Multiply(x=w2156, y=w2134) -> (x*y=w2135:waveform(dbl))
    n1779 = case shown="False" "Read Lateness and Rel Phase" {
      tunnel: w1958 -> [w2317 w2339]
      tunnel: w1957 -> [w2318 w2338]
      tunnel: [w2317 w2337] -> w2119
      tunnel: [w2318 w2336] -> w2118
      frame False {
      }
      frame True {
        n1780 = xnode "Read/Write Control"("FPGA VI Reference In"=w2339, "error in"=w2338) -> ("FPGA VI Reference Out"=w2337:T19, "error out"=w2336:errorcluster, "GI Relative phase"=→"GI relative phase":i16, "Relative phase"=→"Relative phase (AI1)":i16, "AI Late Counter"=→"Late Counter (AI1)":u16, "GI Late Counter"=→"GI Late Counter":u16, "MCL Late Counter"=→"MCL Late Counter":u16, "MCL Relative Phase"=→"Relative Phase (MCL)":i16, "APD Acq Relative Phase"=→"APD Acq Relative Phase":i16, "APD 1 Gate Relative Phase"=→"APD 1 Gate Relative Phase":i16, "APD 2 Gate Relative Phase"=→"APD 2 Gate Relative Phase":i16, "APD Acq Late Counter"=→"APD Acq Late Counter":u16, "APD 1 Gate Late Counter"=→"APD 1 Gate Late Counter":u16, "APD 2 Gate Late Counter"=→"APD 2 Gate Late Counter":u16, "Green FB Relative Phase"=→"Relative phase (Green FB)":i16, "GI Relative phase 2"=→"GI relative phase 2":i16, "GI Late Counter 2"=→"GI Late Counter 2":u16, "Trap Pos FIFO Timeout"=→"Trap Pos FIFO Timeout":u16, "Trap AI FIFO Timeout"=→"Trap AI FIFO Timeout":u16)
      }
    }
    n1781 = Subtract(x=w2123, y=w2122) -> (x-y=w2121:dbl[])
    n1782 = Unbundle By Name(w2156) -> ("Y"=w2091:dbl[])
    n1783 = Unbundle By Name(w2157) -> ("Y"=w2092:dbl[])
    n1784 = Build Array(w2157, w2135) -> (→"Force":waveform(dbl)[])
    n1785 = Subtract(x=w2121, y="Offset (nm)") -> (x-y=w2089:dbl[])
    n1786 = call-poly <vilib>:"Mean.vi"("X"=w2091) -> ("mean"=w2070:dbl)  [unwired: 1 out]
    "T2 X" <- w2070
    n1787 = Absolute Value(x=w2092) -> (abs(x)=w2093:dbl[])
    n1788 = Absolute Value(x=w2091) -> (abs(x)=w2094:dbl[])
    n1789 = call-poly <vilib>:"Mean.vi"("X"=w2092) -> ("mean"=w2071:dbl)  [unwired: 1 out]
    "T1 X" <- w2071
    n1790 = Add(x=w2093, y=w2094) -> (x+y=w2095:dbl[])
    n1791 = Bundle By Name(cluster=w2127, "Y"=w2089) -> (w2057:waveform(dbl))
    "Bead Separation" <- w2057
    n1792 = Divide(x=w2095, y=2.0) -> (x/y=→"Vec Mean of T1 T2":dbl[])
    n1793 = case shown="True" w2104 {
      tunnel: w2146 -> [_ w2344]
      tunnel: w2145 -> [_ w2343]
      tunnel: w2144 -> [_ w2342]
      tunnel: w2141 -> [_ w2341]
      tunnel: w2066 -> [_ w2340]
      frame False {
      }
      frame True {
        n1794 = property on="Force" class="WFChart (strict)"("YScale.NameLbl.Text"=w2344) -> ()  [unwired: 2 in, 2 out]
        n1795 = property on="T2 X" class="DigNum (strict)"("Caption.Text"=w2342) -> ()  [unwired: 2 in, 2 out]
        n1796 = property on="T1 X" class="DigNum (strict)"("Caption.Text"=w2343) -> ()  [unwired: 2 in, 2 out]
        n1797 = property on="Mean" class="DigNum (strict)"("Caption.Text"=w2341) -> ()  [unwired: 2 in, 2 out]
        n1798 = property on="Difference" class="DigNum (strict)"("Caption.Text"=w2340) -> ()  [unwired: 2 in, 2 out]
      }
    }
    n1799 = local read "Tether"() -> (w2098:bool)
    n1800 = Absolute Value(x=w2071) -> (abs(x)=w2068:dbl)
    n1801 = Absolute Value(x=w2070) -> (abs(x)=w2067:dbl)
    n1802 = Add(x=w2068, y=w2067) -> (x+y=w2143:dbl)
    n1803 = Subtract(x=w2068, y=w2067) -> (x-y=→"Difference":dbl)
    n1804 = feedback #18(w2089) -> (w2088:dbl[])
    n1805 = Divide(x=w2143, y=2.0) -> (x/y=w2097:dbl)
    "Mean" <- w2097
    n1806 = case shown="True" w2098 {
      tunnel: w2097 -> [_ w2276]
      frame False {
      }
      frame True {
        n1807 = Greater?(x="Lost Tether Alarm Threshold (pN)", y=w2276) -> (0:w2274:bool)
        n1808 = case shown="True" w2274 {
          frame False {
          }
          frame True {
            n1809 = flat-sequence {
              frame #0 {
                # "stop only if saving"
                n1810 = local read "Saving..."() -> (w2289:bool)
                n1811 = And(x=w2289, y="TA Cancel Save?") -> (x .and. y?=w2288:bool)
                n1812 = local write "Stop Saving"(w2288) -> ()
              }
              frame #1 {
                n1813 = case shown="True" "TA Green Off?" {
                  frame False {
                  }
                  frame True {
                    w2292 = FALSE ("Fl. Triggered...")
                    n1814 = local write "Fl. Triggered..."(w2292) -> ()
                    n1815 = property on="Green Laser ON/Interlacing" class="Bool (strict)"("Val(Sgnl)"=w2292) -> ()  [unwired: 2 in, 2 out]
                  }
                }
              }
            }
            n1816 = local read "Time tether formed"() -> (w2283:timestamp)
            n1817 = Get Date/Time In Seconds() -> (seconds since 1Jan1904=w2284:timestamp)
            n1818 = Subtract(x=w2284, y=w2283) -> (x-y=w2282:dbl)
            n1819 = Number To Decimal String(number=w2282) -> (decimal integer string=w2279:string)  [unwired: 1 out]
            n1820 = local read "Messages"() -> (w2286:string)
            n1821 = call <vilib>:"Beep.vi"() -> ()  [unwired: 3 in, 9 out]
            n1822 = Concatenate Strings("Lost tether (" ("Message to add"), w2279, " s)." ("string")) -> (w2281:string)
            n1823 = local write "Tether"(FALSE ("Tether")) -> ()
            n1824 = call "Update messages.vi"("Message to add"=w2281, "Old message string"=w2286) -> ("New message string"=w2285:string)
            n1825 = local write "Messages"(w2285) -> ()
            n1826 = property on="Trap Pos. FB ON" class="Bool (strict)"("Val(Sgnl)"=FALSE ("Value (Signaling)")) -> ()  [unwired: 2 in, 2 out]
          }
        }
      }
    }
    n1827 = Build Array (concatenate)(w2089, w2088) -> (w2087:dbl[])
    n1828 = Split 1D Array(array=w2087, index=w1969) -> (first subarray=w2083:dbl[])  [unwired: 1 out]
    n1829 = feedback-in #18(w2083) -> ()
    n1830 = call-poly <vilib>:"Mean.vi"("X"=w2083) -> ("mean"=w2082:dbl)  [unwired: 1 out]
    "Bead Mean (nm)" <- w2082
    n1831 = Subtract(x=w2083, y=w2082) -> (x-y=w2081:dbl[])
    n1832 = Square(x=w2081) -> (x^2=w2080:dbl[])
    n1833 = call-poly <vilib>:"Mean.vi"("X"=w2080) -> ("mean"=w2079:dbl)  [unwired: 1 out]
    n1834 = Square Root(x=w2079) -> (sqrt(x)=w2078:dbl)
    n1835 = Multiply(x=10.0, y=w2078) -> (x*y=→"RMS (Ang)":dbl)
    n1836 = xnode "Read/Write Control"("FPGA VI Reference In"=w2119, "error in"=w2118) -> ("FPGA VI Reference Out"=w2237:T19, "error out"=w2231:errorcluster, "AI2 Y Sum Set 1"=w2227:i16, "AI2 Y Sum Set 2"=w2226:i16, "AI1 X Set 1"=w2003:fxp<+/-,16,1>, "AI1 X Set 2"=w2002:fxp<+/-,16,1>, "Trap Pos FB Int Signal"=→"Trap Pos FB Int Signal":fxp<+/-,24,9>, "Trap Pos FB Int-Norm Signal"=→"Trap Pos FB Int-Norm Signal":fxp<+/-,16,1>, "Trap Pos FB Action"=w1996:i64, "Scanning"=→"AOD Scanning":bool, "Scan I"=→"AOD Scan I":u64, "Scanning MCL"=w2229:bool, "Scan I (MCL)"=→"MCL Scan I":u64, "Green FB Signals"=w2166:T47)  [unwired: 1 out]
    "MCL Scanning" <- w2229
    "Trap Pos FB Action" <- w1996
    n1837 = local read "AI2 (V)"() -> (w2228:cluster{"Set 1":dbl, "Set 2":dbl})
    n1838 = Bundle By Name(cluster=w2228, "Set 1"=w2227, "Set 2"=w2226) -> (w2224:cluster{"Set 1":dbl, "Set 2":dbl})
    n1839 = Divide(x=w1996, y=327.67) -> (x/y=→"Action (%)":dbl)
    n1840 = local read "Trap X (AI1)"() -> (w2016:T1)
    n1841 = Divide(x=w2224, y=3276.7) -> (x/y=w2223:cluster{"Set 1":dbl, "Set 2":dbl})
    n1842 = local write "AI2 (V)"(w2223) -> ()
    n1843 = Bundle(cluster=w2016, "Trap 1"=w2003, "Trap 2"=w2002) -> (→"Trap X (AI1)":T1)
    n1844 = Divide(x=w2166, y=3276.7) -> (x/y=w2162:T48)
    n1845 = Unbundle By Name(w2162) -> ("Green FB Ch 0"=w2165:dbl, "Green FB Ch 1"=w2164:dbl, "Green FB Ch 2"=w2163:dbl)
    n1846 = Divide(x=w2165, y=w2163) -> (x/y=w2161:dbl)
    n1847 = Divide(x=w2164, y=w2163) -> (x/y=w2160:dbl)
    n1848 = flat-sequence "To save data" {
      tunnel: [w3166] -> w2248
      tunnel: [w3167] -> w2247
      tunnel: w2197 -> [w3160]
      tunnel: w2085 -> [w3164]
      tunnel: ["Save Calibration"] -> w2220
      tunnel: w2217 -> [w3163]
      tunnel: [w3156] -> w2216
      tunnel: [w3153] -> w2215
      tunnel: [w3150] -> w2214
      tunnel: w2196 -> [w3152]
      tunnel: w2102 -> [w3146]
      tunnel: [w3146] -> w2101
      tunnel: ["Start Saving"] -> w2059
      tunnel: [w3140] -> w1985
      tunnel: [w3139] -> w1984
      tunnel: w2248 -> [w3401]
      tunnel: w2247 -> [w3400]
      tunnel: w1986 -> [w3399]
      tunnel: w2220 -> [w3398]
      tunnel: w2216 -> [w3396]
      tunnel: w2215 -> [w3395]
      tunnel: w2214 -> [w3394]
      tunnel: w2072 -> [w3393]
      tunnel: w2111 -> [w3392]
      tunnel: w2101 -> [w3391]
      tunnel: w2059 -> [w3390]
      tunnel: w2057 -> [w3389]
      tunnel: w2033 -> [w3388]
      tunnel: w1985 -> [w3387]
      tunnel: w1984 -> [w3386]
      tunnel: w1983 -> [w3385]
      frame #0 {
        n1849 = Or(x="Save N Sets", y="Start Saving") -> (x .or. y?=w3147:bool)
        n1850 = To Double Precision Float(number=w3163) -> (double precision float=w3157:dbl)
        n1851 = Build Array(w3147, "Save Calibration", w3160, w3152) -> (w3162:bool[])
        n1852 = Compound Arithmetic op=OR("Save Calibration", w3160, w3147, w3152) -> (w3165:bool)
        n1853 = Boolean Array To Number(Boolean array=w3162) -> (number=w3159:u32)
        n1854 = feedback #19(FALSE ("Save APD Data\nwith Trap Data")) -> (w3141:bool)
        n1855 = feedback #20(refnum<k0> refnum) -> (w3168:refnum<file>)
        n1856 = feedback #21(refnum<k0> refnum) -> (w3143:refnum<file>)
        n1857 = feedback #22(FALSE ("Save APD Data\nwith Trap Data")) -> (w3151:bool)
        n1858 = feedback #23(refnum<k0> refnum) -> (w3154:refnum<file>)
        n1859 = feedback #24(0) -> (w3170:i32)
        n1860 = feedback #25() -> (w3158:u32)  [unwired: 1 out]
        n1861 = case shown="False" w3165 {
          tunnel: [w3177 1] -> w3166
          tunnel: w3170 -> [w3179 _]
          tunnel: [w3178 w3197] -> w3167
          tunnel: w3168 -> [w3178 _]
          tunnel: w3164 -> [_ w3217]
          tunnel: w3157 -> [_ w3215]
          tunnel: w3159 -> [_ w3218]
          tunnel: [w3176 w3196] -> w3156
          tunnel: w3158 -> [w3176 _]
          tunnel: [w3175 w3194] -> w3153
          tunnel: w3154 -> [w3175 _]
          tunnel: [w3174 w3193] -> w3150
          tunnel: w3151 -> [w3174 _]
          tunnel: "Start Saving" -> [_ w3191]
          tunnel: w3146 -> [_ w3190]
          tunnel: [w3173 w3181] -> w3139
          tunnel: w3143 -> [w3173 _]
          tunnel: [w3172 w3180] -> w3140
          tunnel: w3141 -> [w3172 _]
          frame False {
            n1862 = Increment(x=w3179) -> (x+1=w3177:i32)
          }
          frame True {
            w3187 = FALSE ("Start Saving")
            w3192 = 9.0  # File Version
            w3200 = FALSE ("prepend array or string size? (T)")
            w3198 = T29."big-endian, network order" ("byte order (0:big-endian, network order)")
            # "write file headers"
            n1863 = local read "BD 1 Frequency 1 (MHz)"() -> (w3214:dbl)
            n1864 = local read "BD 2 Frequency 1 (MHz)"() -> (w3213:dbl)
            n1865 = local read "BD 1 Frequency 2 (MHz)"() -> (w3212:dbl)
            n1866 = local read "BD 2 Frequency 2 (MHz)"() -> (w3211:dbl)
            n1867 = local read "BD 1 Frequency 3 (MHz)"() -> (w3210:dbl)
            n1868 = local read "BD 2 Frequency 3 (MHz)"() -> (w3209:dbl)
            n1869 = Array Size(array=w3190) -> (size(s)=w3189:i32)
            n1870 = To Double Precision Float(number=w3189) -> (double precision float=w3188:dbl)
            n1871 = local write "Save Calibration"(w3187) -> ()
            n1872 = local write "Start Saving"(w3187) -> ()
            n1873 = Build Array("Save APD Data\nwith Trap Data", "Save Trap Pos. Data") -> (w3184:bool[])
            n1874 = Boolean Array To Number(Boolean array=w3184) -> (number=w3183:u32)
            n1875 = Build Array(w3214, w3213, w3212, w3211, w3210, w3209) -> (w3208:dbl[])
            n1876 = case shown="4" w3218 {
              tunnel: w3217 -> [w3289 w3309 w3325 w3363]
              tunnel: w3188 -> [w3294 w3316 w3345 w3382]
              tunnel: w3215 -> [w3293 w3315 w3344 w3381]
              tunnel: [w3290 w3311 w3336 w3373] -> w3206
              tunnel: [w3281 "Cal sets to save" w3326 w3364] -> w3196
              tunnel: w3208 -> [w3291 w3312 w3338 w3375]
              tunnel: "Save APD Data\nwith Trap Data" -> [w3288 _ w3322 w3361]
              tunnel: [w3288 w3303 w3322 w3361] -> w3193
              tunnel: w3192 -> [w3284 w3304 w3320 w3359]
              tunnel: w3191 -> [w3283 _ _ _]
              tunnel: [w3274 w3303 w3319 w3349] -> w3180
              tunnel: "Save Trap Pos. Data" -> [w3274 _ w3319 w3349]
              tunnel: w3183 -> [w3273 _ w3318 w3348]
              frame 1, Default {
                # "timeseries"
                n1877 = case shown="True" "Profile" {
                  tunnel: [w3297 w3300] -> w3278
                  tunnel: [w3297 w3299] -> w3277
                  tunnel: [w3297 w3298] -> w3276
                  tunnel: [w3297 w3302] -> w3275
                  frame False {
                    w3297 = 0.0 ("f")
                  }
                  frame True {
                    n1878 = local read "Current Position"() -> (w3301:dbl[])
                    n1879 = local read "Y change (mm)"() -> (w3302:dbl)
                    n1880 = call "subVI_explode3array.vi"("Array"=w3301) -> ("x"=w3300:dbl, "y"=w3299:dbl, "z"=w3298:dbl)  [unwired: 12 in]
                  }
                }
                n1881 = local read "Save ave N"() -> (w3296:dbl)
                n1882 = Multiply(x=w3296, y=w3289) -> (x*y=w3295:dbl)
                n1883 = To Double Precision Float(number=w3273) -> (double precision float=w3287:dbl)
                n1884 = Build Array(w3284, w3289, w3295, w3294, w3293, 0.0 ("f")) -> (w3292:dbl[])
                n1885 = Build Array(w3287, w3278, w3277, w3276, w3275) -> (w3285:dbl[])
                n1886 = Select(t=u32 4000000000, s=w3283, f="N sets to save") -> (s? t:f=w3281:u32)
                n1887 = Build Array (concatenate)(w3292, w3291, w3285) -> (w3290:dbl[])
              }
              frame 2 {
                w3306 = 0.0 ("f")
                w3303 = FALSE ("Save APD Data\nwith Trap Data")
                # "calibration"
                n1888 = Boolean To (0,1)(Boolean=w3303) -> (0, 1=w3308:i16)
                n1889 = To Double Precision Float(number=w3308) -> (double precision float=w3307:dbl)
                n1890 = Build Array(w3307, w3306, w3306, w3306, w3306) -> (w3305:dbl[])
                n1891 = Build Array(w3304, w3309, w3309, w3316, w3315, 1.0 ("t")) -> (w3313:dbl[])
                n1892 = Build Array (concatenate)(w3313, w3312, w3305) -> (w3311:dbl[])
                "Calibrating Trap..." <- TRUE ("Calibrating...")
              }
              frame 4 {
                w3323 = 0.0 ("f")
                # "write file header for a trap \nraster scan"
                # "scan dir (x/y = 0/1)"
                # "cycles/step"
                # "n scans (f/b)"
                # "steps"
                # "freq. range"
                # "AOD raster scan"
                n1893 = local read "Number of F/B Scans (AOD)"() -> (w3330:u16)
                n1894 = local read "Cycles/step (AOD)"() -> (w3332:u64)
                n1895 = local read "Scan Range (MHz)"() -> (w3335:dbl)
                n1896 = local read "Scan steps (AOD)"() -> (w3334:u64)
                n1897 = local read "Scan BD"() -> (w3342:bool)
                n1898 = local read "Save ave N"() -> (w3347:dbl)
                n1899 = Boolean To (0,1)(Boolean=w3342) -> (0, 1=w3341:i16)
                n1900 = To Double Precision Float(number=w3330) -> (double precision float=w3329:dbl)
                n1901 = To Double Precision Float(number=w3334) -> (double precision float=w3333:dbl)
                n1902 = To Double Precision Float(number=w3332) -> (double precision float=w3331:dbl)
                n1903 = To Double Precision Float(number=w3341) -> (double precision float=w3340:dbl)
                n1904 = Multiply(x=w3347, y=w3325) -> (x*y=w3346:dbl)
                n1905 = To Double Precision Float(number=w3318) -> (double precision float=w3324:dbl)
                n1906 = Build Array(w3324, w3323, w3323, w3323, w3323) -> (w3321:dbl[])
                n1907 = local read "N sets should be saved"() -> (w3327:dbl)
                n1908 = Build Array(w3340, w3335, w3333, w3331, w3329) -> (w3337:dbl[])
                n1909 = Build Array(w3320, w3325, w3346, w3345, w3344, 2.0 ("t")) -> (w3339:dbl[])
                n1910 = Round Toward +Infinity(x=w3327) -> (ceil(x): smallest int >= x=w3328:dbl)
                n1911 = Build Array (concatenate)(w3339, w3338, w3321, w3337) -> (w3336:dbl[])
                n1912 = To Unsigned Long Integer(number=w3328) -> (unsigned 32bit integer=w3326:u32)
              }
              frame 8 {
                w3356 = 0.0 ("f")
                # "MCL raster scan"
                n1913 = local read "Number of scans (MCL)"() -> (w3351:u64)
                n1914 = local read "Scan lines (y)"() -> (w3350:u64)
                n1915 = local read "2D or 1D Scan"() -> (w3353:bool)
                n1916 = local read "Scan Range (V)\n(of steps)"() -> (w3372:dbl)
                n1917 = local read "Fast Scan Dir"() -> (w3379:bool)
                n1918 = local read "Cycles/step (MCL)"() -> (w3369:u64)
                n1919 = local read "Scan steps (MCL)"() -> (w3371:u64)
                n1920 = Select(t=w3350, s=w3353, f=w3351) -> (s? t:f=w3352:u64)
                n1921 = Boolean To (0,1)(Boolean=w3353) -> (0, 1=w3355:i16)
                n1922 = local read "Save ave N"() -> (w3384:dbl)
                n1923 = local read "Initial X"() -> (w3358:dbl)
                n1924 = local read "Initial Y"() -> (w3357:dbl)
                n1925 = To Double Precision Float(number=w3355) -> (double precision float=w3354:dbl)
                n1926 = Boolean To (0,1)(Boolean=w3379) -> (0, 1=w3378:i16)
                n1927 = To Double Precision Float(number=w3352) -> (double precision float=w3367:dbl)
                n1928 = To Double Precision Float(number=w3371) -> (double precision float=w3370:dbl)
                n1929 = To Double Precision Float(number=w3369) -> (double precision float=w3368:dbl)
                n1930 = To Double Precision Float(number=w3378) -> (double precision float=w3377:dbl)
                n1931 = Multiply(x=w3384, y=w3363) -> (x*y=w3383:dbl)
                n1932 = To Double Precision Float(number=w3348) -> (double precision float=w3362:dbl)
                n1933 = local read "N sets should be saved (MCL)"() -> (w3365:dbl)
                n1934 = Build Array(w3362, w3354, w3356, w3356, w3356) -> (w3360:dbl[])
                n1935 = Build Array(w3377, w3372, w3370, w3368, w3367, w3358, w3357) -> (w3374:dbl[])
                n1936 = Build Array(w3359, w3363, w3383, w3382, w3381, 3.0 ("t")) -> (w3376:dbl[])
                n1937 = Round Toward +Infinity(x=w3365) -> (ceil(x): smallest int >= x=w3366:dbl)
                n1938 = Build Array (concatenate)(w3376, w3375, w3360, w3374) -> (w3373:dbl[])
                n1939 = To Unsigned Long Integer(number=w3366) -> (unsigned 32bit integer=w3364:u32)
              }
            }
            n1940 = local read "Index"() -> (w3223:dbl)
            n1941 = call "Create new save file.vi"("Insert"="", "Ext"=".dat", "Index In"=w3223) -> ("Path Out"=w3182:path, "Index Out"=w3195:dbl)
            n1942 = local write "Save file name"(w3182) -> ()
            n1943 = local write "Index"(w3195) -> ()
            n1944 = local write "Save index"(w3195) -> ()
            n1945 = Array Size(array=w3206) -> (size(s)=w3207:i32)
            n1946 = Open/Create/Replace File(file path (use dialog)=w3182, operation (0:open)=T23."create", access (0:read/write)=enum16{"read/write", "read-only", "write-only"}."write-only") -> (refnum out=w3220:refnum<file>)  [unwired: 1 in, 4 out]
            n1947 = local write "Saving..."(TRUE ("Saving...")) -> ()
            n1948 = To Double Precision Float(number=w3207) -> (double precision float=w3205:dbl)
            n1949 = String Length(string="Comment (data description)") -> (length=w3203:i32)
            n1950 = To Double Precision Float(number=w3203) -> (double precision float=w3202:dbl)
            n1951 = Deny Access(7:w3220) -> (3:w3219:refnum<file>)  [unwired: 1 in, 2 out]
            n1952 = Build Array (concatenate)(w3205, w3206, w3202) -> (w3204:dbl[])
            n1953 = case "If fluorescence data to be saved" shown="True" w3193 {
              tunnel: w3182 -> [_ w3272]
              tunnel: [refnum<k0> refnum w3252] -> w3194
              frame False {
              }
              frame True {
                w3251 = 0.0
                n1954 = local read "APD Integration Time (s)"() -> (w3257:dbl)
                n1955 = local read "N APD Samp/step"() -> (w3250:dbl)
                n1956 = Path To String(path=w3272) -> (string=w3271:string)
                n1957 = String Length(string=w3271) -> (length=w3270:i32)
                n1958 = Subtract(x=w3270, y=4) -> (x-y=w3268:i32)
                n1959 = String Subset(string=w3271, length (rest)=w3268) -> (substring=w3267:string)  [unwired: 1 out]
                n1960 = Build Array(w3257, w3250, w3251, w3251, w3251, w3251, w3251, w3251) -> (w3254:dbl[])
                n1961 = Concatenate Strings(w3267, "_fl.dat" ("string")) -> (w3265:string)
                n1962 = Array Size(array=w3254) -> (size(s)=w3256:i32)
                n1963 = String To Path(string=w3265) -> (path=w3261:path)
                n1964 = Open/Create/Replace File(file path (use dialog)=w3261, operation (0:open)=T23."create", access (0:read/write)=enum16{"read/write", "read-only", "write-only"}."write-only") -> (refnum out=w3262:refnum<file>)  [unwired: 1 in, 4 out]
                n1965 = Deny Access(7:w3262) -> (3:w3258:refnum<file>)  [unwired: 1 in, 2 out]
                n1966 = To Double Precision Float(number=w3256) -> (double precision float=w3255:dbl)
                n1967 = Build Array (concatenate)(w3255, w3254) -> (w3253:dbl[])
                n1968 = Write to Binary File(file (use dialog)=w3258, data=w3253, 5:FALSE ("prepend array or string size? (T)"), 9:T29."big-endian, network order" ("byte order (0:big-endian, network order)")) -> (refnum out=w3252:refnum<file>)  [unwired: 1 in, 3 out]
              }
            }
            n1969 = case shown="True" w3180 {
              tunnel: w3182 -> [_ w3234]
              tunnel: [refnum<k0> refnum w3233] -> w3181
              frame False {
              }
              frame True {
                w3229 = 0.0 ("element")
                n1970 = Path To String(path=w3234) -> (string=w3248:string)
                n1971 = Build Array(w3229, w3229, w3229, w3229, w3229, w3229, w3229, w3229) -> (w3230:dbl[])
                n1972 = String Length(string=w3248) -> (length=w3247:i32)
                n1973 = Subtract(x=w3247, y=4) -> (x-y=w3245:i32)
                n1974 = Array Size(array=w3230) -> (size(s)=w3232:i32)
                n1975 = String Subset(string=w3248, length (rest)=w3245) -> (substring=w3244:string)  [unwired: 1 out]
                n1976 = To Double Precision Float(number=w3232) -> (double precision float=w3231:dbl)
                n1977 = Concatenate Strings(w3244, "_pos.dat" ("string")) -> (w3242:string)
                n1978 = Build Array (concatenate)(w3231, w3230) -> (w3228:dbl[])
                n1979 = String To Path(string=w3242) -> (path=w3238:path)
                n1980 = Open/Create/Replace File(file path (use dialog)=w3238, operation (0:open)=T23."create", access (0:read/write)=enum16{"read/write", "read-only", "write-only"}."write-only") -> (refnum out=w3239:refnum<file>)  [unwired: 1 in, 4 out]
                n1981 = Deny Access(7:w3239) -> (3:w3235:refnum<file>)  [unwired: 1 in, 2 out]
                n1982 = Write to Binary File(file (use dialog)=w3235, data=w3228, 5:FALSE ("prepend array or string size? (T)"), 9:T29."big-endian, network order" ("byte order (0:big-endian, network order)")) -> (refnum out=w3233:refnum<file>)  [unwired: 1 in, 3 out]
              }
            }
            n1983 = Write to Binary File(file (use dialog)=w3219, data=w3204, 5:w3200, 9:w3198) -> (refnum out=w3201:refnum<file>)  [unwired: 1 in, 3 out]
            n1984 = Write to Binary File(file (use dialog)=w3201, data="Comment (data description)", 5:w3200, 9:w3198) -> (refnum out=w3197:refnum<file>)  [unwired: 1 in, 3 out]
          }
        }
        n1985 = feedback-in #19(w3140) -> ()
        n1986 = feedback-in #20(w3167) -> ()
        n1987 = feedback-in #21(w3139) -> ()
        n1988 = feedback-in #22(w3150) -> ()
        n1989 = feedback-in #23(w3153) -> ()
        n1990 = feedback-in #24(w3166) -> ()
        n1991 = feedback-in #25(w3156) -> ()
      }
      frame #1 {
        n1992 = local read "Saving..."() -> (w3397:bool)
        n1993 = case shown="True" w3397 {
          tunnel: w3401 -> [_ w3411]
          tunnel: w3400 -> [_ w3425]
          tunnel: w3399 -> [_ w3421]
          tunnel: w3398 -> [_ w3420]
          tunnel: w3396 -> [_ w3419]
          tunnel: w3395 -> [_ w3414]
          tunnel: w3394 -> [_ w3413]
          tunnel: w3393 -> [_ w3412]
          tunnel: w3392 -> [_ w3410]
          tunnel: w3391 -> [_ w3408]
          tunnel: w3390 -> [_ w3407]
          tunnel: w3389 -> [_ w3406]
          tunnel: w3388 -> [_ w3405]
          tunnel: w3387 -> [_ w3404]
          tunnel: w3386 -> [_ w3403]
          tunnel: w3385 -> [_ w3402]
          frame False {
          }
          frame True {
            n1994 = Multiply(x=w3411, y=w3410) -> (x*y=→"Time (s)":dbl)
            n1995 = Less Or Equal?(x=w3411, y=w3419) -> (x <= y?=w3423:bool)
            n1996 = Or(x="Stop Saving", y="Abort save 2") -> (x .or. y?=w3415:bool)
            n1997 = Not(x=w3415) -> (.not. x?=w3424:bool)
            n1998 = And(x=w3423, y=w3424) -> (x .and. y?=w3422:bool)
            n1999 = case shown="False" w3422 {
              tunnel: w3425 -> [w3432 w3500]
              tunnel: [0.0 w3503] -> w3418
              tunnel: w3411 -> [_ w3501]
              tunnel: w3419 -> [_ w3502]
              tunnel: w3421 -> [_ w3497]
              tunnel: w3420 -> [_ _]
              tunnel: w3414 -> [w3430 w3490]
              tunnel: w3413 -> [w3429 w3491]
              tunnel: w3412 -> [_ w3489]
              tunnel: w3408 -> [_ w3488]
              tunnel: w3407 -> [_ w3442]
              tunnel: w3406 -> [_ w3481]
              tunnel: w3405 -> [_ w3459]
              tunnel: w3404 -> [w3427 w3440]
              tunnel: w3403 -> [w3428 w3439]
              tunnel: w3402 -> [_ w3436]
              frame False {
                w3426 = FALSE
                n2000 = Close File(refnum=w3432) -> ()  [unwired: 1 in, 2 out]
                n2001 = case shown="True" w3429 {
                  tunnel: w3430 -> [_ w3434]
                  frame False {
                  }
                  frame True {
                    n2002 = Close File(refnum=w3434) -> ()  [unwired: 1 in, 2 out]
                  }
                }
                n2003 = case shown="True" w3427 {
                  tunnel: w3428 -> [_ w3433]
                  frame False {
                  }
                  frame True {
                    n2004 = Close File(refnum=w3433) -> ()  [unwired: 1 in, 2 out]
                  }
                }
                n2005 = local write "Calibrating Trap..."(w3426) -> ()
                n2006 = call <vilib>:"Beep.vi"() -> ()  [unwired: 3 in, 9 out]
                n2007 = local write "Stop Saving"(w3426) -> ()
                n2008 = property on="Raster Scanning..." class="Bool (strict)"("Val(Sgnl)"=w3426) -> ()  [unwired: 2 in, 2 out]
                "Saving..." <- w3426
              }
              frame True {
                n2009 = local read "Calibrating Trap..."() -> (w3492:bool)
                n2010 = case "Write fl. data" shown="True" w3491 {
                  tunnel: w3490 -> [_ w3526]
                  tunnel: w3489 -> [_ w3525]
                  frame False {
                  }
                  frame True {
                    n2011 = Write to Binary File(file (use dialog)=w3526, data=w3525, 5:FALSE ("prepend array or string size? (T)"), 9:T29."big-endian, network order" ("byte order (0:big-endian, network order)")) -> ()  [unwired: 1 in, 4 out]
                  }
                }
                n2012 = Greater?(x="Save ave N", y=1.0) -> (0:w3495:bool)
                n2013 = Not(x=w3492) -> (.not. x?=w3494:bool)
                n2014 = And(x=w3494, y=w3495) -> (x .and. y?=w3437:bool)
                n2015 = case shown="True" w3437 {
                  tunnel: w3436 -> [w3506 w3517]
                  tunnel: [w3506 w3509] -> w3435
                  tunnel: "Save ave N" -> [_ w3510]
                  frame False {
                  }
                  frame True {
                    w3507 = 2 ("dimension size")
                    n2016 = Array Size(array=w3517) -> (size(s)=w3511:i32)
                    n2017 = Divide(x=w3511, y=w3507) -> (x/y=w3515:dbl)
                    n2018 = Reshape Array(w3517, w3515, w3507) -> (w3516:u64[][])
                    n2019 = Transpose 2D Array(2D array=w3516) -> (transposed array=w3514:u64[][])
                    n2020 = for {
                      tunnel: w3514 -> [w3519] mode=indexing
                      tunnel: [w3518] -> w3508 mode=indexing
                      tunnel: w3510 -> [w3520]
                      workers-P: _ -> [_]
                      n2021 = call "downsample 1D array - U64.vi"("Ave N"=w3520, "Array In"=w3519) -> ("Array Out"=w3518:u64[])  [unwired: 1 in]
                    }
                    n2022 = Transpose 2D Array(2D array=w3508) -> (transposed array=w3513:u64[][])
                    n2023 = Divide(x=w3511, y=w3510) -> (x/y=w3512:dbl)
                    n2024 = Reshape Array(w3513, w3512) -> (w3509:u64[])
                  }
                }
                n2025 = case shown="True" w3437 {
                  tunnel: w3497 -> [w3529 w3541]
                  tunnel: [w3529 w3533] -> w3493
                  tunnel: "Save ave N" -> [_ w3534]
                  tunnel: w3488 -> [_ w3532]
                  frame False {
                    # "don't downsample data for trap calibration"
                  }
                  frame True {
                    n2026 = Array Size(array=w3541) -> (size(s)=w3535:i32)
                    n2027 = Array Size(array=w3532) -> (size(s)=w3531:i32)
                    n2028 = Divide(x=w3535, y=w3531) -> (x/y=w3539:dbl)
                    n2029 = Reshape Array(w3541, w3539, w3531) -> (w3540:i16[][])
                    n2030 = Transpose 2D Array(2D array=w3540) -> (transposed array=w3538:i16[][])
                    n2031 = for {
                      tunnel: w3538 -> [w3544] mode=indexing
                      tunnel: [w3543] -> w3530 mode=indexing
                      tunnel: w3534 -> [w3542]
                      workers-P: _ -> [_]
                      n2032 = call "downsample 1D array - I16.vi"("Ave N"=w3542, "Array In"=w3544) -> ("Array Out"=w3543:i16[])  [unwired: 1 out]
                    }
                    n2033 = Transpose 2D Array(2D array=w3530) -> (transposed array=w3537:i16[][])
                    n2034 = Divide(x=w3535, y=w3534) -> (x/y=w3536:dbl)
                    n2035 = Reshape Array(w3537, w3536) -> (w3533:i16[])
                  }
                }
                n2036 = Index Array(array=w3459, index=1) -> (element=w3462:waveform(dbl))
                n2037 = Index Array(array=w3459, index=0) -> (element=w3464:waveform(dbl))
                n2038 = Unbundle By Name(w3462) -> ("Y"=w3466:dbl[])
                n2039 = Unbundle By Name(w3464) -> ("Y"=w3474:dbl[])
                n2040 = case "Write trap pos. data" shown="True" w3440 {
                  tunnel: w3439 -> [_ w3522]
                  tunnel: w3435 -> [_ w3521]
                  frame False {
                  }
                  frame True {
                    n2041 = Write to Binary File(file (use dialog)=w3522, data=w3521, 5:FALSE ("prepend array or string size? (T)"), 9:T29."big-endian, network order" ("byte order (0:big-endian, network order)")) -> ()  [unwired: 1 in, 4 out]
                  }
                }
                n2042 = Write to Binary File(file (use dialog)=w3500, data=w3493, 5:FALSE ("prepend array or string size? (T)"), 9:T29."big-endian, network order" ("byte order (0:big-endian, network order)")) -> ()  [unwired: 1 in, 4 out]
                n2043 = feedback #26(w3466) -> (w3468:dbl[])
                n2044 = Build Array (concatenate)(w3468, w3466) -> (w3467:dbl[])
                n2045 = Select(t=w3466, s=w3442, f=w3467) -> (s? t:f=w3452:dbl[])
                n2046 = feedback-in #26(w3452) -> ()
                n2047 = feedback #27(w3474) -> (w3487:dbl[])
                n2048 = Build Array (concatenate)(w3487, w3474) -> (w3486:dbl[])
                n2049 = Select(t=w3474, s=w3442, f=w3486) -> (s? t:f=w3461:dbl[])
                n2050 = feedback-in #27(w3461) -> ()
                n2051 = Divide(x=w3501, y=w3502) -> (x/y=w3504:dbl)
                n2052 = Multiply(x=w3504, y=100.0) -> (x*y=w3503:dbl)
                n2053 = Build Array(w3461, w3452) -> (→"Saved APD":dbl[][])
                n2054 = Array Size(array=w3461) -> (size(s)=w3479:i32)
                n2055 = Unbundle By Name(w3481) -> ("Y"=w3485:dbl[])
                n2056 = Subtract(x=w3479, y="N pts to average") -> (x-y=w3455:i32)
                n2057 = Multiply(x="N pts to average", y=u16 2) -> (x*y=w3456:u16)
                n2058 = Subtract(x=w3479, y=w3456) -> (x-y=w3454:i32)
                n2059 = feedback #28(w3485) -> (w3484:dbl[])
                n2060 = Build Array (concatenate)(w3484, w3485) -> (w3483:dbl[])
                n2061 = Select(t=w3485, s=w3442, f=w3483) -> (s? t:f=w3482:dbl[])
                "Trap Delta Graph" <- w3482
                n2062 = feedback-in #28(w3482) -> ()
                n2063 = Array Subset(array=w3461, index=w3455, length="N pts to average") -> (w3478:dbl[])
                n2064 = Array Subset(array=w3461, index=w3454, length="N pts to average") -> (w3477:dbl[])
                n2065 = Array Subset(array=w3452, index=w3455, length="N pts to average") -> (w3458:dbl[])
                n2066 = Array Subset(array=w3452, index=w3454, length="N pts to average") -> (w3457:dbl[])
                n2067 = call-poly <vilib>:"Mean.vi"("X"=w3478) -> ("mean"=w3476:dbl)  [unwired: 1 out]
                n2068 = call-poly <vilib>:"Mean.vi"("X"=w3458) -> ("mean"=w3451:dbl)  [unwired: 1 out]
                n2069 = call-poly <vilib>:"Mean.vi"("X"=w3477) -> ("mean"=w3475:dbl)  [unwired: 1 out]
                n2070 = call-poly <vilib>:"Mean.vi"("X"=w3457) -> ("mean"=w3450:dbl)  [unwired: 1 out]
                n2071 = Subtract(x=w3451, y=w3450) -> (x-y=w3441:dbl)
                "Delta Fl. 2" <- w3441
                n2072 = Subtract(x=w3476, y=w3475) -> (x-y=w3473:dbl)
                "Delta Fl. 1" <- w3473
                n2073 = Initialize Array(w3473, 1 ("dimension size")) -> (w3470:dbl[])
                n2074 = Initialize Array(w3441, 1 ("dimension size")) -> (w3447:dbl[])
                n2075 = feedback #29(w3470) -> (w3471:dbl[])
                n2076 = Build Array (concatenate)(w3471, w3470) -> (w3469:dbl[])
                n2077 = feedback #30(w3447) -> (w3448:dbl[])
                n2078 = Build Array (concatenate)(w3448, w3447) -> (w3446:dbl[])
                n2079 = Select(t=w3470, s=w3442, f=w3469) -> (s? t:f=w3445:dbl[])
                n2080 = feedback-in #29(w3445) -> ()
                n2081 = Select(t=w3447, s=w3442, f=w3446) -> (s? t:f=w3444:dbl[])
                n2082 = feedback-in #30(w3444) -> ()
                n2083 = Build Array(w3445, w3444) -> (→"Save APD Deriv":dbl[][])
              }
            }
            "Progress" <- w3418
            "Progress 2" <- w3418
          }
        }
      }
    }
    n2084 = Bundle By Name(cluster=w2162, "Green FB Ch 0"=w2161, "Green FB Ch 1"=w2160) -> (w2140:T48)
    "Green FB Signals (V)" <- w2140
    n2085 = Unbundle By Name(w2140) -> ("Green FB Ch 2"=→"Green FB Plot":dbl)
    n2086 = local read "wait to reset values"() -> (w2232:bool)
    n2087 = Not(x=w2229) -> (.not. x?=w2233:bool)
    n2088 = And(x=w2233, y=w2232) -> (x .and. y?=w2234:bool)
    n2089 = case "Part of MCL raster scanning: returns to initial positions after scan done" shown="False" w2234 {
      tunnel: w2237 -> [w2970 w2977]
      tunnel: [w2970 w2976] -> w2236
      tunnel: w2231 -> [w2969 w2975]
      tunnel: [w2969 w2974] -> w2230
      frame False {
      }
      frame True {
        w2985 = 10.0 ("y")
        w2984 = 32767.0 ("y")
        # "to return scan values\nafter a synchronous \nAOM scan"
        n2090 = local read "AO2"() -> (w2978:dbl)
        n2091 = local read "AO1"() -> (w2979:dbl)
        n2092 = local write "wait to reset values"(FALSE ("wait to reset values")) -> ()
        n2093 = Multiply(x=w2979, y=w2984) -> (x*y=w2981:dbl)
        n2094 = Multiply(x=w2978, y=w2984) -> (x*y=w2983:dbl)
        n2095 = Divide(x=w2981, y=w2985) -> (x/y=w2980:dbl)
        n2096 = Divide(x=w2983, y=w2985) -> (x/y=w2982:dbl)
        n2097 = To Word Integer(number=w2980) -> (16bit integer=w2986:i16)
        n2098 = To Word Integer(number=w2982) -> (16bit integer=w2987:i16)
        n2099 = local read "Total Counts (ticks)"() -> (w2971:u32)
        n2100 = xnode "Read/Write Control"("FPGA VI Reference In"=w2977, "error in"=w2975, "AO1"=w2986, "AO2"=w2987, "MCL count"=w2971) -> ("FPGA VI Reference Out"=w2976:T19, "error out"=w2974:errorcluster)
        n2101 = local read "Scan Range (V)\n(of steps)"() -> (w2972:dbl)
        n2102 = property on="Scan Range (V)\n(of steps)" class="DigNum (strict)"("Val(Sgnl)"=w2972) -> ()  [unwired: 2 in, 2 out]
      }
    }
    n2103 = node-c288() -> ()  [unwired: 2 out]
  }
  n2104 = node-c288(3 ("Processor")) -> (w74:T24)  [unwired: 3 out]
  n2105 = timed-loop "Oscillate AOD (debugging)" {
    tunnel: w24 -> [w3546]
    tunnel: [w3545] -> w36
    timing: w74 -> [_]
    timing-out: [_] -> w73
    stop <- w3545 stop-if-true
    n2106 = node-c288() -> ()  [unwired: 2 out]
    n2107 = event shown="[0] \"Oscillate Set 2\", \"Fish for Tether\": Value Change" {
      selector: _ -> [_ _ _]
      dyn-events: _ -> [_ _ _]
      timeout: _ -> [_ _ _]
      tunnel: w3546 -> [w3553 _ _]
      tunnel: [FALSE ("Stop All") _ w3821] -> w3545
      event "Oscillate Set 2", "Fish for Tether": Value Change {
        n2108 = event-data() -> ()  [unwired: 6 out]
        n2109 = local read "Oscillate Set 2"() -> (w3552:bool)
        n2110 = Or(x=w3552, y="Fish for Tether") -> (x .or. y?=w3550:bool)
        n2111 = case shown="True" w3550 {
          tunnel: w3553 -> [_ w3556]
          tunnel: "Fish for Tether" -> [_ w3555]
          frame False {
          }
          frame True {
            n2112 = case shown="True" w3555 {
              frame False {
              }
              frame True {
                n2113 = local write "Scan axis 2"(TRUE) -> ()
                n2114 = local write "Tether"(FALSE ("Tether")) -> ()
              }
            }
            n2115 = node-c288("Period") -> (w3558:T24)  [unwired: 3 out]
            n2116 = timed-loop "Oscillate AOD" {
              timing: w3558 -> [_]
              timing-out: [_] -> w3557
              tunnel: w3556 -> [w3568]
              tunnel: w3555 -> [w3567]
              i -> [w3570]
              stop <- w3566 stop-if-true
              n2117 = node-c288() -> (w3569:i64)  [unwired: 1 out]
              n2118 = flat-sequence {
                tunnel: w3570 -> [w3596]
                tunnel: w3569 -> [w3595]
                tunnel: w3568 -> [w3579]
                tunnel: w3567 -> [w3581]
                tunnel: [w3581] -> w3565
                tunnel: [w3580] -> w3564
                tunnel: [w3578] -> w3563
                tunnel: [w3575] -> w3561
                tunnel: w3565 -> [w3632]
                tunnel: w3564 -> [w3630]
                tunnel: w3563 -> [w3629]
                tunnel: [w3628] -> w3562
                tunnel: w3561 -> [w3627]
                tunnel: [w3696] -> w3566
                tunnel: w3562 -> [w3694]
                frame #0 {
                  n2119 = Divide(x=w3595, y=i64 1000) -> (x/y=w3590:dbl)
                  n2120 = Multiply(x=w3590, y=w3596) -> (x*y=w3592:dbl)
                  n2121 = Multiply(x="Osc. freq. (Hz)", y=6.283185307179586) -> (x*y=w3593:dbl)
                  n2122 = Multiply(x=w3593, y=w3592) -> (x*y=w3577:dbl)
                  n2123 = local read "BD 1 Frequency 2 (MHz)"() -> (w3574:dbl)
                  n2124 = local read "BD 1 Frequency 1 (MHz)"() -> (w3571:dbl)
                  n2125 = case shown="True" w3581 {
                    tunnel: w3577 -> [w3602 w3609]
                    tunnel: w3574 -> [_ w3619]
                    tunnel: [w3599 w3603] -> w3582
                    tunnel: [FALSE w3612] -> w3578
                    tunnel: [0.0 w3605] -> w3575
                    tunnel: w3571 -> [_ w3604]
                    frame False {
                      n2126 = Sine(x=w3602) -> (sin(x)=w3600:dbl)
                      n2127 = Multiply(x=w3600, y="Osc. amp. (MHz)") -> (x*y=w3599:dbl)
                    }
                    frame True {
                      n2128 = Cosine(x=w3609) -> (cos(x)=w3622:dbl)
                      n2129 = Subtract(x=w3619, y=w3604) -> (x-y=w3618:dbl)
                      n2130 = Decrement(x=w3622) -> (x-1=w3621:dbl)
                      n2131 = Subtract(x=w3618, y="Closest Delta (MHz)") -> (x-y=w3615:dbl)
                      n2132 = Divide(x=w3621, y=2.0) -> (x/y=w3616:dbl)
                      n2133 = Multiply(x=w3616, y=w3615) -> (x*y=w3603:dbl)
                      n2134 = local read "Vec Mean of T1 T2"() -> (w3611:dbl[])
                      n2135 = Greater?(x=w3611, y="Stop F (pN)") -> (0:w3613:bool[])
                      n2136 = Or Array Elements(Boolean array=w3613) -> (logical OR=w3612:bool)
                      n2137 = Divide(x=w3609, y=6.283185307179586) -> (x/y=w3608:dbl)
                      n2138 = Round Toward +Infinity(x=w3608) -> (ceil(x): smallest int >= x=w3605:dbl)
                      "Attempts" <- w3605
                      n2139 = Greater?(x=w3605, y="Attempt Limit") -> (0:w3607:bool)
                      n2140 = case shown="True" w3607 {
                        frame False {
                        }
                        frame True {
                          n2141 = local write "Fish for Tether"(FALSE ("Fish for Tether")) -> ()
                          n2142 = call <vilib>:"Beep.vi"() -> ()  [unwired: 3 in, 9 out]
                          n2143 = local read "Messages"() -> (w3624:string)
                          n2144 = call "Update messages.vi"("Message to add"="Tether fishing timeout." ("Messages"), "Old message string"=w3624) -> ("New message string"=→"Messages":string)
                        }
                      }
                    }
                  }
                  n2145 = local read "Y RF Frequency Limits (MHz)"() -> (w3583:T16)
                  n2146 = local read "X RF Frequency Limits (MHz)"() -> (w3584:T16)
                  n2147 = local read "BD 1 Frequency 3 (MHz)"() -> (w3589:dbl)
                  n2148 = local read "BD 2 Frequency 2 (MHz)"() -> (w3573:dbl)
                  n2149 = Select(t=w3574, s="Scan axis 2", f=w3573) -> (s? t:f=w3585:dbl)
                  n2150 = Add(x=w3582, y=w3585) -> (x+y=w3580:dbl)
                  n2151 = Select(t=w3580, s="Scan axis 2", f=w3574) -> (s? t:f=w3572:dbl)
                  n2152 = Select(t=w3573, s="Scan axis 2", f=w3580) -> (s? t:f=w3587:dbl)
                  n2153 = local read "BD 2 Frequency 3 (MHz)"() -> (w3588:dbl)
                  n2154 = call "set RF board frequency - interlace.vi"("Board 2 Frequency Limits"=w3583, "Board 1 Frequency Limits"=w3584, "FPGA VI Reference In"=w3579, "Board 2 Frequency 3 (MHz)"=w3588, "Board 1 Frequency 3 (MHz)"=w3589, "Board 2 Frequency 2 (MHz)"=w3573, "Board 2 Frequency 1 (MHz)"=w3587, "Board 1 Frequency 2 (MHz)"=w3572, "Board 1 Frequency 1  (MHz)"=w3571) -> ()  [unwired: 1 in, 2 out]
                }
                frame #1 {
                  n2155 = And(x=w3632, y=w3629) -> (x .and. y?=w3631:bool)
                  n2156 = case "Only if were fishing and now formed tether" shown="True" w3631 {
                    tunnel: w3630 -> [w3634 w3646]
                    tunnel: [w3633 w3645] -> w3628
                    tunnel: w3627 -> [_ w3641]
                    frame False {
                      n2157 = local read "Fish for Tether"() -> (w3633:bool)
                      n2158 = case shown="True" w3633 {
                        tunnel: w3634 -> [_ _]
                        frame False {
                        }
                        frame True {
                        }
                      }
                    }
                    frame True {
                      w3645 = FALSE ("Fish for Tether")
                      n2159 = call <vilib>:"Beep.vi"() -> ()  [unwired: 3 in, 9 out]
                      n2160 = Number To Decimal String(number=w3641, width (-)=i16 1) -> (decimal integer string=w3639:string)
                      n2161 = case shown="\"2\", \"3\", \"4\", \"5\", \"6\"" "Then..." {
                        selector: "Then..." -> [_ w3649]
                        tunnel: w3646 -> [w3648 _]
                        frame "1", Default {
                          # "do nothing"
                          n2162 = property on="BD 1 Frequency 1 (MHz)" class="DigNum (strict)"("Val(Sgnl)"=w3648) -> ()  [unwired: 2 in, 2 out]
                        }
                        frame "2", "3", "4", "5", "6" {
                          n2163 = flat-sequence {
                            tunnel: w3649 -> [w3651]
                            frame #0 {
                              n2164 = property on="Trap Delta (MHz)" class="Slide (strict)"("Val(Sgnl)"="Move to Delta 1 (MHz)") -> ()  [unwired: 2 in, 2 out]
                            }
                            frame #1 {
                              n2165 = case shown="\"3\", \"4\"" w3651 {
                                selector: w3651 -> [w3654 w3664 _]
                                frame "3", "4" {
                                n2166 = flat-sequence {
                                tunnel: w3654 -> [w3655]
                                tunnel: [w3655] -> w3652
                                tunnel: [w3657] -> w3653
                                tunnel: w3652 -> [w3657]
                                tunnel: w3653 -> [w3661]
                                frame #0 {
                                n2167 = property on="Green Laser ON/Interlacing" class="Bool (strict)"("Val(Sgnl)"=TRUE ("Value (Signaling)")) -> ()  [unwired: 2 in, 2 out]
                                }
                                frame #1 {
                                n2168 = Multiply(x="Wait Before Save (s)", y=u32 1000 ("x")) -> (x*y=w3659:u32)
                                n2169 = Wait (ms)(milliseconds to wait=w3659) -> ()  [unwired: 1 out]
                                }
                                frame #2 {
                                n2170 = property on="Start Saving" class="Bool (strict)"("Value"=TRUE ("Start Saving")) -> ()  [unwired: 2 in, 2 out]
                                n2171 = case shown="Default" w3661 {
                                frame Default {
                                }
                                frame "4" {
                                n2172 = property on="Fl. Triggered..." class="Bool (strict)"("Val(Sgnl)"=TRUE ("Value (Signaling)")) -> ()  [unwired: 2 in, 2 out]
                                }
                                }
                                }
                                }
                                }
                                frame "5", "6" {
                                n2173 = stacked-sequence {
                                tunnel: w3664 -> [_ _ _ _ _ _ _ _ w3681 _ _]
                                frame #0 {
                                n2174 = Replace Array Subset(array=u32[] [0] ("Index Values"), new element="Raster Set Upon Tether", index=0) -> (w3665:u32[])
                                n2175 = property on="Saved AOD Raster Scan Parameter Sets" class="Arr (strict)"("Index Values"=w3665) -> ()  [unwired: 2 in, 2 out]
                                }
                                frame #1 {
                                n2176 = Wait (ms)(milliseconds to wait=u32 500) -> ()  [unwired: 1 out]
                                }
                                frame #2 {
                                n2177 = property on="Load parameters" class="Bool (strict)"("Val(Sgnl)"=TRUE ("Value (Signaling)")) -> ()  [unwired: 2 in, 2 out]
                                }
                                frame #3 {
                                n2178 = Wait (ms)(milliseconds to wait=u32 500) -> ()  [unwired: 1 out]
                                }
                                frame #4 {
                                n2179 = property on="Trap Raster Scan" class="Bool (strict)"("Val(Sgnl)"=TRUE ("Value (Signaling)")) -> ()  [unwired: 2 in, 2 out]
                                }
                                frame #5 {
                                n2180 = Wait (ms)(milliseconds to wait=u32 2000) -> ()  [unwired: 1 out]
                                }
                                frame #6 {
                                n2181 = while {
                                stop <- w3676 stop-if-true
                                n2182 = local read "Raster Scanning..."() -> (w3675:bool)
                                n2183 = local read "Saving..."() -> (w3678:bool)
                                n2184 = Wait (ms)(milliseconds to wait=u32 100) -> ()  [unwired: 1 out]
                                n2185 = Not(x=w3678) -> (.not. x?=w3677:bool)
                                n2186 = Not(x=w3675) -> (.not. x?=w3674:bool)
                                n2187 = And(x=w3677, y=w3674) -> (x .and. y?=w3676:bool)
                                }
                                }
                                frame #7 {
                                n2188 = property on="Trap Delta (MHz)" class="Slide (strict)"("Val(Sgnl)"="Move to Delta 2 (MHz)") -> ()  [unwired: 2 in, 2 out]
                                }
                                frame #8 {
                                n2189 = local read "Tether"() -> (w3682:bool)
                                n2190 = case shown="True" w3682 {
                                tunnel: w3681 -> [_ w3683]
                                frame False {
                                }
                                frame True {
                                n2191 = flat-sequence {
                                tunnel: w3683 -> [w3685]
                                frame #0 {
                                n2192 = Wait (ms)(milliseconds to wait=u32 500) -> ()  [unwired: 1 out]
                                }
                                frame #1 {
                                n2193 = case shown="\"6\"" w3685 {
                                frame Default {
                                }
                                frame "6" {
                                n2194 = property on="Green Laser ON/Interlacing" class="Bool (strict)"("Val(Sgnl)"=TRUE ("Green Laser ON/Interlacing")) -> ()  [unwired: 2 in, 2 out]
                                }
                                }
                                }
                                frame #2 {
                                n2195 = Wait (ms)(milliseconds to wait=u32 500) -> ()  [unwired: 1 out]
                                }
                                frame #3 {
                                n2196 = local write "Start Saving"("Save at end (5, 6)") -> ()
                                }
                                }
                                }
                                }
                                }
                                frame #9 {
                                n2197 = local read "Bead Sep. Int. Time (s)"() -> (w3691:dbl)
                                n2198 = Multiply(x=w3691, y=1000.0) -> (x*y=w3690:dbl)
                                n2199 = Wait (ms)(milliseconds to wait=w3690) -> ()  [unwired: 1 out]
                                }
                                frame #10 {
                                n2200 = property on="Rescale on Mean" class="Bool (strict)"("Val(Sgnl)"=TRUE ("Value (Signaling)")) -> ()  [unwired: 2 in, 2 out]
                                }
                                }
                                }
                                frame "2", Default {
                                }
                              }
                            }
                          }
                        }
                      }
                      n2201 = Concatenate Strings("Formed tether in ", w3639, " attempt(s)." ("string")) -> (w3636:string)
                      n2202 = local read "Messages"() -> (w3643:string)
                      n2203 = local write "Fish for Tether"(w3645) -> ()
                      n2204 = call "Update messages.vi"("Message to add"=w3636, "Old message string"=w3643) -> ("New message string"=w3642:string)
                      n2205 = local write "Messages"(w3642) -> ()
                      n2206 = Get Date/Time In Seconds() -> (seconds since 1Jan1904=→"Time tether formed":timestamp)
                      "Tether" <- "Tether Alarm?"
                    }
                  }
                }
                frame #2 {
                  n2207 = local read "Oscillate Set 2"() -> (w3695:bool)
                  n2208 = local read "Stop All"() -> (w3697:bool)
                  n2209 = Not Or(1:w3694, 2:w3695) -> (0:w3693:bool)
                  n2210 = Compound Arithmetic op=OR(w3697, w3693) -> (w3696:bool)
                }
              }
              n2211 = node-c288() -> ()  [unwired: 2 out]
            }
            n2212 = node-c288(w3557) -> ()  [unwired: 1 out]
          }
        }
      }
      event "Fl. Triggered...": Value Change {
        n2213 = event-data() -> ()  [unwired: 7 out]
        n2214 = case shown="True" "Fl. Triggered..." {
          frame False {
          }
          frame True {
            n2215 = node-c288() -> (w3709:T24)  [unwired: 4 out]
            n2216 = timed-loop {
              timing: w3709 -> [_]
              timing-out: [_] -> w3708
              tunnel: "Action" -> [w3713]
              shift-right: [w3710] -> _
              shift-left: u8 255 -> [w3712]
              stop <- w3714 stop-if-true
              n2217 = node-c288() -> ()  [unwired: 2 out]
              n2218 = flat-sequence {
                tunnel: w3713 -> [w3726]
                tunnel: w3712 -> [w3723]
                tunnel: [w3722] -> w3711
                tunnel: [w3812] -> w3714
                tunnel: w3711 -> [w3811]
                tunnel: [w3811] -> w3710
                frame #0 {
                  n2219 = local read "Delta Fl. 2"() -> (w3717:dbl)
                  n2220 = local read "Delta Fl. 1"() -> (w3718:dbl)
                  n2221 = Select(t=w3718, s="APD to Watch", f=w3717) -> (s? t:f=w3716:dbl)
                  n2222 = Multiply(x="Fl. Delta Thresh. (kHz)", y=1000.0) -> (x*y=w3725:dbl)
                  n2223 = Greater?(x=w3716, y=w3725) -> (0:w3720:bool)
                  n2224 = Or(x="Force Yank", y=w3720) -> (x .or. y?=w3721:bool)
                  n2225 = case shown="True" w3721 {
                    tunnel: w3726 -> [_ w3736]
                    tunnel: w3723 -> [w3728 w3732]
                    tunnel: [w3728 w3729] -> w3722
                    frame False {
                    }
                    frame True {
                      n2226 = flat-sequence {
                        tunnel: w3733 -> [w3742]
                        tunnel: [w3742] -> w3737
                        tunnel: w3736 -> [w3741]
                        tunnel: [w3741] -> w3735
                        tunnel: [w3740] -> w3734
                        tunnel: w3732 -> [w3739]
                        tunnel: [w3738] -> w3731
                        tunnel: w3737 -> [w3767]
                        tunnel: w3735 -> [w3766]
                        tunnel: w3734 -> [w3765]
                        tunnel: w3731 -> [w3764]
                        tunnel: [w3764] -> w3730
                        tunnel: w3730 -> [w3809]
                        tunnel: [w3809] -> w3729
                        frame #0 {
                          n2227 = call <vilib>:"Beep.vi"() -> ()  [unwired: 3 in, 9 out]
                          n2228 = local write "Waiting"(FALSE ("Waiting")) -> ()
                          n2229 = Increment(x=w3739) -> (x+1=w3738:u8)
                          n2230 = case shown="\"Yank\"" w3741 {
                            tunnel: w3738 -> [_ _ w3748]
                            frame "Image" {
                              n2231 = property on="Confocal Image" class="Bool (strict)"("Val(Sgnl)"=TRUE ("Value (Signaling)")) -> ()  [unwired: 2 in, 2 out]
                            }
                            frame "Alarm", Default {
                            }
                            frame "Yank" {
                              n2232 = flat-sequence {
                                tunnel: w3748 -> [w3751]
                                tunnel: [w3750] -> w3747
                                tunnel: ["N Array El"] -> w3746
                                tunnel: w3747 -> [w3761]
                                tunnel: w3746 -> [w3757]
                                frame #0 {
                                n2233 = Multiply(x="Yank Delay (s)", y=1000.0) -> (x*y=w3754:dbl)
                                n2234 = Quotient & Remainder(x=w3751, y="N Array El") -> (x-y*floor(x/y)=w3750:u8)  [unwired: 1 out]
                                n2235 = Wait (ms)(milliseconds to wait=w3754) -> ()  [unwired: 1 out]
                                }
                                frame #1 {
                                n2236 = Random Number (0-1)() -> (number: 0 to 1=w3758:dbl)
                                n2237 = Multiply(x=w3757, y=w3758) -> (x*y=w3756:dbl)
                                n2238 = Round Toward -Infinity(1:w3756) -> (0:w3755:dbl)
                                n2239 = Select(t=w3755, s="Random Choice", f=w3761) -> (s? t:f=w3759:dbl)
                                n2240 = Index Array(array="Yank to Delta Array (MHz)", index=w3759) -> (element=w3762:dbl)
                                n2241 = property on="Trap Delta (MHz)" class="Slide (strict)"("Val(Sgnl)"=w3762) -> ()  [unwired: 2 in, 2 out]
                                }
                              }
                            }
                          }
                          n2242 = local read "Time (s)"() -> (w3740:dbl)
                          "Fl. High" <- TRUE ("Yanking")
                        }
                        frame #1 {
                          n2243 = node-c288() -> (w3769:T24)  [unwired: 4 out]
                          n2244 = timed-loop {
                            timing: w3769 -> [_]
                            timing-out: [_] -> w3768
                            tunnel: w3767 -> [w3785]
                            tunnel: w3766 -> [w3783]
                            tunnel: w3765 -> [w3782]
                            stop <- w3784 stop-if-true
                            n2245 = node-c288() -> ()  [unwired: 2 out]
                            n2246 = local read "Fl. Delta Thresh. (kHz)"() -> (w3777:dbl)
                            n2247 = local read "Fl. Triggered..."() -> (w3786:bool)
                            n2248 = local read "Delta Fl. 1"() -> (w3773:dbl)
                            n2249 = local read "Delta Fl. 2"() -> (w3771:dbl)
                            n2250 = local read "Stop All"() -> (w3780:bool)
                            n2251 = local read "APD to Watch"() -> (w3772:bool)
                            n2252 = Select(t=w3773, s=w3772, f=w3771) -> (s? t:f=w3770:dbl)
                            n2253 = Not(x=w3786) -> (.not. x?=w3781:bool)
                            n2254 = Multiply(x=w3777, y=1000.0) -> (x*y=w3776:dbl)
                            n2255 = Negate(x=w3776) -> (-x=w3775:dbl)
                            n2256 = Less?(x=w3770, y=w3775) -> (x < y?=w3779:bool)
                            n2257 = Compound Arithmetic op=OR(w3779, w3780, w3781, "Force Reset") -> (w3784:bool)
                            n2258 = case shown="True" w3784 {
                              tunnel: w3785 -> [_ w3797]
                              tunnel: w3783 -> [_ w3796]
                              tunnel: w3782 -> [_ w3794]
                              frame False {
                              }
                              frame True {
                                n2259 = case shown="\"Yank\"" w3796 {
                                tunnel: w3797 -> [_ w3798]
                                frame "Image", Default {
                                }
                                frame "Yank" {
                                n2260 = flat-sequence {
                                tunnel: [w3803] -> w3799
                                tunnel: w3798 -> [w3803]
                                tunnel: w3799 -> [w3804]
                                frame #0 {
                                n2261 = local read "Yank Delay (s)"() -> (w3802:dbl)
                                n2262 = Multiply(x=w3802, y=1000.0) -> (x*y=w3800:dbl)
                                n2263 = Wait (ms)(milliseconds to wait=w3800) -> ()  [unwired: 1 out]
                                }
                                frame #1 {
                                n2264 = property on="Trap Delta (MHz)" class="Slide (strict)"("Val(Sgnl)"=w3804) -> ()  [unwired: 2 in, 2 out]
                                }
                                }
                                }
                                }
                                n2265 = local read "Time (s)"() -> (w3795:dbl)
                                n2266 = Subtract(x=w3795, y=w3794) -> (x-y=w3791:dbl)
                                "Duration (s)" <- w3791
                                n2267 = Number To Decimal String(number=w3791, width (-)=i16 0) -> (decimal integer string=w3789:string)
                                n2268 = Concatenate Strings(w3789, " s fluorescence event." ("string")) -> (w3787:string)
                                n2269 = local read "Messages"() -> (w3793:string)
                                n2270 = call "Update messages.vi"("Message to add"=w3787, "Old message string"=w3793) -> ("New message string"=w3792:string)
                                n2271 = call <vilib>:"Beep.vi"() -> ()  [unwired: 3 in, 9 out]
                                n2272 = local write "Messages"(w3792) -> ()
                              }
                            }
                            n2273 = node-c288() -> ()  [unwired: 2 out]
                          }
                          n2274 = node-c288(w3768) -> ()  [unwired: 1 out]
                        }
                        frame #2 {
                          n2275 = local write "Fl. High"(FALSE ("Yanking")) -> ()
                        }
                      }
                      n2276 = local read "Trap Delta (MHz)"() -> (w3733:dbl)
                    }
                  }
                }
                frame #1 {
                  n2277 = local read "Stop All"() -> (w3815:bool)
                  n2278 = local read "Fl. Triggered..."() -> (w3813:bool)
                  n2279 = Not(x=w3813) -> (.not. x?=w3814:bool)
                  n2280 = Or(x=w3814, y=w3815) -> (x .or. y?=w3812:bool)
                  n2281 = Not(x=w3812) -> (.not. x?=→"Waiting":bool)
                }
              }
              n2282 = node-c288() -> ()  [unwired: 2 out]
            }
            n2283 = node-c288(w3708) -> ()  [unwired: 1 out]
          }
        }
      }
      event "Stop All": Value Change {
        n2284 = event-data() -> ()  [unwired: 7 out]
        n2285 = local read "Stop All"() -> (w3821:bool)
      }
    }
    n2286 = node-c288() -> ()  [unwired: 2 out]
  }
  n2287 = node-c288(w73) -> ()  [unwired: 1 out]
  n2288 = node-c288(w163) -> ()  [unwired: 1 out]
  n2289 = flat-sequence {
    tunnel: w33 -> [w3826]
    tunnel: [w3825] -> w39
    tunnel: [w3822] -> w38
    tunnel: w37 -> [_]
    tunnel: w36 -> [_]
    tunnel: w35 -> [_]
    tunnel: w34 -> [_]
    tunnel: w32 -> [w3823]
    tunnel: w39 -> [w3829]
    tunnel: w38 -> [w3828]
    frame #0 {
      w3824 = FALSE ("APD to FIFO")
      n2290 = xnode "Read/Write Control"("FPGA VI Reference In"=w3826, "error in"=w3823, "APD to FIFO"=w3824, "AI to FIFO"=w3824) -> ("FPGA VI Reference Out"=w3825:T19, "error out"=w3822:errorcluster)
    }
    frame #1 {
      n2291 = xnode "Invoke Method"("FPGA VI Reference In"=w3829, "error in"=w3828) -> ("FPGA VI Reference Out"=w3827:T19)  [unwired: 1 out]
      n2292 = xnode "Close FPGA VI Reference"("FPGA VI Reference In"=w3827) -> ()  [unwired: 1 in, 1 out]
    }
  }
